vi "UHR-Fleezers Control (host) - 10.8MV.vi"() -> ()   [LabVIEW 2013]
uses:
  <vilib>/Utility/miscctls.llb/LVPoint32TypeDef.ctl
  <vilib>/Utility/miscctls.llb/LVMinMaxIncTypeDef.ctl
  <vilib>/userdefined/High Color/nirio_resource_hc.ctl
  <vilib>/Platform/TimedLoop/XDataNode/timing_clust.ctl
  <vilib>/Platform/TimedLoop/XDataNode/nitl_modes.ctl
  <vilib>/Platform/TimedLoop/XDataNode/wakeup.ctl
  <vilib>/Analysis/baseanly.llb/Mean (DBL).vi
  <vilib>/FPGAPlugInAG/PCIe-7852R/niLvFpga_Open_PCIe-7852R.vi
  <vilib>/FPGAPlugInAG/PCIe-7852R/niLvFpga_Reset_PCIe-7852R.vi
  <vilib>/Utility/error.llb/Error Cluster From Error Code.vi
  <vilib>/rvi/errors/niLvFpgaAdjustHostInterfaceError.vi
  <vilib>/rvi/interface/common/niFpgaWaitOnOcc.vi
  <vilib>/FPGAPlugInAG/PCIe-7852R/niLvFpga_Run_PCIe-7852R.vi
  <vilib>/express/express analysis/Spectral/Block/exnSpectralBlock spectral measurements PSD poly.vi
  <vilib>/express/express analysis/Spectral/Block/exnSpectralBlock spectral measurements PSD WFM.vi
  <vilib>/Waveform/WDTOps.llb/WDT Append Waveforms DBL.vi
  <vilib>/FPGAPlugInAG/PCIe-7852R/niLvFpga_Abort_PCIe-7852R.vi
  <vilib>/FPGAPlugInAG/PCIe-7852R/niLvFpga_Close_PCIe-7852R.vi
  openfpgaref.8.6.ctl
  <vilib>/Platform/TimedLoop/XDataNode/XDataNode.xnode
  <vilib>/rvi/interface/nirviOpenFPGA/nirviOpenFPGA.xnode
  FPGA Bitfiles/UHR-FleezersInst_FPGATarget_UHR-FleezersCont_0F5B06C4.lvbitx
  UHR-Fleezers Control (fpga) - 10.3.vi
  <vilib>/rvi/interface/nirviMethod/nirviMethod.xnode
  <vilib>/rvi/interface/nirviReadWriteControl/nirviReadWriteControl.xnode
  <vilib>/express/express analysis/Spectral/XNode/ExpressSpectralMeasurementsBlockNode.xnode
  <vilib>/rvi/interface/nirviCloseFPGA/nirviCloseFPGA.xnode
  <vilib>/Analysis/NI_AALBase.lvlib
  <vilib>/Platform/TimedLoop/XDataNode/XDNodeRunTimeDep.lvlib
  <vilib>/vision/NI_Vision_Development_Module.lvlib
  NiFpgaLv.dll
  <vilib>/FPGAPlugInAG/PCIe-7852R/niLvFpga_ConfigureFifo_PCIe-7852R.vi
  <vilib>/rvi/errors/niLvFpgaMergeErrorWithErrorCode.vi
  <vilib>/FPGAPlugInAG/PCIe-7852R/niLvFpga_ReadFifo_PCIe-7852R.vi
panel:
  out "Location path":path=path "D:/UnifiedHighRes_VIs/Locations.txt"
  in  "ESP ZL-Limit":string="-0.5"
  in  "ESP ZR-Limit":string="12.5"
  out "Location Matrix":string[][](array[string])=[["N.D.\r\n", "N.D.\r\n", "N.D.\r\n"], ["0.19233\r\n", "0.00156\r\n", "0.20615\r\n"], ["N.D.\r\n", "N.D.\r\n", "N.D.\r\n"], ["N.D.\r\n", "N.D.\r\n", "N.D.\r\n"]]
  in  "radius":i32=10 min=1 max=20
  in  "clear markers":bool
  in  "trap\nmarkers?":bool
  in  "Sample Channel Flow":bool
  in  "Pump 3 contents":string="Bottom: ADig beads" caption="contents"
  in  "Pump 1 contents":string="Top: DNA beads" caption="contents"
  in  "Scripts":T1(tab)
  in  "Take Stepping Data":bool
  in  "Got DNA bead":bool
  in  "Got ADig bead":bool
  in  "Cap 1 Flow ON":bool=TRUE
  in  "Move Cap. 1 (DNA Top)":bool
  in  "Cal/Data Acq. Spot":bool
  in  "Dump Beads":bool
  in  "Cap 1 T ON":bool=TRUE
  in  "Cap 1 Samp Flow ON":bool=TRUE
  in  "Offset 2 Set":dbl=2.0
  in  "Offset 1 Set":dbl
  in  "Cal @ (MHz)":dbl=41.0
  in  "W/ Offset 1":bool
  in  "Offset 1 Start (MHz)":dbl=13.0
  in  "W/ Offset 2":bool
  in  "Offset 2 Start (MHz)":dbl=16.0
  in  "Pause at Closest Delta (s)":dbl
  in  "Move to Delta 2 (MHz)":dbl=41.0
  in  "Attempt Limit":dbl=30.0 caption="Limit"
  out "Attempts":dbl=1.0
  in  "Wait Before Save (s)":u32=1
  in  "Fish for Tether":bool
  in  "Closest Delta (MHz)":dbl=21.0 step=0.25
  in  "Stop F (pN)":dbl=3.0
  in  "Then...":string(combo)="5"
  in  "Move to Delta 1 (MHz)":dbl=41.0
  in  "Tether Alarm?":bool=TRUE
  out "Tether":bool
  in  "TA Cancel Save?":bool=TRUE
  in  "TA Green Off?":bool=TRUE
  in  "Raster Set Upon Tether":u32=1
  in  "Save at end (5, 6)":bool
  in  "N Steps":dbl=20.0
  in  "Step Size (nm)":dbl=0.34
  in  "Save ave factor":dbl=1.0
  in  "Dip Trap Delta 1 (MHz)":dbl=15.0
  in  "Move Trap Before?":bool
  in  "Save Data After?":bool
  in  "Green ON After?":bool
  in  "Dip Trap Delta 2 (MHz)":dbl=15.0
  in  "Move Trap After?":bool
  in  "Duration (s)":dbl=1.0
  in  "Dip for Protein":bool
  in  "APD to Watch":bool
  out "Duration (s)":dbl
  in  "Action":string(combo)="Yank"
  in  "Fl. Triggered...":bool
  in  "Fl. Delta Thresh. (kHz)":dbl=0.6
  out "Waiting":bool
  out "Fl. High":bool
  in  "N pts to average":u16=6
  in  "Yank Delay (s)":dbl=3.5
  in  "Yank to Delta Array (MHz)":dbl[](array[numeric])=[16.3, 15.85, 14.85]
  in  "N Array El":u8=3 min=1 step=1
  in  "Random Choice":bool=TRUE
  in  "Force Yank":bool
  in  "Force Reset":bool
  in  "Y change (mm)":dbl
  in  "Profile":bool
  out "Sigma/Mean 2":dbl=nan caption="Sigma/Mean" format="%#_2g"
  out "Rate sigma (Hz) 2":dbl caption="Sigma (Hz)" format="%0.2f"
  out "APD 2 Rate (Hz)":dbl format="%#_3p"
  out "Primary Video Display":T2(plugin-control)
  out "Waveform Graph":dbl[](graph) caption="APD Line Scan"
  in  "Inject Top":bool caption="Inject Pump 3"
  in  "Inject Bottom":bool caption="Inject Pump 1"
  out "Messages":string="7:59 AM\tUHR-Fleezers ready.\r"
  in  "APD Ave N":dbl=10.0
  out "Int. Time (s)":dbl=3.0
  in  "Stop All":bool=TRUE
  out "Sigma/Mean":dbl=nan format="%#_2g"
  out "Rate sigma (Hz)":dbl caption="Sigma (Hz)" format="%0.2f"
  in  "Tab Control 6":T3(tab)
  in  "APD 2 Offset":dbl
  in  "APD 1 Offset":dbl
  out "RMS (Ang)":dbl=nan format="%_2g"
  in  "Bead Sep. Int. Time (s)":dbl=5.0 caption="Int. Time (s)"
  in  "Below (kHz)":dbl=0.5
  in  "Above (kHz)":dbl=2.0
  in  "Adjust Scale\nto Mean":bool
  in  "Rescale on Mean":bool
  in  "Offset (nm)":dbl
  out "Mean":dbl=nan caption="Mean (V)" format="%#_3g"
  out "Force":waveform(dbl)[](graph)=[{"t0"=timestamp(12.90000000000001 s since 1904-01-01), "dt"=0.15, "Y"=[nan, nan], "attributes"=variant("NI_ChannelName"=variant(string "T1 X"))}, {"t0"=timestamp(12.90000000000001 s since 1904-01-01), "dt"=0.15, "Y"=[nan, nan], "attributes"=variant("NI_ChannelName"=variant(string "T2 X"))}]
  out "APD Chart":waveform(dbl)[](graph)=[{"t0"=timestamp(12.90000000000001 s since 1904-01-01), "dt"=0.02, "Y"=[0.0, 0.0, 0.0, 0.0, 0.0, 0.0, 0.0, 0.0, 0.0, 0.0, 0.0, 0.0, 0.0, 0.0, 0.0], "attributes"=variant("NI_ChannelName"=variant(string "APD 1"))}, {"t0"=timestamp(12.90000000000001 s since 1904-01-01), "dt"=0.02, "Y"=[0.0, 0.0, 0.0, 0.0, 0.0, 0.0, 0.0, 0.0, 0.0, 0.0, 0.0, 0.0, 0.0, 0.0, 0.0], "attributes"=variant("NI_ChannelName"=variant(string "APD 2"))}]
  in  "Calibration":u16(ring) items=["None", "Position", "Force"]
  out "T1 X":dbl=nan caption="T1 X (V)" format="%0.2f"
  out "T2 X":dbl=nan caption="T2 X (V)" format="%0.2f"
  out "Bead Separation":waveform(dbl)(graph)={"t0"=timestamp(12.90000000000001 s since 1904-01-01), "dt"=0.15, "Y"=[nan, nan], "attributes"=variant("NI_ChannelName"=variant(string "T1 X"))}
  in  "Amplitude (nm)":dbl=3.0
  out "Bead Mean (nm)":dbl=nan caption="Mean (nm)" format="%0.2f"
  out "Difference":dbl=nan caption="Difference (V)" format="%.2g"
  in  "Take Detection Laser\nImage":bool
  out "APD 2":T2(plugin-control) caption="APD 2 (Cy5)"
  in  "Flip Green Filter":bool
  in  "Set X Only":bool
  in  "Set Y Only":bool
  out "APD 1":T2(plugin-control) caption="APD 1 (Cy3)"
  out "Detection Laser Y":T2(plugin-control)
  out "Pointer Y (V)":dbl format="%_3g"
  out "Pointer X (V)":dbl format="%_3g"
  in  "Set Confocal Spot (X-Y)":bool
  out "Detection Laser X":T2(plugin-control)
  out "Saved APD":dbl[][](graph) caption="Most Recent Time Trace"
  out "Trap Delta Graph":dbl[](graph) caption="Most Recent Time Trace"
  out "Save APD Deriv":dbl[][](graph) caption="Most Recent Time Trace"
  out "Delta Fl. 1":dbl
  out "Delta Fl. 2":dbl
  out "All Signals":waveform(dbl)[](graph)=[{"t0"=timestamp(12.90000000000001 s since 1904-01-01), "dt"=0.02, "Y"=[0.0, 0.0, 0.0, 0.0, 0.0, 0.0, 0.0, 0.0, 0.0, 0.0, 0.0, 0.0, 0.0, 0.0, 0.0], "attributes"=variant("NI_ChannelName"=variant(string "APD 1"))}, {"t0"=timestamp(12.90000000000001 s since 1904-01-01), "dt"=0.02, "Y"=[0.0, 0.0, 0.0, 0.0, 0.0, 0.0, 0.0, 0.0, 0.0, 0.0, 0.0, 0.0, 0.0, 0.0, 0.0], "attributes"=variant("NI_ChannelName"=variant(string "APD 2"))}, {"t0"=timestamp(12.90000000000001 s since 1904-01-01), "dt"=0.15, "Y"=[nan, nan], "attributes"=variant("NI_ChannelName"=variant(string "T1 Y"))}, {"t0"=timestamp(12.90000000000001 s since 1904-01-01), "dt"=0.15, "Y"=[nan, nan], "attributes"=variant("NI_ChannelName"=variant(string "T1 X"))}, {"t0"=timestamp(12.90000000000001 s since 1904-01-01), "dt"=0.15, "Y"=[-0.0004235663930173644, -0.0004722739341410556], "attributes"=variant("NI_ChannelName"=variant(string "T1 Sum"))}, {"t0"=timestamp(12.90000000000001 s since 1904-01-01), "dt"=0.15, "Y"=[nan, nan], "attributes"=variant("NI_ChannelName"=variant(string "T2 Y"))}, {"t0"=timestamp(12.90000000000001 s since 1904-01-01), "dt"=0.15, "Y"=[nan, nan], "attributes"=variant("NI_ChannelName"=variant(string "T2 X"))}, {"t0"=timestamp(12.90000000000001 s since 1904-01-01), "dt"=0.15, "Y"=[-0.0005883053071687949, -0.0006281319620349712], "attributes"=variant("NI_ChannelName"=variant(string "T2 Sum"))}, {"t0"=timestamp(12.90000000000001 s since 1904-01-01), "dt"=0.15, "Y"=[nan, nan], "attributes"=variant("NI_ChannelName"=variant(string "T1 FB X"))}, {"t0"=timestamp(12.90000000000001 s since 1904-01-01), "dt"=0.15, "Y"=[-0.0004680013428144157, -0.0005167699209570592], "attributes"=variant("NI_ChannelName"=variant(string "T2 FB Sum"))}, {"t0"=timestamp(12.90000000000001 s since 1904-01-01), "dt"=0.15, "Y"=[nan, nan], "attributes"=variant("NI_ChannelName"=variant(string "T2 FB X"))}, {"t0"=timestamp(12.90000000000001 s since 1904-01-01), "dt"=0.15, "Y"=[-0.0006226691488387671, -0.0006504715109714008], "attributes"=variant("NI_ChannelName"=variant(string "T2 FB Sum"))}, {"t0"=timestamp(12.90000000000001 s since 1904-01-01), "dt"=0.15, "Y"=[-0.0007901852473525123, -0.0008601641895809732], "attributes"=variant("NI_ChannelName"=variant(string "PSD Y"))}, {"t0"=timestamp(12.90000000000001 s since 1904-01-01), "dt"=0.15, "Y"=[0.00031556138798181086, 0.0002525101474044007], "attributes"=variant("NI_ChannelName"=variant(string "PSD X"))}, {"t0"=timestamp(12.90000000000001 s since 1904-01-01), "dt"=0.15, "Y"=[-0.00019678334910122974, -0.0002453993346964931], "attributes"=variant("NI_ChannelName"=variant(string "PSD Sum"))}]
  in  "Signals to Plot":i32(listbox)
  out "Trap Disp. Freq. (Hz)":dbl=6.666666666666667 caption="Freq. (Hz)" format="%#_6p"
  out "Display Period (s)":dbl=0.15 caption="Period (s)" format="%#_6p"
  in  "Trap Disp. Downsample":dbl=10000.0 caption="Downsample" max=20000.0
  in  "APD Disp. Scale":dbl=0.1 caption="Scale (Divide,\nfor above plot only)"
  in  "APD Disp. Downsample":dbl=2.0 caption="Integrate" min=1.0 max=30.0 step=1.0
  out "APD Display Freq. (Hz)":dbl=50.0 caption="Freq. (Hz)"
  out "APD Display Period (s)":dbl=0.02 caption="Period (s)"
  out "FFT 1":cluster{"f0":dbl, "df":dbl, "magnitude":dbl[]}[](graph)=[{"f0"=0.0, "df"=16.666666666666668, "magnitude"=[-331.1367572010275, -79.05506245821404, -86.61411242440559, -88.4728176091699, -90.3181253945935, -94.12566333707997, -92.52740723119955, -94.92192587982518, -99.60936585245742, -96.87568627870715, -94.02570383337763, -83.8058550151726, -97.57441397235512, -101.59968530846606, -101.523049255742, -103.35038532190343, -101.58594091014982, -102.96098031851216, -91.39759462745924, -103.75019963279499, -104.45030075054324, -103.04245334279298, -104.0720279134107, -106.06482372394834, -103.69131867828104, -104.40395035115309, -105.96420043276396, -107.6735556337804, -106.673030006608, -107.34889066208132, -108.05626565233933, -106.25659018850432, -105.29934513380842, -105.43096056709592, -108.3728498841465, -106.0555440144992, -105.78001282181421, -107.48741857324953, -108.67624970548897, -105.39976667156175, -105.91413119232612, -109.4222808198164, -107.0898971593174, -107.91164191890915, -108.26032038855709, -107.58332347164534, -108.23559688234297, -108.01271040303237, -107.66511723652701, -106.51901583170391, -109.27249501469946, -108.55647681594805, -107.93499259231463, -107.05068166453935, -109.13641475410455, -109.29679733781423, -108.19360835527803, -109.57747591546632, -109.58364591011674, -110.47061433372711, -109.8144340420426, -108.79067462293897, -107.54887553357234, -107.99559866705923, -108.85023923652685, -109.68733225238618, -108.51101278437793, -108.51620475114115, -108.22212402200637, -104.63726950302143, -110.2989919678048, -107.61796444414897, -108.68882962798736, -104.79193983043893, -103.59504263746938, -93.64633660288543, -101.9191640501395, -105.73717393151816, -108.92572458793902, -107.43962662800902, -107.79595323081325, -107.0923101993207, -108.17603277205289, -107.87074270713183, -109.20899066381877, -108.61832060412445, -109.10072003106593, -105.76480632823524, -108.60877649218978, -109.67541158970121, -110.2286232768028, -109.84952155309578, -109.33772024076384, -109.95251642394683, -110.14777282585466, -109.13825677905699, -110.05989365698167, -109.39359990189426, -110.56255614635295, -109.66477183197163, -108.9397158528824, -110.26529907650465, -109.20049464984628, -108.20183857013548, -109.09752250184418, -108.00440442238454, -108.35465963524055, -111.16774134451799, -110.34812550238405, -108.94506763426756, -108.72845542102493, -109.41512344014713, -112.44661664432377, -110.35437330889101, -111.32939440655925, -109.42989530434981, -110.98084669076195, -111.92160561143541, -108.57755551751093, -111.40042616180912, -110.15284955891853, -112.21455132279115, -111.40787773511747, -108.82949641635288, -110.13442122547907, -111.42229298204664, -112.06314940885191, -110.6015308813694, -109.51144097251623, -111.15989713761475, -110.25535755335385, -109.65868178057926, -110.51649885452997, -109.77194745285269, -108.4234206864394, -109.50892632093968, -109.46471287444389, -107.92241289271415, -109.72283805386196, -108.63426821579918, -110.37316681536255, -111.09713996884652, -110.32903619589223, -105.32012665515045, -107.36858557554393, -108.00382215905725, -110.06430686942338, -108.81666625979916, -110.01277074453823, -110.94194741225512, -109.65934609082873, -107.80979136006962, -112.81333866824724, -111.61474300955487, -109.83998277184975, -109.45953946904639, -109.79640584952526, -108.19172301667324, -109.28894656674316, -107.61471301278785, -108.83814006090513, -109.08866847726084, -108.20250571862371, -107.96222236861584, -107.03811197900873, -108.93533000393974, -107.74482548035408, -110.79811544577694, -111.1387476496877, -107.42970105883512, -109.18442281176472, -108.73546184641192, -108.71800246690864, -108.51945944378063, -108.06825856571285, -107.27210712368412, -108.12304695877637, -107.84933283677306, -109.73682373154998, -109.32284761503395, -109.31328817453769, -106.68762108642842, -109.79203616876461, -109.9020278896408, -110.27080024357275, -108.54152101558762, -111.00464391726017, -112.42244020766577, -110.82707315747889, -111.00344011890857, -109.90461839395674, -109.42877207451863, -109.73549298167016, -111.67494793393293, -108.85799077901427, -108.5348443278263, -109.803781083881, -108.30644755543659, -108.5079527456017, -111.2055351312823, -108.53089994340155, -108.01739789012176, -108.70360662855235, -107.95873456794631, -109.58297170693093, -108.9372401694271, -110.15921663527153, -109.22399119911955, -110.89883651739237, -108.92840112258382, -110.0545300523626, -109.05961065387005, -109.45831398589371, -108.61239387653227, -110.13001256174265, -108.80060224137931, -109.46327400696283, -108.0177965824709, -109.29727944627197, -110.3237255895986, -109.03258262543821, -110.97880178489321, -109.70034895077919, -111.16405638194153, -109.17324451464711, -109.65698250854277, -108.96750235822178, -112.00534231585624, -108.69274607723942, -108.98110446396657, -108.40723795464795, -111.44459094807324, -111.74799245277113, -111.1601960491512, -108.92048232753773, -110.30506377784799, -111.33145973979093, -110.91850998672503, -110.33684985776448, -108.90206518366908, -109.28458878227542, -108.98773986023751, -110.85813863075646, -109.00041591105906, -110.84543686681204, -109.84382395806176, -109.69722434763266, -108.50915601095721, -107.80829925826895, -110.59736107582401, -109.75377770317087, -109.3992084496136, -110.51151565846742, -112.49753959826434, -109.7299632589479, -109.54070743868353, -109.90314341132164, -111.05974202976806, -109.03766862152392, -109.46667095459878, -109.52800799036197, -111.3163121356807, -110.07817134522178, -108.69251657453547, -109.40472158898045, -109.71400709815576, -110.60534468715097, -109.46937396724682, -107.70342491418788, -109.86331122597839, -108.64971387994616, -110.90117371097081, -108.34928840565928, -110.04172889660904, -111.52979926554961, -110.34759300823305, -109.62712781837159, -109.24131154553284, -110.23196152450447, -108.68509612326807, -108.0246905483419, -106.61876139289784, -101.5519630114271, -80.57695480953835, -102.03744443354402, -107.1449217193017, -110.0695213407169, -106.61597783999268, -110.79221011808191, -109.58974545931426, -109.1149802216988, -109.20993813088597, -109.63768480465863, -110.10428394219181, -109.08445084271477, -108.83472375362581, -109.69508502050168, -108.05588796178941, -110.62586360101581, -109.95315261676905, -107.52208264977473, -108.80708007514875, -110.43484881098874, -110.45942171588936, -107.83804717866751, -109.98973910294193, -109.3496496054193, -108.425252911127, -110.94579264380809, -108.54181722177951, -108.67696070083541, -108.4150202151644, -109.24973583101504, -112.0454922608961, -111.29046597340738, -110.75018248960077, -109.38326363603683, -109.2033340336957, -109.45076170874889, -109.52878049853727, -109.32340869724774, -110.98123395128233, -110.75736340635505, -109.7218385823809, -107.97422606064993, -109.77313701758703, -110.95948744392717, -110.08996774172691, -108.51011830110778, -109.78063140243836, -110.65996628628228, -109.83684298615616, -110.33329049188029, -110.13755118968292, -110.3717925645783, -108.55302219178951, -106.86811628734195, -108.6302156589162, -108.75341391045045, -108.32589578384841, -108.70061474734084, -112.30742263527534, -109.16842570592085, -109.29767035534508, -108.87829025017463, -108.2255616391397, -108.4316108616088, -108.82995906929271, -110.40135575415563, -109.51623498946435, -109.79409808792403, -107.03832759632121, -108.36534528684132, -109.72010868372905, -107.90933028179892, -106.95643597294047, -111.29929166165778, -110.23001135794706, -108.98838015381585, -109.79115357104436, -108.18627479511115, -108.14988122174307, -109.12074063466532, -109.41904850488358, -111.40409873721113, -108.83156790193294, -108.77032248953847, -108.88363158686694, -108.47515048290681, -105.94172147874599, -109.38146940214403, -109.21277078848794, -108.11309390545507, -110.70840012427504, -109.5504457849329, -109.52330684534209, -110.06776026911132, -108.21949434182314, -111.21266686269992, -108.78581501170974, -108.43115799297222, -109.63260325780062, -109.84070220619535, -109.72041980780126, -110.29615941882527, -110.60316734262464, -108.79165446414692, -110.95840439895592, -109.64926233107009, -109.16526769544322, -108.65292362430982, -109.56113898129935, -109.85693046339026, -108.92316027325207, -109.79492493553914, -109.38157962945887, -110.24545136266825, -109.30031463492487, -109.0795429936869, -111.4091719525013, -108.63499083917162, -108.43863465339358, -109.23207864880891, -111.21947487191643, -109.24525201480154, -109.56842406077318, -109.46711940800672, -111.91389548262572, -108.15655736690546, -108.71882059966947, -111.26328503478568, -110.95027143873176, -108.4853106242357, -110.36902802777546, -109.9314203579182, -108.77686164101732, -108.71871020068312, -111.04829661168574, -109.95072655339462, -109.88221342875462, -109.53241732756136, -108.2625005404823, -108.00677030040697, -110.19659317581693, -108.93858924796267, -109.46817875483995, -110.78063992017232, -111.11066570318451, -110.78774336696706, -109.19199744617812, -108.54914256407436, -109.28414960420909, -110.64143585101183, -110.5855350821307, -109.47578632252726, -108.89705360836223, -109.89214013612292, -107.93271261027171, -109.32631601340563, -108.60274611341092, -109.40110159872573, -110.889237682208, -110.01391165813328, -109.99747108785071, -108.65542819213674, -110.37211847668736, -110.44656500845738, -110.8128133834973, -108.8909299260433, -110.19551227077532, -111.37647266643523, -110.83802189730321, -109.98519377913681, -110.52378970770522, -108.16970420057817, -110.70974729773344, -110.76836765494402, -110.26884275594577, -109.22041044268806, -109.87809744746195, -107.76823252107832, -109.12119474042969, -110.28066108731146, -108.55000033509207, -110.18152097767907, -110.73030521152278, -111.49470908029893, -110.2320929919509, -110.03370979233021, -109.79181668155233, -108.6673501209991, -109.86695766650877, -107.88926518046961, -110.95525003776572, -109.18130359755742, -110.42618009658618, -107.90341931158893, -111.44736855661769, -110.72634267386593, -109.29945988519303, -107.67889101961411, -108.81148059987765, -109.13375212757057, -109.8122873383549, -109.80176697684155, -109.96342275204768, -109.90406635707086, -108.75674342748256, -110.12362902701081, -109.82151095527837, -108.62543344241836, -110.09171852771195, -110.21434637862887, -109.97254504855631, -109.27043209093468, -111.35149588204125, -110.12399876776051, -111.65983675538546, -109.28788875768564, -110.86554069990251, -111.26990906470603, -108.60956517491746, -111.49613890850938, -111.79685722966795, -109.26269485364045, -110.38555615546439, -109.40641023162068, -110.966136593156, -108.78892524584494, -110.29340727375603, -111.44032043281035, -109.95212021173755, -109.79233511584334, -112.41184021118175, -109.73687851881148, -108.65493879781806, -110.76132988919045, -108.43230346094671, -110.32968175895853, -110.29890782023821, -108.77609076424456, -110.3298662333555, -109.47734504217333, -108.2677295732245, -109.21234363352882, -107.83278941978479, -108.85136784424789, -108.43241251530755, -109.76609391460555, -108.53204373005357, -110.9660641972934, -110.3152512161094, -110.72570499399905, -109.23877906286317, -111.72407743101837, -109.20311421918561, -108.06021800233717, -109.29288625761943, -108.78395253409145, -111.85250172876302, -108.78827588901797, -109.79775055719482, -109.12089297455859, -109.49896359356035, -110.34432647103819, -107.94700097960238, -109.30489238477631, -108.89170290869342, -108.82574563272509, -110.11024077194833, -107.37946433552314, -109.60167933458756, -107.80625057819019, -110.11489057210264, -107.35436859378505, -105.69819484613895, -109.11280625683739, -109.27770293057978, -107.7053735252589, -109.75022444894368, -109.3310543596577, -107.87683693707739, -108.19931495338068, -109.26462246191564, -106.71885779297867, -100.00018022217961, -92.54434511397295, -107.20472143807373, -107.39203415155283, -110.04461177268398, -108.48860496315312, -109.0057168110333, -108.37627790492552, -108.4108380728248, -109.65509454313073, -109.64243000632982, -97.04219069306761, -109.0928856629964, -107.9760697315632, -107.52611064047497, -108.87702814778996, -109.08437599027614, -110.70097118837974, -109.00969860961283, -110.38275386163214, -110.0699155421545, -106.91498895181175, -106.22178738309017, -109.36827866896039, -107.59953130968307, -109.19516217272808, -108.31502495393616, -109.384158926223, -107.11670654202719, -108.09436312738853, -110.14559230873704, -109.84997663447679, -107.83465335309926, -108.60947100624459, -108.9932479423645, -109.17174810371898, -108.79457339828916, -109.40909327982367, -109.6328723628302, -109.51081854476179, -107.63054408568418, -109.63728404010122, -108.51163794839918, -107.55002282725216, -108.97796212764939, -107.24648164623483, -112.21470452291085, -108.74294024554423, -109.62070777514892, -108.05768666239368, -109.8224946685739, -109.34575507446003, -108.53536952609525, -109.60789300457671, -107.56681538208278, -109.22777325016398, -108.79047910308894, -110.10332477250668, -108.00206387955672, -108.45604004720035, -109.00645795765472, -109.81039564269616, -108.92785144634745, -108.3978471520567, -107.94411095685999, -110.53486519304262, -108.8773780319227, -109.03345093296107, -107.30746693745031, -108.54277704832029, -108.77629108166091, -108.91111762599647, -107.74965195880401, -109.97375370738439, -109.76326492689246, -107.91717581777407, -109.0730556927617, -107.66804873204664, -110.40438871064791, -108.05794247751498, -108.80206615156494, -107.51329354700796, -108.83687012994949, -107.57713176895379, -107.94774159581414, -109.41894615439651, -107.10869425078764, -110.51480854078629, -108.92221367099775, -109.91358786461535, -110.1744263092835, -109.30795472883494, -107.91359710691006, -109.77888185049835, -109.52060975706438, -108.66686651982212, -108.71041801553639, -110.13619546359467, -108.87957097273856, -109.72150387215271, -109.00776068810654, -109.70251113927438, -110.75769213896399, -108.53234896741436, -109.69439526582246, -110.15412541604617, -108.25183374628219, -107.97402569656481, -110.34920156998648, -108.45106995186384, -108.82031145748209, -111.38690005057539, -107.01968459818563, -110.3044500039584, -110.8755481852125, -111.08915057663255, -107.94824988655199, -110.21669144934839, -109.90539774633154, -109.58985438756767, -110.12258796623348, -109.41689951612143, -109.31128210476795, -109.00258476567323, -109.11093063041056, -108.83347064311234, -108.32685287566952, -109.44770946560935, -108.40145063144861, -109.68448193892085, -108.76525439243828, -107.62837139034596, -107.39300298848994, -109.36993934990318, -109.2465218489418, -106.66307369796812, -110.15891092764934, -109.57151745419041, -108.92425698310808, -109.8036704717834, -108.79751146756549, -109.25926431818017, -108.46260574057584, -109.1967554647261, -110.63319560262356, -109.02343067385144, -111.22073171487528, -109.4731095097105, -109.69335000085164, -109.48782989577005, -107.95204227683271, -108.19468255763758, -111.36195112053247, -109.55696116543685, -110.3130767640534, -108.9621824253354, -109.99735074896789, -109.20198058456344, -108.12100614259485, -111.27227490807289, -110.09248554008288, -109.14395535060149, -110.80882692379708, -109.22632926901655, -108.64497210802793, -111.00030482190711, -111.1317849358033, -107.43140429257826, -107.9783302193555, -109.2639893652291, -108.97008485446163, -108.66556668859064, -108.12995785876932, -109.73001061107855, -108.09691302413727, -110.68391499215569, -112.78583642012705, -108.7093037763389, -110.67868795924797, -109.0190959349128, -108.36247198231372, -109.82829353258869, -108.24916379311045, -109.84154533905823, -108.55470160833775, -109.75438989348815, -108.82865632118325, -107.63622268162582, -111.00943492886312, -110.81824358463759, -109.46028423652966, -107.52479398900992, -108.99087806823736, -109.94494831750349, -110.26788355564504, -109.8954055022304, -106.9478122391182, -108.91705388158901, -107.76095584490312, -109.28456723055147, -109.7982307261767, -108.98552661346622, -109.98937979783426, -110.57907422426224, -108.68113463944836, -108.06257240208589, -110.0707224529617, -109.19515280354733, -109.35868842818849, -110.37311467065695, -109.0404734478992, -108.16686395270187, -108.61859220485148, -109.19986437876149, -108.19707189725302, -110.06564239663074, -108.87850403465154, -110.63824157544798, -107.36918104067212, -108.7008736325543, -110.9359398265406, -111.08529123080929, -108.44209934821818, -109.79529621208783, -108.38917887958179, -108.169117639508, -109.24332926356216, -110.50584058811704, -109.63592524002665, -109.32261039377495, -109.16720880524552, -109.3084314664462, -109.5812223978583, -107.70213196487856, -108.0557884982431, -110.67058020007828, -111.68459781023608, -109.66270627185824, -110.52536245663693, -109.70208409132103, -108.78645420809342, -109.23122088059863, -109.24601474121832, -111.25604763816514, -109.50225851581177, -107.32434217163818, -109.28548556764925, -107.59972621660836, -110.46928774723048, -109.25950101547609, -110.32016453935465, -107.78482761561703, -107.89462895091089, -107.51366154391481, -108.08036891159172, -109.53371809947035, -101.2452927166745, -109.32763325689056, -107.52166868423687, -109.89648659445174, -109.11350200980485, -109.81336712738089, -110.02799517445062, -108.02767143538516, -107.97850220501483, -109.50772934896838, -109.31069875721964, -108.49991657749598, -105.60880911233095, -109.79128597340213, -106.91084537903113, -107.84880087118997, -109.63628170511824, -109.03203967193224, -110.64186113413658, -110.98027990365594, -112.33841002907062, -111.01793075565425, -108.58025797022215, -110.4259296883756, -110.38643255981424, -108.93051671115133, -110.97544177116494, -108.63883100482677, -108.37581711765226, -108.90240163126536, -107.94688047875466, -109.9482937437732, -110.09097112364414, -110.09805032265376, -111.44307114024532, -109.15483789122554, -110.9713708217832, -107.8548737634672, -111.41418477109195, -109.45699779859628, -97.03595099331734, -109.16746744169623, -109.66209204485918, -112.57048704774604, -109.73989735035725, -108.16252575067017, -110.7546980664636, -108.91536673403449, -109.20509151422344, -111.0260632167785, -109.62924582406518, -110.45466277291722, -110.2973970018937, -109.67550222925419, -108.84481022020094, -107.23686414357573, -111.79004633370906, -109.85453094194085, -109.45617270081004, -110.73920606732504, -108.90879956851099, -109.67774425528265, -109.4745715721361, -110.18080454693559, -109.26079184315502, -109.41692499885505, -109.02240975088358, -107.80833423058168, -109.32657361431549, -107.87138278655101, -110.910364670719, -109.70067156846706, -108.55301754282077, -109.4243252157005, -109.77567725161107, -107.83737232063925, -110.36509412773016, -109.6371048811367, -109.49430894422814, -108.55509251499753, -108.03996302911446, -110.4385715838736, -110.08864436068788, -109.48922484379962, -109.90865554258562, -109.7491963238264, -110.04796094537969, -107.413043439116, -108.54229076126079, -108.2522516728666, -109.75464941327974, -110.26795832300996, -109.28073673851144, -108.62990200974927, -109.89408067552287, -109.09160284731726, -109.90740624925795, -109.92534708896517, -109.79578862362752, -109.97278346890566, -107.80679350393824, -112.81728446281548, -108.09689504419987, -109.89549991422173, -108.43930976031248, -109.95153099843282, -108.18277483720716, -111.89607792605433, -109.52567003805, -109.17125106979698, -109.64300739407085, -108.21045178846524, -109.64036472149706, -109.02324448538845, -109.039163008889, -110.41006510134076, -109.50289952116489, -110.4732620447796, -110.08777181504614, -110.15589511434341, -109.55705089158471, -109.2547682932589, -110.86823885471617, -109.96330502176939, -109.85995369810554, -110.63211290903473, -112.08007783432191, -110.24725218052279, -107.62861148917592, -110.08691795849435, -108.89793794632287, -111.07702220466341, -109.46946126482341, -109.19747345337464, -110.70018609416007, -109.66366205691908, -110.78032312133551, -108.05724200456513, -108.195661625627, -110.90724508408255, -110.08307674771669, -110.76863516643007, -110.46620425061583, -109.16986788877276, -109.61921294239114, -108.51159432329543, -109.96308336765689, -107.38178944242856, -111.95930944846394, -109.3329826827624, -109.59119636368249, -108.83148571828912, -110.46194288788257, -105.87694286145472, -107.985886302892, -109.2975019660806, -111.05138725716857, -109.60005889204612, -110.92871351729086, -110.73480546964537, -108.41587420326718, -109.84275465824477, -108.8249071047676, -107.65358887817105, -108.3254150042995, -111.47362100321767, -112.7287536850025, -108.8217125660507, -109.50232320231771, -110.29587061625348, -109.30644535112089, -107.69178032077258, -110.84522325672016, -109.3735891463141, -109.12506388923123, -109.65582307934665, -111.11427272192576, -112.19827973435466, -109.11306367925813, -108.19203577968261, -107.89831568266465, -108.85805249169313, -109.51100049661844, -111.71546684086955, -109.53880495724334, -107.07739286222231, -110.66836728754211, -111.5415170557177, -110.16051267940297, -110.6107546662698, -111.36389129556191, -107.77888179117923, -110.34160392509817, -109.61287125994414, -110.23791773883013, -111.00669159903549, -110.97165069538953, -109.43965413392434, -110.6813161690388, -110.31441293654314, -111.96129906273796, -108.15998218707462, -110.08095912053633, -109.41084567452768, -109.28774416263552, -110.80159950384204, -110.41956747809755, -108.85005186267244, -107.9069227847757, -108.84249369063123, -109.92569208845894, -109.34109797584448, -109.41334788055491, -108.76462023086997, -108.22069272136177, -107.0786679601274, -108.30206755098202, -108.57613406368954, -110.83330887636482, -111.93966942736989, -109.76373713473264, -108.25782074884941, -108.16490627215555, -109.93351470267982, -110.75525684428368, -108.22814762283093, -109.73442331991602, -107.53145627482685, -108.27195221226805, -110.33032779278457, -109.48951857415828, -108.12599093700939, -107.97627415508097, -108.81426859968796, -111.21764717894752, -109.80856212352333, -110.92658779118501, -109.71551885834796, -110.38682741010847, -108.87671328341361, -109.68368600774755, -108.35359806351899, -111.7519400010676, -109.89407081573103, -108.24301180922755, -110.00646944788126, -108.6685299083706, -107.52856885980722, -111.7622363038509, -111.0025144494897, -108.64719599357296, -110.62968467177518, -108.821509935539, -107.94915453463719, -111.53070432277694, -109.87282048586256, -110.71167589371663, -109.79225006081626, -109.96203471712074, -110.29921092232489, -110.10644439440416, -111.28815007382043, -111.19165661703703, -108.46024117100558, -110.22528296512183, -110.32184972386672, -110.05120383416072, -109.78792549362107, -109.00355659956696, -108.85989369286315, -113.00899556732638, -110.91756826567867, -111.25016866167897, -111.84225040552181, -110.54451635944174, -110.72722829912917, -109.60759702177283, -110.49362602516815, -108.74419542915284, -110.3379671069179, -109.66259088220754, -110.45956400953156, -109.13956157147233, -109.27130155486806, -110.83015602667983, -109.17970724944131, -109.09662765889193, -108.0447366108107, -108.9536269357457, -110.35663108940085, -108.73418835472056, -113.42965806805827, -111.81270536656905, -110.06155590173537, -108.76582224646269, -106.7488061675813, -108.5700320158723, -111.11038264410035, -110.41435767488723, -109.12763443489911, -109.30517580756394, -111.61251165371237, -109.8116632664339, -109.36845864976851, -109.00390009629231, -110.54359197165573, -109.52629258465976, -110.75932197632896, -109.50903215359567, -107.42652056246085, -107.81146496533543, -103.22224383145215, -108.53803076819163, -109.78623360072066, -109.66306634612869, -110.80245829141279, -111.87835085452016, -102.27372781471168, -111.27763038431458, -108.45838423437681, -108.79077917058028, -109.31951755762685, -110.05415097017186, -109.5535934823387, -111.62732254641111, -110.73478247119641, -109.9468722686683, -110.39698367573979, -109.30612942398305, -109.7578384694043, -109.34817295524313, -105.56944757301993, -110.1940418750125, -109.27076023513962, -111.03491935225027, -112.2980497521063, -110.65725497955563, -109.0567530102422, -110.31700596563523, -109.64508026365678, -109.6190471404421, -110.52566833759428, -109.68595899227789, -109.7431160985074, -110.4798230300751, -109.45506977604765, -110.69504157940786, -110.63067849573177, -108.06456949500138, -107.99354148885966, -108.11349194720599, -109.15944121207349, -110.61766925164031, -110.14145801314527, -110.67420842201165, -111.91532881806512, -112.15901550030345, -109.94774413630104, -109.2819568305201, -110.94623189179737, -110.17685430287735, -110.39082916961016, -109.53953238698966, -110.76940623620611, -109.89327922318515, -109.10275695043765, -110.21445972656734, -110.58968777252528, -110.57016757660259, -109.59208496373341, -109.07946946465374, -109.10762003745964, -110.36892993974607, -109.81864495218393, -112.12972189864566, -109.26185849434863, -111.56305819991357, -111.36019621828058, -110.3397604159226, -109.58675612753163, -110.58041217474447, -106.34739062044932, -108.6722699609389, -110.03906060709869, -109.16794717548382, -109.65012481802809, -109.35377624077988, -110.51889143862303, -110.03397458059777, -110.7981307056636, -110.56653507062292, -107.61367005067231, -109.99279736988825, -111.79875182878175, -108.60382315996031, -109.71381533228038, -108.60388131505613, -107.0933685540362, -107.86037690830757, -108.40980028847238, -108.83869602763895, -110.76921375395764, -109.96766364716046, -110.8256171465781, -110.13805084291067, -108.5349140035878, -110.57158437465219, -110.8920694413417, -108.71646695477324, -108.33274238445665, -108.96152108305608, -111.03750932994224, -109.48915027983756, -110.29725207211165, -110.79527247268442, -109.47969936716117, -109.79306701834035, -110.16840035577498, -110.29840230783668, -109.15306387075587, -110.72651274964761, -109.08881658764956, -110.8349724030761, -110.64653625576447, -111.40392562616867, -109.94581588927414, -108.85136340231294, -109.77228546607624, -111.48297395390018, -109.7334001251941, -109.30537415590783, -109.63937411233408, -109.69785848648013, -109.3523781030017, -112.04667421182404, -111.56311816195343, -108.18548447362308, -110.63388993686104, -111.39768634137992, -109.87157345395542, -108.6734208287271, -109.46213300216168, -111.75774769437145, -110.10245994173216, -109.52385139033495, -110.96513097775451, -111.8709319163154, -111.54948269614047, -110.29760900080463, -108.52168175904663, -111.09033925738258, -111.14752744054172, -108.83074523709202, -109.05704141259113, -111.74377805749482, -109.57200906899736, -108.84121318623825, -110.86657990204343, -109.54363603755047, -110.89448416316372, -109.58965570570145, -110.21012263847972, -110.4063470702923, -109.5021950342969, -110.33648801598177, -110.90551031296536, -109.69205870504638, -109.8648503154861, -110.28183391384131, -109.65970942950766, -108.43615680946908, -111.11790511866548, -110.89043476451553, -113.64898442872548, -113.08004494963895, -110.81525412051718, -113.91009875719509, -110.95802128672312, -110.40944585634135, -110.33464695414992, -109.98984645778987, -110.18795067005652, -110.62364351231234, -110.44029833291248, -109.01598585569788, -110.95430216511514, -109.77987141110621, -108.54452361812068, -111.41780266439777, -110.47172771858405, -109.06084635984516, -109.30794593246578, -108.8764083815745, -108.18222749506985, -110.31330487887435, -109.04176821738014, -108.8558386035048, -109.47888284507395, -110.01459604573937, -110.48596659065309, -112.6781342298378, -109.85522803775775, -109.0569534499285, -109.08991286548698, -110.89485727880403, -109.18715778948663, -111.50381433568144, -111.3545424730884, -110.07710926239977, -111.99977850157067, -109.47444853853723, -109.81605328527645, -110.74995213151195, -112.56834665925544, -108.52052472391404, -110.89121213995557, -112.02004142355113, -108.66413739656008, -111.10053848695652, -110.41241079991636, -111.80152991764473, -110.21746151515111, -110.63265128607344, -109.483042128511, -112.78639954059729, -109.47114195846122, -109.23309637902875, -108.97133643967169, -110.08909147812822, -111.01105271457081, -111.18602432128249, -110.04633990216801, -109.53453538673071, -108.81939452082017, -111.13486114285661, -111.65877073200598, -111.63763706753498, -112.14107810664572, -113.6231865196724, -109.31743865878806, -109.18551713085722, -108.74951309653638, -109.28206426212142, -112.36687029711229, -110.10933061193728, -111.29501093502684, -108.19021080564794, -109.34497312126749, -110.37228033937312, -108.63277512903049, -110.61033993911002, -111.2975761598062, -111.49780004751436, -109.91019436685814, -109.32789992989028, -111.4482538110117, -110.1538439123475, -110.66347034043578, -110.05055133068794, -108.53002033538341, -111.7522199783972, -113.49108651193104, -108.03793940563418, -110.07108694011555, -110.83958739865201, -109.62805629409038, -112.69637731014087, -109.57996950503268, -110.104850643722, -108.83376203949506, -108.69400304840181, -110.59434352922563, -110.69121011800921, -110.18694553784364, -111.90598571547098, -110.30230802494223, -109.66810649416752, -112.6017099000434, -111.00296745333219, -110.64462650261785, -111.4775358707403, -111.98753241268494, -112.26574909791167, -112.04796822399412, -110.65853064447325, -109.6623218025264, -109.40559579075378, -110.42174451813142, -109.18991987957241, -111.02050178263048, -112.77950487440032, -110.42443751566815, -111.35440372400903, -108.5263524245987, -105.07498063939795, -107.15444425741984, -110.4508720018025, -110.25163264819463, -111.1383261104107, -109.91171620173931, -110.52200560606038, -110.5299174299573, -109.34628087255733, -110.26101817411786, -109.65071853372183, -109.66953335961068, -110.83590602054682, -110.980546313788, -109.4110066989163, -111.47223607390256, -110.00281523859483, -109.4088722967626, -109.00401922839337, -109.59655302543185, -109.7359970854586, -111.46016206343049, -110.23478747568004, -109.29441275295858, -109.82941912510167, -110.43088525283673, -108.21649744751299, -108.70220592702613, -105.2334473604296, -110.60620657984927, -107.97533820921146, -110.7664079806058, -110.56406610911355, -111.76465470250328, -108.84172809688911, -111.03661078143631, -109.85351980370237, -110.70091167176791, -109.52380717508088, -108.4356492672842, -112.25498760397127, -110.69648730540193, -110.36748838594507, -109.99090797924349, -111.2678642544111, -110.42541694325627, -111.4575545259775, -109.3211175669008, -112.7465573314208, -109.56208667784249, -111.59733497772172, -109.42295730962105, -108.55804089331346, -108.71397903286748, -110.09188290952392, -108.90810063278326, -110.31333217069538, -109.69794714542728, -109.06210020835357, -112.42465112160288, -111.74630553904855, -109.99304310093493, -108.93867687355595, -113.1669287525049, -109.09193568851137, -109.27500368450697, -108.99643325722404, -110.53962759110647, -111.2052088429852, -110.05855563908841, -110.30763723153481, -110.03411001268613, -109.6161415052669, -110.6304714466923, -110.17116005754627, -109.0753171640551, -110.92564270851628, -109.60831770517053, -110.25913363817017, -107.76644895378317, -109.2619309023068, -107.64198246311884, -107.37056168314048, -107.31978563121643, -107.68171928702894, -104.57515288104209, -104.75187637758803, -105.27246893266054, -106.96524396060869, -105.93920355631757, -103.66449995825586, -104.08476660009461, -104.53081578265315, -103.0148493379086, -106.74751670818362, -104.92309629919443, -103.98320340724693, -104.81633219413234, -105.77996356028235, -107.12559309216644, -107.28196039053535, -108.84583578337953, -109.4494696919565, -109.15525441177898, -109.7634811359225, -110.79433338587495, -108.44440079452527, -108.79597700117748, -109.98590735173822, -110.72144284267539, -109.30550753718086, -109.70072152916897, -109.65801130162137, -109.65949265997646, -109.82238573025273, -110.30669821947491, -109.83394128869384, -108.90433312205332, -110.664046708231, -110.39926453734134, -110.37725911098757, -112.12508639032839, -110.26795666332589, -108.98741993218054, -107.76168841100478, -109.82334992872889, -110.83516363498563, -112.60649745671253, -111.1960726449926, -111.03919163866381, -112.05129034965563, -108.83187987662883, -109.57240688505179, -109.32857861150738, -109.54934849013647, -108.29359879300195, -111.5179112931669, -109.52702486426027, -109.95429980789645, -110.7011078611564, -109.43204524997455, -105.56031249677113, -107.70609254346495, -108.78303653454363, -108.11457060956113, -110.44215460317537, -110.78267897406572, -110.33119812901934, -109.34449539666907, -108.82636558484161, -107.1834151347969, -108.83808254322192, -108.2542825327446, -108.80298057862501, -107.59922121598055, -108.9131916496929, -109.51519107961856, -107.7704986323755, -108.79678029009878, -111.13791068210752, -110.402746275919, -111.31702623823912, -108.49812727557243, -110.63723264798182, -109.32890666586829, -110.29721723278237, -111.66560929315017, -111.04227698307153, -111.36927505376269, -112.5203298417673, -109.93967930487354, -110.14533835678606, -110.3868348991775, -110.85413569165249, -108.44519725537315, -107.93391978795047, -109.82778679299085, -109.79311153223738, -109.25261055399044, -111.47738679135526, -111.11775495397512, -108.65898844492045, -110.26505495390529, -111.02017977446526, -110.34817965403467, -107.55161094495372, -110.21667403085983, -112.43970497917284, -110.70535338255132, -110.79438078890512, -109.81809822502822, -108.99167960596515, -106.5556893069368, -97.51736665041192, -105.29926513345109, -108.72453297392224, -108.23203912463346, -109.50324111400698, -110.9939986929772, -108.05367524487318, -108.37339392211176, -109.8553291283933, -110.46179639493138, -112.48795697163695, -111.88145079973545, -110.8678969738583, -110.62677605624849, -111.83824818603244, -109.76798658735359, -109.6654742351465, -112.58543522753767, -110.3406716250781, -109.55013159400883, -108.00481229232405, -109.90793236599207, -111.28597960985334, -110.54144527494444, -110.14704702870655, -111.2652554338908, -110.97520848958668, -108.63647576273343, -110.52472680617548, -113.16137826273847, -109.62457037485827, -109.53869420402964, -110.71399284283449, -108.55435337782664, -108.09492728294455, -112.2373886856363, -110.3693019226993, -111.65116752865308, -111.3223986412311, -109.67734725401074, -111.36420709226297, -109.14293108556625, -110.5982939020188, -110.29596476096043, -112.69847120697035, -108.39052787054206, -109.06205229490357, -110.00045399262885, -110.71775009467346, -110.69530760167493, -112.54144940754935, -109.55755373438097, -107.88943697845929, -109.98578587243783, -110.14202980613851, -110.80051915904802, -109.11327182471621, -109.50637030500913, -109.77023677605327, -109.98552825925917, -110.40235854896, -109.37603004890141, -111.36989177909379, -110.8399811877331, -109.30394670937987, -112.2769814990538, -109.10893172594731, -109.17733972841754, -108.35968166480572, -112.64492569586005, -110.13779257328873, -110.64439690778532, -108.45446935516622, -108.97325006911116, -110.54637968933774, -110.66412364132371, -111.38627695224784, -109.8942998516069, -110.36392017322382, -109.92355133054227, -109.61886697310419, -109.71969465343778, -109.85627196259388, -112.1407808286419, -111.1013489416651, -110.70428953307596, -109.3454280179969, -110.22984684615578, -109.53826801613613, -107.83673208330934, -108.72742563398342, -109.5745872123195, -108.83031823548816, -110.89059911076627, -109.87842545384129, -109.21980161063786, -109.07140273870678, -109.04628915564135, -108.79255665097845, -105.20875397856382, -110.0838008881032, -109.68293832806683, -111.24644641302518, -110.01257579497496, -110.99281477454484, -108.99296184719546, -110.96495665514604, -110.70404386182749, -108.25078498739035, -100.77667501455139, -107.61479263900088, -110.06600976399395, -110.02035637581871, -111.45524052052504, -109.975541184397, -111.07333860975358, -108.4808974233161, -109.59513524582242, -110.74711589861774, -109.50005300854993, -105.23071652566294, -111.81094849223531, -109.0168079712372, -111.89029991620679, -109.90672274216391, -109.30959446424889, -108.23718655264584, -110.10868108588909, -109.21139771899594, -110.33333323577992, -110.25792318324204, -110.67825932924109, -112.33148517950511, -108.9724848367048, -110.78371843797613, -111.40913868573313, -110.2930522718577, -111.9538408094371, -108.63639312641844, -112.4462941079034, -110.40266356498321, -108.66617580940074, -109.44306834729083, -111.08962916641603, -110.52132608161017, -110.53757698855654, -111.5587344449704, -109.77722315102946, -110.40060629757771, -109.45395807961631, -108.77558572395142, -109.0151938598724, -109.80739619986889, -108.9332873172888, -112.49933978358132, -111.28667321897437, -110.40629082858706, -109.9829216820938, -108.85102919990373, -110.84179127037925, -110.27309817549309, -109.88857884367955, -112.24517967927224, -110.23377125710859, -111.26951227953063, -110.09782138347559, -109.77508406986834, -110.55359722398646, -110.09534729906368, -109.96333904888587, -110.29372855476366, -111.36651812163072, -109.97141184588116, -110.16701683369045, -112.8562627359291, -110.66651146857079, -108.78873821095968, -108.59208174618087, -110.31784275318834, -109.43177042415276, -112.80272887161644, -111.79874205007107, -111.08216899537892, -110.73699224045636, -111.04738767291953, -110.43395896705012, -111.62106163510778, -111.32599933330843, -110.29360981749807, -109.66562228449096, -109.21316193790335, -110.06363162177448, -110.54480468587292, -109.31791670875509, -112.65386492377107, -109.91857609999171, -110.57233605624137, -110.7597333064856, -111.49767138733276, -109.36548654843229, -112.34145274183716, -110.52831153822652, -111.55802243871352, -111.81399803046556, -110.17680125962372, -111.23811621944807, -110.48042049674514, -112.43786993562033, -109.56507357271987, -110.67030752598993, -110.86377249100713, -109.06001892813467, -111.37023727930494, -109.52881096984436, -112.95107295160436, -110.49467818026214, -109.29804210589607, -109.89270706931751, -109.46354468058833, -112.10350702955014, -111.06083529077077, -110.49996587015904, -111.1617248913634, -108.84725633199014, -111.42852695852422, -110.01433866707184, -109.11616968390972, -110.76961079765468, -111.80403513904453, -109.84442686379181, -109.65447921666167, -111.3378640555306, -110.8882647652338, -112.58014202075226, -109.67128881545659, -111.73429980763389, -110.82258070774773, -110.71895931098041, -112.5117489008152, -109.16182299471309, -109.71651258790612, -109.7770618808562, -111.94294809571427, -111.1629115541574, -109.57489224865171, -109.8402445779754, -111.17931450307283, -110.09045865447595, -109.23658206733491, -112.54929616847242, -110.5150381158864, -111.32296447909377, -111.64472156295191, -111.65832771066007, -111.03359562742956, -110.85303206770837, -110.80655337650862, -109.3712696310075, -110.57313454785879, -111.18525355670417, -111.67423695430561, -112.00829831274282, -111.08915434609605, -110.3298290221436, -108.68552957386795, -112.11377370993225, -110.80288297661977, -110.33640536217185, -109.5907971201988, -107.9195263775506, -108.50223113159429, -111.91191347156142, -110.29585599512956, -109.50902788911351, -110.76819145749467, -108.86899533416589, -112.09963049260891, -110.13374376572433, -110.15881393584463, -110.87392107947531, -109.18658540731009, -109.72734703956934, -110.18732487568724, -108.76554115185057, -109.94122289815374, -110.39583285609643, -111.09540935727229, -110.6618176357367, -111.6281345666718, -109.69686483639367, -110.31633402076315, -110.61246951748903, -111.73300235294965, -111.34221378834899, -109.46708370903485, -110.70412671997354, -110.7007891485379, -110.31685483435038, -111.03016917417074, -110.94517365625376, -109.46580797053619, -111.20935248224806, -109.20661126636224, -109.50147037097533, -110.14241781654353, -109.8510950344643, -111.3794198224028, -111.28966889207122, -110.43347441663424, -109.86759980279523, -111.92101892013198, -109.31594011390644, -112.92253433794441, -110.74000829597605, -110.3690783911604, -111.9386136764295, -111.04196305034188, -110.41800427558245, -110.94287511448232, -111.66035388807579, -107.53723747644062, -110.68014818358719, -111.86628806511304, -110.12097497430523, -109.69880468221378, -111.4312783987915, -109.18240866486639, -111.45649839248873, -110.1242345454651, -113.75911576151633, -112.71747598882953, -110.9614554157337, -110.92294419716129, -110.87229098694876, -111.09943759113875, -109.48107247947176, -108.62783006742795, -110.8108025857779, -111.63342408317932, -112.0221522906341, -109.96411229549527, -111.29821085030613, -110.04566676239914, -108.41674583097112, -107.50256474992416, -108.68086611003493, -110.3738906060137, -108.86763212826641, -109.81681043446049, -111.04539822346567, -111.73290882980949, -109.75238769150758, -110.55268275367449, -110.48423701377924, -112.1116140908134, -109.53952175199518, -108.538611608547, -111.3788321484912, -110.36378736224961, -110.37712171023523, -109.82150687920334, -109.17046632238393, -105.1169578108227, -110.84067642540583, -112.91626789016587, -111.32030958133453, -108.93375913686056, -112.44450956563915, -111.1596840012794, -110.17380444915341, -109.634859036508, -110.68819277718731, -110.0648098825346, -108.87385575091399, -111.99676414571755, -111.32585405719519, -110.59892045991457, -110.32589048340424, -111.1172696292077, -109.79946399891651, -110.10030723919304, -110.71841081343656, -112.23013150012054, -108.94400401141407, -109.71044551701596, -111.77560214164039, -109.68779520039777, -110.96119601299907, -113.66477058855787, -110.17794649102234, -110.30159876509862, -110.11953836266514]}, ...(2 in all)]
  out "FFT 2":cluster{"f0":dbl, "df":dbl, "magnitude":dbl[]}[](graph)=[{"f0"=0.0, "df"=16.666666666666668, "magnitude"=[-324.19011195451765, -78.1272953812706, -85.85545438627958, -89.30587144190069, -92.90590394398903, -93.63083388385274, -91.8644929119412, -95.26924857401164, -97.0710469181336, -98.01148078956652, -99.33043660296804, -95.58776817681839, -99.9570097527269, -101.45494093095093, -101.51838334751548, -101.00386616525799, -103.01963069818913, -103.20223925731209, -103.53783076500916, -103.48065647812659, -103.97797518531912, -104.58942778240602, -104.46991277190502, -104.59813972158683, -104.56685024229951, -104.69893799348945, -105.05669000016238, -106.17061117835001, -106.43303821862656, -107.39468286383597, -106.2899368267905, -105.7863846168199, -105.17170638885071, -104.53818172761852, -106.70340956723133, -106.55444321137247, -106.67654843051936, -107.79888413750199, -107.86424326005849, -106.09722609215336, -107.71648639013972, -107.79500725395155, -106.17330953637067, -105.43663624517525, -108.04970689199158, -109.92106271611999, -106.2505251183406, -110.60221373795562, -107.11377887451098, -108.4126937286195, -108.37794745021417, -113.22457316369011, -106.38281814065472, -107.55385617652075, -108.93026538982782, -106.19334142366085, -108.90462602264525, -107.63084712174981, -109.12192537022624, -107.90627042480016, -109.44472079190832, -108.91731458372392, -105.74102972706788, -105.74407510394178, -107.5989477192235, -106.2838630137392, -107.46190542725505, -107.38881299750702, -109.08024783239452, -104.97871836903269, -106.65424712290651, -107.04966019632134, -106.16202578092883, -102.98374199247179, -99.1568704142098, -87.07383781389657, -96.41471411313154, -102.65176579899618, -107.65674867775193, -102.85397890306213, -107.58658613411464, -104.79044898833125, -106.65282019869865, -108.65027966345534, -109.46169054950127, -108.69969979291741, -110.4048706652988, -108.81020193837274, -109.42808902484134, -108.85398463561398, -108.3849716744813, -109.1844457168716, -109.32787859535676, -111.01992124870878, -106.64843449415699, -108.9926343573667, -111.59837822080355, -110.57121677672183, -111.17280164669164, -110.68901970586144, -111.69013245592781, -109.90200577018311, -109.3554172126163, -110.7515368822992, -109.2863324212524, -109.66209701262974, -108.50795548698007, -110.58126481096504, -112.36093896766921, -109.78612141282203, -108.85120530917233, -109.91424431080952, -109.84698632196245, -110.93960894966105, -109.77214706089354, -110.30762971422381, -108.77791302937449, -110.79522659679036, -108.47242514643455, -111.20629758187835, -109.05996769621125, -111.13574821570619, -107.79388178889101, -111.5768481279296, -110.52058839597171, -111.58729762739313, -108.99000864386126, -111.6585121505227, -110.50715371958135, -108.87151956974363, -110.30486244367107, -108.32392040018144, -108.1769507919999, -110.43198471512189, -109.81454097966842, -110.26717009815644, -110.82924135076777, -110.34103661156989, -110.0692667126265, -109.34555682020833, -109.1694484721415, -109.9940980324044, -110.81940616215803, -108.21162003366862, -107.97087538330561, -107.55312461506225, -110.60339321606872, -110.09004629292225, -109.05860430198882, -113.1412749514818, -109.81628200948371, -108.62343219429849, -109.48172424209761, -110.85978755785311, -109.47778611557064, -108.81728552967951, -107.47864241666747, -107.61735128422292, -109.62511618983821, -110.32417726356636, -108.24287897478176, -108.60460879530194, -110.2181558494026, -107.95550802888957, -110.80234484950323, -111.09955733353904, -109.43923052503506, -108.98949130235951, -110.05778199870154, -110.36224432927585, -108.13523430027999, -110.681114579241, -110.49106131529867, -108.73493328004297, -110.07663907252234, -109.9968931372618, -112.10715231091008, -108.80994125105168, -111.63774865669372, -111.54355694032755, -111.64024217585788, -109.34986300492378, -108.88053713185408, -111.14370830146245, -111.17327416167232, -110.36311492990576, -109.99414559884396, -112.96912007380595, -111.43191437097785, -111.71327312809349, -108.77202323682606, -110.25970374932486, -112.59574277180732, -109.77247894866957, -110.09219852365874, -111.7197662726775, -109.85454092697009, -110.06789440397942, -110.38055758638309, -111.04251386932805, -111.54279434240568, -109.74385329575985, -110.98924544863415, -111.17898077762852, -110.98364252730245, -110.75024385843372, -109.24766708578407, -109.67753987004863, -110.6537235844391, -111.84436313010086, -109.12654337292446, -109.65519521121124, -111.1845162935778, -110.5009101465602, -110.22980642268818, -110.88540043278346, -110.29249073109453, -108.80459864528464, -107.49372141121728, -108.50353962704821, -110.00730069533373, -112.012876492648, -109.01283702976382, -109.07442203290057, -108.2961442983685, -111.60962842680907, -108.84312815413224, -108.6276642979969, -108.75132871638827, -109.30004903844721, -107.20359872252604, -109.12175943862074, -110.43914247337625, -109.55954680842791, -110.37116786618797, -108.55907813251434, -110.19249995041955, -106.95269845697632, -111.07027929458712, -110.1073996792702, -110.61729280468039, -109.6419175310234, -109.47995019876329, -109.66602827275211, -110.01953864498805, -108.45989120418268, -109.79778555296474, -109.94663827736616, -109.52410616839379, -110.58014441463794, -110.09182359045897, -111.0487262011397, -110.49609187214915, -110.6114701312941, -111.17752423063314, -109.74965389041003, -108.58973724447526, -108.84292130035902, -108.90689510645983, -110.69840140049361, -111.30494362640982, -111.00224390075273, -110.50848328538423, -111.59232911931113, -109.30826761863756, -108.44510893127558, -109.63744704504391, -108.95037574307332, -111.36486409910674, -112.74508631930381, -111.03952454593811, -110.57133212903979, -110.59969855145111, -108.25570461975128, -110.44617635200193, -110.32190307214704, -110.95204704643322, -112.0595421753479, -110.45342552693265, -112.50183987758867, -110.08217804938009, -108.90353583389084, -107.02032313792242, -88.3334978919524, -107.92027625495886, -109.83148570028482, -110.30427997450572, -110.92855407802753, -109.67404674397338, -111.03606345823586, -110.58277018943096, -109.77692362669393, -109.39170901729935, -110.20711662408928, -109.41601946806779, -110.34213214925832, -111.2283900972803, -111.51682597931386, -110.47069117801351, -110.93808974285523, -111.11277478000933, -112.50698886748012, -112.12918507523611, -110.46316790252011, -109.9387334819968, -109.78723249688426, -107.13037722044297, -108.16132376075751, -109.07255491017162, -108.85068428558272, -110.28038153100799, -107.77611023481016, -110.69754506886444, -110.09495581837979, -109.21214884561816, -112.62718526248648, -109.22048725312992, -109.17793923163308, -110.87372121410577, -109.71902632604333, -112.61041177225496, -109.6374750969677, -110.74738952366951, -108.93404661877067, -109.84938675700889, -112.25316361679832, -110.30788094875312, -109.26929069321925, -111.20853536783942, -110.05212566057608, -111.72448131932816, -111.55474439772887, -111.81988954424324, -108.44452452934028, -109.21897824914645, -109.55634869894358, -111.36318572800242, -110.05777399011298, -109.64458567712875, -108.73315084760529, -108.93332091319675, -108.4816455312154, -108.80120578498936, -108.1804470361839, -109.7177707524778, -109.31977709844544, -109.33603116022124, -111.46120546572519, -111.7480378245176, -109.17907150677627, -110.47970652472505, -109.73718750984082, -109.7935026884937, -110.40458408612054, -110.91781389491092, -108.39352075861481, -108.27512197925346, -109.59155075404814, -110.40183121737397, -109.25423373270381, -108.37769008625712, -107.91335995938509, -109.5576520703013, -107.27392145737491, -110.98592762117059, -108.41809950647861, -111.48163889400448, -109.70961684769624, -109.22952568656495, -109.76504719131209, -108.86928627177666, -107.97855299877004, -109.8412204399902, -109.6690048999326, -112.28329030175193, -111.54977099314607, -109.55689540119126, -107.93716711232997, -109.84247640855929, -111.5098351445789, -109.14317615215809, -110.28319116384824, -110.57901069942578, -107.2890252845352, -109.66754569546274, -110.15708115946433, -108.83782190109405, -111.60783857760667, -111.46884385151185, -109.21985333366634, -109.63605494317056, -110.87999187262697, -112.26992029775087, -111.05491095860552, -109.22795442529183, -108.99135781712076, -110.46475190704264, -109.35746113713218, -109.29125989270668, -107.40922407684049, -109.24391685563656, -110.41554602144217, -110.68952735085914, -110.62457364102458, -110.39856310555466, -108.84256124354566, -110.01614601335088, -109.8071306678428, -110.2804500736802, -108.76205061238203, -110.3962440297242, -108.98253716257014, -109.32990745926702, -111.17276766165281, -110.41113652364085, -110.36616199963426, -112.09767002991742, -108.43599666470733, -110.91876588140981, -109.05329272502944, -107.07198690769708, -108.72934463903034, -108.6666471996132, -108.97529973794413, -109.68895260146817, -109.2658844652487, -109.75690097249196, -109.38585024123027, -110.17593039468063, -107.87223111061134, -108.15261097418302, -110.09277437980633, -110.8665497655964, -108.43061614348413, -110.3052458526819, -109.22446919161898, -110.51909692711594, -110.06620699121913, -109.53439413051383, -110.31952463872884, -111.4732125902982, -110.41443606663168, -109.9579358088152, -109.930778061577, -108.5473214465574, -109.34719220288939, -109.16964653934396, -110.04824158176345, -109.42616539603762, -108.3556027482992, -110.62331917617789, -111.3652147859356, -110.12362012120938, -110.13175448595814, -111.20110099151856, -111.50643914621541, -108.11659117128028, -111.06037600347967, -109.03822892917451, -108.25678204604324, -110.82608024151122, -109.15887945314851, -109.88255674562845, -111.18322672526185, -110.95836040044516, -107.91535345885436, -110.66285812468733, -109.61906549925033, -109.58059721670746, -109.65198009505977, -109.65950565672951, -108.95264505276342, -109.23343669003113, -110.74308548011575, -106.39170014998685, -109.61471203101753, -108.24258770956924, -109.84609566640096, -107.83834185503922, -108.93052854090027, -107.55568820082641, -109.758551082242, -110.65892780872205, -111.99907420485852, -110.71043004141137, -110.62257237494617, -109.15610413532767, -106.87403836327807, -108.19175324576331, -110.27819583792918, -110.23918003777561, -108.29703377268754, -110.07182881114713, -109.60256111108491, -111.00394752430006, -110.30750337485472, -108.78309624082331, -109.24103013025798, -108.76979253891403, -109.91618737478264, -108.83915940855513, -110.92536150834754, -109.72250903746432, -108.96533939688658, -111.08949280651164, -109.20335070860871, -109.37826578362439, -109.77953166722301, -110.1867310744785, -110.07114559821346, -110.7003631567182, -107.86455899696074, -108.94113264174617, -109.35999427135138, -109.33627364788704, -108.96588828808375, -109.08716536982254, -108.73575375369026, -109.47770132070654, -109.83726171472907, -110.73516506891792, -110.56827134787686, -107.65667508354096, -109.30200115708924, -109.28406803847896, -110.55374624323233, -111.2017766725333, -108.50851279608973, -109.79494403619485, -109.08320018013063, -110.21850624918747, -108.4652936555984, -108.74837610538873, -108.81326140648238, -108.83830180036702, -108.785270477003, -110.01845876259073, -108.76030368637825, -108.57879884880157, -110.6610608456059, -108.74669367794318, -111.55956030460833, -110.22906685783455, -110.48411613865359, -109.48060880085136, -112.77556331479562, -108.2676071206087, -108.8571136162698, -108.56944905160177, -109.16406757131058, -111.42259299295839, -108.25216316582294, -110.48487127684025, -109.69532331373831, -108.13992755196784, -109.2987762526628, -109.82536192480795, -111.28650061088359, -109.12820736404241, -109.37960655471406, -108.96014976926716, -107.97535047619023, -112.31953123574708, -109.06198330523004, -107.52722515967098, -107.31555373665437, -99.89671790804692, -107.44442600896275, -110.6549218761941, -108.02265794322076, -109.63582761762919, -110.00574746987859, -109.51565124961209, -109.3550083591902, -110.4541529175301, -107.85799722437162, -105.1197113090786, -110.25038075579738, -110.39710812865657, -109.3618876098789, -107.6131301952152, -109.21529527621463, -108.7995754403799, -108.48347353145697, -106.45678488065816, -109.60427918561142, -110.81194387812535, -109.52215044127382, -109.88751598659705, -109.30205143590227, -110.74984456751768, -109.03952092986351, -110.69170786328897, -110.39236248162467, -108.65456161733339, -107.60439764386904, -109.97367926606955, -110.2754359970249, -108.81546418006434, -106.99691398176165, -108.42047325825182, -107.24499915944605, -109.28116135603187, -108.70650358781573, -108.05516916105047, -107.20893100196241, -112.07029265690055, -109.38099990478445, -111.53461820465232, -108.11312509555277, -108.76714028655223, -109.89565008459624, -107.71879172001115, -108.08434857420214, -108.79142773619792, -107.25153085963885, -110.05595039449301, -109.31604222314259, -109.94405791565286, -109.04715370361387, -108.89278831045846, -108.84682466376424, -110.0067927716526, -107.63768959294084, -108.98109382020348, -111.4720219575084, -110.76023788797733, -108.78599647633777, -106.59726674064618, -108.66715709719243, -107.99134359630926, -110.11396713841884, -107.21091759882775, -108.08576824949941, -108.80217666857972, -111.72949572713338, -107.33126296136014, -107.33731660097102, -108.04470462977443, -109.42963925921418, -111.03517778720736, -109.55293581015796, -107.99948151285162, -106.59480934999681, -107.63777243313498, -108.96490626068824, -108.8948210299064, -108.30870516747477, -109.13612869658097, -109.59971429402015, -110.2571461001396, -108.7655464686992, -109.81144209568883, -109.80796806645141, -109.20948481699544, -108.68653880881129, -109.26329796696166, -109.22428132233863, -110.12571678351438, -109.14615461144786, -107.08261621308327, -109.11338327144382, -107.75421565039201, -107.45291780756361, -109.00477000647248, -107.41031480478154, -109.98948062864928, -107.45953654921264, -106.37522884807879, -107.7786128523167, -108.03610987358499, -108.05926797128022, -108.59400205554164, -109.89620453365603, -109.03811240487515, -109.96909236705363, -109.28212981785472, -109.6772152101994, -108.26493868190678, -110.55558039199732, -106.6252818398841, -110.19075011176416, -109.56520012524705, -109.8023423576176, -111.2697570480663, -108.26752571816566, -112.00337375484828, -109.85709226796116, -109.36922081321148, -108.8424844298318, -111.2512302139209, -110.61775974680471, -110.22501328999012, -107.76874906708105, -110.71023653476604, -109.4025656165291, -107.66667684986125, -107.59759854092948, -107.94763263251238, -107.3888591871119, -108.62692803125044, -109.18012867988286, -107.78662871481455, -108.5072814073944, -109.50348958982907, -109.95177634938378, -107.78756251182895, -108.03865042797304, -110.1814993556385, -109.34937567548833, -109.52162025123161, -109.50819015441117, -108.20953105254624, -110.52154040214435, -109.3324404469266, -109.2696617050831, -109.54675609195674, -108.5940367000989, -109.40184828664549, -108.2518305610941, -108.55972691669434, -109.03647225394408, -108.48166656251695, -107.42023429066523, -109.42453054302521, -110.09532345960083, -108.78315822119662, -109.97508586102265, -108.22687406536997, -109.17110028890058, -110.15390449992647, -107.88577458651508, -108.28851074361447, -108.52030295163331, -110.03496861709483, -109.40014319167584, -107.73048113044877, -108.17571683963915, -110.34839852994926, -108.55894048192191, -108.74107339998285, -111.17734138993401, -110.22946440841412, -109.45511941802884, -108.0657300641843, -109.33797363184166, -106.95974095511333, -107.93068343723691, -109.78867669512647, -107.2087297624043, -109.542665021243, -110.05035859052961, -110.30235238883523, -109.20586170783808, -109.2796396673401, -109.14260673746566, -108.22019460542734, -109.99011886871159, -109.89103038547285, -110.36964772493243, -108.62340319923602, -109.06779821699769, -109.21830861066148, -107.7402395759509, -107.7178850938205, -113.45665085929117, -109.24039191621704, -109.30387033426037, -107.61849760982835, -109.41430582703529, -109.11482836392241, -111.89328423764577, -111.84653367963301, -109.00674896486915, -109.84488648739638, -109.41914760797953, -108.53442910169935, -109.66883322968232, -107.68762956301386, -109.82583101109167, -107.83405397804887, -108.78052031141966, -107.37842078941692, -105.40843158543845, -108.81430898189338, -109.57374640194516, -109.41111270322058, -108.82621700188898, -110.2552502368822, -110.23903890097205, -110.52171662278697, -108.21249857906324, -109.97268479379733, -108.20088823960992, -108.85682002802234, -110.11642849164285, -109.94087886999255, -111.63180946270296, -108.20899499456195, -106.73341567332112, -109.90003508676807, -110.14688274481229, -109.62259307329889, -107.57811196819495, -106.88584597822792, -109.16132624528932, -109.78677836397806, -108.59319344451784, -108.55877448618652, -109.46883711353044, -108.47309455543844, -108.09487065732198, -109.82219079158135, -109.63780237877428, -109.28348848877269, -107.62893405379826, -109.46986737961593, -108.03089712610223, -110.3931917410696, -106.06970126043262, -109.41866550703786, -105.31710372440419, -109.20218082282653, -108.28467118008108, -108.80026326744611, -107.40729224715713, -111.07322915141532, -107.1057186510818, -107.98286374205958, -108.51298722989311, -108.69632670891366, -107.96509231988331, -108.15882223414738, -106.85862416470376, -109.70705792539056, -108.64519930633055, -106.78708421443504, -109.43552377900174, -109.4474526498122, -109.10135248755788, -111.43316642580763, -109.33457343739448, -110.23547887071898, -108.95690647379442, -109.21159903769149, -108.12969562680841, -110.82751409340537, -108.55724349027832, -109.8796329603075, -108.50369978374582, -107.43145467247209, -108.60003323209516, -108.77155705999647, -109.33806063660796, -108.37500858898439, -109.65641721611547, -109.81905873737344, -108.03483220769625, -110.48028107566635, -108.60527372219985, -109.28768201151478, -99.8804125587218, -108.8913334544964, -108.23534920737794, -111.07646463287153, -108.59029790589766, -110.3405916586831, -107.66387718565608, -108.73793152614131, -110.61440166477816, -108.76211382544581, -110.23236978486065, -109.10669297094852, -109.15247609779597, -109.00539004923506, -110.14424353412238, -110.55445060661157, -109.48721312920799, -108.17040942305823, -108.77592227268228, -108.77130256578067, -107.82494496098512, -109.57266989523707, -108.75767497229612, -108.13688624150026, -107.8280716764963, -105.676279602552, -107.6370316684844, -109.73508547021689, -109.25365178573009, -108.86767843317584, -109.70969944273735, -108.91917504090888, -109.97734866522867, -112.17308993943783, -110.28356299479682, -110.7927103729386, -110.30837645846702, -107.56364161860179, -109.50188349731121, -109.36065627483853, -109.75389877587511, -109.81713476007774, -108.14524057525358, -109.43832376796216, -110.89342891210596, -108.15657882822792, -106.84106061627887, -107.83091759905821, -108.61794662682962, -109.57142366843581, -109.85402645528154, -110.12877022469837, -109.19414429724044, -110.56168468006764, -108.74720588273881, -107.90448559921305, -108.54421401507743, -105.06700039841249, -109.17937358052484, -108.94317576365822, -107.79410219455083, -109.24955437598658, -108.23334395173994, -108.98759227946937, -107.05986359444529, -107.20956512998849, -109.00295831471958, -109.43119556916457, -108.93348410522628, -108.99932477701081, -106.6448790859128, -109.06877251308666, -107.67053918439544, -109.15052780608639, -110.16878033319385, -106.55101141640301, -108.02811045752685, -111.52173447126572, -110.16854119242062, -110.93164036911654, -111.25979320890855, -108.82629030379024, -108.52004501839738, -107.09697056562636, -108.94233383169858, -107.37962568194772, -109.1239201710643, -108.93949898577122, -110.62573772949195, -110.09592372075662, -107.56136391005947, -110.45600430869621, -108.79481000016084, -109.41462449554598, -109.30248158488335, -108.70735295493108, -109.9174743694956, -109.94232543385962, -110.71725446170196, -110.0346196158573, -110.34814317845934, -110.6651078322521, -107.55409880424479, -108.71734776861287, -109.50902203986271, -110.40207542979611, -108.7847687630861, -111.10599488129682, -109.30824728923263, -108.20134064331717, -110.55959112431609, -107.77099734327174, -110.23862843385446, -108.48520797666865, -108.54205896654946, -107.79288769037599, -109.84022250170581, -108.02758364115576, -109.35132492327935, -108.87009749667932, -109.86905123364855, -109.19826752168308, -106.835240323691, -109.37910022114056, -110.80633973102931, -109.12703823829597, -111.07432699570984, -111.8064506085314, -110.09349947650527, -108.66467295777367, -108.75119108236053, -112.63983351316729, -110.90940743670113, -110.27973159222081, -109.57141664526549, -108.61645363771719, -109.31742355616147, -109.5839599160637, -110.01188998365383, -110.01923429741011, -108.94779759137936, -108.26169431000017, -109.24553201026085, -109.95709526422822, -110.68677343596859, -108.7678734483002, -110.47090469179284, -110.31604700116512, -110.10256600741997, -109.76634647265719, -110.8830805828562, -109.94609564072982, -109.20662382740542, -108.12492970530919, -110.5274435478767, -108.02351960398035, -110.6264936805739, -107.14559226383577, -109.13821777857531, -111.05324489472586, -110.15190797512811, -107.96366234783144, -110.03950681967147, -109.17476300510336, -110.41251816187909, -111.39219865477246, -111.32530426869943, -109.97369363558423, -108.98666403063845, -109.62049358645565, -109.58130494498671, -111.72738873188874, -110.39825891106616, -108.57430325757545, -111.28625510212446, -108.77421250595326, -109.75025415031793, -109.51948456745635, -108.82129398637998, -109.81362137198361, -107.86292494316123, -107.49318292857053, -109.66948564589373, -109.54288390056654, -107.99912445612077, -110.3497559614379, -108.00549349666127, -110.01361420523357, -108.4977916421456, -109.67078387286976, -109.85678367732866, -112.01237658746248, -108.4855625950998, -110.84880875737286, -110.9178674382154, -110.44187536727453, -108.75076921971127, -110.04946286646651, -109.99780941000827, -110.14242932305507, -109.56343773672316, -109.6278993388131, -108.77419573790174, -109.10543670530926, -109.7801848627463, -110.30733124104881, -113.13440550301436, -109.32709134514755, -109.74136656933283, -110.01525283266193, -109.43924662938396, -110.25325289253, -107.75460576671303, -110.60057027395933, -110.71458404922404, -110.15788509050662, -110.69167485018224, -110.96006652476157, -111.01156633983031, -111.6058448010008, -109.51364005052672, -109.76058205940885, -108.43421621088261, -109.47973949170208, -109.25533250208288, -109.47422603921065, -111.36411644613841, -107.27566171102698, -110.45098686173688, -109.93589296291184, -109.03803734663714, -110.53118128434016, -110.2408872254969, -110.0532234862915, -109.94185495614619, -110.2662004220774, -109.51094016962288, -108.5210104215432, -108.13691752270934, -110.18460088390265, -108.32609309150783, -109.89652230508281, -109.80923900768477, -109.01917388968883, -110.01248300968739, -109.43415605440147, -108.09823485138017, -107.40637725320931, -109.40632232658412, -111.97981999127656, -111.16609811629485, -111.64500793960192, -110.99793748693381, -109.55531276386903, -110.2535662621666, -108.17429802469516, -109.09425673355422, -110.23187110421917, -110.55358397926925, -109.93461124753053, -109.55604345832225, -109.44569510408274, -109.72185151080762, -109.52963702944834, -109.2303630328152, -109.74819502244243, -109.3932530349457, -109.17096788339686, -110.46153727064616, -113.1073731246639, -109.43753070459397, -108.13332547768168, -109.42294574929969, -108.45798401969856, -110.29453435046327, -112.66249403705643, -108.78314667434937, -105.9634478773668, -109.14327524669528, -108.50645190860273, -100.81571594994128, -104.4482859840643, -110.68926237051092, -109.12362553230196, -109.45234390564677, -107.91461416156068, -110.67788819353727, -110.05744935668449, -111.78333392154664, -106.83628914455993, -110.11115457346548, -109.13434608275826, -110.80006861194663, -110.35323502651462, -112.29149906501372, -109.01656376530778, -109.30871662948859, -109.79736315392456, -109.17848983603582, -108.09752397056482, -111.6039030763455, -109.27008844877828, -110.84475733314184, -109.72393917557073, -111.31060762894991, -110.78858793807466, -107.12841545099752, -109.54510865218204, -105.2805426080281, -106.28514149354733, -109.50656759582803, -110.14700878401054, -110.49737016725709, -109.19811547071924, -109.92527399676051, -110.7961615015146, -109.7447227818197, -109.49432012009893, -108.714081576733, -110.09766801550917, -109.08448507943001, -110.36154838733857, -109.86328656267403, -109.21144237434696, -112.4145136888034, -108.57567151011159, -109.66748589540896, -109.72985837578446, -109.29989238126763, -109.85868902806475, -111.01778182304162, -111.23625326328558, -110.01270868104203, -109.27067928081415, -109.71171312410247, -109.28697459293629, -110.67868067201007, -110.91353786857455, -111.21479955051575, -109.11315965407708, -109.40418681804496, -107.80511819596003, -107.37201025889816, -111.81969609169838, -109.89875624306032, -110.29328043898657, -109.74853280072202, -111.39527865400605, -109.47746221101964, -111.75141177452517, -109.31325306583483, -109.30117448911659, -109.3997781364162, -109.45356931295724, -109.60585285774386, -111.33951689512735, -107.74187210470228, -109.62706021606415, -108.72139655505221, -109.79552836110567, -110.64354037499807, -110.96138240913136, -110.02215059889615, -110.92978442698893, -110.0620778287114, -110.85019647293322, -111.77397403227091, -109.81257196800128, -109.15643451383403, -110.72777566469594, -108.7463769025616, -109.80959395914073, -111.24500986151126, -110.48863498350322, -110.30863780110901, -109.79331354195703, -110.34087081762074, -109.45183222569266, -109.6440990067103, -111.15034876658994, -112.14912485578341, -111.8886180186196, -110.57054820211916, -111.07556239924551, -110.5872832735073, -110.28912501038172, -108.91501133754849, -111.44575118962761, -109.90799859177967, -109.74421995550023, -108.70941446115883, -110.28822893097275, -109.70039554000401, -110.33701797570251, -110.79445894683306, -109.57694314608153, -108.816904416038, -109.66517126767175, -109.39501469321644, -110.85775022889956, -109.3689402795614, -112.09107318723095, -110.67985626248422, -110.32971146814747, -112.08166943494875, -109.93955548712543, -109.31722953035252, -110.2062913031861, -108.22565380081006, -110.680898028151, -111.95386604441454, -110.83354130587097, -108.5873626748948, -111.97536144124408, -109.23944159551515, -111.57859477689586, -110.80135186615524, -110.4800953731021, -110.14040729648133, -109.25873050390551, -108.87000960474569, -110.97091597211167, -110.15787270199012, -111.62434537618091, -108.5421625277294, -110.42258666403919, -110.96896115868603, -108.98253068925274, -109.54245055160168, -110.28051096122468, -109.48060498658319, -109.77618362117276, -111.64513838754992, -111.13945484239875, -110.18094280356001, -110.43757222770748, -110.81588360154201, -110.11656805555333, -108.47936291282355, -109.16476249859961, -109.3549985917136, -110.77753190334253, -111.46065694661178, -110.40387985996301, -109.95673803226478, -111.58660981285446, -108.59894875229345, -109.37333363882607, -110.26849699991793, -109.30500469266264, -109.23789020998296, -110.82000706486865, -109.25927538839868, -111.03285659417519, -111.08899832832414, -110.69361682858042, -109.45187168573815, -109.9614018482838, -109.70209527974106, -112.11903952100165, -109.59713611623246, -110.70292028698111, -110.12743849746808, -110.63315585514292, -108.60450276298175, -109.32832664986026, -109.99753023477764, -109.46644696130294, -109.1781290160558, -111.58830180575129, -111.67229040267557, -111.3750024136205, -108.33616679452298, -109.99797067800029, -110.50892429124391, -108.66074740829372, -111.17094662568759, -109.87538933985836, -109.152526628291, -110.44623159817101, -110.21603106403009, -110.64376935639365, -109.36897426842583, -108.67303022227141, -109.89327693080823, -111.50442955563923, -111.37532237834381, -109.38132821290205, -109.73509680539144, -110.53918379735906, -111.22869870340647, -109.39977573957616, -110.3674665334106, -110.5366125953241, -109.99025356764304, -109.97300035646616, -109.87631077033762, -109.64608829594286, -113.02486102973394, -108.26250283140733, -109.62234918138763, -111.18766216512655, -110.33666026406992, -110.5808115327039, -108.2971671321189, -110.10964334161903, -110.61254021379767, -109.89852549557533, -110.16562049054073, -109.41433790018287, -111.2453823439446, -110.45554802599901, -113.11454453784393, -110.7333866145056, -110.00858191882439, -108.54745315874294, -110.08430415376903, -111.9006972727596, -110.3031506154679, -110.26331790366497, -109.36797925566673, -109.04860552478912, -111.83514212681175, -111.38960737633833, -109.01429665187288, -110.96404839103826, -108.95488871107163, -109.09652004914592, -111.884304581971, -110.57566691021339, -111.95113404442795, -110.13677174050159, -108.10078686353354, -107.69442565416006, -112.42676605669463, -109.12681161784135, -109.23120766087519, -110.57649395555585, -110.22143082743162, -108.40065951773644, -109.46923168308618, -111.39095086729745, -110.46375658526013, -111.45145283328486, -112.22610823637353, -110.61090190564383, -112.22250292674809, -111.7379343196361, -110.18530386733481, -108.93867365671692, -111.89304844956082, -109.06146134986984, -110.98405731832798, -109.76366821333497, -108.08326795663608, -109.95041147835065, -112.94140614324155, -111.79814935135965, -108.07337559063119, -109.13733403265212, -111.74906646037496, -111.12228668433455, -110.02899450462209, -110.22237716929811, -109.0224776891049, -110.18135850497721, -113.32516073881047, -111.3576490243877, -110.60510094465171, -109.6935518470342, -110.36313473154901, -111.95933240129618, -109.49625308071019, -109.18827910216122, -110.54311407822692, -108.4811035913567, -112.81280225723607, -108.86530665787413, -110.85796435061886, -110.40059714639627, -108.19250716343407, -108.96956521802292, -108.61281798886506, -109.78061525370413, -111.58885511891798, -109.06279169160345, -111.43043988466789, -111.63169336321079, -109.54702536206447, -109.62860636296405, -109.47865811135546, -108.02265793654806, -109.97461304995515, -110.72549884050886, -111.57309413919933, -110.03317891949746, -110.39570411598524, -110.27606115470397, -110.63294457306095, -110.71821689302902, -110.38076268941819, -111.51223508887897, -110.40703572670697, -112.24933273737743, -109.74954300082398, -108.46020292937696, -111.05315219575881, -110.38635148390118, -109.58268303790976, -112.34211536832117, -108.45894118755307, -108.96463982695337, -110.56040438523046, -110.67803313671729, -111.07349872375121, -110.42184162876096, -111.82081126435692, -108.85923651136297, -112.57723799596502, -113.65690874668172, -112.62314325834605, -110.70357529341362, -110.959925221544, -111.26336183001875, -108.1350700630152, -107.94545932312926, -111.17610778209841, -110.20386728310686, -108.55646511121591, -109.8400922569145, -111.73466587035968, -110.47272877573613, -108.33011124048193, -107.93042857580332, -108.60928277989103, -109.25240966798974, -108.96403833602028, -106.94222615757475, -109.37086694261907, -106.72743097285155, -109.03160193412796, -107.3549903889451, -106.8543848510082, -107.83503929060929, -106.30745467433752, -108.36915807168845, -107.13065938379303, -107.84769200880969, -106.08004345082777, -108.15244601930225, -108.37254117816573, -106.57863034819223, -108.1283698227614, -108.19776505569902, -107.58283412238643, -108.17365133196301, -108.6794309781181, -107.91552140588759, -111.60122989270022, -107.04360635941174, -111.55535949001795, -109.39870426166594, -109.55937904851662, -111.81389508925734, -109.88957041098786, -110.84764586896561, -110.59130246272693, -111.15944135223884, -110.19496154041607, -111.51861903129362, -110.74798816525838, -111.37312965175558, -110.10842817220238, -110.73198099204856, -111.36708667993291, -110.30840247819665, -110.11744489669044, -110.55237850846444, -108.2073528237766, -112.70750856801911, -110.99917956040802, -109.84949484779976, -111.3403161887679, -110.08924435263565, -110.17749213365616, -112.10849123224503, -110.94270741299202, -109.29350963424746, -110.33477486966507, -112.19620157705627, -111.45484078395934, -111.86858843505124, -110.22491147345858, -108.96177661263177, -108.67862820579893, -107.55155410582937, -108.27984439169573, -108.72682528077233, -110.64231212183269, -109.32873093119183, -112.98564364754564, -110.78933114228725, -108.50921025910479, -107.91087245586935, -112.57350030929283, -111.75871577457525, -108.42095298945462, -112.31266064114303, -110.1295657579673, -109.67444664474456, -110.33749884929306, -109.16098218724147, -109.63554874360221, -109.15892392675141, -111.90580809179818, -108.81196712336858, -111.42223552606656, -109.90571484965518, -109.99739812086352, -111.64103850263211, -111.31463957090885, -110.61247447444549, -110.20960333715526, -110.1707327818923, -109.70412636554525, -110.97278093107532, -110.24386747740314, -109.81378546061525, -110.83784085086458, -109.77357954318757, -111.22663832948885, -111.14563050139252, -110.87152231402447, -110.34246044319893, -109.97174570657546, -110.23599592972218, -111.08206161770731, -110.0073315341242, -111.11748366902188, -112.04005964728601, -109.81290191679287, -109.68543639040858, -112.01143296194752, -110.13641850530031, -108.19348942447623, -109.7534468948808, -109.36697824644176, -97.56454580435337, -104.97829040517887, -108.1539132982256, -110.048991273122, -107.46172505860011, -110.49269280640675, -109.94209901400029, -109.38576869679022, -111.43699124347364, -110.89973083498887, -111.2994445418276, -109.25144782032437, -113.25676258473536, -110.82078737428088, -109.97779571182073, -113.36294799183014, -111.38584551238931, -112.17267897274873, -108.56430946159155, -112.06841286528645, -110.36822473102735, -109.54758527532016, -110.48190506674653, -110.03535695860182, -109.3951469796576, -112.41910682256774, -111.38124138857238, -109.37850389100952, -111.65544568836181, -111.55876881606889, -109.3029209617236, -109.20030046194076, -108.82610577621037, -110.53329453526098, -109.96090595542142, -109.67834229432077, -110.62303603007352, -109.8388817181171, -109.22430039793213, -108.92749786663613, -110.05794249283548, -109.58534943218437, -110.50493887507297, -109.96373022997366, -111.0645036323456, -111.28501675364454, -109.77386932343008, -108.8952247140968, -110.09242801628717, -112.90943444063141, -110.72299296247249, -109.39094335967056, -110.95165384057718, -109.59809519359453, -110.4978602309597, -109.67109981692639, -111.2489619905986, -110.0937750887109, -109.76771021128954, -108.32976315018955, -111.3058145792439, -111.09464974601362, -110.99797900696136, -109.174315000222, -109.630351559617, -110.26289147175856, -110.22688407202517, -109.96748050100612, -112.13247633583758, -110.59994952890855, -110.93023020153811, -109.22457750926695, -110.26162558926984, -110.09713110375579, -111.73858994918328, -109.78183160058515, -109.7603471824367, -110.96016892586911, -111.23309626937036, -109.83093663960678, -114.05354944347246, -111.58202863059464, -110.42281828744524, -110.9521484732059, -112.5120328206343, -111.614891937737, -109.84428787405484, -111.61119567831453, -110.43095563229411, -111.71833448430398, -110.01132196809407, -109.37558169247951, -109.14091380022785, -110.42663661754088, -110.3598013572826, -109.78207135281417, -109.94058843992468, -109.88210328447205, -108.6217811850147, -107.17834387173707, -110.6447226986756, -111.10704778101115, -111.24396771977769, -110.47849395539598, -110.75150631628034, -109.67662689396347, -109.23145032835053, -108.83780193265358, -109.43468321661163, -102.22521103859944, -106.90009867479111, -108.91580608784525, -109.58671397003187, -110.56692028436989, -108.75103142680105, -111.00795573084157, -110.75039085328763, -109.48222099288613, -111.8621134816908, -110.26507966786443, -108.885924716389, -109.30841399453053, -112.3188631425597, -111.05677697153163, -108.8268571902449, -109.63028152237679, -114.82339015806369, -107.03435216376964, -111.34847692589166, -109.61354114874855, -112.32687758049907, -109.59816404231358, -111.64248480241805, -111.84075757907273, -110.44017657636552, -110.15181635726277, -111.93813663582833, -109.11826378836209, -109.99779889778326, -109.927119030584, -109.4389650887841, -111.52448814187727, -111.38736268499642, -110.51920914917922, -108.64230614681055, -108.90307263595304, -110.57246891832371, -109.65575340646116, -109.80359672370373, -108.83368585528197, -111.09385004343437, -108.83430005497769, -112.37784208819113, -109.50005381621696, -109.67421750136593, -111.39664088797532, -109.70867599669316, -109.52498993629875, -111.12341349673187, -110.0484037026941, -109.55138667646308, -111.06614422098669, -109.4785941493091, -110.25724082617013, -110.93950616855716, -110.53487953881397, -111.45722057988401, -110.32393446412904, -110.34361936710438, -108.6610336097813, -109.53631603696368, -108.06930707969195, -107.68056561368934, -108.73860971027449, -108.87111384617579, -108.40433837098611, -110.55999576884835, -106.83832061167207, -108.28786975902513, -109.18482905697472, -107.81071696594883, -107.91047268802457, -108.79613111673706, -111.05361322310213, -109.97897453479862, -109.12920563729425, -111.20538391490288, -109.26286135293664, -111.31400407177502, -109.92167984752287, -110.70854322826071, -108.59406515713611, -109.69371333227458, -109.36664873267313, -110.35521729513704, -110.40667924006368, -112.0181844636846, -111.01529188207431, -110.59246505728431, -109.95068312717868, -110.75807466894047, -109.58596443762707, -111.12127793384956, -109.59041634463125, -111.56255571372793, -110.43405578864342, -108.39660324329928, -111.1420710307505, -113.64788483868595, -111.67645688353934, -111.36878760365944, -109.68523694561108, -110.11608766310304, -109.25670490330123, -110.73546181099229, -111.77855039399805, -107.9662794718261, -109.67483334602832, -109.891258579519, -110.24757768183042, -109.50202895993814, -110.07763831916637, -109.96891925839451, -110.97268925927641, -109.31698133827767, -112.27933593506792, -110.36206721075725, -109.47379463718867, -110.27836850941338, -110.63738280998388, -111.3611682777485, -110.72689155959884, -111.55480904927032, -111.16689658479412, -110.35555645743601, -111.56609319131051, -110.88279459952174, -114.73607246523177, -109.95813757295693, -107.64639932425493, -111.26486783320321, -112.03946356928121, -111.8915972448334, -110.35245920812773, -110.83155104803564, -110.67437747473863, -110.9959682920065, -110.7815352345103, -111.13722283763049, -112.54797265493127, -110.06894780898469, -111.65186554925783, -111.83545188116254, -110.65894756123697, -108.48458025065264, -112.43760714427981, -114.1368408201927, -110.40065777895025, -110.1066998945526, -108.60654239598591, -110.5716060205154, -110.74257357180736, -111.1136089342442, -111.53539811075092, -113.2559601458872, -109.2003227548348, -110.42285840441025, -111.4086884998834, -111.61503050693868, -110.8194303494779, -108.9701587059964, -112.58521089509063, -110.10873915265242, -112.43440038319561, -110.03468788439882, -111.57896603236308, -110.21939233582523, -109.03614470500777, -110.11738923539659, -109.55359574898291, -110.416473622654, -109.4626868574157, -111.17164025076731, -110.3579689035081, -109.04338716157822, -112.36157114517567, -109.32125615922843, -112.71105693789394, -110.11019129547768, -108.96439402555632, -111.107663418839, -111.48306369859839, -110.9317530461794, -107.98628540532181, -111.1636972328743, -110.47837837583148, -109.04649309175733, -110.27110334963734, -111.35803630614352, -110.77259078859605, -111.46352820533895, -111.16789261049541, -109.2376344776325, -111.6795794983659, -111.74292205167644, -109.40835022991612, -111.02163652600731, -108.79482078001607, -110.6718658416566, -111.08747067599332, -112.15383726791498, -109.47049126158717, -109.061574046483, -111.23993049318979, -111.02521156588335, -109.46012868444186, -110.13918914826291, -112.08180381836377, -110.61929875223015, -111.4424805369965, -111.43420275069585, -109.71347556238717, -110.24726273025648, -109.7860268673935, -109.94126895018422, -111.41948668868926, -108.90555991781676, -110.81242861886172, -109.65007052722677, -112.12672329335953, -110.01123170946096, -111.13980448279096, -113.92013682657084, -108.6000853867411, -110.66793592761913, -110.61237681642844, -110.00839105230496, -109.38083187034974, -109.46119372195675, -110.3708067287448, -108.55518656223285, -113.33935987443276, -111.92184778392033, -111.80820718236087, -107.36852757311246, -109.51077803361602, -110.066791721019, -108.756710558672, -107.91391289865918, -110.72851430959301, -111.39074956442978, -112.928843679455, -109.87348280521556, -112.21371750380071, -110.82495902297394, -109.94006136010094, -110.58757785050143, -110.2790091349881, -111.43884888223081, -108.09540986530712, -109.63783244641691, -110.19577975613292, -110.01690033746098, -112.75938920157155, -109.27158857362184, -111.19519821680541, -110.14381902425255, -110.45955291199236, -111.55660330002316, -110.75604254261134, -111.02122553784838, -111.6490091060193, -110.93362819419399, -110.49033159684308, -110.70789549836027, -110.41991882034145, -110.0264093421208, -109.18432746063652, -110.15292268755287, -112.40733942236504, -111.32869665965416, -110.95418667871114, -111.14291568823575, -111.75555369152653, -112.98146297069803, -109.73870744292117, -111.33806139459435, -110.18838799491355, -112.60408243005732, -110.26112648646833, -110.58257045107274, -109.75155437454112]}, ...(2 in all)]
  in  "FFT 1 Choice 1":u16(ring) items=["T1 Y", "T1 X", "T1 Sum", "T2 Y", "T2 X", "T2 Sum", "T1 FB X", "T1 FB Sum", "T2 FB X", "T2 FB Sum", "PSD Y", "PSD X", "PSD Y Sum", "none"]
  in  "FFT 2 Choice 1":u16(ring)=3 items=["T1 Y", "T1 X", "T1 Sum", "T2 Y", "T2 X", "T2 Sum", "T1 FB X", "T1 FB Sum", "T2 FB X", "T2 FB Sum", "PSD Y", "PSD X", "PSD Y Sum", "none"]
  in  "FFT 1 Choice 2":u16(ring)=1 items=["T1 Y", "T1 X", "T1 Sum", "T2 Y", "T2 X", "T2 Sum", "T1 FB X", "T1 FB Sum", "T2 FB X", "T2 FB Sum", "PSD Y", "PSD X", "PSD Y Sum", "none"]
  in  "FFT 2 Choice 2":u16(ring)=4 items=["T1 Y", "T1 X", "T1 Sum", "T2 Y", "T2 X", "T2 Sum", "T1 FB X", "T1 FB Sum", "T2 FB X", "T2 FB Sum", "PSD Y", "PSD X", "PSD Y Sum", "none"]
  in  "Compute FFT":bool
  in  "Reset FFT":bool
  in  "# Spectra to Ave.":dbl=25.0
  out "Ave. Time (s)":dbl=1.5
  out "1 Channel":waveform(dbl)(graph)={"t0"=timestamp(0 s since 1904-01-01), "dt"=1.4999999999999999e-05, "Y"=array[20000 elements], "attributes"=variant("NI_ChannelName"=variant(string "T1 Y"))}
  out "Slow mean":dbl=nan format="%0.2f"
  in  "Slow mean N ave.":dbl=1.0 min=1.0 step=1.0
  out "Mean Intensity":dbl=nan
  out "Sigma":dbl=nan
  out "Sigma/Mean":dbl=nan
  in  "Subtract mean":bool
  in  "High Res. Display":u16(ring) items=["T1 Y", "T1 X", "T1 Sum", "T2 Y", "T2 X", "T2 Sum", "T1 FB X", "T1 FB Sum", "T2 FB X", "T2 FB Sum", "PSD Y", "PSD X", "PSD Y Sum"]
  out "APD 1 Rate (Hz)":dbl format="%#_3p"
  in  "Tab Control":T4(tab)=enum."Sample Stage"
  out "Stage Moving":bool
  in  "Read Cal":bool
  in  "Confocal Linescan":bool
  in  "Speed (nm/s)":dbl=100.0
  in  "Furthest Withdraw (MHz)":dbl=15.0
  in  "Confocal Image":bool
  in  "Round T1 X":bool caption="Round"
  in  "T1 offset_x (mV)":dbl=nan format="%#_2g"
  in  "T1 kappa_x (pN/nm)":dbl=nan min=0.0 step=0.001 format="%#_2g"
  out "Time (s)":dbl=6.12
  out "Total Time (s)":dbl=60.0
  in  "Start Saving":bool
  in  "Cal sets to save":u32=50 min=1 step=1
  in  "Comment (data description)":string="testing confocal setup"
  out "Calibrating Trap...":bool
  in  "Trap 2 (ON/OFF)":bool=TRUE
  in  "Trap 1 (ON/OFF)":bool=TRUE
  in  "Save Calibration":bool
  in  "N sets to save":u32=200 caption="N Sets"
  in  "Save N Sets":bool
  out "Save file name":path=path "C:/Data/110526/110526_022.dat"
  in  "Save ave N":dbl=500.0 caption="Averaging Factor"
  out "Saving...":bool
  in  "Stop Saving":bool
  out "Progress":u16(slide) scale=0.0..100.0
  out "Manipulating Trap":bool
  out "Buffer Status":dbl(slide) scale=0.0..1.0
  out "Overflow (data lost)":bool
  in  "Reset":bool
  out "Data Rate (Hz)":dbl=66666.66666666667 caption="Trap Data Rate (Hz)" format="%#_3p"
  out "Data Period (s)":dbl=1.4999999999999999e-05 caption="Trap Data Period (s)" format="%#_6p"
  out "Save Data Rate (Hz)":dbl=133.33333333333334 caption="Rate (Hz)" format="%#_6p"
  out "Save Data Period (s)":dbl=0.0075 caption="Period (s)" format="%#_6p"
  in  "T1 alpha_x (nm/V)":dbl=nan step=10.0 format="%#_3g"
  in  "T2 alpha_x (nm/V)":dbl=nan step=10.0 format="%#_3g"
  in  "T2 kappa_x (pN/nm)":dbl=nan min=0.0 step=0.001 format="%#_2g"
  in  "T2 offset_x (mV)":dbl=nan format="%#_2g"
  in  "BD 1 Frequency 2 (MHz)":dbl=80.0 caption="T2 X (MHz)" min=50.0 max=100.0 step=1.0 format="%#_6p"
  in  "Green Laser ON/Interlacing":bool=TRUE
  in  "Round T2 X":bool caption="Round"
  in  "AO1":dbl(slide)=5.0 caption="Confocal Y (V)" min=0.0 max=10.0 step=0.01 scale=0.0..10.0 scale format="%_1f"
  in  "AO2":dbl(slide)=5.0 caption="Confocal X (V)" min=0.0 max=10.0 step=0.01 scale=0.0..10.0 scale format="%_1f"
  in  "Trap Raster Scan":bool
  out "Raster Scanning...":bool
  in  "Trap Delta (MHz)":dbl=41.0
  in  "Trap Intensity\nSetpoints (V)":cluster{"Set 1":dbl, "Set 2":dbl}={"Set 1"=5.2, "Set 2"=6.6}
  in  "Index":dbl=1.0 caption="Save File Index" min=1.0 step=1.0
  in  "BD 1 Frequency 1 (MHz)":dbl=65.0 caption="T1 X (MHz)" min=50.0 max=100.0 step=1.0 format="%#_6p"
  out "Current Position":dbl[](array[numeric])=[4.2944, 4.91027471, 2.9278058] format="%7_7g"
  in  "Position Label 5":string="upper flow spot" caption="5"
  in  "Position 1 Label":string="Top capillary (SA beads)" caption="1"
  in  "Position 2 Label":string="Bottom capillary (AD) beads)" caption="2"
  in  "Position 3 Label":string="lower flow spot (ATP)" caption="3"
  in  "Position 4 Label":string="Dump beads" caption="4"
  out "Pump 3 cont disp":string="Left: ADig beads"
  out "Pump 1 cont disp":string="Right: DNA beads "
  in  "Ch 1 Inject Rate (ul/h)":dbl=50.0
  in  "Pump write delay (ms)":dbl=300.0
  in  "All Pump Parameters":T5={"Pump 1"={"Diameter (mm)"=4.61, "Units"=4.0, "Volume"=100.0, "Rate"=50.0}, "Pump 2"={"Diameter (mm)"=4.61, "Units"=3.0, "Volume"=0.0, "Rate"=0.0}, "Pump 3"={"Diameter (mm)"=4.61, "Units"=4.0, "Volume"=100.0, "Rate"=250.0}}
  in  "Ch 2 Inject Volume (uL)":dbl=100.0
  in  "Pump pause delay (ms)":u32
  in  "Ch 3 Inject Volume (uL)":dbl=100.0
  in  "Ch 3 Inject Rate (ul/h)":dbl=250.0
  in  "Flush Center Ch Volume (uL)":dbl=15.0
  in  "Flush Center Ch Rate (ul/m)":dbl=100.0
  in  "Inject Valve B":bool caption="Inject Pump 2\n(Flush Center)"
  in  "Total Volume\nFlushed (uL)":dbl
  in  "Tab Control 2":T6(tab)=enum."Feedback on Trap Intensity"
  in  "Restart RF":bool
  out "Total Counts (ticks)":u32=600
  in  "Trap ON/OFF X or Y Amp?":bool=TRUE
  in  "Oscillate Set 2":bool
  in  "Trap 1 ON":bool=TRUE
  in  "Number Interlace Sets":u8=3 min=1 max=3
  in  "DIO count 3 (ticks)":u32=200
  in  "DIO count 2 (ticks)":u32=200
  in  "DIO count 1 (ticks)":u32=200
  in  "BD 2 Amplitude 3 (%)":dbl min=0.0 max=75.0 step=1.0
  in  "BD 2 Amplitude 2 (%)":dbl min=0.0 max=75.0 step=1.0
  in  "BD 2 Amplitude 1 (%)":dbl min=0.0 max=75.0 step=1.0
  in  "BD 1 Amplitude 3 (%)":dbl min=0.0 max=75.0 step=1.0
  in  "BD 1 Amplitude 2 (%)":dbl=25.0 min=0.0 max=75.0 step=1.0
  in  "BD 1 Amplitude 1 (%)":dbl=25.0 min=0.0 max=75.0 step=1.0
  in  "BD 2 Frequency 3 (MHz)":dbl=26.0 min=50.0 max=100.0 step=1.0 format="%#_6p"
  in  "BD 1 Frequency 3 (MHz)":dbl=70.0 min=50.0 max=100.0 step=1.0 format="%#_6p"
  in  "BD 2 Frequency 2 (MHz)":dbl=26.0 min=50.0 max=100.0 step=1.0 format="%#_6p"
  in  "BD 2 Frequency 1 (MHz)":dbl=26.0 min=50.0 max=100.0 step=1.0 format="%#_6p"
  in  "Not-Interlacing Set":enum32{"Set 1", "Set 2", "Set 3"}(radio)
  in  "Interlace":bool=TRUE
  in  "Trap 2 ON":bool=TRUE
  in  "Trap 3 ON":bool
  in  "Scan axis 2":bool=TRUE
  in  "Osc. freq. (Hz)":dbl=0.25
  in  "Osc. amp. (MHz)":dbl=2.0 format="%1_3g"
  out "Coords":T7
  in  "Manipulation Scaling":cluster{"Horizontal":dbl, "Vertical":dbl}={"Horizontal"=0.075, "Vertical"=0.01}
  in  "Freq or Amp switch first":bool=TRUE
  in  "Swap F1 and F2":bool
  in  "Freq switch delay":u16
  in  "Amp switch delay":u16=5
  in  "Period":i64=2
  in  "MCL Step Increment (V_int)":dbl=3.0
  out "Time to Finish All (min)":dbl=0.122877 format="%#_2p"
  in  "Scan Speed (nm/s)":dbl=100.0
  in  "Scan Range (nm)":dbl=369.00000000000034
  in  "Step Size (nm)":dbl=1.0
  in  "MCL/AOM Scale Tweak":dbl=1.0
  in  "MCL Step Position Ratio":dbl=0.5
  in  "Move MCL Also?":bool=TRUE
  out "Final sep (nm)":dbl=4587.0
  out "Initial sep (nm)":dbl=4218.0
  out "Save index":dbl=22.0
  out "Final delta (MHz)":dbl=44.0
  out "Initial delta (MHz)":dbl=41.0
  out "Final freq. (MHz)":dbl=50.0
  out "Initial freq. (MHz)":dbl=53.0
  in  "Saved AOD Raster Scan Parameter Sets":T8(array[cluster])=[{"Scan Range AOD (nm) 2"=500.0, "Step Size AOD (nm) 2"=1.0, "Scan Speed AOD (nm/s) 2"=100.0, "Number of scans (AOD) 2"=1, "Label"="offset curve"}, {"Scan Range AOD (nm) 2"=420.0, "Step Size AOD (nm) 2"=1.0, "Scan Speed AOD (nm/s) 2"=100.0, "Number of scans (AOD) 2"=1, "Label"="hp raster check"}, {"Scan Range AOD (nm) 2"=6.8, "Step Size AOD (nm) 2"=0.34, "Scan Speed AOD (nm/s) 2"=0.34, "Number of scans (AOD) 2"=1, "Label"="3.4 kbp - 1 bp steps"}]
  in  "Load parameters":bool
  out "Scan Range (MHz)":dbl=-3.0000000000000027
  in  "Restart DMA? (AOD)":bool=TRUE caption="Restart DMA?"
  out "Incr. int (AOD)":i64=-7759651845
  out "Time/Scan (s) (AOD)":dbl=3.68631 format="%#_2p"
  out "Data points/scans":dbl=491508.0
  out "Data points/scan (f/b)":dbl=491508.0
  in  "Save scans":bool=TRUE
  out "AOD Scan I":u64 caption="Scan I"
  in  "Continuous AOD Scanning":bool caption="Continuous Scanning"
  in  "Abort AOD Scan":bool caption="Abort Scan"
  in  "Scan BD":bool=TRUE
  out "Cycles/step (AOD)":u64=666 format="%.3p"
  in  "Number of F/B Scans (AOD)":u16=1 min=1
  out "Scan steps (AOD)":u64=369
  out "Scan Increment (MHz)":dbl=-0.008152173913043485
  out "AOD Scanning":bool caption="Scanning"
  in  "Start AOD Scan":bool caption="Start Scan"
  out "N sets should be saved":dbl=24.5754
  out "Progress 2":u16(slide) caption="Progress" scale=0.0..100.0
  in  "Abort save 2":bool caption="Abort save"
  in  "Trap 1 Bead Size (nm)":dbl=880.0
  in  "Trap 2 Bead Size (nm)":dbl=900.0
  out "MCL Count":dbl=230502201.82069838
  in  "All FB On/Off":bool
  in  "AI2 to Setpoint":cluster{"Set 1":bool, "Set 2":bool}
  out "AI2 (V)":cluster{"Set 1":dbl, "Set 2":dbl}={"Set 1"=-0.0012207403790398877, "Set 2"=0.004577776421399579}
  in  "Reset Feedback":cluster{"Set 1":bool, "Set 2":bool}
  in  "PID Gains":T9={"Set 1"={"proportional gain (Kc)"=0, "integral gain (Kc*Ts/Ti)"=5, "derivative gain (Kc*Td/Ts)"=0}, "Set 2"={"proportional gain (Kc)"=0, "integral gain (Kc*Ts/Ti)"=5, "derivative gain (Kc*Td/Ts)"=0}}
  in  "Feedback On/Off":cluster{"Set 1":bool, "Set 2":bool}={"Set 1"=TRUE, "Set 2"=TRUE}
  in  "Set SP to Reading":bool
  out "Trap X (AI1)":T10={"Trap 1"=-1.0, "Trap 2"=0.899993896484375}
  in  "Trap Pos FB SP":fxp<+/-,16,1>=-0.092803955078125 caption="Setpoint"
  in  "Trap Pos. FB ON":bool
  in  "Reset Trap Pos. FB":bool
  out "Trap Positions":waveform(dbl)[](graph)=[{"t0"=timestamp(12.90000000000001 s since 1904-01-01), "dt"=0.15, "Y"=[-1.7479351299698465e-12, -1.7479351299698465e-12], "attributes"=variant("NI_ChannelName"=variant(string "Trap 1 Pos."))}, {"t0"=timestamp(12.90000000000001 s since 1904-01-01), "dt"=0.15, "Y"=[6.991740519879386e-12, 6.991740519879386e-12], "attributes"=variant("NI_ChannelName"=variant(string "Trap 2 Pos."))}]
  in  "Tab Control 8":enum32{"Main Setting", "Details"}(tab)
  in  "Trap Pos FB Int Count":u16=100
  in  "Trap Pos. FB Gains":T11={"proportional gain (Kc)"=10.0, "integral gain (Kc*Ts/Ti)"=10.0, "derivative gain (Kc*Td/Ts)"=0.0} {"proportional gain (Kc)" format="%.11g"; "integral gain (Kc*Ts/Ti)" format="%.11g"; "derivative gain (Kc*Td/Ts)" format="%.11g"}
  in  "Trap Pos. FB Offset Factor":i64
  in  "Trap Pos FB Negate Action":bool
  in  "Trap Pos. FB Mult Factor":i64=33554432
  in  "Trap Pos. AI1 X Pre-scale":u16
  in  "Trap Pos. FB Range":T12={"output high"=0.999969482421875, "output low"=-1.0}
  out "Trap Pos FB Int Signal":fxp<+/-,24,9> format="%.18g"
  out "Trap Pos FB Int-Norm Signal":fxp<+/-,16,1> format="%.16g"
  in  "Set SP Using...":bool
  in  "Trap Pos FB Monitor\nT1 or T2":bool
  out "Trap X AI1 (DMA)":T13={"Set 1"=0.999969482421875, "Set 2"=0.999969482421875}
  in  "N El. to Ave.":dbl=10000.0
  out "Trap Pos FB Action":i64
  out "Action (%)":dbl(knob) scale=-100.0..100.0
  in  "Trap Pos. FB Out Scale 2^n":u8=23 caption="Action Scale"
  out "Mean T1 Position (nm)":dbl=-1.7479351299698465e-12 caption="Mean T1 (nm)" format="%0.2f"
  out "Trap 1 Position RMS (A)":dbl caption="RMS (Ang)"
  in  "Tab Control 3":enum32{"Timing", "MCL Scan", "Analog Out"}(tab)
  out "APD 2 Gate Late Counter":u32
  out "APD 2 Gate Relative Phase":i16
  in  "Phase Adj. (APD 2 Gate)":i16=20
  in  "Initial Phase Adjustment (APD 2 Gate)":i16=55
  out "APD 1 Gate Late Counter":u32
  in  "- phase (APD 1 Gate)":bool
  in  "+ phase (APD 1 Gate)":bool
  out "APD 1 Gate Relative Phase":i16
  in  "Phase Adj. (APD 1 Gate)":i16=20
  in  "Initial Phase Adjustment (APD 1 Gate)":i16=60
  in  "Save APD Data\nwith Trap Data":bool=TRUE
  out "APD FIFO Elements Remaining":u32
  in  "- phase (APD Acq)":bool
  in  "+ phase (APD Acq)":bool
  out "APD Acq Late Counter":u32
  out "APD Acq Relative Phase":i16
  in  "Phase Adj. (APD Acq)":i16=20
  in  "Initial Phase Adjustment (APD Acq)":i16
  in  "Invert APD Gate":bool caption="Invert Gate"
  in  "APD Gate OFF Count":u32=450 caption="Gate OFF Count"
  in  "APD Gate ON Count":u32=150 caption="Gate ON Count"
  in  "APD Gate":enum32{"ON", "OFF", "Interlace"}(radio)=enum."Interlace"
  in  "APD Integration Time (s)":dbl=0.01 caption="Integration Time (s)"
  out "APD Acq Rate (Hz)":dbl=100.0 caption="Rate (Hz)"
  out "APD Samples/FIFO Acq.":dbl=30.0
  out "APD Elements/DMA read":u32=60
  out "APD Int. Count":u32=400000 format="%.0p"
  in  "+ phase (APD 2 Gate)":bool
  in  "- phase (APD 2 Gate)":bool
  in  "Tab Control 5":enum32{"PSD X", "PSD Y", "Other Data Channel"}(tab)
  out "Data map":dbl[][](graph)
  in  "Channel":i32=4
  in  "Abort MCL Scan":bool
  out "MCL Scan I":u64
  out "MCL Scanning":bool
  in  "Start MCL Scan":bool
  out "wait to reset values":bool
  in  "Tab Control 4":enum32{"Scan Settings", "MCL FPGA Loop Timing"}(tab)
  out "Total Time (s)":dbl=48.0
  in  "Scan lines (y)":u64=20
  in  "Fast Scan Dir":bool=TRUE
  in  "2D or 1D Scan":bool=TRUE
  out "Initial X":dbl
  out "Initial Y":dbl
  out "Time/f+b scan (s) (MCL)":dbl=2.4 caption="Time/scan (s)"
  in  "Number of scans (MCL)":u64=1 caption="Scans"
  in  "Scan steps (MCL)":u64=40 caption="Scan steps (x)"
  in  "N APD Samp/step":dbl=3.0
  in  "Scan Range (V)\n(of steps)":dbl=3.5
  in  "Restart DMA? (MCL)":bool=TRUE caption="Restart DMA?"
  in  "Continuous MCL Scanning":bool caption="Cont. Scanning"
  in  "Center Scan":bool=TRUE
  in  "Save Data (MCL)":bool=TRUE caption="Save Data"
  out "Actual Incr. int (MCL)":i16=294 caption="Incr. int"
  out "Desired incr (int)":dbl=294.0628205128205
  out "Desired Scan Incr (V)":dbl=0.08974358974358974
  out "N sets should be saved (MCL)":dbl=160.0 caption="N sets should be saved"
  out "Data points/scans (MCL)":dbl=4800.0 caption="Data points/scans"
  out "Data points/scan (f+b)":dbl=240.0 caption="points/scan (f+b)"
  out "Cycles/step (MCL)":u64=2000 caption="Cycles/step" format="%.0p"
  out "Actual MCL Inc (V)":dbl=0.08972441785943175
  in  "Phase adjust (MCL)":i16 caption="Phase adjust"
  out "Relative Phase (MCL)":i16 caption="Relative Phase"
  in  "Initial Phase Adj. (MCL)":i16 caption="Initial Phase Adj."
  in  "Update Count (MCL)":u32=600
  in  "+ phase (MCL)":bool
  in  "- phase (MCL)":bool
  out "MCL Late Counter":u32
  in  "APD 1 AO Mult.":i16=1 min=1
  in  "APD 2 AO Mult.":i16=1 min=1
  in  "Tab Control 7":enum32{"Green FB Signals", "Slow MCL Scan"}(tab)
  out "Green FB Plot":dbl(graph)=10.0
  out "MCL Scan 2":cluster{"Begin (V)":dbl, dbl, dbl[]}(graph)
  out "MCL Scan":cluster{"Begin (V)":dbl, dbl, dbl[]}(graph)
  in  "Green laser mode":enum32{"Laser ON", "Laser OFF", "Interlace"}(radio)
  in  "GI Frequency, ON count":u32=150 min=1 step=1
  in  "Invert GI":bool
  out "GI Late Counter":u32
  in  "Phase adj. (GI)":i16=5
  out "GI relative phase":i16
  in  "+ phase (GI)":bool
  in  "Initial Phase Adjustment (GI)":i16=19
  in  "GI Frequency, OFF count":u32=450 min=1 step=1
  in  "- phase (GI)":bool
  out "Green FB Signals (V)":cluster{"Y":dbl, "X":dbl, "Sum":dbl}={"Y"=1.0, "X"=1.0, "Sum"=10.0}
  out "Relative phase (Green FB)":i16
  in  "+ phase (Green FB)":bool
  in  "- phase (Green FB)":bool
  in  "Green FB Count":u32=600
  in  "Phase adj. (Green FB)":i16=10
  in  "Initial Phase Adjustment (Green FB)":i16=50
  in  "Green FB On/Off":bool
  in  "Current When FB OFF (%)":dbl=10.0 min=0.0 max=100.0 step=1.0
  in  "Green int current ON count adj":u32=150
  in  "Green FB Gains":T14={"proportional gain (Kc)"=10, "integral gain (Kc*Ts/Ti)"=5, "derivative gain (Kc*Td/Ts)"=0}
  in  "Green FB Setpoint (mV)":dbl=100.0
  in  "- phase (GI) 2":bool
  in  "Initial Phase Adjustment (GI) 2":i16=-100
  in  "+ phase (GI) 2":bool
  out "GI relative phase 2":i16
  in  "Phase adj. (GI) 2":i16=20
  out "GI Late Counter 2":u32
  in  "Trap Position FIFO Depth":u32=300000 format="%.0p"
  in  "# Samples/trap":u32=20000 format="%.0p"
  out "Trap AI Elements/DMA read":u32=320000 format="%.0p"
  out "Ave. Rate (Hz)":dbl=200000.0 format="%#_6p"
  out "Trap AI FIFO El. Rem.":u32 format="%.0p"
  in  "Phase adj. (AI1)":i16
  out "Relative phase (AI1)":i16
  in  "+ phase (AI1)":bool
  in  "- phase (AI1)":bool
  out "Late Counter (AI1)":u32
  in  "Initial Phase Adjustment (AI1)":i16=180
  out "AI rate (Hz)":dbl=200000.0 format="%#_6p"
  in  "AI Count (ticks)":u32=200
  out "# Samples/channel":u32=40000 format="%.0p"
  in  "Trap AI FIFO Depth":u32=340000 format="%.0p"
  in  "Detector Type":string(combo)="UCB Fleezers 052511"
  in  "N Acq Sets (Traps + Fl.)":i16=3
  in  "Sets to FIFO (Traps)":T15={"Set 1"=TRUE, "Set 2"=TRUE, "Set 3"=FALSE}
  in  "FPGA Ave.":dbl=1.0 min=1.0 step=1.0
  out "Ave. Period (s)":dbl=5e-06 format="%#_6p"
  out "DMA Update Period (s)":dbl=0.3
  out "FPGA Averaging":bool
  out "Trap Sets":u32=2
  out "Counts/DMA":dbl=12000000.0 format="%#_6p"
  out "Trap Pos FIFO El Remaining":u32=141
  out "Trap Pos Elements/DMA read":u32=120000 format="%.0p"
  out "Trap AI FIFO Timeout":u16
  out "Trap Pos FIFO Timeout":u16
  out "Waveform Chart":i32(graph)=320000
  out "error out 2":errorcluster
  in  "Lost Tether Alarm Threshold (pN)":dbl=0.5
  in  "AOM X Cal (nm/MHz)":dbl=123.0
  in  "MCL X Cal (nm/V)":dbl=1070.0
  out "X RF Amplitude Limits (%)":T16={"Minimum"=0.0, "Maximum"=50.0, "Increment"=1.0}
  out "X RF Frequency Limits (MHz)":T16={"Minimum"=50.0, "Maximum"=100.0, "Increment"=1.0}
  out "Y RF Frequency Limits (MHz)":T16={"Minimum"=50.0, "Maximum"=100.0, "Increment"=1.0}
  out "Y RF Amplitude Limits (%)":T16={"Minimum"=0.0, "Maximum"=50.0, "Increment"=1.0}
  in  "Manip. X?":bool=TRUE
  in  "Manip. Y?":bool
  in  "Force Manip Abort":bool
  out "Read cal error":errorcluster
  in  "DAQ Delay (ms)":u32=1000
  in  "Start Scan":bool
  in  "Scan axis":bool
  in  "Osc. amp. (V)":dbl=5.0
  in  "Osc. center (V)":dbl=5.0
  in  "Osc. freq. (Hz) 2":dbl=1.0
  in  "MCL Mode":u16(ring) items=["Manual Positioning", "Sinusoidal Wave", "Linear Scan"]
  in  "Begin (V)":dbl
  in  "End (V)":dbl=10.0
  in  "N Points":dbl=20.0
  in  "Delay to Interlace (s)":dbl
  in  "Delayed Interlace Start":bool
  in  "Read Lateness and Rel Phase":bool
  out "Vec Mean of T1 T2":dbl[](array[numeric])=[nan, nan]
  in  "Cal read wait (s)":u32=5
  out "Time tether formed":timestamp=timestamp(3371146929.513132 s since 1904-01-01)
  in  "Chemyx Syringe Pump Serial Port":refnum<visa-resource-name>="ASRL3::INSTR"
  in  "Limit Min (MHz)":dbl=10.0 caption="Min (MHz)"
  in  "Limit Max (MHz)":dbl=16.0 caption="Max (MHz)"
  in  "Limits Enable":bool=TRUE caption="Enable"
  out "AI labels":string[](array[string])=["T1 Y", "T1 X", "T1 Sum", "T2 Y", "T2 X", "T2 Sum", "T1 FB X", "T2 FB Sum", "T2 FB X", "T2 FB Sum", "PSD Y", "PSD X", "PSD Sum"]
  in  "Save Trap Pos. Data":bool=TRUE
  in  "ESP Port":refnum<visa-resource-name>="COM22"
  out "Z Pos Pos":string="0.21899\r\n"
  out "Y Pos":string="0.00713\r\n"
  out "X Pos":string="0.20503\r\n"
  out "error out":errorcluster
  in  "error in":errorcluster
  in  "Locations":i32(listbox)=1
  out "Selected Location":cluster{"x":string, "y":string, "z":string}={"x"="0.19233\r\n", "y"="0.00156\r\n", "z"="0.20615\r\n"}
  in  "Capture":bool
  in  "Save":bool
  in  "Goto Top (F6)":bool
  in  "Goto Exp (F8)":bool
  in  "Goto Bottom (F7)":bool
  in  "Axis 3":string="0.00500\r\n"
  in  "Axis 2":string="0.00500\r\n"
  in  "Axis 1":string="0.00500\r\n"
  in  "Axis 3":string="0.20000\r\n"
  in  "Axis 2":string="0.20000\r\n"
  in  "Axis 1":string="0.20000\r\n"
  in  "Activate Joystick":bool
  # "After"
  # "During"
  # "Trap On?"
  # "BD Flow ON?"
  # "Samp Flow ON?"
  # "1"
  # "2"
  # "Trap Display:"
  # "APD Display:"
  # "originally 10k"
  # "Trap Manipulation"
  # "DAQ"
  # "Data Saving"
  # "F9"
  # "Bead Calibration"
  # "F10"
  # "F4"
  # "Press F12 to move stage\nwith the mouse. F12 to cancel."
  # "F5"
  # "F6"
  # "F7"
  # "F8"
  # "Harvard Pump\n(sample channel for flow exp)"
  # "Chemyx Pump 2"
  # "Units: \n1 = ml/m\n2 = ml/h\n3 = ul/m\n4 = ul/h"
  # "Rate param is ul/h\nVolume param is ul"
  # "X"
  # "Y"
  # "Oscillate Set 2 freq. (debugging)"
  # "BD 1"
  # "BD 2"
  # "AOD Raster Scan"
  # "Approx. trap separations"
  # "X"
  # "Y"
  # "DON'T TURN ON\nUNTIL YOU CLOSE\nTHE LOOP"
  # "FPGA\nreading"
  # "DMA\ntransfer"
  # "APD Gates"
  # "APD 2"
  # "APD 1"
  # "X"
  # "2D"
  # "Y"
  # "1D"
  # "Green Laser Interlacing"
  # "Green FB Measurement"
  # "Digital Gate"
  # "Current Analog Control"
  # "was 87"
  # "originally 600k"
  # "Total AI Rates (NOT rates/trap)"
  # "originally 20k"
  # "(Samples/trap x Trap Sets)"
  # "(Samples/channel x\n8 if averaging (8 channels)\n4 if no averaging)"
  # "Trap 1"
  # "Trap 2"
  # "Flour./Trap 3"
  # "External Video Window"
  # "MCL Position Debugging"
  # "Temporary Control Storage\n(these used to be somewhere else, still want to keep them)"
  # "Y"
  # "X"
  # "Trap Position Difference Limits"
  # "Joystick Control"
  # "Current Location"
  # "Save Positions of Cambers"
  # "Errors detected in determing Current Location"
  # "High Jog Velocity"
  # "Low Jog Velocity"
  # "Select the chamber to go to"
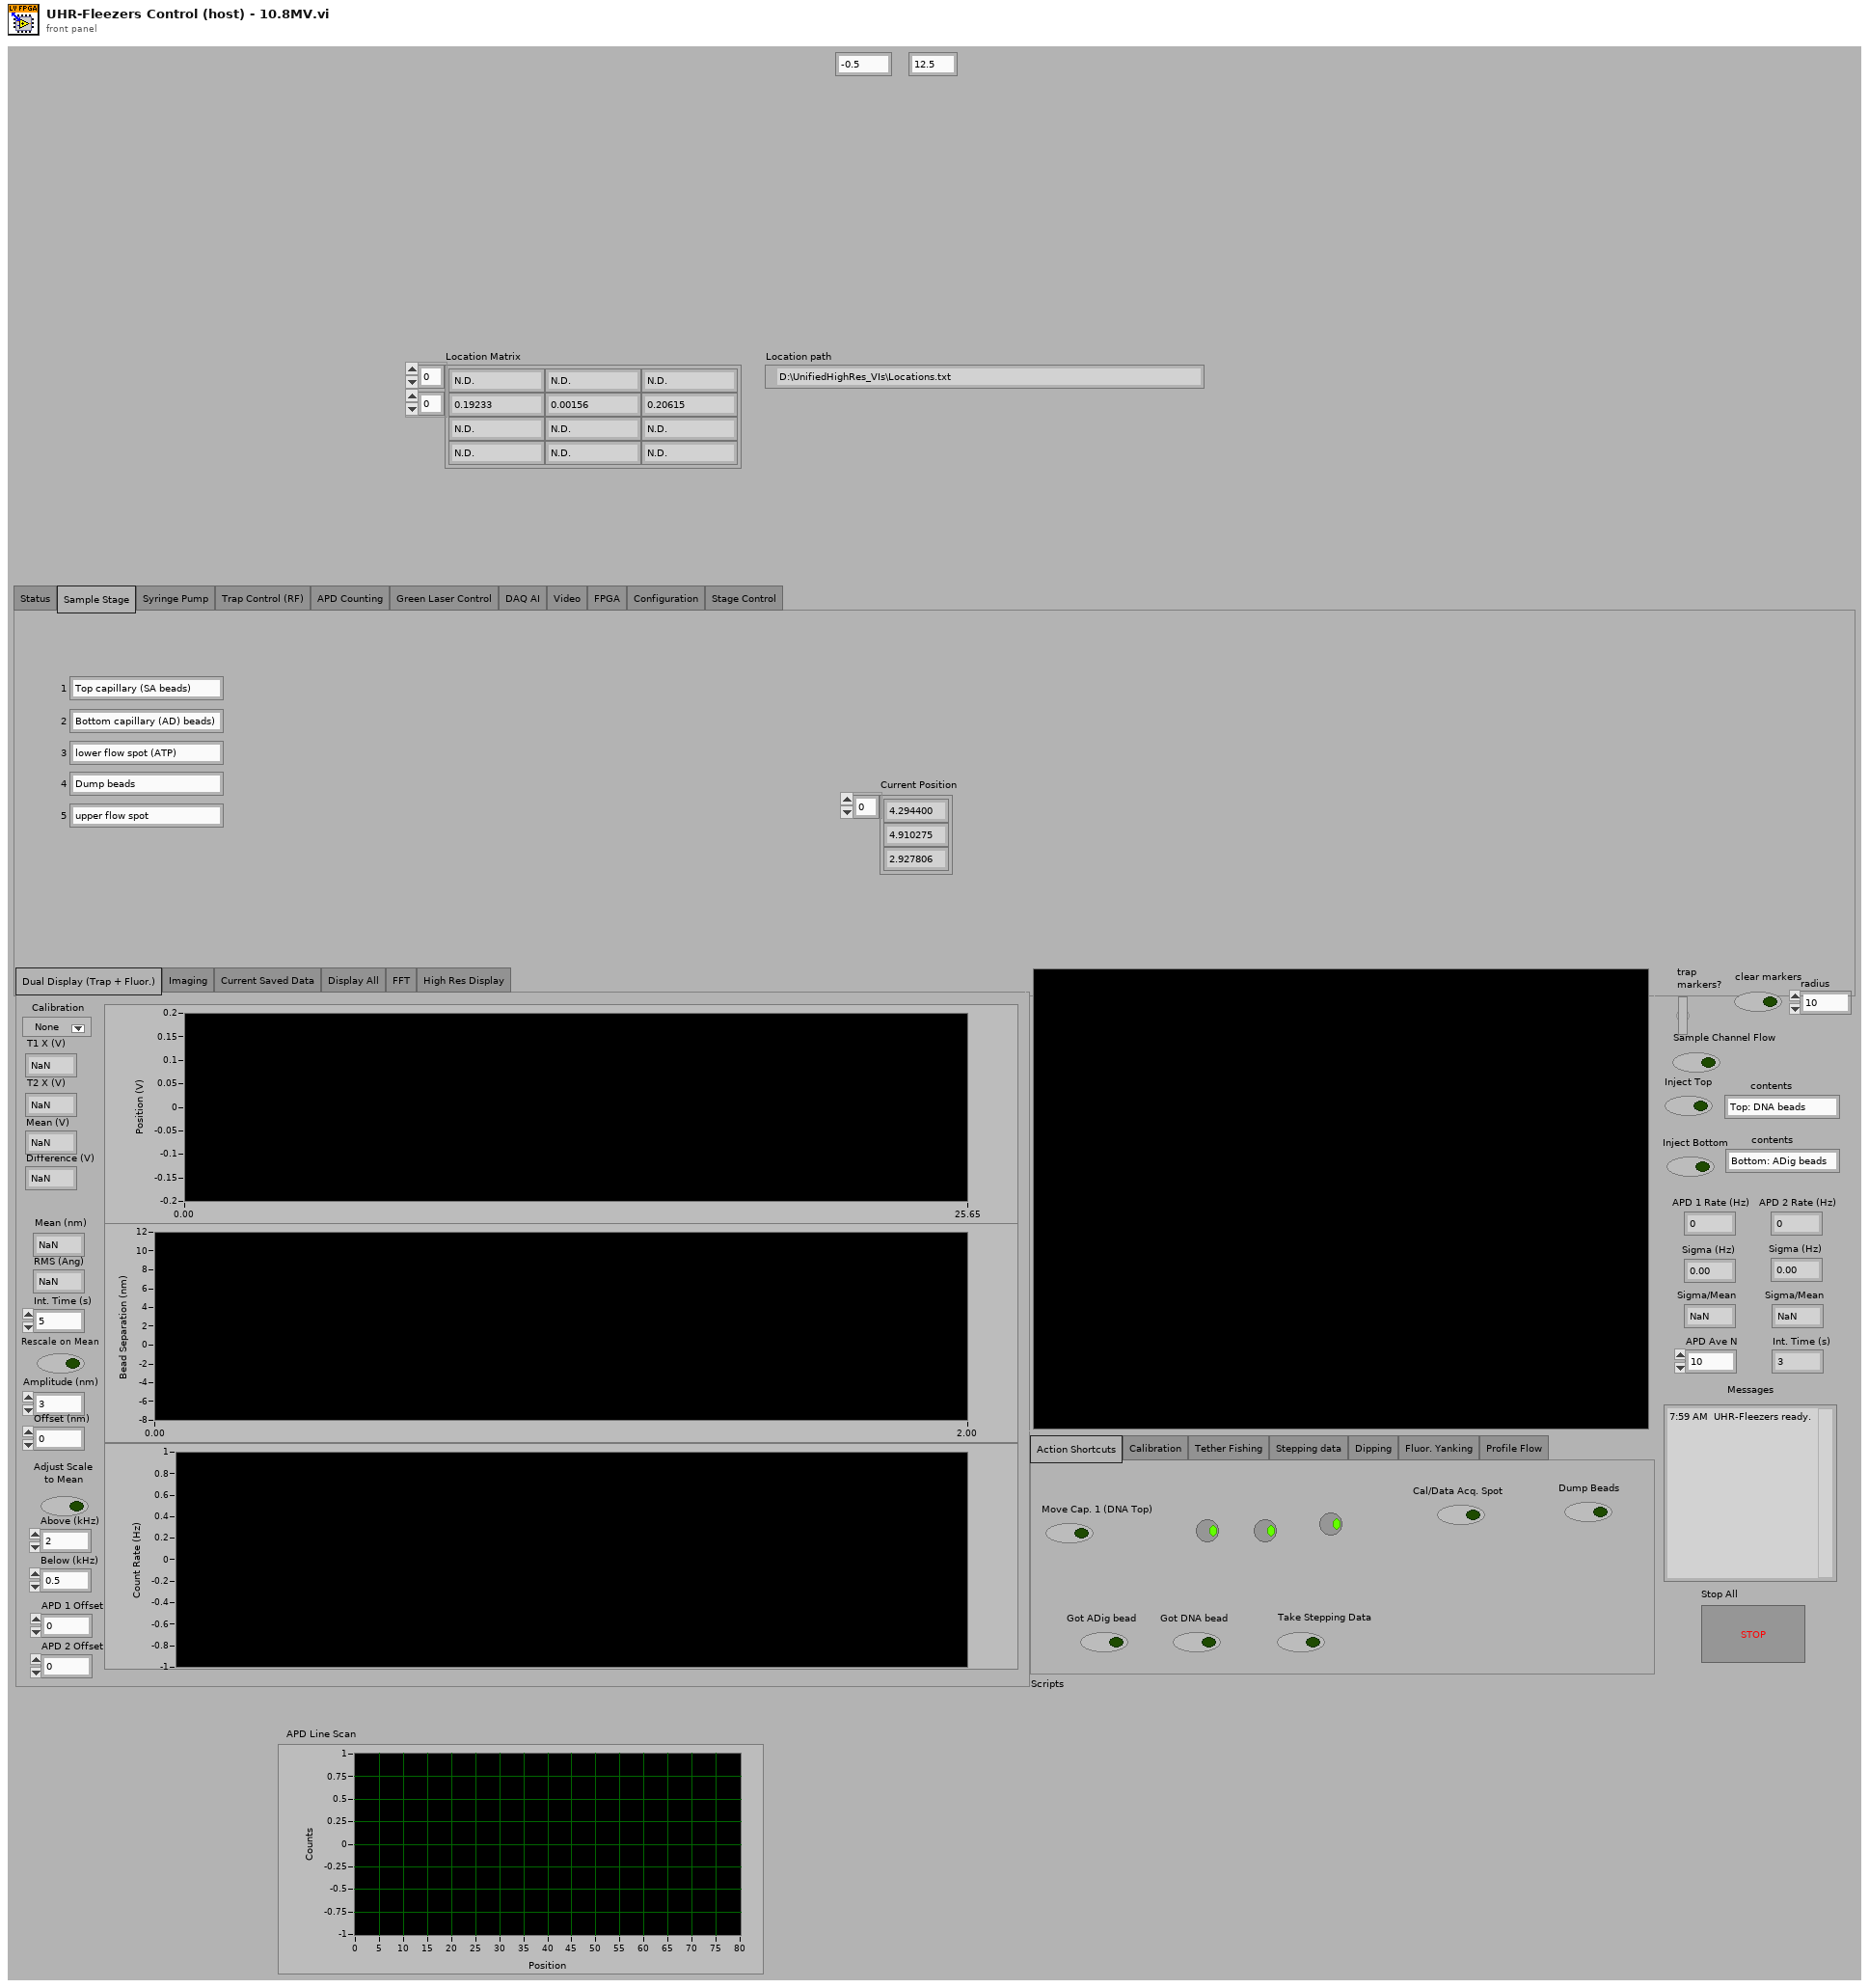
[diagram p1: front panel]
types:
  T1 = enum32{"Action Shortcuts", "Calibration", "Tether Fishing", "Stepping data", "Dipping", "Fluor. Yanking", "Profile Flow"}
  T2 = typedef "IMAQ Image.ctl" = refnum<image>
  T3 = enum32{"Dual Display (Trap + Fluor.)", "Imaging", "Current Saved Data", "Display All", "FFT", "High Res Display"}
  T4 = enum32{"Status", "Sample Stage", "Syringe Pump", "Trap Control (RF)", "APD Counting", "Green Laser Control", "DAQ AI", "Video", "FPGA", "Configuration", "Stage Control"}
  T5 = cluster{"Pump 1":cluster{"Diameter (mm)":dbl, "Units":dbl, "Volume":dbl, "Rate":dbl}, "Pump 2":cluster{"Diameter (mm)":dbl, "Units":dbl, "Volume":dbl, "Rate":dbl}, "Pump 3":cluster{"Diameter (mm)":dbl, "Units":dbl, "Volume":dbl, "Rate":dbl}}
  T6 = enum32{"IR Laser Interlacing (Direct RF Board Control Method)", "AOD Raster Scan", "Feedback on Trap Intensity", "Feedback on Trap Position"}
  T7 = typedef "LVPoint32TypeDef.ctl" = cluster{"Horizontal":i32, "Vertical":i32}
  T8 = cluster{"Scan Range AOD (nm) 2":dbl, "Step Size AOD (nm) 2":dbl, "Scan Speed AOD (nm/s) 2":dbl, "Number of scans (AOD) 2":u16, "Label":string}[]
  T9 = cluster{"Set 1":cluster{"proportional gain (Kc)":i16, "integral gain (Kc*Ts/Ti)":i16, "derivative gain (Kc*Td/Ts)":i16}, "Set 2":cluster{"proportional gain (Kc)":i16, "integral gain (Kc*Ts/Ti)":i16, "derivative gain (Kc*Td/Ts)":i16}}
  T10 = cluster{"Trap 1":fxp<+/-,16,1>, "Trap 2":fxp<+/-,16,1>}
  T11 = cluster{"proportional gain (Kc)":fxp<+/-,16,8>, "integral gain (Kc*Ts/Ti)":fxp<+/-,16,8>, "derivative gain (Kc*Td/Ts)":fxp<+/-,16,8>}
  T12 = cluster{"output high":fxp<+/-,16,1>, "output low":fxp<+/-,16,1>}
  T13 = cluster{"Set 1":fxp<+/-,16,1>, "Set 2":fxp<+/-,16,1>}
  T14 = cluster{"proportional gain (Kc)":i16, "integral gain (Kc*Ts/Ti)":i16, "derivative gain (Kc*Td/Ts)":i16}
  T15 = cluster{"Set 1":bool, "Set 2":bool, "Set 3":bool}
  T16 = typedef "LVMinMaxIncTypeDef.ctl" = cluster{"Minimum":dbl, "Maximum":dbl, "Increment":dbl}
  T17 = typedef "Image Type" = u32
  T18 = typedef "nirio_resource_hc.ctl" = tag
  T19 = typedef "openfpgaref.8.6.ctl" = refnum<k20>
  T20 = enum16{"CONNECT", "INITIALIZE VALVES", "DISCONNECT", "MOVE VALVE"}
  T21 = cluster{"New Image":T2, "New Image":T2, "New Image":T2, "New Image":T2}
  T22 = enum16{"open", "replace", "create", "open or create", "replace or create", "replace or create with confirmation"}
  T23 = typedef "XDNodeRunTimeDep.lvlib/timing_clust.ctl" = cluster{"Expected End [f-1]":u64, "Actual End [f-1]":u64, "Finished Late? [f-1]":bool, "Expected End [i-1]":u64, "Actual End [i-1]":u64, "Finished Late? [i-1]":bool, "Expected Start [i]":u64, "Actual Start [i]":u64, "Expected Start [f]":u64, "Actual Start [f]":u64, "Source Name":string, "Structure Name":string, "Period":i64, "Deadline":i64, "Offset":i64, "Start":i64, "Priority":i32, "Timeout":i32, "Mode":T24, "Wakeup Reason":T25, "Error":errorcluster, "Source Type":string, "Secondary Source Type":string, "Global End Time":u64, "Global Start Time":u64, "Frame Duration":u64, "Iteration Duration":u64, "Assigned CPU":i32, "I/O Scan Engine Mode":u32}
  T24 = typedef "XDNodeRunTimeDep.lvlib/nitl_modes.ctl" = enum32{"No Change", "Process missed periods, maintain original phase", "Discard missed periods, maintain original phase", "Process missed periods, ignore original phase", "Discard missed periods, ignore original phase"}
  T25 = typedef "XDNodeRunTimeDep.lvlib/wakeup.ctl" = enum32{"Normal", "Aborted", "Asynchronous wakeup", "Timing source error", "Timed loop error", "Timeout"}
  T26 = cluster{"[0]":i32, "[1]":i32, "[2]":i32, "[3]":i32}
  T27 = cluster{"[0]":i32, "[1]":i32, "[2]":i32, "[3]":i32}[]
  T28 = cluster{"Location Matrix[0]":string, "Location Matrix[1]":string, "Location Matrix[2]":string}
  T29 = enum16{"big-endian, network order", "native, host order", "little-endian"}
  T30 = cluster{"Scan Range AOD (nm) 2":dbl, "Step Size AOD (nm) 2":dbl, "Scan Speed AOD (nm/s) 2":dbl, "Number of scans (AOD) 2":u16, "Label":string}
  T31 = cluster{"[0]":dbl, "[1]":dbl, "[2]":dbl, "[3]":dbl, "[4]":dbl, "[5]":dbl}
  T32 = cluster{"Diameter (mm)":dbl, "Units":dbl, "Volume":dbl, "Rate":dbl}
  T33 = enum32{"Normal Display", "Dual Display (APD)", "FFT", "High Res Display"}
  T34 = cluster{"Origin Pixel":cluster{"X":sgl, "Y":sgl}, "Angle Relative to Horizontal (deg)":sgl, "Axis Reference":u32}
  T35 = typedef "Simple Grid Descriptor" = cluster{"X Step":sgl, "Y Step":sgl, "Unit":T36}
  T36 = typedef "Image Unit" = enum32{"Undefined", "Angström", "Micrometer", "Millimeter", "Centimeter", "Meter", "Kilometer", "Microinch", "Inch", "Feet", "Nautical miles", "Standard miles", "Steps"}
  T37 = cluster{"averaging mode":u16, "weighting mode":u16, "number of averages":u32}
  T38 = cluster{"dB On (F)":bool, "unwrap phase (F)":bool, "convert to degree (F)":bool}
  T39 = cluster{string, string, string, string, string, string, string, string}
  T40 = cluster{string, string, string, string, string, string, string, string, string, string, string, string}
  T41 = cluster{string, string, string, string, string, string, string, string, string, string, string, string, string}
  T42 = cluster{string, string, string, string, string, string, string, string, string, string, string, string, string, string}
  T43 = cluster{"BD 1 Frequency 1 (MHz)":dbl, "BD 1 Frequency 2 (MHz)":dbl}
  T44 = cluster{"f0":dbl, "df":dbl, "magnitude":dbl[]}[][]
  T45 = cluster{"Green FB Ch 0":i16, "Green FB Ch 1":i16, "Green FB Ch 2":i16}
  T46 = cluster{"Green FB Ch 0":dbl, "Green FB Ch 1":dbl, "Green FB Ch 2":dbl}
  T47 = cluster{"Left":i32, "Top":i32, "Width":u32, "Height":u32}
  T48 = cluster{cluster{"Left":i32, "Top":i32, "Width":u32, "Height":u32}}[]
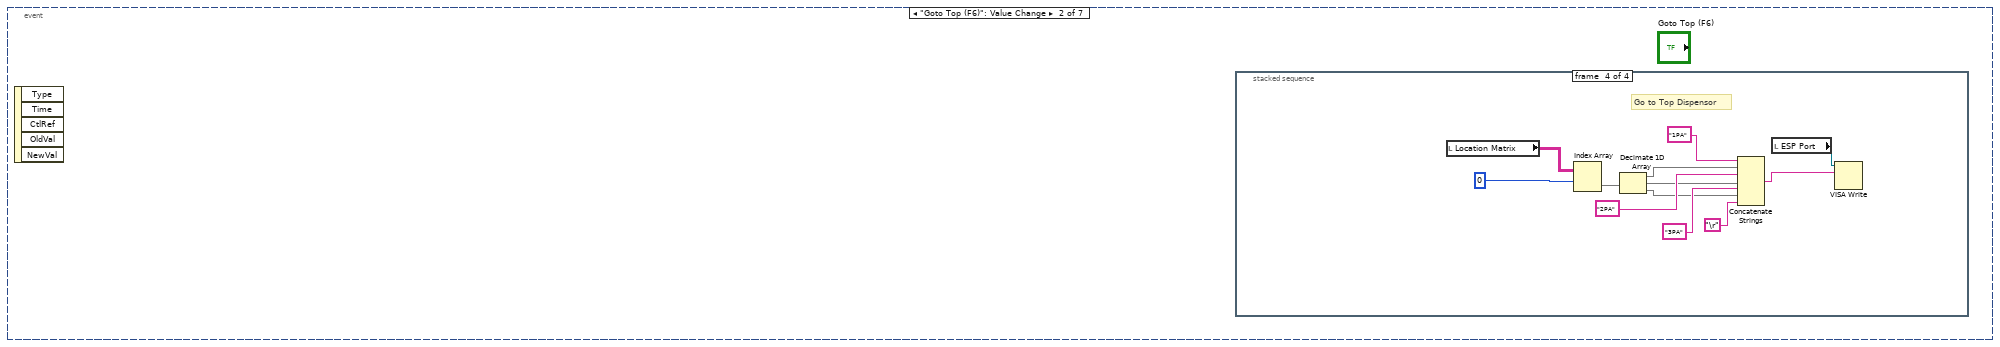
[diagram p3: hidden frame]
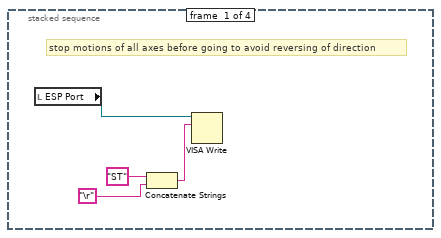
[diagram p4: hidden frame]
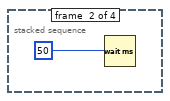
[diagram p5: hidden frame]
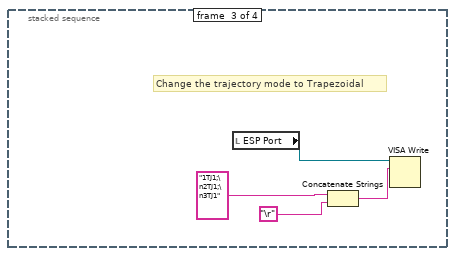
[diagram p6: hidden frame]
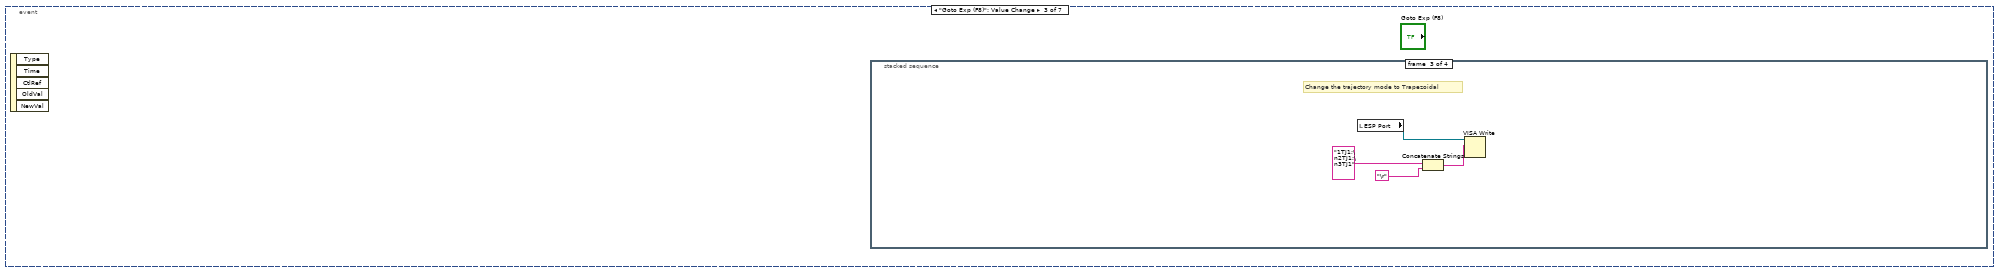
[diagram p7: hidden frame]
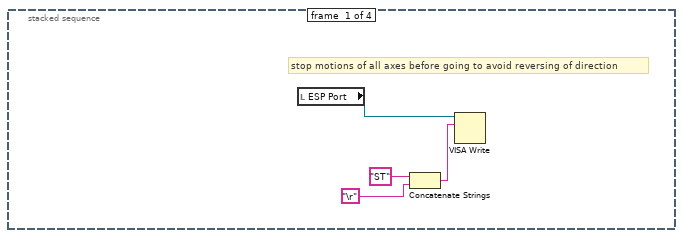
[diagram p8: hidden frame]
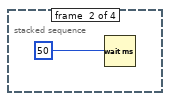
[diagram p9: hidden frame]
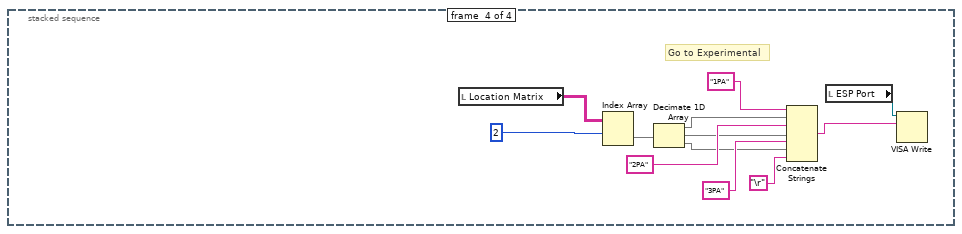
[diagram p10: hidden frame]
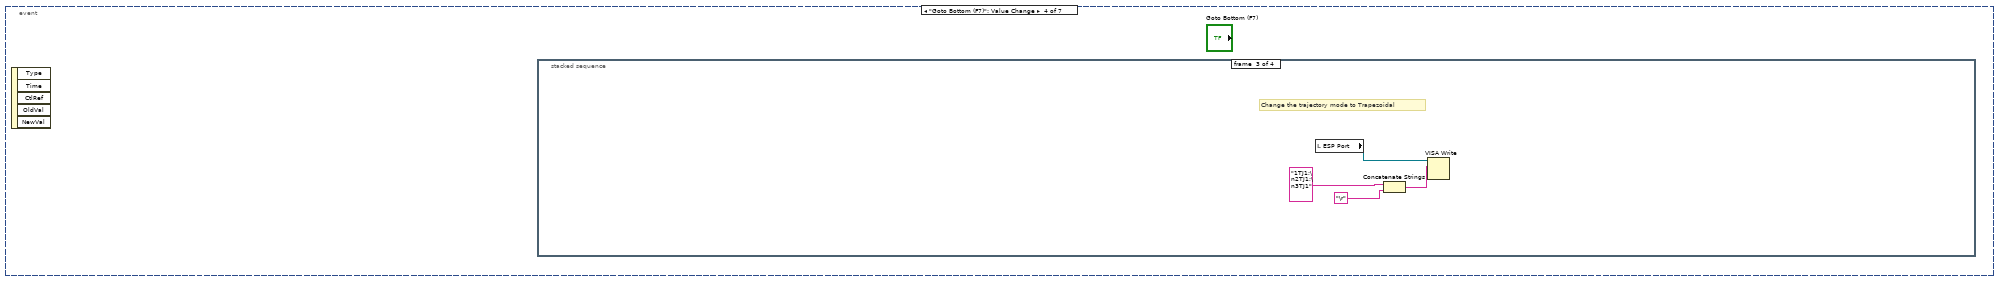
[diagram p11: hidden frame]
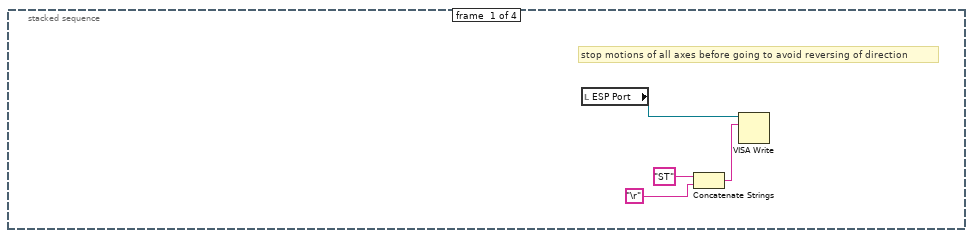
[diagram p12: hidden frame]
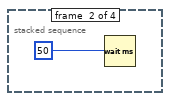
[diagram p13: hidden frame]
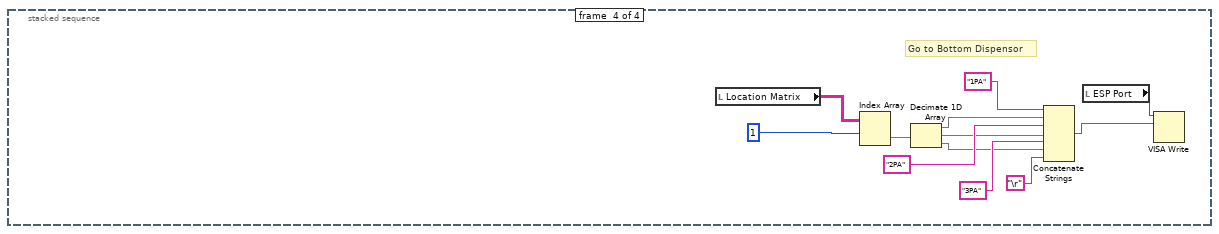
[diagram p14: hidden frame]
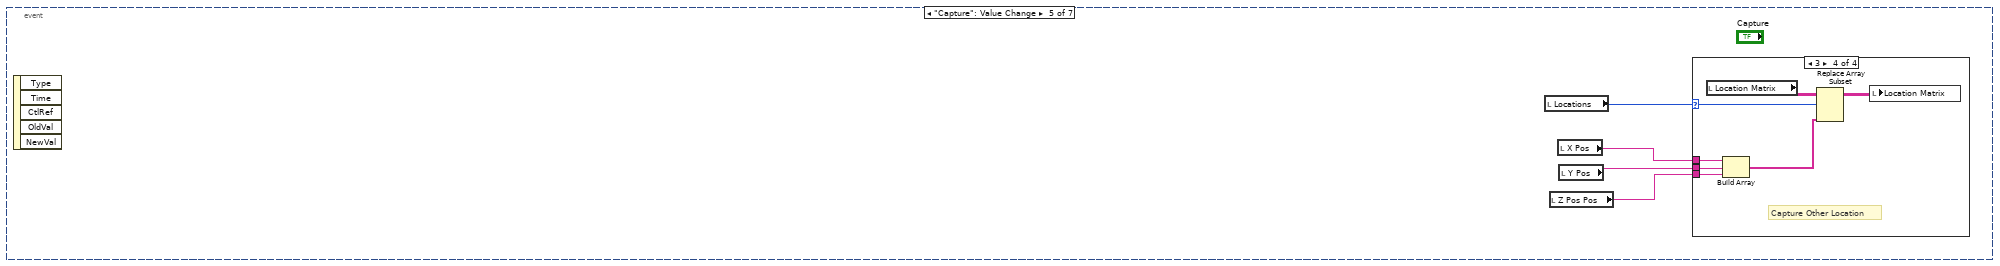
[diagram p15: hidden frame]
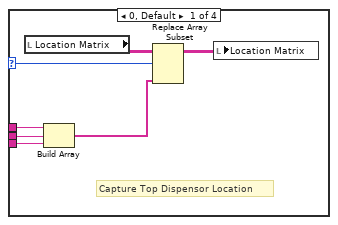
[diagram p16: hidden frame]
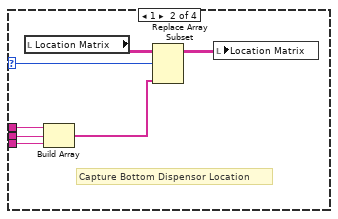
[diagram p17: hidden frame]
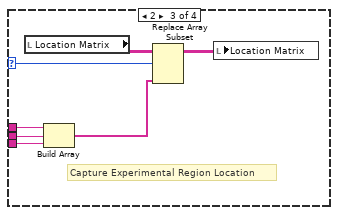
[diagram p18: hidden frame]
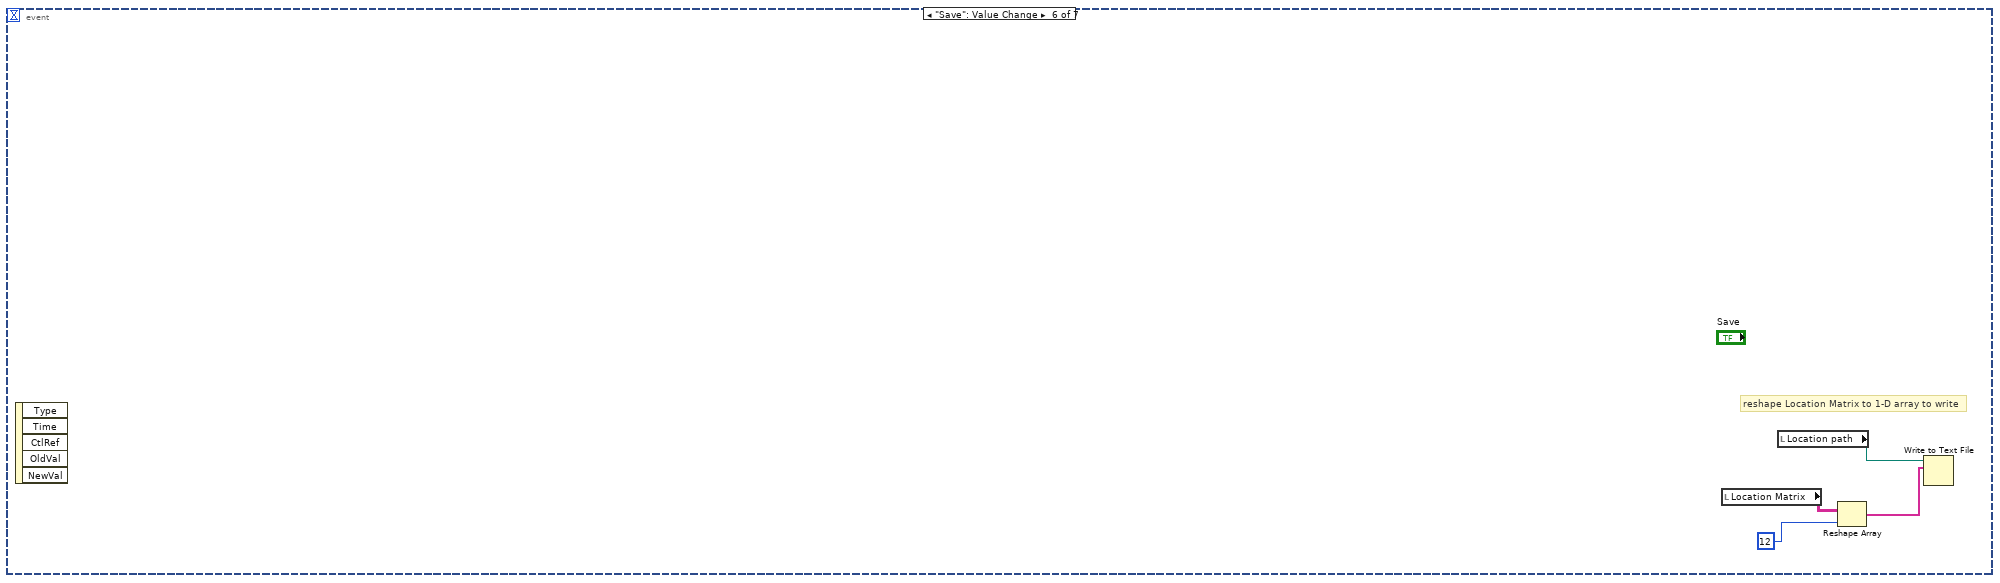
[diagram p19: hidden frame]
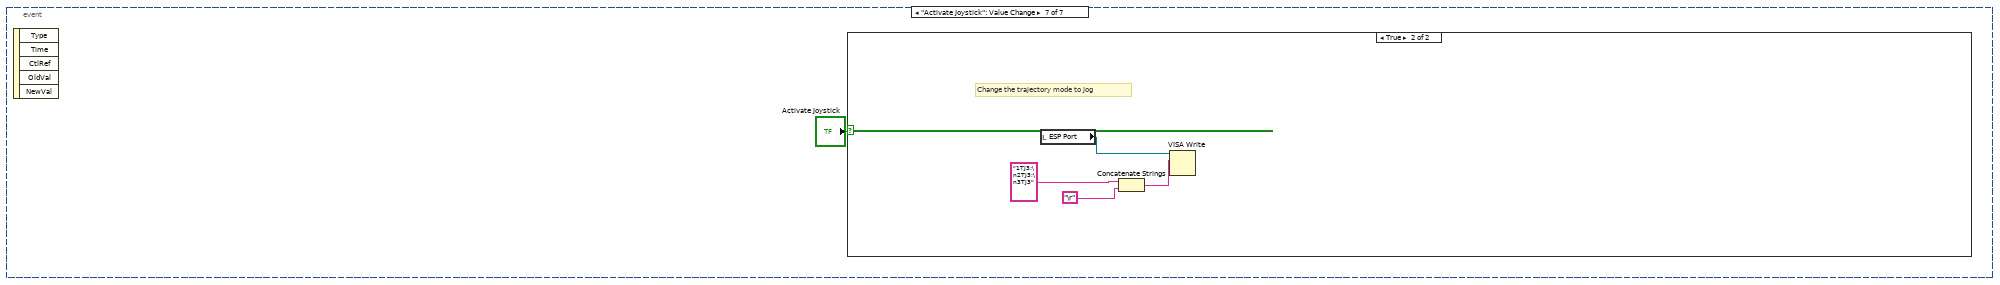
[diagram p20: hidden frame]
diagram:
  w64 = T17 2 items=["Grayscale (U8)", "Grayscale (I16)", "Grayscale (SGL)", "Complex (CSG)", "RGB (U32)", "HSL (U32)", "RGB (U64)", "Grayscale (U16)"] ("Image Type")
  w121 = cluster{"output high":i16, "output low":i16} {"output high"=3000, "output low"=0} ("FB output range 1")
  w196 = 10.0 ("y")
  w195 = 32767.0 ("y")
  w211 = 6.0  # clock mult.
  w212 = 49152000.0  # TCXO frequ.
  # "Initialize location matrix"
  n1 = Build Array("DIO count 1 (ticks)", "DIO count 2 (ticks)", "DIO count 3 (ticks)") -> (w110:u32[])
  n2 = Multiply(x="APD Integration Time (s)", y=40000000.0) -> (x*y=w128:dbl)
  n3 = Reciprocal(x="APD Integration Time (s)") -> (1/x=w125:dbl)
  n4 = local write "APD Acq Rate (Hz)"(w125) -> ()
  n5 = local read "AO1"() -> (w190:dbl)
  n6 = local read "AO2"() -> (w189:dbl)
  n7 = To Unsigned Long Integer(number=w128) -> (unsigned 32bit integer=w127:u32)
  "APD Int. Count" <- w127
  n8 = local read "Scan Increment (MHz)"() -> (w207:dbl)
  n9 = local read "Continuous MCL Scanning"() -> (w177:bool)
  n10 = local read "Fast Scan Dir"() -> (w176:bool)
  n11 = local read "Trap Intensity\nSetpoints (V)"() -> (w226:cluster{"Set 1":dbl, "Set 2":dbl})
  n12 = local read "Number of scans (MCL)"() -> (w178:u64)
  n13 = Multiply(x=w190, y=w195) -> (x*y=w192:dbl)
  n14 = Multiply(x=w189, y=w195) -> (x*y=w194:dbl)
  n15 = Divide(x=w192, y=w196) -> (x/y=w191:dbl)
  n16 = Divide(x=w194, y=w196) -> (x/y=w193:dbl)
  n17 = To Word Integer(number=w191) -> (16bit integer=w188:i16)
  n18 = To Word Integer(number=w193) -> (16bit integer=w187:i16)
  n19 = Not(x=w176) -> (.not. x?=w171:bool)
  n20 = local read "Cycles/step (MCL)"() -> (w179:u64)
  n21 = Multiply(x=w207, y=1000.0) -> (x*y=w214:dbl)
  n22 = local read "Scan steps (MCL)"() -> (w180:u64)
  n23 = local write "Trap Pos FIFO Timeout"(u16 0 ("Trap Pos FIFO Timeout")) -> ()
  n24 = local read "Desired Scan Incr (V)"() -> (w182:dbl)
  n25 = Scale By Power Of 2(n=48, x=w214) -> (x*2^n=w215:dbl)
  n26 = Multiply(x=w212, y=w211) -> (x*y=w210:dbl)
  n27 = Divide(x=w215, y=w210) -> (x/y=w209:dbl)
  n28 = local read "Number Interlace Sets"() -> (w103:u8)
  n29 = Split 1D Array(array=w110, index=w103) -> (first subarray=w112:u32[])  [unwired: 1 out]
  n30 = Add Array Elements(numeric array=w112) -> (sum=w111:u32)
  n31 = property on="AI Count (ticks)" class="DigNum (strict)"("Val(Sgnl)"="AI Count (ticks)") -> ()  [unwired: 2 in, 2 out]
  n32 = local read "# Samples/channel"() -> (w199:u32)
  n33 = local read "Number of F/B Scans (AOD)"() -> (w200:u16)
  n34 = To Quad Integer(1:w209) -> (0:w206:i64)
  n35 = local read "Not-Interlacing Set"() -> (w102:enum32{"Set 1", "Set 2", "Set 3"})
  n36 = To Unsigned Byte Integer(number=w102) -> (unsigned 8bit integer=w108:u8)
  n37 = Index Array(array=w110, index=w108) -> (element=w109:u32)
  n38 = local read "Feedback On/Off"() -> (w229:cluster{"Set 1":bool, "Set 2":bool})
  n39 = local read "PID Gains"() -> (w221:T9)
  n40 = Divide(x=40000000.0, y="AI Count (ticks)") -> (x/y=w168:dbl)
  n41 = Multiply(x=w182, y=32767.0) -> (x*y=w184:dbl)
  n42 = local read "Scan steps (AOD)"() -> (w205:u64)
  n43 = local read "All FB On/Off"() -> (w230:bool)
  n44 = local read "Cycles/step (AOD)"() -> (w204:u64)
  n45 = local write "AI rate (Hz)"(w168) -> ()
  n46 = Divide(x=w184, y=10.0) -> (x/y=w183:dbl)
  n47 = Multiply(x=w205, y=w204) -> (x*y=w203:u64)
  n48 = Multiply(x=3276.7, y=w226) -> (x*y=w225:cluster{"Set 1":dbl, "Set 2":dbl})
  n49 = To Word Integer(number=w183) -> (16bit integer=w181:i16)
  n50 = Multiply(x=w203, y=u64 2) -> (x*y=w201:u64)
  n51 = local read "Sets to FIFO (Traps)"() -> (w233:T15)
  n52 = Divide(x=w168, y="FPGA Ave.") -> (x/y=w169:dbl)
  n53 = To Word Integer(number=w225) -> (16bit integer=w224:cluster{"Set 1":i16, "Set 2":i16})
  n54 = xnode "Open FPGA VI Reference"("resource name"=T18 "750kHzDAQ") -> ("FPGA VI Reference Out"=w218:T19)  [unwired: 1 in, 1 out]
  n55 = Unbundle By Name(w221) -> ("Set 1"=w220:T14, "Set 2"=w219:T14)
  n56 = Multiply(x=w201, y=w200) -> (x*y=w198:u64)
  n57 = local write "Ave. Rate (Hz)"(w169) -> ()
  n58 = Divide(x=w198, y=w199) -> (x/y=w197:dbl)
  n59 = Unbundle By Name(w224) -> ("Set 1"=w223:i16, "Set 2"=w222:i16)
  n60 = local read "2D or 1D Scan"() -> (w122:bool)
  n61 = local write "Data points/scans"(w198) -> ()
  n62 = local read "Scan BD"() -> (w216:bool)
  n63 = And(x=w229, y=w230) -> (x .and. y?=w228:cluster{"Set 1":bool, "Set 2":bool})
  n64 = local write "Data points/scan (f/b)"(w201) -> ()
  n65 = Reciprocal(x=w169) -> (1/x=w170:dbl)
  n66 = local read "N Acq Sets (Traps + Fl.)"() -> (w161:i16)
  n67 = local write "N sets should be saved"(w197) -> ()
  n68 = Unbundle By Name(w228) -> ("Set 1"=w232:bool, "Set 2"=w231:bool)
  n69 = local read "Interlace"() -> (w104:bool)
  n70 = Select(t=w111, s=w104, f=w109) -> (s? t:f=w101:u32)
  n71 = local write "Update Count (MCL)"(w101) -> ()
  n72 = local write "Total Counts (ticks)"(w101) -> ()
  n73 = xnode "Invoke Method"("FPGA VI Reference In"=w218) -> ("FPGA VI Reference Out"=w120:T19, "error out"=w139:errorcluster)  [unwired: 1 in]
  n74 = local write "Ave. Period (s)"(w170) -> ()
  n75 = property on="2D or 1D Scan" class="Bool (strict)"("Val(Sgnl)"=w122) -> ()  [unwired: 2 in, 2 out]
  n76 = xnode "Read/Write Control"("FPGA VI Reference In"=w119, "error in"=w139, "ai count"="AI Count (ticks)", "Interlace ON/OFF"=w104, "Number Interlace Cycles"=w103, "AI1 Sets to FIFO"=w233, "FB On/Off Set 1"=w232, "FB On/Off Set 2"=w231, "Interlace Off Parameters"=w102, "FB Setpoint Set 1"=w223, "FB Setpoint Set 2"=w222, "FB Gains Set 1"=w220, "FB Gains Set 2"=w219, "FB output range 1"=w121, "FB output range 2"=w121, "Cycles per step"=w204, "Scan BD"=w216, "Number of scans"=w200, "Scan steps"=w205, "Scan freq.  increment"=w206, "AO1"=w188, "AO2"=w187, "Scan freq.  increment (MCL)"=w181, "Scan steps (MCL)"=w180, "Cycles per step (MCL)"=w179, "Number of scans (MCL)"=w178, "MCL count"=w101, "Cont. Scan (MCL)"=w177, "MCL Scan Axis"=w171, "1D or 2D Scan?"=w122, "N of AI1 Int Acq Sets"=w161, "Freq or Amp switch first"="Freq or Amp switch first", "Freq switch delay"="Freq switch delay", "Amp switch delay"="Amp switch delay", "Swap F1 and F2"="Swap F1 and F2", "APD Acq Rate Count"=w127, "APD to FIFO"=FALSE, "APD Gate Operating Mode"="APD Gate", "APD Gate ON Count"="APD Gate ON Count", "APD Gate OFF Count"="APD Gate OFF Count", "Invert APD Gate"="Invert APD Gate", "DIO count 1 (ticks)"="DIO count 1 (ticks)", "DIO count 2 (ticks)"="DIO count 2 (ticks)", "DIO count 3 (ticks)"="DIO count 3 (ticks)", "APD 1 AO scale factor"="APD 1 AO Mult.", "APD 2 AO scale factor"="APD 2 AO Mult.") -> ("FPGA VI Reference Out"=w96:T19, "error out"=w98:errorcluster)  [unwired: 1 in]
  n77 = local read "Green Laser ON/Interlacing"() -> (w99:bool)
  n78 = local read "Green laser mode"() -> (w100:enum32{"Laser ON", "Laser OFF", "Interlace"})
  n79 = local read "GI Frequency, OFF count"() -> (w92:u32)
  n80 = local read "GI Frequency, ON count"() -> (w91:u32)
  n81 = Multiply(x="Current When FB OFF (%)", y=655.35) -> (x*y=w82:dbl)
  n82 = local read "Green FB Count"() -> (w90:u32)
  n83 = Multiply(x="Green FB Setpoint (mV)", y=3.2767) -> (x*y=w79:dbl)
  n84 = To Unsigned Word Integer(number=w82) -> (unsigned 16bit integer=w80:u16)
  n85 = local read "Invert GI"() -> (w94:bool)
  n86 = To Word Integer(number=w79) -> (16bit integer=w77:i16)
  n87 = case shown="True" w99 {
    tunnel: w100 -> [_ w253]
    tunnel: [enum32{"Laser ON", "Laser OFF", "Interlace"}."Laser OFF" ("Green laser mode") w253] -> w93
    frame False {
    }
    frame True {
    }
  }
  n88 = local read "Trap Pos. AI1 X Pre-scale"() -> (w48:u16)
  n89 = local read "Trap Pos FB Monitor\nT1 or T2"() -> (w55:bool)
  n90 = local read "Trap Pos FB Int Count"() -> (w43:u16)
  n91 = local read "Trap Pos FB Negate Action"() -> (w54:bool)
  n92 = local read "Trap Pos. FB Offset Factor"() -> (w53:i64)
  n93 = local read "Trap Pos. FB Mult Factor"() -> (w52:i64)
  n94 = local read "Trap Pos. FB Gains"() -> (w50:T11)
  n95 = local read "Trap Pos. FB Range"() -> (w51:T12)
  n96 = xnode "Read/Write Control"("FPGA VI Reference In"=w96, "error in"=w98, "Green interlace ON count 2"=w91, "Green interlace OFF count 2"=w92, "Invert GI 2"=w94, "Operating Mode 2"=w93, "Green FB Gains"="Green FB Gains", "Green FB Setpoint"=w77, "Green FB On/Off"="Green FB On/Off", "Current Out"=w80, "Green int current ON count adj"="Green int current ON count adj", "Green FB Count"=w90, "Operating Mode"=w93, "Green interlace OFF count"=w92, "Green interlace ON count"=w91, "Invert GI"=w94, "Trap Pos FB Monitor T1 or T2"=w55, "Trap Pos FB Negate Action"=w54, "Trap Pos. FB Offset Factor"=w53, "Trap Pos. FB Mult Factor"=w52, "Trap Pos. FB Range"=w51, "Trap Pos. FB Gains"=w50, "Force feedback"=FALSE, "AI1 X Scale"=w48, "Trap Pos to FIFO"=TRUE, "Trap Pos FB Int Count"=w43) -> ("FPGA VI Reference Out"=w95:T19, "error out"=w97:errorcluster)
  n97 = xnode "Invoke Method"("FPGA VI Reference In"=w95, "error in"=w97, "Requested Depth"="Trap AI FIFO Depth") -> ("FPGA VI Reference Out"=w58:T19, "error out"=w57:errorcluster)  [unwired: 1 out]
  n98 = xnode "Invoke Method"("FPGA VI Reference In"=w58, "error in"=w57, "Requested Depth"="Trap Position FIFO Depth") -> ("FPGA VI Reference Out"=w45:T19, "error out"=w44:errorcluster)  [unwired: 1 out]
  n99 = flat-sequence {
    tunnel: w120 -> [w258]
    tunnel: [w258] -> w119
    tunnel: [w257] -> w118
    tunnel: [w256] -> w117
    tunnel: [w254] -> w115
    tunnel: [w255] -> w116
    frame #0 {
      w255 = T16 {"Minimum"=50.0, "Maximum"=100.0, "Increment"=1.0} ("Min Max Inc")
      w254 = T16 {"Minimum"=0.0, "Maximum"=75.0, "Increment"=1.0} ("Data Entry Limits")
      w257 = T16 {"Minimum"=50.0, "Maximum"=100.0, "Increment"=1.0} ("Min Max Inc")
      w256 = T16 {"Minimum"=0.0, "Maximum"=75.0, "Increment"=1.0} ("Data Entry Limits")
      n100 = property on="BD 2 Frequency 1 (MHz)" class="DigNum (strict)"("Data Range"=w255) -> ()  [unwired: 2 in, 2 out]
      n101 = property on="BD 2 Frequency 3 (MHz)" class="DigNum (strict)"("Data Range"=w255) -> ()  [unwired: 2 in, 2 out]
      n102 = property on="BD 2 Frequency 2 (MHz)" class="DigNum (strict)"("Data Range"=w255) -> ()  [unwired: 2 in, 2 out]
      n103 = property on="BD 1 Frequency 1 (MHz)" class="DigNum (strict)"("Data Range"=w257) -> ()  [unwired: 2 in, 2 out]
      n104 = property on="BD 1 Frequency 2 (MHz)" class="DigNum (strict)"("Data Range"=w257) -> ()  [unwired: 2 in, 2 out]
      n105 = property on="BD 1 Frequency 3 (MHz)" class="DigNum (strict)"("Data Range"=w257) -> ()  [unwired: 2 in, 2 out]
      n106 = property on="BD 2 Amplitude 1 (%)" class="DigNum (strict)"("Data Range"=w254) -> ()  [unwired: 2 in, 2 out]
      n107 = property on="BD 2 Amplitude 2 (%)" class="DigNum (strict)"("Data Range"=w254) -> ()  [unwired: 2 in, 2 out]
      n108 = property on="BD 2 Amplitude 3 (%)" class="DigNum (strict)"("Data Range"=w254) -> ()  [unwired: 2 in, 2 out]
      n109 = property on="BD 1 Amplitude 3 (%)" class="DigNum (strict)"("Data Range"=w256) -> ()  [unwired: 2 in, 2 out]
      n110 = property on="BD 1 Amplitude 2 (%)" class="DigNum (strict)"("Data Range"=w256) -> ()  [unwired: 2 in, 2 out]
      n111 = property on="BD 1 Amplitude 1 (%)" class="DigNum (strict)"("Data Range"=w256) -> ()  [unwired: 2 in, 2 out]
      "X RF Frequency Limits (MHz)" <- w257
      "X RF Amplitude Limits (%)" <- w256
      "Y RF Amplitude Limits (%)" <- w254
      "Y RF Frequency Limits (MHz)" <- w255
    }
  }
  n112 = xnode "Invoke Method"("FPGA VI Reference In"=w45, "error in"=w44) -> ("FPGA VI Reference Out"=w22:T19, "error out"=w21:errorcluster)  [unwired: 1 in]
  n113 = flat-sequence "Initial FPGA Loop Relative Phase Adjustment" {
    tunnel: "Initial Phase Adjustment (APD 2 Gate)" -> [w260]
    tunnel: "Initial Phase Adjustment (GI) 2" -> [w261]
    tunnel: "Initial Phase Adj. (MCL)" -> [w262]
    tunnel: w21 -> [w263]
    tunnel: w22 -> [w264]
    tunnel: "Initial Phase Adjustment (GI)" -> [w265]
    tunnel: "Initial Phase Adjustment (AI1)" -> [w266]
    tunnel: [w266] -> w31
    tunnel: [w265] -> w30
    tunnel: [w264] -> w29
    tunnel: [w263] -> w28
    tunnel: [w262] -> w27
    tunnel: [w261] -> w26
    tunnel: [w260] -> w25
    tunnel: [w278] -> w145
    tunnel: [w272] -> w143
    tunnel: "Initial Phase Adjustment (APD Acq)" -> [w271]
    tunnel: "Initial Phase Adjustment (APD 1 Gate)" -> [w270]
    tunnel: "Initial Phase Adjustment (Green FB)" -> [w269]
    tunnel: w31 -> [w277]
    tunnel: w30 -> [w276]
    tunnel: w29 -> [w275]
    tunnel: w28 -> [w274]
    tunnel: w27 -> [w273]
    tunnel: w26 -> [w268]
    tunnel: w25 -> [w267]
    tunnel: w145 -> [w280]
    tunnel: [w281] -> w144
    tunnel: w143 -> [w281]
    tunnel: [w280] -> w142
    tunnel: w144 -> [w284]
    tunnel: w142 -> [w283]
    tunnel: [w286] -> w141
    tunnel: [w285] -> w140
    tunnel: [w288] -> w20
    tunnel: [w289] -> w23
    tunnel: w141 -> [w289]
    tunnel: w140 -> [w288]
    frame #0 {
      n114 = Wait (ms)(milliseconds to wait=u32 1000) -> ()  [unwired: 1 out]
    }
    frame #1 {
      n115 = xnode "Read/Write Control"("FPGA VI Reference In"=w275, "error in"=w274, "Phase count adjustment"=w277, "Phase count adjustment (GI)"=w276, "Phase count adjustment (MCL)"=w273, "Phase Count Adjustment (APD Acq)"=w271, "Phase count adjustment (APD 1 Gate)"=w270, "Phase count adjustment (APD 2 Gate)"=w267, "Phase count adjustment (Green FB)"=w269, "Phase count adjustment (GI) 2"=w268) -> ("FPGA VI Reference Out"=w272:T19, "error out"=w278:errorcluster)
    }
    frame #2 {
      n116 = Wait (ms)(milliseconds to wait=u32 1000) -> ()  [unwired: 1 out]
    }
    frame #3 {
      w282 = TRUE
      n117 = xnode "Read/Write Control"("FPGA VI Reference In"=w284, "error in"=w283, "+ phase"=w282, "+ phase (GI)"=w282, "+ phase (MCL)"=w282, "+ phase (APD Acq)"=w282, "+ phase (APD 1 Gate)"=w282, "+ phase (APD 2 Gate)"=w282, "+ phase (Green FB)"=w282, "+ phase (GI) 2"=w282) -> ("FPGA VI Reference Out"=w285:T19, "error out"=w286:errorcluster)
    }
    frame #4 {
      n118 = Wait (ms)(milliseconds to wait=u32 1000) -> ()  [unwired: 1 out]
    }
  }
  n119 = local read "Phase adj. (Green FB)"() -> (w113:i16)
  n120 = local read "Phase adj. (GI) 2"() -> (w83:i16)
  n121 = local read "Phase adjust (MCL)"() -> (w172:i16)
  n122 = local read "Phase adj. (AI1)"() -> (w174:i16)
  n123 = local read "Phase adj. (GI)"() -> (w173:i16)
  n124 = xnode "Read/Write Control"("FPGA VI Reference In"=w20, "error in"=w23, "Phase count adjustment"=w174, "Phase count adjustment (GI)"=w173, "Phase count adjustment (MCL)"=w172, "Phase Count Adjustment (APD Acq)"="Phase Adj. (APD Acq)", "Phase count adjustment (APD 1 Gate)"="Phase Adj. (APD 1 Gate)", "Phase count adjustment (APD 2 Gate)"="Phase Adj. (APD 2 Gate)", "Phase count adjustment (Green FB)"=w113, "Phase count adjustment (GI) 2"=w83) -> ("FPGA VI Reference Out"=w19:T19, "error out"=w18:errorcluster)
  n125 = call "Initialize RF boards - interlace 3.vi"("error in"=w18, "FPGA VI Reference In"=w19) -> ("FPGA VI Reference Out"=w150:T19)  [unwired: 1 out]
  n126 = call "set RF board frequency - interlace.vi"("Board 2 Frequency Limits"=w116, "Board 1 Frequency Limits"=w118, "FPGA VI Reference In"=w150, "Board 2 Frequency 3 (MHz)"="BD 2 Frequency 3 (MHz)", "Board 1 Frequency 3 (MHz)"="BD 1 Frequency 3 (MHz)", "Board 2 Frequency 2 (MHz)"="BD 2 Frequency 2 (MHz)", "Board 2 Frequency 1 (MHz)"="BD 2 Frequency 1 (MHz)", "Board 1 Frequency 2 (MHz)"="BD 1 Frequency 2 (MHz)", "Board 1 Frequency 1  (MHz)"="BD 1 Frequency 1 (MHz)") -> ("error out"=w244:errorcluster, "FPGA VI Reference Out"=w245:T19)  [unwired: 1 in]
  n127 = call "set RF board amplitude - interlace.vi"("Board 2 Amplitude Limits"=w115, "Board 1 Amplitude Limits"=w117, "error in"=w244, "FPGA VI Reference In"=w245, "Board 2 Amplitude 3 (%)"="BD 2 Amplitude 3 (%)", "Board 1 Amplitude 3 (%)"="BD 1 Amplitude 3 (%)", "Board 2 Amplitude 2 (%)"="BD 2 Amplitude 2 (%)", "Board 2 Amplitude 1 (%)"="BD 2 Amplitude 1 (%)", "Board 1 Amplitude 2 (%)"="BD 1 Amplitude 2 (%)", "Board 1 Amplitude 1 (%)"="BD 1 Amplitude 1 (%)") -> ("error out"=w16:errorcluster, "FPGA VI Reference Out"=w17:T19)
  n128 = flat-sequence {
    tunnel: w17 -> [w298]
    tunnel: w16 -> [w297]
    tunnel: [w296] -> w237
    tunnel: [w295] -> w236
    tunnel: [w302] -> w235
    tunnel: w237 -> [w302]
    tunnel: [w301] -> w234
    tunnel: w236 -> [w301]
    tunnel: w235 -> [w311]
    tunnel: w234 -> [w310]
    tunnel: [w309] -> w12
    tunnel: [w304] -> w11
    tunnel: [w314] -> w40
    tunnel: [w318] -> w24
    tunnel: w12 -> [w318]
    tunnel: w11 -> [w313]
    frame #0 {
      n129 = local read "Trap 1 (ON/OFF)"() -> (w290:bool)
      n130 = xnode "Read/Write Control"("FPGA VI Reference In"=w298, "error in"=w297, "Direct RF Box  Communication"=FALSE) -> ("FPGA VI Reference Out"=w296:T19, "error out"=w295:errorcluster)
      n131 = local write "Saving..."(FALSE ("Saving Data")) -> ()
      n132 = local write "Stop All"(FALSE ("Stop All")) -> ()
      n133 = local write "Index"(1.0 ("Index")) -> ()
      n134 = property on="Trap 1 ON" class="Bool (strict)"("Value"=w290) -> ()  [unwired: 2 in, 2 out]
      "Manipulating Trap" <- FALSE ("Manipulating Trap")
    }
    frame #1 {
      n135 = local read "Trap 2 (ON/OFF)"() -> (w300:bool)
      n136 = Wait (ms)(milliseconds to wait=u32 50) -> ()  [unwired: 1 out]
      n137 = property on="Trap 2 ON" class="Bool (strict)"("Val(Sgnl)"=w300) -> ()  [unwired: 2 in, 2 out]
    }
    frame #2 {
      n138 = local read "Scan Range (nm)"() -> (w305:dbl)
      n139 = xnode "Read/Write Control"("FPGA VI Reference In"=w311, "error in"=w310, "FPGA Controls  RF Box"=TRUE ("Direct RF Box  Communication")) -> ("FPGA VI Reference Out"=w309:T19, "error out"=w304:errorcluster)
      n140 = call "Update messages.vi"("Message to add"="UHR-Fleezers ready.", "Old message string"="") -> ("New message string"=w308:string)
      n141 = local write "Messages"(w308) -> ()
      n142 = property on="Scan Range (nm)" class="DigNum (strict)"("Val(Sgnl)"=w305) -> ()  [unwired: 2 in, 2 out]
    }
    frame #3 {
      n143 = call "hamilton_controller.vi"("error in"=w313, "action"=T20."CONNECT") -> ("error out"=w315:errorcluster)  [unwired: 9 in]
      n144 = call "hamilton_controller.vi"("error in"=w315, "action"=T20."INITIALIZE VALVES") -> ("error out"=w314:errorcluster)  [unwired: 9 in]
    }
  }
  n145 = Subtract(x="BD 1 Frequency 1 (MHz)", y="BD 1 Frequency 2 (MHz)") -> (x-y=w160:dbl)
  n146 = Subtract(x="BD 2 Frequency 1 (MHz)", y="BD 2 Frequency 2 (MHz)") -> (x-y=w159:dbl)
  n147 = Square(x=w159) -> (x^2=w157:dbl)
  n148 = Square(x=w160) -> (x^2=w158:dbl)
  n149 = Add(x=w158, y=w157) -> (x+y=w156:dbl)
  n150 = Square Root(x=w156) -> (sqrt(x)=w155:dbl)
  n151 = local write "Trap Delta (MHz)"(w155) -> ()
  n152 = Current VI's Path() -> (path=w1:path)
  n153 = Strip Path(path=w1) -> (stripped path=w2:path)  [unwired: 1 out]
  n154 = Build Path(base path=w2, name or relative path="Locations.txt") -> (appended path=→"Location path":path)
  n155 = Concatenate Strings("N.D.", "\r\n") -> (w5:string)
  n156 = Initialize Array(w5, 4, 3) -> (w8:string[][])
  n157 = local write "Location Matrix"(w8) -> ()
  n158 = call "IMAQ Create"("Image Name"="APD 1 Image", "Image Type"=w64) -> ("New Image"=w63:T2)  [unwired: 3 in, 1 out]
  n159 = call "IMAQ Create"("Image Name"="APD 2 Image", "Image Type"=w64) -> ("New Image"=w62:T2)  [unwired: 3 in, 1 out]
  n160 = call "IMAQ Create"("Image Name"="Det. X Image", "Image Type"=w64) -> ("New Image"=w61:T2)  [unwired: 3 in, 1 out]
  n161 = call "IMAQ Create"("Image Name"="Det. Y Image", "Image Type"=w64) -> ("New Image"=w60:T2)  [unwired: 3 in, 1 out]
  n162 = Bundle("New Image"=w63, "New Image"=w62, "New Image"=w61, "New Image"=w60) -> (w59:T21)  [unwired: 1 in]
  n163 = disable-structure shown="Disabled" {
    disable-tunnel: w24 -> [w347 _]
    frame Disabled {
      w342 = T17 0 items=["Grayscale (U8)", "Grayscale (I16)", "Grayscale (SGL)", "Complex (CSG)", "RGB (U32)", "HSL (U32)", "RGB (U64)", "Grayscale (U16)"] ("Image Type")
      n164 = call <vilib>:"IMAQ Init.vi"("Interface Name"="img0") -> ("error out"=w344:errorcluster, "IMAQ Session Out"=w346:refnum<k11>)  [unwired: 9 in]
      n165 = call <vilib>:"IMAQ Grab Setup.vi"("error in (no error)"=w344, "IMAQ Session In"=w346) -> ("error out"=w340:errorcluster, "IMAQ Session Out"=w341:refnum<k11>)  [unwired: 8 in]
      n166 = call "IMAQ Create"("Image Name"="untitled", "Image Type"=w342) -> ("New Image"=w339:T2)  [unwired: 3 in, 1 out]
      n167 = call <vilib>:"Application Directory.vi"() -> ("Application Directory"=w326:path)
      n168 = Build Path(base path=w326, name or relative path="_trap_screen_positions") -> (appended path=w334:path)
      n169 = Open/Create/Replace File(file path (use dialog)=w334, operation (0:open)=T22."open or create", access (0:read/write)=enum16{"read/write", "read-only", "write-only"}."read/write") -> (refnum out=w336:refnum<file>)  [unwired: 3 in, 2 out]
      n170 = local read "Trap Sets"() -> (w328:u32)
      n171 = for "Load trap positions on video screen from file." {
        N: w328 -> [_]
        tunnel: [w354] -> w329
        tunnel: w336 -> [w353]
        tunnel: [w350] -> w325 mode=indexing
        w352 = 4
        n172 = for {
          N: w352 -> [_]
          tunnel: [w358] -> w354
          tunnel: w353 -> [w357]
          tunnel: w352 -> [w356]
          tunnel: [w355] -> w351 mode=indexing
          n173 = Read from Binary File(5:w356, 11:w357) -> (2:w355:i32, 3:w358:refnum<file>)  [unwired: 4 in, 2 out]
        }
        n174 = Array To Cluster(array=w351) -> (cluster=w350:T26)
      }
      n175 = node-c288() -> (w349:T23)  [unwired: 4 in]
      n176 = timed-loop "acquire video and stage position" {
        timing: w349 -> [_]
        timing-out: [_] -> w348
        tunnel: w341 -> [w377]
        tunnel: w340 -> [w376]
        tunnel: w339 -> [w375]
        tunnel: [w374] -> w321
        tunnel: [w371] -> w322
        tunnel: [w372] -> w320
        tunnel: w347 -> [_]
        shift-right: [w368] -> w338
        shift-left: w325 -> [w369]
        tunnel: w328 -> [w366]
        stop <- w373 stop-if-true
        n177 = node-c288() -> ()  [unwired: 1 in, 1 out]
        n178 = event shown="[2] \"Primary Video Display\": Mouse Down" {
          selector: _ -> [_ _ _ _]
          dyn-events: _ -> [_ _ _ _]
          timeout: 10 -> [_ _ _ _]
          tunnel: w377 -> [w388 w403 w412 w431]
          tunnel: w376 -> [w387 w405 w410 w433]
          tunnel: w375 -> [w386 w404 w411 w432]
          tunnel: [w385 w403 w412 w431] -> w374
          tunnel: [w378 w407 FALSE FALSE] -> w373
          tunnel: [w382 w405 w410 w433] -> w372
          tunnel: [w381 w404 w411 w432] -> w371
          tunnel: "radius" -> [_ _ w417 _]
          tunnel: w369 -> [w379 w406 w415 _]
          tunnel: [w379 w406 w416 cluster{i32, i32, i32, i32}[] []] -> w368
          tunnel: w366 -> [_ _ w408 _]
          event Timeout {
            n179 = event-data() -> ()  [unwired: 1 in, 2 out]
            n180 = call <vilib>:"IMAQ Grab Acquire.vi"("error in (no error)"=w387, "Image In"=w386, "IMAQ Session In"=w388) -> ("error out"=w383:errorcluster, "Image Out"=w384:T2, "IMAQ Session Out"=w385:refnum<k11>)  [unwired: 5 in, 1 out]
            n181 = case shown="True" "trap\nmarkers?" {
              tunnel: w379 -> [_ w396]
              tunnel: w384 -> [w390 w395]
              tunnel: w383 -> [w389 w394]
              tunnel: [w389 w393] -> w382
              tunnel: [w390 w391] -> w381
              frame False {
              }
              frame True {
                n182 = for {
                  tunnel: w396 -> [w402] mode=indexing
                  shift-right: [w400] -> w391
                  shift-left: w395 -> [w401]
                  tunnel: w394 -> [w399]
                  tunnel: [w398] -> w393
                  tunnel: u32 16711680 ("Color") -> [w397]
                  n183 = call "IMAQ Overlay Oval"("Color"=w397, "error in (no error)"=w399, "Bounding Rectangle"=w402, "Image"=w401) -> ("error out"=w398:errorcluster, "Image Out"=w400:T2)  [unwired: 6 in]
                }
              }
            }
            "Primary Video Display" <- w381
            n184 = Unbundle By Name(w383) -> ("status"=w378:bool)
          }
          event "Stop All": Value Change {
            n185 = event-data() -> ()  [unwired: 1 in, 5 out]
            n186 = local read "Stop All"() -> (w407:bool)
          }
          event "Primary Video Display": Mouse Down {
            n187 = event-data() -> ()  [unwired: 1 in, 7 out]
            n188 = Array Size(array=w415) -> (size(s)=w414:i32)
            n189 = Less?(x=w414, y=w408) -> (x < y?=w413:bool)
            n190 = case shown="True" w413 {
              tunnel: w417 -> [_ w427]
              tunnel: w415 -> [w418 w421]
              tunnel: [w418 w420] -> w416
              frame False {
              }
              frame True {
                n191 = property on="Primary Video Display" class="ImageControl"() -> ("Last Mouse Position"=w419:cluster{"X":i32, "Y":i32})  [unwired: 2 in, 2 out]
                n192 = Unbundle By Name(w419) -> ("X"=w429:i32, "Y"=w428:i32)
                n193 = Add(x=w428, y=w427) -> (x+y=w425:i32)
                n194 = Subtract(x=w428, y=w427) -> (x-y=w423:i32)
                n195 = Add(x=w429, y=w427) -> (x+y=w424:i32)
                n196 = Subtract(x=w429, y=w427) -> (x-y=w426:i32)
                n197 = Bundle(w426, w425, w424, w423) -> (w422:cluster{i32, i32, i32, i32})  [unwired: 1 in]
                n198 = Build Array (concatenate)(w421, w422) -> (w420:T27)
              }
            }
          }
          event "clear markers": Value Change {
            n199 = event-data() -> ()  [unwired: 1 in, 5 out]
          }
        }
        n200 = node-c288() -> ()  [unwired: 1 in, 1 out]
      }
      n201 = node-c288(w348) -> ()  [unwired: 1 out]
      n202 = Set File Position(offset (in bytes) (0)=i64 0, refnum=w329, from (0:start)=enum16{"start", "end", "current"}."start") -> (refnum out=w330:refnum<file>)  [unwired: 1 in, 1 out]
      n203 = for "Write trap positions to file so they can be remembered\nwhen program is removed from memory" {
        tunnel: w338 -> [w362] mode=indexing
        tunnel: [w360] -> w337
        tunnel: w330 -> [w359]
        n204 = Cluster To Array(cluster=w362) -> (array=w361:i32[])
        n205 = for {
          tunnel: w361 -> [w365] mode=indexing
          tunnel: [w364] -> w360
          tunnel: w359 -> [w363]
          n206 = Write to Binary File(file (use dialog)=w363, data=w365) -> (refnum out=w364:refnum<file>)  [unwired: 4 in, 2 out]
        }
      }
      n207 = Close File(refnum=w337) -> ()  [unwired: 1 in, 2 out]
      n208 = call "IMAQ Dispose"("Image"=w322, "error in (no error)"=w320) -> ("error out"=w319:errorcluster)  [unwired: 4 in]
      n209 = call <vilib>:"IMAQ Stop.vi"("error in (no error)"=w319, "IMAQ Session In"=w321) -> ("error out"=w323:errorcluster, "IMAQ Session Out"=w324:refnum<k11>)  [unwired: 8 in]
      n210 = call <vilib>:"IMAQ Close.vi"("error in (no error)"=w323, "IMAQ Session In"=w324) -> ()  [unwired: 9 in, 1 out]
    }
    frame Enabled {
    }
  }
  n211 = while {
    stop <- w439 stop-if-true
    n212 = event shown="[0] Timeout" {
      selector: _ -> [_ _ _ _ _ _ _]
      dyn-events: _ -> [_ _ _ _ _ _ _]
      timeout: 10 -> [_ _ _ _ _ _ _]
      tunnel: [FALSE _ _ _ _ _ _] -> w439
      event Timeout {
        # "Setting ESP300 left and right limits for Z-axis, input in mm"
        # "Change Low Jog Velocity"
        # "Change High Jog Velocity"
        # "Display Selected Location"
        # "Query and display stage positions"
        n213 = event-data() -> ()  [unwired: 1 in, 2 out]
        n214 = local read "ESP Port"() -> (w447:refnum<visa-resource-name>)
        n215 = Concatenate Strings("3SL" ("Substring"), "ESP ZL-Limit", "3SR", "ESP ZR-Limit", "\r") -> (w446:string)
        n216 = VISA Write(VISA resource name=w447, write buffer=w446) -> ()  [unwired: 1 in, 3 out]
        n217 = local read "Location Matrix"() -> (w471:string[][])
        n218 = local read "Locations"() -> (w470:i32)
        n219 = Index Array(array=w471, index (row)=w470) -> (element=w469:string[])  [unwired: 1 in]
        n220 = Concatenate Strings("1JH" ("Substring"), "Axis 1", "2JH" ("Substring"), "Axis 2", "3JH" ("Substring"), "Axis 3", "\r") -> (w465:string)
        n221 = local read "ESP Port"() -> (w464:refnum<visa-resource-name>)
        n222 = VISA Write(VISA resource name=w464, write buffer=w465) -> ()  [unwired: 1 in, 3 out]
        n223 = Array To Cluster(array=w469) -> (cluster=w468:T28)
        n224 = local write "Selected Location"(w468) -> ()
        n225 = Concatenate Strings("1JW" ("Substring"), "Axis 1", "2JW" ("Substring"), "Axis 2", "3JW" ("Substring"), "Axis 3", "\r") -> (w456:string)
        n226 = local read "ESP Port"() -> (w455:refnum<visa-resource-name>)
        n227 = VISA Write(VISA resource name=w455, write buffer=w456) -> ()  [unwired: 1 in, 3 out]
        n228 = Concatenate Strings("1TP;\n2TP;\n3TP" ("Substring"), "\r") -> (w474:string)
        n229 = local read "ESP Port"() -> (w477:refnum<visa-resource-name>)
        n230 = VISA Write(VISA resource name=w477, write buffer=w474, error in (no error)="error in") -> (VISA resource name out=w475:refnum<visa-resource-name>, error out=w473:errorcluster)  [unwired: 1 out]
        n231 = case shown="True" TRUE ("Case Constant\n(See Context Help)") {
          tunnel: w475 -> [_ w490]
          tunnel: w473 -> [w480 w489]
          tunnel: [w480 w486] -> w479
          frame False {
          }
          frame True {
            w482 = u16 10 items=["1.0"=10, "1.5"=15, "2.0"=20] ("Serial Settings:Stop Bits")
            w483 = u16 0 items=["None", "Odd", "Even", "Mark", "Space"] ("Serial Settings:Parity")
            n232 = property class="Instr"(reference=w490, error in=w489, "Baud"=u32 921600 ("Serial Settings:Baud Rate"), "Data Bits"=u16 8 ("Serial Settings:Data Bits"), "Parity"=w483, "Stop Bits"=w482) -> (reference out=w488:refnum<visa-resource-name>, error out=w487:errorcluster, "Bytes at Port"=w481:u32)
            n233 = Wait (ms)(milliseconds to wait=u32 10) -> ()  [unwired: 1 out]
            n234 = VISA Read(VISA resource name=w488, byte count=w481, error in (no error)=w487) -> (VISA resource name out=w496:refnum<visa-resource-name>, read buffer=→"X Pos":string, error out=w497:errorcluster)  [unwired: 1 out]
            n235 = VISA Read(VISA resource name=w496, byte count=w481, error in (no error)=w497) -> (VISA resource name out=w494:refnum<visa-resource-name>, read buffer=→"Y Pos":string, error out=w495:errorcluster)  [unwired: 1 out]
            n236 = VISA Read(VISA resource name=w494, byte count=w481, error in (no error)=w495) -> (read buffer=→"Z Pos Pos":string, error out=w486:errorcluster)  [unwired: 2 out]
          }
        }
        "error out" <- w479
      }
      event "Goto Top (F6)": Value Change {
        n237 = event-data() -> ()  [unwired: 1 in, 5 out]
        n238 = stacked-sequence {
          frame #0 {
            # "stop motions of all axes before going to avoid reversing of direction"
            n239 = local read "ESP Port"() -> (w502:refnum<visa-resource-name>)
            n240 = Concatenate Strings("ST" ("Substring"), "\r") -> (w499:string)
            n241 = VISA Write(VISA resource name=w502, write buffer=w499) -> ()  [unwired: 1 in, 3 out]
          }
          frame #1 {
            n242 = Wait (ms)(milliseconds to wait=u32 50) -> ()  [unwired: 1 out]
          }
          frame #2 {
            # "Change the trajectory mode to Trapezoidal"
            n243 = local read "ESP Port"() -> (w507:refnum<visa-resource-name>)
            n244 = Concatenate Strings("1TJ1;\n2TJ1;\n3TJ1" ("Substring"), "\r") -> (w504:string)
            n245 = VISA Write(VISA resource name=w507, write buffer=w504) -> ()  [unwired: 1 in, 3 out]
          }
          frame #3 {
            # "Go to Top Dispensor"
            n246 = local read "Location Matrix"() -> (w519:string[][])
            n247 = Index Array(array=w519, index (row)=0) -> (element=w515:string[])  [unwired: 1 in]
            n248 = Decimate 1D Array(w515) -> (w513:string[], w511:string[], w509:string[])
            n249 = Concatenate Strings("1PA" ("Substring"), w513, "2PA" ("Substring"), w511, "3PA" ("Substring"), w509, "\r") -> (w517:string)
            n250 = local read "ESP Port"() -> (w516:refnum<visa-resource-name>)
            n251 = VISA Write(VISA resource name=w516, write buffer=w517) -> ()  [unwired: 1 in, 3 out]
          }
        }
      }
      event "Goto Exp (F8)": Value Change {
        n252 = event-data() -> ()  [unwired: 1 in, 5 out]
        n253 = stacked-sequence {
          frame #0 {
            # "stop motions of all axes before going to avoid reversing of direction"
            n254 = local read "ESP Port"() -> (w523:refnum<visa-resource-name>)
            n255 = Concatenate Strings("ST" ("Substring"), "\r") -> (w520:string)
            n256 = VISA Write(VISA resource name=w523, write buffer=w520) -> ()  [unwired: 1 in, 3 out]
          }
          frame #1 {
            n257 = Wait (ms)(milliseconds to wait=u32 50) -> ()  [unwired: 1 out]
          }
          frame #2 {
            # "Change the trajectory mode to Trapezoidal"
            n258 = local read "ESP Port"() -> (w528:refnum<visa-resource-name>)
            n259 = Concatenate Strings("1TJ1;\n2TJ1;\n3TJ1" ("Substring"), "\r") -> (w525:string)
            n260 = VISA Write(VISA resource name=w528, write buffer=w525) -> ()  [unwired: 1 in, 3 out]
          }
          frame #3 {
            # "Go to Experimental"
            n261 = local read "Location Matrix"() -> (w540:string[][])
            n262 = Index Array(array=w540, index (row)=2) -> (element=w536:string[])  [unwired: 1 in]
            n263 = Decimate 1D Array(w536) -> (w534:string[], w532:string[], w530:string[])
            n264 = Concatenate Strings("1PA" ("Substring"), w534, "2PA" ("Substring"), w532, "3PA" ("Substring"), w530, "\r") -> (w538:string)
            n265 = local read "ESP Port"() -> (w537:refnum<visa-resource-name>)
            n266 = VISA Write(VISA resource name=w537, write buffer=w538) -> ()  [unwired: 1 in, 3 out]
          }
        }
      }
      event "Goto Bottom (F7)": Value Change {
        n267 = event-data() -> ()  [unwired: 1 in, 5 out]
        n268 = stacked-sequence {
          frame #0 {
            # "stop motions of all axes before going to avoid reversing of direction"
            n269 = local read "ESP Port"() -> (w544:refnum<visa-resource-name>)
            n270 = Concatenate Strings("ST" ("Substring"), "\r") -> (w541:string)
            n271 = VISA Write(VISA resource name=w544, write buffer=w541) -> ()  [unwired: 1 in, 3 out]
          }
          frame #1 {
            n272 = Wait (ms)(milliseconds to wait=u32 50) -> ()  [unwired: 1 out]
          }
          frame #2 {
            # "Change the trajectory mode to Trapezoidal"
            n273 = local read "ESP Port"() -> (w549:refnum<visa-resource-name>)
            n274 = Concatenate Strings("1TJ1;\n2TJ1;\n3TJ1" ("Substring"), "\r") -> (w546:string)
            n275 = VISA Write(VISA resource name=w549, write buffer=w546) -> ()  [unwired: 1 in, 3 out]
          }
          frame #3 {
            # "Go to Bottom Dispensor"
            n276 = local read "Location Matrix"() -> (w561:string[][])
            n277 = Index Array(array=w561, index (row)=1) -> (element=w557:string[])  [unwired: 1 in]
            n278 = Decimate 1D Array(w557) -> (w555:string[], w553:string[], w551:string[])
            n279 = Concatenate Strings("1PA" ("Substring"), w555, "2PA" ("Substring"), w553, "3PA" ("Substring"), w551, "\r") -> (w559:string)
            n280 = local read "ESP Port"() -> (w558:refnum<visa-resource-name>)
            n281 = VISA Write(VISA resource name=w558, write buffer=w559) -> ()  [unwired: 1 in, 3 out]
          }
        }
      }
      event "Capture": Value Change {
        n282 = event-data() -> ()  [unwired: 1 in, 5 out]
        n283 = local read "Locations"() -> (w562:i32)
        n284 = local read "Z Pos Pos"() -> (w563:string)
        n285 = local read "X Pos"() -> (w565:string)
        n286 = local read "Y Pos"() -> (w564:string)
        n287 = case shown="3" w562 {
          selector: w562 -> [w569 w576 w583 w590]
          tunnel: w565 -> [w572 w579 w586 w593]
          tunnel: w564 -> [w571 w578 w585 w592]
          tunnel: w563 -> [w570 w577 w584 w591]
          frame 0, Default {
            # "Capture Top Dispensor Location"
            n288 = local read "Location Matrix"() -> (w568:string[][])
            n289 = Build Array(w572, w571, w570) -> (w567:string[])
            n290 = Replace Array Subset(array=w568, new element=w567, index (row)=w569) -> (w566:string[][])  [unwired: 1 in]
            n291 = local write "Location Matrix"(w566) -> ()
          }
          frame 1 {
            # "Capture Bottom Dispensor Location"
            n292 = local read "Location Matrix"() -> (w575:string[][])
            n293 = Build Array(w579, w578, w577) -> (w574:string[])
            n294 = Replace Array Subset(array=w575, new element=w574, index (row)=w576) -> (w573:string[][])  [unwired: 1 in]
            n295 = local write "Location Matrix"(w573) -> ()
          }
          frame 2 {
            # "Capture Experimental Region Location"
            n296 = local read "Location Matrix"() -> (w582:string[][])
            n297 = Build Array(w586, w585, w584) -> (w581:string[])
            n298 = Replace Array Subset(array=w582, new element=w581, index (row)=w583) -> (w580:string[][])  [unwired: 1 in]
            n299 = local write "Location Matrix"(w580) -> ()
          }
          frame 3 {
            # "Capture Other Location"
            n300 = local read "Location Matrix"() -> (w589:string[][])
            n301 = Build Array(w593, w592, w591) -> (w588:string[])
            n302 = Replace Array Subset(array=w589, new element=w588, index (row)=w590) -> (w587:string[][])  [unwired: 1 in]
            n303 = local write "Location Matrix"(w587) -> ()
          }
        }
      }
      event "Save": Value Change {
        # "reshape Location Matrix to 1-D array to write"
        n304 = event-data() -> ()  [unwired: 1 in, 5 out]
        n305 = local read "Location Matrix"() -> (w597:string[][])
        n306 = local read "Location path"() -> (w594:path)
        n307 = Reshape Array(w597, 12) -> (w595:string[])
        n308 = Write to Text File(file (use dialog)=w594, text=w595) -> ()  [unwired: 2 in, 3 out]
      }
      event "Activate Joystick": Value Change {
        n309 = event-data() -> ()  [unwired: 1 in, 5 out]
        n310 = case shown="True" "Activate Joystick" {
          frame False {
          }
          frame True {
            # "Change the trajectory mode to Jog"
            n311 = local read "ESP Port"() -> (w602:refnum<visa-resource-name>)
            n312 = Concatenate Strings("1TJ3;\n2TJ3;\n3TJ3" ("Substring"), "\r") -> (w599:string)
            n313 = VISA Write(VISA resource name=w602, write buffer=w599) -> ()  [unwired: 1 in, 3 out]
          }
        }
      }
    }
  }
  n314 = node-c288(2 ("Processor")) -> (w15:T23)  [unwired: 3 in]
  n315 = node-c288() -> (w69:T23)  [unwired: 4 in]
  n316 = node-c288(i64 1 ("Period"), 1 ("Processor")) -> (w164:T23)  [unwired: 2 out]
  n317 = disable-structure shown="Enabled" {
    disable-tunnel: [w604 _] -> w35
    disable-tunnel: w24 -> [w603 _]
    frame Enabled {
      n318 = node-c288() -> (w606:T23)  [unwired: 4 out]
      n319 = timed-loop "Rough control of MCL mirror stage (debugging)" {
        tunnel: w603 -> [w609]
        tunnel: [w608] -> w604
        timing: w606 -> [_]
        timing-out: [_] -> w605
        stop <- w608 stop-if-true
        n320 = node-c288() -> ()  [unwired: 2 out]
        n321 = case shown="1" "MCL Mode" {
          tunnel: w609 -> [_ w612 w659]
          frame 0, Default {
            # "manual positioning"
          }
          frame 1 {
            # "sinusoidal wave"
            n322 = node-c288() -> (w614:T23)  [unwired: 4 out]
            n323 = timed-loop "Oscillate MCL mirror" {
              timing: w614 -> [_]
              timing-out: [_] -> w613
              tunnel: w612 -> [w653]
              i -> [w652]
              stop <- w615 stop-if-true
              n324 = node-c288() -> (w651:i64)  [unwired: 1 out]
              n325 = Multiply(x="AO1", y=32767.0) -> (x*y=w647:dbl)
              n326 = Multiply(x="AO2", y=32767.0) -> (x*y=w642:dbl)
              n327 = Divide(x=w647, y=10.0) -> (x/y=w648:dbl)
              n328 = Divide(x=w642, y=10.0) -> (x/y=w643:dbl)
              n329 = To Word Integer(number=w648) -> (16bit integer=w640:i16)
              n330 = To Word Integer(number=w643) -> (16bit integer=w639:i16)
              n331 = Divide(x=w651, y=i64 1000) -> (x/y=w622:dbl)
              n332 = Multiply(x=w622, y=w652) -> (x*y=w633:dbl)
              n333 = Multiply(x="Osc. freq. (Hz) 2", y=6.283185307179586) -> (x*y=w634:dbl)
              n334 = Multiply(x=w634, y=w633) -> (x*y=w632:dbl)
              n335 = Sine(x=w632) -> (sin(x)=w631:dbl)
              n336 = Multiply(x=w631, y="Osc. amp. (V)") -> (x*y=w629:dbl)
              n337 = Add(x=w629, y="Osc. center (V)") -> (x+y=w627:dbl)
              n338 = Divide(x=w627, y=10.0) -> (x/y=w625:dbl)
              n339 = Multiply(x=w625, y=32767.0) -> (x*y=w620:dbl)
              n340 = Select(t=w620, s="Scan axis", f=w640) -> (s? t:f=w638:dbl)
              n341 = Select(t=w639, s="Scan axis", f=w620) -> (s? t:f=w637:dbl)
              n342 = local read "MCL Mode"() -> (w619:u16)
              n343 = Not Equal?(x=w619, y=u16 1) -> (x != y?=w616:bool)
              n344 = local read "Stop All"() -> (w617:bool)
              n345 = xnode "Read/Write Control"("FPGA VI Reference In"=w653, "AO1"=w638, "AO2"=w637) -> ()  [unwired: 1 in, 2 out]
              n346 = Compound Arithmetic op=OR(w617, w616) -> (w615:bool)
              n347 = node-c288() -> ()  [unwired: 2 out]
            }
            n348 = node-c288(w613) -> ()  [unwired: 1 out]
          }
          frame 2 {
            # "linear scan"
            n349 = case shown="True" "Start Scan" {
              tunnel: w659 -> [_ w671]
              frame False {
              }
              frame True {
                n350 = Subtract(x="End (V)", y="Begin (V)") -> (x-y=w667:dbl)
                n351 = Decrement(x="N Points") -> (x-1=w666:dbl)
                n352 = Divide(x=w667, y=w666) -> (x/y=w664:dbl)
                n353 = for {
                  N: "N Points" -> [_]
                  tunnel: "Begin (V)" -> [w684]
                  tunnel: w671 -> [w676]
                  tunnel: [w675] -> w670 mode=indexing
                  tunnel: w664 -> [w674]
                  tunnel: [w672] -> w663 mode=indexing
                  i -> [w683]
                  n354 = Multiply(x=w674, y=w683) -> (x*y=w682:dbl)
                  n355 = Add(x=w684, y=w682) -> (x+y=w679:dbl)
                  n356 = local read "Scan axis"() -> (w673:bool)
                  n357 = local read "AO1"() -> (w681:dbl)
                  n358 = local read "AO2"() -> (w680:dbl)
                  n359 = Select(t=w679, s=w673, f=w681) -> (s? t:f=w678:dbl)
                  n360 = Select(t=w680, s=w673, f=w679) -> (s? t:f=w677:dbl)
                  n361 = flat-sequence {
                    tunnel: w678 -> [w688]
                    tunnel: w677 -> [w687]
                    tunnel: w676 -> [w685]
                    tunnel: [w698] -> w675
                    tunnel: [w697] -> w672
                    frame #0 {
                      w691 = 10.0 ("y")
                      w686 = 32767.0 ("y")
                      n362 = Multiply(x=w688, y=w686) -> (x*y=w694:dbl)
                      n363 = Multiply(x=w687, y=w686) -> (x*y=w692:dbl)
                      n364 = Divide(x=w694, y=w691) -> (x/y=w695:dbl)
                      n365 = Divide(x=w692, y=w691) -> (x/y=w693:dbl)
                      n366 = To Word Integer(number=w695) -> (16bit integer=w689:i16)
                      n367 = To Word Integer(number=w693) -> (16bit integer=w690:i16)
                      n368 = xnode "Read/Write Control"("FPGA VI Reference In"=w685, "AO1"=w689, "AO2"=w690) -> ()  [unwired: 1 in, 2 out]
                    }
                    frame #1 {
                      n369 = Wait (ms)(milliseconds to wait="DAQ Delay (ms)") -> ()  [unwired: 1 out]
                    }
                    frame #2 {
                      n370 = local read "Slow mean"() -> (w698:dbl)
                      n371 = local read "Sigma"() -> (w697:dbl)
                    }
                  }
                }
                n372 = Bundle("Begin (V)"="Begin (V)", w664, w670) -> (→"MCL Scan":cluster{"Begin (V)":dbl, dbl, dbl[]})  [unwired: 1 out]
                n373 = Bundle("Begin (V)"="Begin (V)", w664, w663) -> (→"MCL Scan 2":cluster{"Begin (V)":dbl, dbl, dbl[]})  [unwired: 1 out]
              }
            }
          }
        }
        n374 = local read "Stop All"() -> (w608:bool)
        n375 = node-c288() -> ()  [unwired: 2 out]
      }
      n376 = node-c288(w605) -> ()  [unwired: 1 out]
    }
    frame Disabled {
    }
  }
  n377 = timed-loop "Control parameters (event loop)" {
    tunnel: w24 -> [w704]
    shift-right: [w703] -> _
    shift-left: errorcluster {"status"=FALSE, "code"=0, "source"=""} ("error out") -> [w702]
    tunnel: [w701] -> w37
    timing: w15 -> [_]
    timing-out: [_] -> w14
    stop <- w701 stop-if-true
    n378 = node-c288() -> ()  [unwired: 1 in, 1 out]
    n379 = event shown="[22] \"- phase (APD 1 Gate)\", \"+ phase (APD 1 Gate)\": Value Change" {
      selector: _ -> [_ _ _ _ _ _ _ _ _ _ _ _ _ _ _ _ _ _ _ _ _ _ _ _ _ _ _ _ _ _ _ _ _ _ _ _ _ _ _ _ _ _ _ _ _ _ _ _ _ _ _ _ _ _ _]
      dyn-events: _ -> [_ _ _ _ _ _ _ _ _ _ _ _ _ _ _ _ _ _ _ _ _ _ _ _ _ _ _ _ _ _ _ _ _ _ _ _ _ _ _ _ _ _ _ _ _ _ _ _ _ _ _ _ _ _ _]
      timeout: _ -> [_ _ _ _ _ _ _ _ _ _ _ _ _ _ _ _ _ _ _ _ _ _ _ _ _ _ _ _ _ _ _ _ _ _ _ _ _ _ _ _ _ _ _ _ _ _ _ _ _ _ _ _ _ _ _]
      tunnel: w704 -> [w742 _ _ _ w779 _ w801 _ w865 _ _ _ w908 _ _ w951 w957 w962 w968 w1004 w1022 w1029 w1047 w1058 w1069 w1080 w1091 w1102 w1120 w1126 w1220 _ w1229 w1267 _ w1302 w1306 w1317 w1321 w1325 _ w1333 _ _ _ _ w1467 _ w1484 w1487 w1496 w1499 w1503 _ w1520]
      tunnel: [w741 _ _ _ w769 _ w800 _ w828 _ w873 _ w887 _ _ w950 w953 w959 w965 w1003 w1020 w1028 w1041 w1052 w1063 w1074 w1085 w1096 w1118 w1125 w1218 _ w1227 w1265 _ w1300 w1304 w1307 w1319 w1323 _ w1331 _ _ _ _ w1465 _ _ _ _ _ _ _ _] -> w703
      tunnel: w702 -> [w740 _ _ _ w778 _ w799 _ w860 _ w873 _ w907 _ _ w949 w952 w958 w964 w1002 w1021 w1027 w1046 w1057 w1068 w1079 w1090 w1101 w1119 w1124 w1219 _ w1228 w1266 _ w1301 w1305 w1316 w1320 w1324 _ w1332 _ _ _ _ w1466 _ w1483 w1486 w1495 w1498 w1502 _ w1519]
      tunnel: [_ _ _ _ _ _ _ _ _ _ w872 _ _ _ _ _ _ _ _ _ _ _ _ _ _ _ _ _ _ _ _ _ _ _ _ _ _ _ _ _ _ _ _ _ _ _ _ _ _ _ _ _ _ _ _] -> w701
      tunnel: [_ _ _ _ _ _ _ "Round T1 X" _ _ _ _ _ _ _ _ _ _ _ _ _ _ _ _ _ _ _ _ _ _ _ _ _ _ _ _ _ _ _ _ _ _ _ _ _ _ _ _ _ _ _ _ _ _ _] -> _
      tunnel: [_ _ _ "Adjust Scale\nto Mean" _ _ _ _ _ _ _ _ _ _ _ _ _ _ _ _ _ _ _ _ _ _ _ _ _ _ _ _ _ _ _ _ _ _ _ _ _ _ _ _ _ _ _ _ _ _ _ _ "Set SP to Reading" _ _] -> _
      tunnel: [_ _ _ _ _ _ _ _ _ "Round T2 X" _ "Delayed Interlace Start" _ _ _ _ _ _ _ _ _ _ _ _ _ _ _ _ _ _ _ _ _ _ _ _ _ _ _ _ _ _ _ _ _ _ _ _ _ _ _ _ _ _ _] -> _
      event "AI Count (ticks)", "Sets to FIFO (Traps)", "Save ave N", "FPGA Ave.", "# Samples/channel", "N sets to save": Value Change {
        # "So that if 'Save ave N' is updated, the AOD scanning code updates too."
        n380 = event-data() -> ()  [unwired: 6 out]
        n381 = local read "AI Count (ticks)"() -> (w722:u32)
        n382 = Boolean To (0,1)(Boolean="Sets to FIFO (Traps)") -> (0, 1=w732:cluster{"Set 1":i16, "Set 2":i16, "Set 3":i16})
        n383 = xnode "Read/Write Control"("FPGA VI Reference In"=w742, "error in"=w740, "ai count"=w722, "AI1 Sets to FIFO"="Sets to FIFO (Traps)", "N of AI1 Int Acq Sets"="N Acq Sets (Traps + Fl.)") -> ("error out"=w741:errorcluster)  [unwired: 1 out]
        n384 = Cluster To Array(cluster=w732) -> (array=w731:i16[])
        n385 = To Unsigned Long Integer(number=w731) -> (unsigned 32bit integer=w711:u32[])
        n386 = local read "Scan steps (AOD)"() -> (w733:u64)
        n387 = Multiply(x=w722, y="N Acq Sets (Traps + Fl.)") -> (x*y=w720:u32)
        n388 = Divide(x=40000000.0, y=w722) -> (x/y=w714:dbl)
        "AI rate (Hz)" <- w714
        "Ave. Rate (Hz)" <- w714
        n389 = Add Array Elements(numeric array=w711) -> (sum=w723:u32)
        "Trap Sets" <- w723
        n390 = Reciprocal(x=w714) -> (1/x=→"Ave. Period (s)":dbl)
        n391 = property on="Scan steps (AOD)" class="DigNum (strict)"("Val(Sgnl)"=w733) -> ()  [unwired: 2 in, 2 out]
        n392 = Divide(x=w714, y="N Acq Sets (Traps + Fl.)") -> (x/y=w737:dbl)
        "Data Rate (Hz)" <- w737
        n393 = Reciprocal(x=w737) -> (1/x=→"Data Period (s)":dbl)
        n394 = local read "Save ave N"() -> (w736:dbl)
        n395 = Divide(x=w737, y=w736) -> (x/y=w735:dbl)
        "Save Data Rate (Hz)" <- w735
        n396 = Reciprocal(x=w735) -> (1/x=→"Save Data Period (s)":dbl)
        n397 = Multiply(x=w720, y="# Samples/trap") -> (x*y=w718:u32)
        "Counts/DMA" <- w718
        n398 = property on="Trap Disp. Downsample" class="DigNum (strict)"("Maximum"="# Samples/trap") -> ()  [unwired: 2 in, 2 out]
        n399 = Multiply(x=w723, y="# Samples/trap") -> (x*y=w712:u32)
        "# Samples/channel" <- w712
        n400 = Multiply(x=w712, y=u32 8) -> (x*y=→"Trap AI Elements/DMA read":u32)
        n401 = local read "APD Int. Count"() -> (w719:u32)
        n402 = Multiply(x=w712, y=u32 3) -> (x*y=→"Trap Pos Elements/DMA read":u32)
        n403 = Divide(x=w718, y=w719) -> (x/y=w709:dbl)
        "APD Samples/FIFO Acq." <- w709
        n404 = Divide(x=w718, y=40000000.0) -> (x/y=w716:dbl)
        "DMA Update Period (s)" <- w716
        n405 = Multiply(x=2.0, y=w709) -> (x*y=→"APD Elements/DMA read":dbl)
        n406 = property on="APD Disp. Downsample" class="DigNum (strict)"("Maximum"=w709) -> ()  [unwired: 2 in, 2 out]
        n407 = local read "N sets to save"() -> (w729:u32)
        n408 = Multiply(x=w716, y=w729) -> (x*y=→"Total Time (s)":dbl)
        "FPGA Averaging" <- FALSE ("FPGA Averaging")
      }
      event "Rescale on Mean": Value Change {
        n409 = event-data() -> ()  [unwired: 7 out]
        n410 = And(x=FALSE, y="Rescale on Mean") -> (x .and. y?=w744:bool)
        n411 = local write "Rescale on Mean"(w744) -> ()
        n412 = local read "Bead Mean (nm)"() -> (w749:dbl)
        n413 = Add(x="Amplitude (nm)", y=w749) -> (x+y=w747:dbl)
        n414 = Subtract(x=w749, y="Amplitude (nm)") -> (x-y=w746:dbl)
        n415 = property on="Bead Separation" class="WFChart (strict)"("YScale.Minimum"=w746) -> ()  [unwired: 2 in, 2 out]
        n416 = property on="Bead Separation" class="WFChart (strict)"("YScale.Maximum"=w747) -> ()  [unwired: 2 in, 2 out]
      }
      event "Detector Type": Value Change {
        n417 = event-data() -> ()  [unwired: 7 out]
        n418 = local read "AI labels"() -> (w750:string[])
        n419 = property on="High Res. Display" class="Ring (strict)"("Strings []"=w750) -> ()  [unwired: 2 in, 2 out]
        n420 = Build Array (concatenate)(w750, "none") -> (w751:string[])
        n421 = property on="FFT 1 Choice 1" class="Ring (strict)"("Strings []"=w751) -> ()  [unwired: 2 in, 2 out]
        n422 = property on="FFT 1 Choice 2" class="Ring (strict)"("Strings []"=w751) -> ()  [unwired: 2 in, 2 out]
        n423 = property on="FFT 2 Choice 1" class="Ring (strict)"("Strings []"=w751) -> ()  [unwired: 2 in, 2 out]
        n424 = property on="FFT 2 Choice 2" class="Ring (strict)"("Strings []"=w751) -> ()  [unwired: 2 in, 2 out]
        n425 = Bundle("APD 1", "APD 2") -> (w754:cluster{string, string})  [unwired: 1 out]
        n426 = Cluster To Array(cluster=w754) -> (array=w752:string[])
        n427 = Build Array (concatenate)(w752, w751) -> (w756:string[])
        n428 = Array Size(array=w756) -> (size(s)=w757:i32)
        n429 = property on="Signals to Plot" class="LstBox (strict)"("Item Names"=w756) -> ()  [unwired: 2 in, 2 out]
        n430 = property on="Signals to Plot" class="LstBox (strict)"("Number of Rows"=w757) -> ()  [unwired: 2 in, 2 out]
        n431 = property on="All Signals" class="WFChart (strict)"("LegNumRows"=w757) -> ()  [unwired: 2 in, 2 out]
      }
      event "Adjust Scale\nto Mean": Value Change {
        n432 = event-data() -> ()  [unwired: 7 out]
        n433 = local read "APD 1 Rate (Hz)"() -> (w766:dbl)
        n434 = Multiply(x=1000.0, y="Above (kHz)") -> (x*y=w764:dbl)
        n435 = Multiply(x=1000.0, y="Below (kHz)") -> (x*y=w762:dbl)
        n436 = Add(x=w764, y=w766) -> (x+y=w759:dbl)
        n437 = Subtract(x=w766, y=w762) -> (x-y=w760:dbl)
        n438 = property on="APD Chart" class="WFChart (strict)"("YScale.Minimum"=w760) -> ()  [unwired: 2 in, 2 out]
        n439 = property on="APD Chart" class="WFChart (strict)"("YScale.Maximum"=w759) -> ()  [unwired: 2 in, 2 out]
      }
      event "Phase adj. (AI1)", "+ phase (AI1)", "- phase (AI1)": Value Change {
        n440 = event-data() -> ()  [unwired: 7 out]
        n441 = Negate(x="Phase adj. (AI1)") -> (-x=w776:i16)
        n442 = Select(t=w776, s="- phase (AI1)", f="Phase adj. (AI1)") -> (s? t:f=w775:i16)
        n443 = xnode "Read/Write Control"("FPGA VI Reference In"=w779, "error in"=w778, "Phase count adjustment"=w775) -> ("FPGA VI Reference Out"=w774:T19, "error out"=w773:errorcluster)
        n444 = Or(x="- phase (AI1)", y="+ phase (AI1)") -> (x .or. y?=w770:bool)
        n445 = xnode "Read/Write Control"("FPGA VI Reference In"=w774, "error in"=w773, "+ phase"=w770) -> ("error out"=w769:errorcluster)  [unwired: 1 out]
      }
      event "Signals to Plot": Double Click {
        w782 = u32 9868950 ("Color Box")
        n446 = event-data() -> ("Row"=w784:i32)  [unwired: 9 out]
        n447 = property on="All Signals" class="WFChart (strict)"("Active Plot"=w784) -> (error out=w795:errorcluster)  [unwired: 2 in, 1 out]
        n448 = property on="All Signals" class="WFChart (strict)" props=["Plot", "Visible?", "Plot", "Plot Color"](error in=w795) -> (error out=w794:errorcluster, "Plot.Visible?"=w793:bool)  [unwired: 1 in, 2 out]
        n449 = Select(t=FALSE ("Plot.Visible"), s=w793, f=TRUE ("Plot.Visible")) -> (s? t:f=w788:bool)
        n450 = property on="All Signals" class="WFChart (strict)"(error in=w794, "Plot.Visible?"=w788) -> (error out=w790:errorcluster)  [unwired: 1 in, 1 out]
        n451 = property on="All Signals" class="WFChart (strict)"(error in=w790) -> (error out=w785:errorcluster, "Plot.Plot Color"=w789:u32)  [unwired: 1 in, 1 out]
        n452 = property on="Signals to Plot" class="LstBox (strict)"(error in=w785, "Active Row"=w784) -> (error out=w783:errorcluster)  [unwired: 1 in, 1 out]
        n453 = Select(t=w789, s=w788, f=u32 0) -> (s? t:f=w786:u32)
        n454 = property on="Signals to Plot" class="LstBox (strict)"(error in=w783, "CellFontColor"=w786, "SelColor"=w782, "CellBG"=w782, "CellFontSize"=u32 20 ("Active Row:Cell Font:Size"), "CellFontBold"=TRUE ("Active Row:Cell Font:Bold")) -> ()  [unwired: 1 in, 2 out]
      }
      event "BD 1 Frequency 1 (MHz)", "BD 1 Frequency 2 (MHz)", "BD 1 Frequency 3 (MHz)", "BD 2 Frequency 1 (MHz)", "BD 2 Frequency 2 (MHz)", "BD 2 Frequency 3 (MHz)", "Trap Delta (MHz)": Value Change {
        # "anytime one of the frequencies is changed, write it to the RF board UNLESS Set 2 is being oscillated. The oscillation\nscript writes the frequencies to the RF board."
        n455 = event-data() -> ("CtlRef"=w798:refnum<vi>)  [unwired: 6 out]
        n456 = control-ref of="Trap Delta (MHz)"() -> (w797:refnum<vi>)
        n457 = Equal?(x=w797, y=w798) -> (x = y?=w796:bool)
        n458 = case shown="False" "Oscillate Set 2" {
          tunnel: w801 -> [w821 _]
          tunnel: [w820 w824] -> w800
          tunnel: w799 -> [w819 w824]
          tunnel: w796 -> [w805 _]
          frame False {
            n459 = local read "BD 1 Frequency 1 (MHz)"() -> (w803:dbl)
            n460 = local read "BD 1 Frequency 2 (MHz)"() -> (w807:dbl)
            n461 = Add(x=w803, y="Trap Delta (MHz)") -> (x+y=w806:dbl)
            n462 = Select(t=w806, s=w805, f=w807) -> (s? t:f=w804:dbl)
            n463 = local read "Y RF Frequency Limits (MHz)"() -> (w809:T16)
            n464 = local read "X RF Frequency Limits (MHz)"() -> (w810:T16)
            n465 = local read "BD 1 Frequency 3 (MHz)"() -> (w822:dbl)
            n466 = local write "BD 1 Frequency 2 (MHz)"(w804) -> ()
            n467 = local read "BD 2 Frequency 1 (MHz)"() -> (w813:dbl)
            n468 = local read "BD 2 Frequency 2 (MHz)"() -> (w812:dbl)
            n469 = local read "BD 2 Frequency 3 (MHz)"() -> (w823:dbl)
            n470 = call "set RF board frequency - interlace.vi"("Board 2 Frequency Limits"=w809, "Board 1 Frequency Limits"=w810, "error in"=w819, "FPGA VI Reference In"=w821, "Board 2 Frequency 3 (MHz)"=w823, "Board 1 Frequency 3 (MHz)"=w822, "Board 2 Frequency 2 (MHz)"=w812, "Board 2 Frequency 1 (MHz)"=w813, "Board 1 Frequency 2 (MHz)"=w804, "Board 1 Frequency 1  (MHz)"=w803) -> ("error out"=w820:errorcluster)  [unwired: 1 out]
            n471 = Subtract(x=w813, y=w812) -> (x-y=w817:dbl)
            n472 = Subtract(x=w804, y=w803) -> (x-y=w818:dbl)
            n473 = Square(x=w817) -> (x^2=w815:dbl)
            n474 = Square(x=w818) -> (x^2=w816:dbl)
            n475 = Add(x=w816, y=w815) -> (x+y=w814:dbl)
            n476 = Square Root(x=w814) -> (sqrt(x)=w811:dbl)
            n477 = local write "Trap Delta (MHz)"(w811) -> ()
            n478 = property on="Initial delta (MHz)" class="DigNum (strict)"("Val(Sgnl)"=w811) -> ()  [unwired: 2 in, 2 out]
          }
          frame True {
          }
        }
      }
      event "Round T1 X": Value Change {
        n479 = event-data() -> ()  [unwired: 7 out]
        n480 = local read "BD 1 Frequency 1 (MHz)"() -> (w827:dbl)
        n481 = Round To Nearest(number=w827) -> (nearest integer value=w826:dbl)
        n482 = property on="BD 1 Frequency 1 (MHz)" class="DigNum (strict)"("Val(Sgnl)"=w826) -> ()  [unwired: 2 in, 2 out]
      }
      event "Restart RF": Value Change {
        n483 = event-data() -> ()  [unwired: 7 out]
        n484 = xnode "Read/Write Control"("FPGA VI Reference In"=w865, "error in"=w860, "FPGA Controls  RF Box"=FALSE) -> ("FPGA VI Reference Out"=w864:T19, "error out"=w859:errorcluster)
        n485 = local read "Y RF Amplitude Limits (%)"() -> (w840:T16)
        n486 = local read "X RF Amplitude Limits (%)"() -> (w841:T16)
        n487 = local read "X RF Frequency Limits (MHz)"() -> (w843:T16)
        n488 = local read "Y RF Frequency Limits (MHz)"() -> (w842:T16)
        n489 = xnode "Read/Write Control"("FPGA VI Reference In"=w864, "error in"=w859, "Direct RF Box  Communication"=TRUE) -> ("FPGA VI Reference Out"=w863:T19, "error out"=w858:errorcluster)
        n490 = local read "BD 2 Frequency 3 (MHz)"() -> (w850:dbl)
        n491 = local read "BD 2 Frequency 2 (MHz)"() -> (w851:dbl)
        n492 = local read "BD 1 Frequency 3 (MHz)"() -> (w854:dbl)
        n493 = local read "BD 1 Frequency 1 (MHz)"() -> (w855:dbl)
        n494 = local read "BD 2 Frequency 1 (MHz)"() -> (w852:dbl)
        n495 = local read "BD 1 Frequency 2 (MHz)"() -> (w853:dbl)
        n496 = call "Initialize RF boards - interlace 3.vi"("error in"=w858, "FPGA VI Reference In"=w863) -> ("error out"=w857:errorcluster, "FPGA VI Reference Out"=w862:T19)
        n497 = local read "BD 2 Amplitude 2 (%)"() -> (w845:dbl)
        n498 = local read "BD 2 Amplitude 1 (%)"() -> (w846:dbl)
        n499 = local read "BD 2 Amplitude 3 (%)"() -> (w844:dbl)
        n500 = local read "BD 1 Amplitude 3 (%)"() -> (w849:dbl)
        n501 = local read "BD 1 Amplitude 1 (%)"() -> (w848:dbl)
        n502 = local read "BD 1 Amplitude 2 (%)"() -> (w847:dbl)
        n503 = call "set RF board frequency - interlace.vi"("Board 2 Frequency Limits"=w842, "Board 1 Frequency Limits"=w843, "error in"=w857, "FPGA VI Reference In"=w862, "Board 2 Frequency 3 (MHz)"=w850, "Board 1 Frequency 3 (MHz)"=w854, "Board 2 Frequency 2 (MHz)"=w851, "Board 2 Frequency 1 (MHz)"=w852, "Board 1 Frequency 2 (MHz)"=w853, "Board 1 Frequency 1  (MHz)"=w855) -> ("error out"=w856:errorcluster, "FPGA VI Reference Out"=w861:T19)
        n504 = call "set RF board amplitude - interlace.vi"("Board 2 Amplitude Limits"=w840, "Board 1 Amplitude Limits"=w841, "error in"=w856, "FPGA VI Reference In"=w861, "Board 2 Amplitude 3 (%)"=w844, "Board 1 Amplitude 3 (%)"=w849, "Board 2 Amplitude 2 (%)"=w845, "Board 2 Amplitude 1 (%)"=w846, "Board 1 Amplitude 2 (%)"=w847, "Board 1 Amplitude 1 (%)"=w848) -> ("error out"=w833:errorcluster, "FPGA VI Reference Out"=w837:T19)
        n505 = xnode "Read/Write Control"("FPGA VI Reference In"=w837, "error in"=w833, "Direct RF Box  Communication"=FALSE) -> ("FPGA VI Reference Out"=w836:T19, "error out"=w835:errorcluster)
        n506 = flat-sequence {
          tunnel: w835 -> [w866]
          tunnel: [w866] -> w834
          frame #0 {
            n507 = Wait (ms)(milliseconds to wait=u32 50) -> ()  [unwired: 1 out]
          }
        }
        n508 = xnode "Read/Write Control"("FPGA VI Reference In"=w836, "error in"=w834, "FPGA Controls  RF Box"=TRUE) -> ("error out"=w829:errorcluster)  [unwired: 1 out]
        n509 = property on="Restart RF" class="Bool (strict)"(error in=w829, "Value"=FALSE ("Restart RF")) -> (error out=w828:errorcluster)  [unwired: 1 in, 1 out]
      }
      event "Round T2 X": Value Change {
        n510 = event-data() -> ()  [unwired: 7 out]
        n511 = local read "BD 1 Frequency 2 (MHz)"() -> (w869:dbl)
        n512 = Round To Nearest(number=w869) -> (nearest integer value=w868:dbl)
        n513 = property on="BD 1 Frequency 2 (MHz)" class="DigNum (strict)"("Val(Sgnl)"=w868) -> ()  [unwired: 2 in, 2 out]
      }
      event "Stop All": Value Change {
        n514 = event-data() -> ()  [unwired: 7 out]
        n515 = call "hamilton_controller.vi"("action"=T20."DISCONNECT") -> ()  [unwired: 10 in, 1 out]
        n516 = local read "Stop All"() -> (w872:bool)
      }
      event "Delayed Interlace Start": Value Change {
        n517 = event-data() -> ()  [unwired: 7 out]
        n518 = flat-sequence {
          frame #0 {
            n519 = Multiply(x="Delay to Interlace (s)", y=1000.0) -> (x*y=w875:dbl)
            n520 = Wait (ms)(milliseconds to wait=w875) -> ()  [unwired: 1 out]
          }
          frame #1 {
            n521 = property on="Green laser mode" class="RadioBtnsControl (strict)"("Val(Sgnl)"=enum32{"Laser ON", "Laser OFF", "Interlace"}."Interlace" ("Value (Signaling)")) -> ()  [unwired: 2 in, 2 out]
          }
        }
      }
      event "BD 1 Amplitude 1 (%)", "BD 1 Amplitude 2 (%)", "BD 1 Amplitude 3 (%)", "BD 2 Amplitude 1 (%)", "BD 2 Amplitude 2 (%)", "BD 2 Amplitude 3 (%)", "Trap 1 ON", "Trap 2 ON", "Trap 3 ON", "Feedback On/Off", "All FB On/Off": Value Change {
        w899 = i16 1 ("f")
        n522 = event-data() -> ()  [unwired: 7 out]
        n523 = local write "Trap 1 (ON/OFF)"("Trap 1 ON") -> ()
        n524 = local write "Trap 2 (ON/OFF)"("Trap 2 ON") -> ()
        n525 = Boolean To (0,1)(Boolean="Trap 3 ON") -> (0, 1=w900:i16)
        n526 = Boolean To (0,1)(Boolean="Trap 1 ON") -> (0, 1=w901:i16)
        n527 = Boolean To (0,1)(Boolean="Trap 2 ON") -> (0, 1=w902:i16)
        n528 = Select(t=w902, s="Trap ON/OFF X or Y Amp?", f=w899) -> (s? t:f=w897:i16)
        n529 = Select(t=w901, s="Trap ON/OFF X or Y Amp?", f=w899) -> (s? t:f=w898:i16)
        n530 = Select(t=w900, s="Trap ON/OFF X or Y Amp?", f=w899) -> (s? t:f=w896:i16)
        n531 = Select(t=w899, s="Trap ON/OFF X or Y Amp?", f=w902) -> (s? t:f=w894:i16)
        n532 = Select(t=w899, s="Trap ON/OFF X or Y Amp?", f=w901) -> (s? t:f=w895:i16)
        n533 = Select(t=w899, s="Trap ON/OFF X or Y Amp?", f=w900) -> (s? t:f=w893:i16)
        n534 = And(x="All FB On/Off", y="Feedback On/Off") -> (x .and. y?=w891:cluster{"Set 1":bool, "Set 2":bool})
        n535 = local read "BD 1 Amplitude 1 (%)"() -> (w911:dbl)
        n536 = local read "BD 1 Amplitude 2 (%)"() -> (w910:dbl)
        n537 = local read "BD 1 Amplitude 3 (%)"() -> (w909:dbl)
        n538 = Unbundle By Name(w891) -> ("Set 1"=w886:bool, "Set 2"=w883:bool)
        n539 = local read "Y RF Amplitude Limits (%)"() -> (w879:T16)
        n540 = local read "X RF Amplitude Limits (%)"() -> (w880:T16)
        n541 = local read "BD 2 Amplitude 1 (%)"() -> (w912:dbl)
        n542 = local read "BD 2 Amplitude 2 (%)"() -> (w913:dbl)
        n543 = local read "BD 2 Amplitude 3 (%)"() -> (w914:dbl)
        n544 = And(x="Trap 2 ON", y=w883) -> (x .and. y?=w881:bool)
        n545 = And(x="Trap 1 ON", y=w886) -> (x .and. y?=w884:bool)
        n546 = Multiply(x=w898, y=w911) -> (x*y=w906:dbl)
        n547 = Multiply(x=w910, y=w897) -> (x*y=w904:dbl)
        n548 = Multiply(x=w909, y=w896) -> (x*y=w905:dbl)
        n549 = Multiply(x=w912, y=w895) -> (x*y=w915:dbl)
        n550 = Multiply(x=w913, y=w894) -> (x*y=w916:dbl)
        n551 = Multiply(x=w914, y=w893) -> (x*y=w917:dbl)
        n552 = call "set RF board amplitude - interlace.vi"("Board 2 Amplitude Limits"=w879, "Board 1 Amplitude Limits"=w880, "error in"=w907, "FPGA VI Reference In"=w908, "Board 2 Amplitude 3 (%)"=w917, "Board 1 Amplitude 3 (%)"=w905, "Board 2 Amplitude 2 (%)"=w916, "Board 2 Amplitude 1 (%)"=w915, "Board 1 Amplitude 2 (%)"=w904, "Board 1 Amplitude 1 (%)"=w906) -> ("error out"=w888:errorcluster, "FPGA VI Reference Out"=w889:T19)
        n553 = xnode "Read/Write Control"("FPGA VI Reference In"=w889, "error in"=w888, "FB On/Off Set 1"=w884, "FB On/Off Set 2"=w881) -> ("error out"=w887:errorcluster)  [unwired: 1 out]
      }
      event "Load parameters": Value Change {
        n554 = event-data() -> ()  [unwired: 7 out]
        n555 = property on="Saved AOD Raster Scan Parameter Sets" class="Arr (strict)"() -> ("Index Values"=w928:u32[])  [unwired: 2 in, 2 out]
        n556 = Index Array(array=w928, index=0) -> (element=w925:u32)
        n557 = local write "Load parameters"(FALSE ("Load parameters")) -> ()
        n558 = Index Array(array="Saved AOD Raster Scan Parameter Sets", index=w925) -> (element=w924:T30)
        n559 = Unbundle By Name(w924) -> ("Scan Range AOD (nm) 2"=w923:dbl, "Step Size AOD (nm) 2"=w922:dbl, "Scan Speed AOD (nm/s) 2"=w921:dbl, "Number of scans (AOD) 2"=w920:u16)
        n560 = flat-sequence {
          tunnel: w923 -> [w931]
          tunnel: w922 -> [w930]
          tunnel: w921 -> [w929]
          tunnel: w920 -> [w932]
          frame #0 {
            n561 = local write "Scan Speed (nm/s)"(w929) -> ()
            n562 = local write "Scan Range (nm)"(w931) -> ()
            n563 = local write "Step Size (nm)"(w930) -> ()
          }
          frame #1 {
            n564 = property on="Number of F/B Scans (AOD)" class="DigNum (strict)"("Val(Sgnl)"=w932) -> ()  [unwired: 2 in, 2 out]
          }
        }
      }
      event "Trap 1 (ON/OFF)", "Trap 2 (ON/OFF)": Value Change {
        n565 = event-data() -> ()  [unwired: 7 out]
        n566 = property on="Trap 2 ON" class="Bool (strict)"("Val(Sgnl)"="Trap 2 (ON/OFF)") -> ()  [unwired: 2 in, 2 out]
        n567 = property on="Trap 1 ON" class="Bool (strict)"("Val(Sgnl)"="Trap 1 (ON/OFF)") -> ()  [unwired: 2 in, 2 out]
      }
      event "DIO count 1 (ticks)", "DIO count 2 (ticks)", "DIO count 3 (ticks)", "Interlace", "Number Interlace Sets", "Not-Interlacing Set": Value Change {
        n568 = event-data() -> ()  [unwired: 7 out]
        n569 = local read "DIO count 3 (ticks)"() -> (w945:u32)
        n570 = local read "DIO count 1 (ticks)"() -> (w947:u32)
        n571 = local read "DIO count 2 (ticks)"() -> (w946:u32)
        n572 = To Unsigned Byte Integer(number="Not-Interlacing Set") -> (unsigned 8bit integer=w936:u8)
        n573 = Add(x=w936, y=u8 1) -> (x+y=w940:u8)
        n574 = xnode "Read/Write Control"("FPGA VI Reference In"=w951, "error in"=w949, "DIO count 1 (ticks)"=w947, "DIO count 2 (ticks)"=w946, "DIO count 3 (ticks)"=w945, "Interlace ON/OFF"="Interlace", "Number Interlace Cycles"="Number Interlace Sets", "Interlace Off Parameters"=w940) -> ("error out"=w950:errorcluster)  [unwired: 1 out]
        n575 = Build Array(w947, w946, w945) -> (w938:u32[])
        n576 = Split 1D Array(array=w938, index="Number Interlace Sets") -> (first subarray=w948:u32[])  [unwired: 1 out]
        n577 = Index Array(array=w938, index=w936) -> (element=w937:u32)
        n578 = Add Array Elements(numeric array=w948) -> (sum=w942:u32)
        n579 = Select(t=w942, s="Interlace", f=w937) -> (s? t:f=→"Total Counts (ticks)":u32)
      }
      event "Reset Feedback": Value Change {
        n580 = event-data() -> ()  [unwired: 7 out]
        n581 = Unbundle By Name("Reset Feedback") -> ("Set 1"=w955:bool, "Set 2"=w954:bool)
        n582 = xnode "Read/Write Control"("FPGA VI Reference In"=w957, "error in"=w952, "FB Reset Set 1"=w955, "FB Reset Set 2"=w954) -> ("error out"=w953:errorcluster)  [unwired: 1 out]
      }
      event "PID Gains": Value Change {
        n583 = event-data() -> ()  [unwired: 7 out]
        n584 = Unbundle By Name("PID Gains") -> ("Set 1"=w961:T14, "Set 2"=w960:T14)
        n585 = xnode "Read/Write Control"("FPGA VI Reference In"=w962, "error in"=w958, "FB Gains Set 1"=w961, "FB Gains Set 2"=w960) -> ("error out"=w959:errorcluster)  [unwired: 1 out]
      }
      event "AI2 to Setpoint", "Trap Intensity\nSetpoints (V)": Value Change {
        n586 = event-data() -> ()  [unwired: 7 out]
        n587 = xnode "Read/Write Control"("FPGA VI Reference In"=w968, "error in"=w964) -> ("FPGA VI Reference Out"=w967:T19, "error out"=w966:errorcluster, "AI2 Y Sum Set 1"=w975:i16, "AI2 Y Sum Set 2"=w974:i16)
        n588 = Cluster To Array(cluster="AI2 to Setpoint") -> (array=w978:bool[])
        n589 = local read "AI2 (V)"() -> (w976:cluster{"Set 1":dbl, "Set 2":dbl})
        n590 = Or Array Elements(Boolean array=w978) -> (logical OR=w979:bool)
        n591 = Bundle By Name(cluster=w976, "Set 1"=w975, "Set 2"=w974) -> (w973:cluster{"Set 1":dbl, "Set 2":dbl})
        n592 = Divide(x=w973, y=3276.7) -> (x/y=w972:cluster{"Set 1":dbl, "Set 2":dbl})
        "AI2 (V)" <- w972
        n593 = case shown="True" w979 {
          tunnel: [w982 w999] -> w971
          tunnel: "AI2 to Setpoint" -> [_ w995]
          tunnel: "Trap Intensity\nSetpoints (V)" -> [w983 w998]
          tunnel: w972 -> [_ w992]
          frame False {
            n594 = Multiply(x=3276.7, y=w983) -> (x*y=w984:cluster{"Set 1":dbl, "Set 2":dbl})
            n595 = To Word Integer(number=w984) -> (16bit integer=w982:cluster{"Set 1":i16, "Set 2":i16})
          }
          frame True {
            n596 = Unbundle By Name(w992) -> ("Set 1"=w991:dbl, "Set 2"=w990:dbl)
            n597 = Unbundle By Name(w998) -> ("Set 1"=w997:dbl, "Set 2"=w996:dbl)
            n598 = Unbundle By Name(w995) -> ("Set 1"=w994:bool, "Set 2"=w993:bool)
            n599 = Select(t=w991, s=w994, f=w997) -> (s? t:f=w989:dbl)
            n600 = Select(t=w990, s=w993, f=w996) -> (s? t:f=w988:dbl)
            n601 = Bundle By Name(cluster=w998, "Set 1"=w989, "Set 2"=w988) -> (w986:cluster{"Set 1":dbl, "Set 2":dbl})
            n602 = local write "Trap Intensity\nSetpoints (V)"(w986) -> ()
            n603 = Multiply(x=3276.7, y=w986) -> (x*y=w987:cluster{"Set 1":dbl, "Set 2":dbl})
            n604 = To Word Integer(number=w987) -> (16bit integer=w999:cluster{"Set 1":i16, "Set 2":i16})
          }
        }
        n605 = Unbundle By Name(w971) -> ("Set 1"=w970:i16, "Set 2"=w969:i16)
        n606 = xnode "Read/Write Control"("FPGA VI Reference In"=w967, "error in"=w966, "FB Setpoint Set 1"=w970, "FB Setpoint Set 2"=w969) -> ("error out"=w965:errorcluster)  [unwired: 1 out]
      }
      event "Invert GI": Value Change {
        n607 = event-data() -> ()  [unwired: 7 out]
        n608 = xnode "Read/Write Control"("FPGA VI Reference In"=w1004, "error in"=w1002, "Invert GI"="Invert GI", "Invert GI 2"="Invert GI") -> ("error out"=w1003:errorcluster)  [unwired: 1 out]
      }
      event "Green FB Setpoint (mV)", "Green FB Gains", "Green FB On/Off", "Current When FB OFF (%)", "Green int current ON count adj": Value Change {
        n609 = event-data() -> ()  [unwired: 7 out]
        n610 = local read "Green FB Setpoint (mV)"() -> (w1011:dbl)
        n611 = local read "Current When FB OFF (%)"() -> (w1014:dbl)
        n612 = Multiply(x=w1011, y=3.2767) -> (x*y=w1010:dbl)
        n613 = Multiply(x=w1014, y=655.35) -> (x*y=w1015:dbl)
        n614 = To Unsigned Word Integer(number=w1015) -> (unsigned 16bit integer=w1013:u16)
        n615 = local read "Green int current ON count adj"() -> (w1018:u32)
        n616 = local read "Green FB Gains"() -> (w1017:T14)
        n617 = local read "Green Laser ON/Interlacing"() -> (w1008:bool)
        n618 = local read "Green laser mode"() -> (w1007:enum32{"Laser ON", "Laser OFF", "Interlace"})
        n619 = local read "Green FB On/Off"() -> (w1019:bool)
        n620 = Equal?(x=w1007, y=enum32{"Laser ON", "Laser OFF", "Interlace"}."Interlace") -> (x = y?=w1005:bool)
        n621 = Compound Arithmetic op=AND(w1005, w1019, w1008) -> (w1009:bool)
        n622 = xnode "Read/Write Control"("FPGA VI Reference In"=w1022, "error in"=w1021, "Green FB Setpoint"=w1010, "Green FB On/Off"=w1009, "Current Out"=w1013, "Green int current ON count adj"=w1018, "Green FB Gains"=w1017) -> ("error out"=w1020:errorcluster)  [unwired: 1 out]
      }
      event "Green laser mode", "Green Laser ON/Interlacing": Value Change {
        n623 = event-data() -> ()  [unwired: 7 out]
        n624 = case shown="True" "Green Laser ON/Interlacing" {
          tunnel: "Green laser mode" -> [_ w1036]
          tunnel: [enum32{"Laser ON", "Laser OFF", "Interlace"}."Laser OFF" ("Green laser mode") w1036] -> w1024
          tunnel: [FALSE w1032] -> w1023
          frame False {
          }
          frame True {
            n625 = local read "Green FB On/Off"() -> (w1033:bool)
            n626 = Equal?(x=w1036, y=enum32{"Laser ON", "Laser OFF", "Interlace"}."Interlace") -> (x = y?=w1034:bool)
            n627 = And(x=w1034, y=w1033) -> (x .and. y?=w1032:bool)
          }
        }
        n628 = xnode "Read/Write Control"("FPGA VI Reference In"=w1029, "error in"=w1027, "Operating Mode"=w1024, "Operating Mode 2"=w1024, "Green FB On/Off"=w1023) -> ("error out"=w1028:errorcluster)  [unwired: 1 out]
      }
      event "- phase (APD 1 Gate)", "+ phase (APD 1 Gate)": Value Change {
        n629 = event-data() -> ()  [unwired: 7 out]
        n630 = local read "Phase Adj. (APD 1 Gate)"() -> (w1037:i16)
        n631 = Negate(x=w1037) -> (-x=w1045:i16)
        n632 = Select(t=w1045, s="- phase (APD 1 Gate)", f=w1037) -> (s? t:f=w1044:i16)
        n633 = Or(x="- phase (APD 1 Gate)", y="+ phase (APD 1 Gate)") -> (x .or. y?=w1040:bool)
        n634 = xnode "Read/Write Control"("FPGA VI Reference In"=w1047, "error in"=w1046, "Phase count adjustment (APD 1 Gate)"=w1044) -> ("FPGA VI Reference Out"=w1042:T19, "error out"=w1043:errorcluster)
        n635 = xnode "Read/Write Control"("FPGA VI Reference In"=w1042, "error in"=w1043, "+ phase (APD 1 Gate)"=w1040) -> ("error out"=w1041:errorcluster)  [unwired: 1 out]
      }
      event "+ phase (APD 2 Gate)", "- phase (APD 2 Gate)": Value Change {
        n636 = event-data() -> ()  [unwired: 7 out]
        n637 = local read "Phase Adj. (APD 2 Gate)"() -> (w1048:i16)
        n638 = Negate(x=w1048) -> (-x=w1056:i16)
        n639 = Select(t=w1056, s="- phase (APD 2 Gate)", f=w1048) -> (s? t:f=w1055:i16)
        n640 = Or(x="- phase (APD 2 Gate)", y="+ phase (APD 2 Gate)") -> (x .or. y?=w1051:bool)
        n641 = xnode "Read/Write Control"("FPGA VI Reference In"=w1058, "error in"=w1057, "Phase count adjustment (APD 2 Gate)"=w1055) -> ("FPGA VI Reference Out"=w1053:T19, "error out"=w1054:errorcluster)
        n642 = xnode "Read/Write Control"("FPGA VI Reference In"=w1053, "error in"=w1054, "+ phase (APD 2 Gate)"=w1051) -> ("error out"=w1052:errorcluster)  [unwired: 1 out]
      }
      event "Phase Adj. (APD Acq)", "+ phase (APD Acq)", "- phase (APD Acq)": Value Change {
        n643 = event-data() -> ()  [unwired: 7 out]
        n644 = local read "Phase Adj. (APD Acq)"() -> (w1061:i16)
        n645 = Negate(x=w1061) -> (-x=w1067:i16)
        n646 = Select(t=w1067, s="+ phase (APD Acq)", f=w1061) -> (s? t:f=w1066:i16)
        n647 = Or(x="+ phase (APD Acq)", y="- phase (APD Acq)") -> (x .or. y?=w1062:bool)
        n648 = xnode "Read/Write Control"("FPGA VI Reference In"=w1069, "error in"=w1068, "Phase Count Adjustment (APD Acq)"=w1066) -> ("FPGA VI Reference Out"=w1064:T19, "error out"=w1065:errorcluster)
        n649 = xnode "Read/Write Control"("FPGA VI Reference In"=w1064, "error in"=w1065, "+ phase (APD Acq)"=w1062) -> ("error out"=w1063:errorcluster)  [unwired: 1 out]
      }
      event "Phase adj. (GI)", "+ phase (GI)", "- phase (GI)": Value Change {
        n650 = event-data() -> ()  [unwired: 7 out]
        n651 = Negate(x="Phase adj. (GI)") -> (-x=w1078:i16)
        n652 = Select(t=w1078, s="+ phase (GI)", f="Phase adj. (GI)") -> (s? t:f=w1077:i16)
        n653 = Or(x="+ phase (GI)", y="- phase (GI)") -> (x .or. y?=w1073:bool)
        n654 = xnode "Read/Write Control"("FPGA VI Reference In"=w1080, "error in"=w1079, "Phase count adjustment (GI)"=w1077) -> ("FPGA VI Reference Out"=w1075:T19, "error out"=w1076:errorcluster)
        n655 = xnode "Read/Write Control"("FPGA VI Reference In"=w1075, "error in"=w1076, "+ phase (GI)"=w1073) -> ("error out"=w1074:errorcluster)  [unwired: 1 out]
      }
      event "Phase adj. (GI) 2", "+ phase (GI) 2", "- phase (GI) 2": Value Change {
        n656 = event-data() -> ()  [unwired: 7 out]
        n657 = Negate(x="Phase adj. (GI) 2") -> (-x=w1089:i16)
        n658 = Select(t=w1089, s="+ phase (GI) 2", f="Phase adj. (GI) 2") -> (s? t:f=w1088:i16)
        n659 = Or(x="+ phase (GI) 2", y="- phase (GI) 2") -> (x .or. y?=w1084:bool)
        n660 = xnode "Read/Write Control"("FPGA VI Reference In"=w1091, "error in"=w1090, "Phase count adjustment (GI) 2"=w1088) -> ("FPGA VI Reference Out"=w1086:T19, "error out"=w1087:errorcluster)
        n661 = xnode "Read/Write Control"("FPGA VI Reference In"=w1086, "error in"=w1087, "+ phase (GI) 2"=w1084) -> ("error out"=w1085:errorcluster)  [unwired: 1 out]
      }
      event "Phase adj. (Green FB)", "- phase (Green FB)", "+ phase (Green FB)": Value Change {
        n662 = event-data() -> ()  [unwired: 7 out]
        n663 = Negate(x="Phase adj. (Green FB)") -> (-x=w1100:i16)
        n664 = Select(t=w1100, s="+ phase (Green FB)", f="Phase adj. (Green FB)") -> (s? t:f=w1099:i16)
        n665 = Or(x="+ phase (Green FB)", y="- phase (Green FB)") -> (x .or. y?=w1095:bool)
        n666 = xnode "Read/Write Control"("FPGA VI Reference In"=w1102, "error in"=w1101, "Phase count adjustment (Green FB)"=w1099) -> ("FPGA VI Reference Out"=w1097:T19, "error out"=w1098:errorcluster)
        n667 = xnode "Read/Write Control"("FPGA VI Reference In"=w1097, "error in"=w1098, "+ phase (Green FB)"=w1095) -> ("error out"=w1096:errorcluster)  [unwired: 1 out]
      }
      event "Invert APD Gate", "APD Gate ON Count", "APD Gate OFF Count", "APD Gate", "APD Integration Time (s)", "APD 1 AO Mult.", "APD 2 AO Mult.": Value Change {
        n668 = event-data() -> ()  [unwired: 7 out]
        n669 = local read "APD Integration Time (s)"() -> (w1103:dbl)
        n670 = local read "APD Gate ON Count"() -> (w1116:u32)
        n671 = local read "APD Gate OFF Count"() -> (w1115:u32)
        n672 = local read "Invert APD Gate"() -> (w1117:bool)
        n673 = local read "APD Gate"() -> (w1114:enum32{"ON", "OFF", "Interlace"})
        n674 = Multiply(x=w1103, y=40000000.0) -> (x*y=w1112:dbl)
        n675 = Reciprocal(x=w1103) -> (1/x=→"APD Acq Rate (Hz)":dbl)
        n676 = To Unsigned Long Integer(number=w1112) -> (unsigned 32bit integer=w1111:u32)
        n677 = local read "DMA Update Period (s)"() -> (w1104:dbl)
        n678 = Divide(x=w1104, y=w1103) -> (x/y=w1107:dbl)
        n679 = local read "APD 1 AO Mult."() -> (w1109:i16)
        n680 = local read "APD 2 AO Mult."() -> (w1108:i16)
        n681 = Multiply(x=2.0, y=w1107) -> (x*y=w1106:dbl)
        n682 = local write "APD Samples/FIFO Acq."(w1107) -> ()
        n683 = local write "APD Elements/DMA read"(w1106) -> ()
        n684 = xnode "Read/Write Control"("FPGA VI Reference In"=w1120, "error in"=w1119, "Invert APD Gate"=w1117, "APD Gate ON Count"=w1116, "APD Gate OFF Count"=w1115, "APD Acq Rate Count"=w1111, "APD Gate Operating Mode"=w1114, "APD 1 AO scale factor"=w1109, "APD 2 AO scale factor"=w1108) -> ("error out"=w1118:errorcluster)  [unwired: 1 out]
      }
      event "GI Frequency, ON count", "Green FB Count", "GI Frequency, OFF count": Value Change {
        n685 = event-data() -> ()  [unwired: 7 out]
        n686 = xnode "Read/Write Control"("FPGA VI Reference In"=w1126, "error in"=w1124, "Green interlace ON count"="GI Frequency, ON count", "Green interlace OFF count"="GI Frequency, OFF count", "Green interlace ON count 2"="GI Frequency, ON count", "Green interlace OFF count 2"="GI Frequency, OFF count", "Green FB Count"="Green FB Count") -> ("error out"=w1125:errorcluster)  [unwired: 1 out]
      }
      event "Number of F/B Scans (AOD)", "Scan Speed (nm/s)", "Scan BD", "Initial delta (MHz)", "Step Size (nm)", "Scan Range (nm)": Value Change {
        w1188 = 123.0  # AOM cal (nm/MHz)
        n687 = event-data() -> ()  [unwired: 7 out]
        n688 = local read "BD 1 Frequency 1 (MHz)"() -> (w1171:dbl)
        n689 = local read "AOM X Cal (nm/MHz)"() -> (w1163:dbl)
        n690 = local read "X RF Frequency Limits (MHz)"() -> (w1175:T16)
        n691 = local read "Y RF Frequency Limits (MHz)"() -> (w1172:T16)
        n692 = local read "BD 2 Frequency 1 (MHz)"() -> (w1177:dbl)
        n693 = Negate(x="Scan Range (nm)") -> (-x=w1141:dbl)
        n694 = Divide(x=w1141, y=w1163) -> (x/y=w1145:dbl)
        n695 = Select(t=w1175, s="Scan BD", f=w1172) -> (s? t:f=w1174:T16)
        n696 = Select(t=w1171, s="Scan BD", f=w1177) -> (s? t:f=w1176:dbl)
        n697 = Unbundle By Name(w1174) -> ("Maximum"=w1183:dbl, "Minimum"=w1182:dbl)
        n698 = Add(x=w1145, y=w1176) -> (x+y=w1180:dbl)
        n699 = Divide(x=w1141, y="Step Size (nm)") -> (x/y=w1160:dbl)
        n700 = Divide(x="Step Size (nm)", y=w1163) -> (x/y=w1169:dbl)
        n701 = Absolute Value(x=w1160) -> (abs(x)=w1144:dbl)
        n702 = Sign(1:w1141) -> (0:w1142:dbl)
        n703 = In Range and Coerce(upper limit=w1183, x=w1180, lower limit=w1182) -> (coerced(x)=w1179:dbl, In Range?=w1181:bool)
        n704 = To Unsigned Quad Integer(1:w1144) -> (0:w1159:u64)
        "Scan steps (AOD)" <- w1159
        n705 = call "IR AOM freq to word.vi"("Frequency In (MHz)"=w1169) -> ("Frequency Word Out (double)"=w1166:dbl)
        n706 = Multiply(x=w1142, y=w1166) -> (x*y=w1143:dbl)
        n707 = Subtract(x=w1180, y=w1179) -> (x-y=w1178:dbl)
        n708 = To Quad Integer(1:w1143) -> (0:w1165:i64)
        "Incr. int (AOD)" <- w1165
        n709 = Subtract(x=w1145, y=w1178) -> (x-y=w1164:dbl)
        "Scan Range (MHz)" <- w1164
        n710 = Select(t=w1145, s=w1181, f=w1164) -> (s? t:f=w1184:dbl)
        n711 = Multiply(x=w1164, y=w1163) -> (x*y=w1162:dbl)
        n712 = Decrement(x=w1159) -> (x-1=w1212:u64)
        n713 = Negate(x=w1162) -> (-x=w1158:dbl)
        n714 = local write "Scan Range (nm)"(w1158) -> ()
        n715 = Divide(x=w1184, y=w1212) -> (x/y=w1168:dbl)
        "Scan Increment (MHz)" <- w1168
        n716 = call "IR AOM freq to word.vi"("Frequency In (MHz)"=w1168) -> ("Frequency Word Out (double)"=w1167:dbl)
        n717 = Divide(x="Step Size (nm)", y="Scan Speed (nm/s)") -> (x/y=w1155:dbl)
        n718 = To Quad Integer(1:w1167) -> ()  [unwired: 1 out]
        n719 = local read "Number Interlace Sets"() -> (w1139:u8)
        n720 = local read "AI Count (ticks)"() -> (w1140:u32)
        n721 = local read "Total Counts (ticks)"() -> (w1138:u32)
        n722 = local read "# Samples/trap"() -> (w1170:u32)
        n723 = Multiply(x=w1140, y=w1139) -> (x*y=w1137:u32)
        n724 = Divide(x=w1138, y=w1137) -> (x/y=w1136:dbl)
        n725 = Select(t=w1171, s="Scan BD", f=w1177) -> (s? t:f=w1209:dbl)
        "Initial freq. (MHz)" <- w1209
        n726 = Add(x=w1184, y=w1209) -> (x+y=→"Final freq. (MHz)":dbl)
        n727 = Divide(x=w1138, y=40000000.0) -> (x/y=w1154:dbl)
        n728 = Divide(x=w1155, y=w1154) -> (x/y=w1153:dbl)
        n729 = To Unsigned Quad Integer(1:w1153) -> (0:w1128:u64)
        n730 = Quotient & Remainder(x=w1128, y=u64 2) -> (x-y*floor(x/y)=w1132:u64)  [unwired: 1 out]
        n731 = Equal?(x=w1132, y=u64 0) -> (x = y?=w1130:bool)
        n732 = Decrement(x=w1128) -> (x-1=w1129:u64)
        n733 = Select(t=w1128, s=w1130, f=w1129) -> (s? t:f=w1127:u64)
        "Cycles/step (AOD)" <- w1127
        n734 = xnode "Read/Write Control"("FPGA VI Reference In"=w1220, "error in"=w1219, "Scan steps"=w1159, "Number of scans"="Number of F/B Scans (AOD)", "Cycles per step"=w1127, "Scan freq.  increment"=w1165, "Scan BD"="Scan BD") -> ("error out"=w1218:errorcluster)  [unwired: 1 out]
        n735 = Multiply(x=w1159, y=w1127) -> (x*y=w1213:u64)
        n736 = Multiply(x=w1213, y=u64 2) -> (x*y=w1135:u64)
        n737 = Multiply(x=w1136, y=w1135) -> (x*y=w1134:dbl)
        "Data points/scan (f/b)" <- w1134
        n738 = Multiply(x=w1134, y="Number of F/B Scans (AOD)") -> (x*y=w1216:dbl)
        "Data points/scans" <- w1216
        n739 = Divide(x=w1216, y=w1170) -> (x/y=→"N sets should be saved":dbl)
        n740 = Multiply(x=w1213, y=w1154) -> (x*y=w1152:dbl)
        "Time/Scan (s) (AOD)" <- w1152
        n741 = Select(t=w1184, s="Scan BD", f=0.0) -> (s? t:f=w1210:dbl)
        n742 = Select(t=0.0, s="Scan BD", f=w1184) -> (s? t:f=w1206:dbl)
        n743 = local read "BD 2 Frequency 2 (MHz)"() -> (w1202:dbl)
        n744 = local read "BD 1 Frequency 2 (MHz)"() -> (w1205:dbl)
        n745 = Add(x=w1206, y=w1177) -> (x+y=w1203:dbl)
        n746 = Add(x=w1171, y=w1210) -> (x+y=w1204:dbl)
        n747 = Multiply(x=w1152, y=2.0) -> (x*y=w1151:dbl)
        n748 = Multiply(x=w1151, y="Number of F/B Scans (AOD)") -> (x*y=w1148:dbl)
        n749 = Divide(x=w1148, y=60.0) -> (x/y=→"Time to Finish All (min)":dbl)
        n750 = Add(x="Trap 2 Bead Size (nm)", y="Trap 1 Bead Size (nm)") -> (x+y=w1192:dbl)
        n751 = local read "Initial delta (MHz)"() -> (w1189:dbl)
        n752 = Divide(x=w1192, y=2.0) -> (x/y=w1186:dbl)
        n753 = Subtract(x=w1203, y=w1202) -> (x-y=w1200:dbl)
        n754 = Subtract(x=w1204, y=w1205) -> (x-y=w1201:dbl)
        n755 = Square(x=w1200) -> (x^2=w1199:dbl)
        n756 = Square(x=w1201) -> (x^2=w1198:dbl)
        n757 = Add(x=w1198, y=w1199) -> (x+y=w1197:dbl)
        n758 = Square Root(x=w1197) -> (sqrt(x)=w1196:dbl)
        "Final delta (MHz)" <- w1196
        n759 = Multiply(x=w1188, y=w1196) -> (x*y=w1195:dbl)
        n760 = Multiply(x=w1189, y=w1188) -> (x*y=w1187:dbl)
        n761 = Subtract(x=w1187, y=w1186) -> (x-y=→"Initial sep (nm)":dbl)
        n762 = Subtract(x=w1195, y=w1186) -> (x-y=→"Final sep (nm)":dbl)
      }
      event "Raster Scanning...": Value Change {
        n763 = event-data() -> ("NewVal"=w1221:bool)  [unwired: 6 out]
        n764 = case shown="True" w1221 {
          frame False {
          }
          frame True {
            n765 = property on="BD 1 Frequency 1 (MHz)" class="DigNum (strict)"("Val(Sgnl)"=65.0 ("Value (Signaling)")) -> ()  [unwired: 2 in, 2 out]
          }
        }
      }
      event "Freq or Amp switch first", "Swap F1 and F2", "Freq switch delay", "Amp switch delay": Value Change {
        n766 = event-data() -> ()  [unwired: 7 out]
        n767 = local read "Freq or Amp switch first"() -> (w1223:bool)
        n768 = local read "Amp switch delay"() -> (w1224:u16)
        n769 = local read "Freq switch delay"() -> (w1226:u16)
        n770 = local read "Swap F1 and F2"() -> (w1225:bool)
        n771 = xnode "Read/Write Control"("FPGA VI Reference In"=w1229, "error in"=w1228, "Freq switch delay"=w1226, "Swap F1 and F2"=w1225, "Amp switch delay"=w1224, "Freq or Amp switch first"=w1223) -> ("error out"=w1227:errorcluster)  [unwired: 1 out]
      }
      event "Scan steps (MCL)", "Number of scans (MCL)", "Scan Range (V)\n(of steps)", "2D or 1D Scan", "N APD Samp/step", "Fast Scan Dir", "Continuous MCL Scanning", "Scan lines (y)": Value Change {
        w1231 = 32767.0 ("y")
        n772 = event-data() -> ()  [unwired: 7 out]
        n773 = Select(t="Scan lines (y)", s="2D or 1D Scan", f="Number of scans (MCL)") -> (s? t:f=w1236:u64)
        n774 = Decrement(x="Scan steps (MCL)") -> (x-1=w1252:u64)
        n775 = Divide(x="Scan Range (V)\n(of steps)", y=w1252) -> (x/y=w1251:dbl)
        "Desired Scan Incr (V)" <- w1251
        n776 = local read "APD Integration Time (s)"() -> (w1244:dbl)
        n777 = Multiply(x=w1251, y=w1231) -> (x*y=w1260:dbl)
        n778 = Divide(x=w1260, y=10.0) -> (x/y=w1250:dbl)
        "Desired incr (int)" <- w1250
        n779 = local read "Update Count (MCL)"() -> (w1256:u32)
        n780 = Round Toward -Infinity(1:w1250) -> (0:w1259:dbl)
        n781 = To Word Integer(number=w1259) -> (16bit integer=w1234:i16)
        "Actual Incr. int (MCL)" <- w1234
        n782 = Multiply(x=w1244, y=40000000.0) -> (x*y=w1257:dbl)
        n783 = Divide(x=w1257, y=w1256) -> (x/y=w1255:dbl)
        n784 = Multiply(x=i16 10, y=w1234) -> (x*y=w1232:i16)
        n785 = Multiply(x="N APD Samp/step", y=w1255) -> (x*y=w1254:dbl)
        "Cycles/step (MCL)" <- w1254
        n786 = Divide(x=w1232, y=w1231) -> (x/y=→"Actual MCL Inc (V)":dbl)
        n787 = Multiply(x="N APD Samp/step", y="Scan steps (MCL)") -> (x*y=w1246:dbl)
        n788 = local read "APD Samples/FIFO Acq."() -> (w1243:dbl)
        n789 = Multiply(x=w1246, y=u64 2) -> (x*y=w1245:dbl)
        "Data points/scan (f+b)" <- w1245
        n790 = Multiply(x=w1245, y=w1236) -> (x*y=w1263:dbl)
        "Data points/scans (MCL)" <- w1263
        n791 = Multiply(x=w1244, y=w1245) -> (x*y=w1237:dbl)
        "Time/f+b scan (s) (MCL)" <- w1237
        n792 = Divide(x=w1263, y=w1243) -> (x/y=→"N sets should be saved (MCL)":dbl)
        n793 = Multiply(x=w1237, y=w1236) -> (x*y=→"Total Time (s)":dbl)
        n794 = Not(x="Fast Scan Dir") -> (.not. x?=w1241:bool)
        n795 = xnode "Read/Write Control"("FPGA VI Reference In"=w1267, "error in"=w1266, "Scan steps (MCL)"="Scan steps (MCL)", "Number of scans (MCL)"=w1236, "Cycles per step (MCL)"=w1254, "Scan freq.  increment (MCL)"=w1234, "1D or 2D Scan?"="2D or 1D Scan", "MCL Scan Axis"=w1241, "Cont. Scan (MCL)"="Continuous MCL Scanning") -> ("error out"=w1265:errorcluster)  [unwired: 1 out]
      }
      event "Read Cal": Value Change {
        w1269 = 1000.0 ("y")
        n796 = event-data() -> ()  [unwired: 7 out]
        n797 = local read "Save file name"() -> (w1294:path)
        n798 = local write "Read Cal"(FALSE ("Read Cal")) -> ()
        n799 = Strip Path(path=w1294) -> (stripped path=w1293:path)  [unwired: 1 out]
        n800 = Path To String(path=w1293) -> (string=w1292:string)
        n801 = Concatenate Strings(w1292, "\\current.cal" ("string")) -> (w1290:string)
        n802 = String To Path(string=w1290) -> (path=w1289:path)
        n803 = Open/Create/Replace File(file path (use dialog)=w1289, operation (0:open)=T22."open", access (0:read/write)=enum16{"read/write", "read-only", "write-only"}."read-only") -> (refnum out=w1297:refnum<file>, error out=w1283:errorcluster)  [unwired: 1 in, 3 out]
        n804 = Deny Access(4:w1283, 7:w1297) -> (0:w1282:errorcluster, 3:w1288:refnum<file>)  [unwired: 1 out]
        n805 = Read from Binary File(5:0.0, 8:w1282, 9:T29."big-endian, network order" ("byte order (0:big-endian, network order)"), 10:-1 ("count (1)"), 11:w1288) -> (0:w1281:errorcluster, 2:w1279:dbl[], 3:w1284:refnum<file>)  [unwired: 2 out]
        n806 = Array To Cluster(array=w1279) -> (cluster=w1278:T31)
        n807 = Unbundle(w1278) -> ("[0]"=w1277:dbl, "[1]"=w1276:dbl, "[2]"=w1275:dbl, "[3]"=w1274:dbl, "[4]"=w1273:dbl, "[5]"=w1272:dbl)
        n808 = Close File(refnum=w1284, error in=w1281) -> (error out=→"Read cal error":errorcluster)  [unwired: 1 out]
        n809 = Multiply(x=w1272, y=w1269) -> (x*y=w1270:dbl)
        n810 = local write "T2 kappa_x (pN/nm)"(w1274) -> ()
        n811 = local write "T1 kappa_x (pN/nm)"(w1275) -> ()
        n812 = local write "T1 alpha_x (nm/V)"(w1277) -> ()
        n813 = local write "T2 alpha_x (nm/V)"(w1276) -> ()
        n814 = Multiply(x=w1273, y=w1269) -> (x*y=w1271:dbl)
        n815 = local write "T1 offset_x (mV)"(w1271) -> ()
        n816 = local write "T2 offset_x (mV)"(w1270) -> ()
      }
      event "Abort MCL Scan": Value Change {
        n817 = event-data() -> ()  [unwired: 7 out]
        n818 = local write "MCL Scanning"(FALSE ("MCL Scanning")) -> ()
        n819 = xnode "Read/Write Control"("FPGA VI Reference In"=w1302, "error in"=w1301, "Abort scan (MCL)"="Abort MCL Scan") -> ("error out"=w1300:errorcluster)  [unwired: 1 out]
      }
      event "Update Count (MCL)": Value Change {
        n820 = event-data() -> ()  [unwired: 7 out]
        n821 = xnode "Read/Write Control"("FPGA VI Reference In"=w1306, "error in"=w1305, "MCL count"="Update Count (MCL)") -> ("error out"=w1304:errorcluster)  [unwired: 1 out]
      }
      event "Phase adjust (MCL)", "+ phase (MCL)", "- phase (MCL)": Value Change {
        n822 = event-data() -> ()  [unwired: 7 out]
        n823 = Negate(x="Phase adjust (MCL)") -> (-x=w1315:i16)
        n824 = Select(t=w1315, s="- phase (MCL)", f="Phase adjust (MCL)") -> (s? t:f=w1313:i16)
        n825 = Or(x="- phase (MCL)", y="+ phase (MCL)") -> (x .or. y?=w1308:bool)
        n826 = xnode "Read/Write Control"("FPGA VI Reference In"=w1317, "error in"=w1316, "Phase count adjustment (MCL)"=w1313) -> ("FPGA VI Reference Out"=w1309:T19, "error out"=w1310:errorcluster)
        n827 = xnode "Read/Write Control"("FPGA VI Reference In"=w1309, "error in"=w1310, "+ phase (MCL)"=w1308) -> ("error out"=w1307:errorcluster)  [unwired: 1 out]
      }
      event "Abort AOD Scan": Value Change {
        n828 = event-data() -> ()  [unwired: 7 out]
        n829 = xnode "Read/Write Control"("FPGA VI Reference In"=w1321, "error in"=w1320, "Abort scan"="Abort AOD Scan") -> ("error out"=w1319:errorcluster)  [unwired: 1 out]
      }
      event "Continuous AOD Scanning": Value Change {
        n830 = event-data() -> ()  [unwired: 7 out]
        n831 = xnode "Read/Write Control"("FPGA VI Reference In"=w1325, "error in"=w1324, "Cont. Scan"="Continuous AOD Scanning") -> ("error out"=w1323:errorcluster)  [unwired: 1 out]
      }
      event "Index": Value Change {
        n832 = event-data() -> ()  [unwired: 7 out]
        n833 = call "Create new save file.vi"("Insert"="", "Ext"=".dat" ("string"), "Index In"="Index") -> ("Path Out"=→"Save file name":path, "Index Out"=w1326:dbl)
        "Save index" <- w1326
        n834 = local write "Index"(w1326) -> ()
      }
      event "AO1", "AO2": Value Change {
        w1341 = 10.0 ("y")
        w1340 = 32767.0 ("y")
        n835 = event-data() -> ()  [unwired: 7 out]
        n836 = local read "AO2"() -> (w1339:dbl)
        n837 = local read "AO1"() -> (w1336:dbl)
        n838 = Multiply(x=w1336, y=w1340) -> (x*y=w1335:dbl)
        n839 = Multiply(x=w1339, y=w1340) -> (x*y=w1338:dbl)
        n840 = Divide(x=w1335, y=w1341) -> (x/y=w1334:dbl)
        n841 = Divide(x=w1338, y=w1341) -> (x/y=w1337:dbl)
        n842 = To Word Integer(number=w1334) -> (16bit integer=w1342:i16)
        n843 = To Word Integer(number=w1337) -> (16bit integer=w1343:i16)
        n844 = xnode "Read/Write Control"("FPGA VI Reference In"=w1333, "error in"=w1332, "AO1"=w1342, "AO2"=w1343) -> ("error out"=w1331:errorcluster)  [unwired: 1 out]
      }
      event "Inject Bottom": Value Change {
        n845 = event-data() -> ()  [unwired: 7 out]
        n846 = disable-structure shown="Enabled" {
          disable-tunnel: "Inject Bottom" -> [w1345 w1385]
          frame Disabled {
            n847 = local read "Chemyx Syringe Pump Serial Port"() -> (w1346:refnum<visa-resource-name>)
            n848 = local read "Pump write delay (ms)"() -> (w1347:dbl)
            n849 = case shown="True" w1345 {
              tunnel: w1347 -> [w1353 w1367]
              tunnel: w1346 -> [w1350 w1366]
              frame False {
                n850 = flat-sequence {
                  tunnel: w1350 -> [w1354]
                  tunnel: [w1354] -> w1351
                  tunnel: w1353 -> [_]
                  tunnel: [w1357] -> w1352
                  tunnel: w1351 -> [w1357]
                  tunnel: w1352 -> [w1358]
                  tunnel: [w1358] -> w1348
                  tunnel: [w1360] -> w1349
                  tunnel: w1348 -> [w1360]
                  tunnel: w1349 -> [w1362]
                  frame #0 {
                    n851 = call "Write to pump.vi"("string"="enter pump1", "VISA resource name"=w1354) -> ()  [unwired: 1 out]
                  }
                  frame #1 {
                    n852 = Wait (ms)(milliseconds to wait="Pump pause delay (ms)") -> ()  [unwired: 1 out]
                  }
                  frame #2 {
                    n853 = call "Write to pump.vi"("string"="stop", "VISA resource name"=w1358) -> ()  [unwired: 1 out]
                  }
                  frame #3 {
                    n854 = Wait (ms)(milliseconds to wait=u32 500) -> ()  [unwired: 1 out]
                  }
                  frame #4 {
                    n855 = call "Write to pump.vi"("string"="stop", "VISA resource name"=w1362) -> ()  [unwired: 1 out]
                  }
                }
              }
              frame True {
                n856 = flat-sequence {
                  tunnel: w1366 -> [w1376]
                  tunnel: w1367 -> [w1371]
                  tunnel: w1367 -> [w1378]
                  tunnel: w1366 -> [w1379]
                  tunnel: [w1379] -> w1364
                  tunnel: [w1381] -> w1365
                  tunnel: w1364 -> [w1381]
                  tunnel: w1365 -> [w1383]
                  frame #0 {
                    n857 = local read "All Pump Parameters"() -> (w1370:T5)
                    n858 = Unbundle By Name(w1370) -> ("Pump 1"=w1377:T32)
                    n859 = call "Set pump parameters.vi"("Pump write delay (ms)"=w1371, "Volume (uL)"="Ch 2 Inject Volume (uL)", "Rate (uL/h)"="Ch 1 Inject Rate (ul/h)", "Units"=4.0, "Pump #"=1.0, "Pump Parameters In"=w1377, "VISA resource name"=w1376) -> ("Pump Parameters Out"=w1369:T32)  [unwired: 3 in]
                    n860 = Bundle By Name(cluster=w1370, "Pump 1"=w1369) -> (w1368:T5)
                    n861 = local write "All Pump Parameters"(w1368) -> ()
                  }
                  frame #1 {
                    n862 = Wait (ms)(milliseconds to wait=w1378) -> ()  [unwired: 1 out]
                  }
                  frame #2 {
                    n863 = call "Write to pump.vi"("string"="start", "VISA resource name"=w1379) -> ()  [unwired: 1 out]
                  }
                  frame #3 {
                    n864 = Wait (ms)(milliseconds to wait=u32 500) -> ()  [unwired: 1 out]
                  }
                  frame #4 {
                    n865 = call "Write to pump.vi"("string"="start", "VISA resource name"=w1383) -> ()  [unwired: 1 out]
                  }
                }
              }
            }
          }
          frame Enabled {
            n866 = call "hamilton_controller.vi"("Open?"=w1385, "valve"=enum16{"A", "B", "C", "D", "ALL"}."B", "action"=T20."MOVE VALVE") -> ()  [unwired: 8 in, 1 out]
          }
        }
      }
      event "Inject Top": Value Change {
        n867 = event-data() -> ()  [unwired: 7 out]
        n868 = disable-structure shown="Disabled" {
          disable-tunnel: "Inject Top" -> [_ w1429]
          frame Disabled {
            n869 = local read "Pump write delay (ms)"() -> (w1390:dbl)
            n870 = case shown="False" w1391 {
              tunnel: w1390 -> [w1397 w1411]
              tunnel: "Chemyx Syringe Pump Serial Port" -> [w1394 w1410]
              frame False {
                n871 = flat-sequence {
                  tunnel: w1394 -> [w1398]
                  tunnel: [w1398] -> w1395
                  tunnel: w1397 -> [_]
                  tunnel: [w1401] -> w1396
                  tunnel: w1395 -> [w1401]
                  tunnel: w1396 -> [w1402]
                  tunnel: [w1402] -> w1392
                  tunnel: [w1404] -> w1393
                  tunnel: w1392 -> [w1404]
                  tunnel: w1393 -> [w1406]
                  frame #0 {
                    n872 = call "Write to pump.vi"("string"="enter pump3", "VISA resource name"=w1398) -> ()  [unwired: 1 out]
                  }
                  frame #1 {
                    n873 = local read "Pump pause delay (ms)"() -> (w1400:u32)
                    n874 = Wait (ms)(milliseconds to wait=w1400) -> ()  [unwired: 1 out]
                  }
                  frame #2 {
                    n875 = call "Write to pump.vi"("string"="stop", "VISA resource name"=w1402) -> ()  [unwired: 1 out]
                  }
                  frame #3 {
                    n876 = Wait (ms)(milliseconds to wait=u32 0) -> ()  [unwired: 1 out]
                  }
                  frame #4 {
                    n877 = call "Write to pump.vi"("string"="stop", "VISA resource name"=w1406) -> ()  [unwired: 1 out]
                  }
                }
              }
              frame True {
                n878 = flat-sequence {
                  tunnel: w1410 -> [w1420]
                  tunnel: w1411 -> [w1415]
                  tunnel: w1411 -> [w1422]
                  tunnel: w1410 -> [w1423]
                  tunnel: [w1423] -> w1408
                  tunnel: [w1426] -> w1409
                  tunnel: w1408 -> [w1426]
                  tunnel: w1409 -> [w1427]
                  frame #0 {
                    n879 = local read "All Pump Parameters"() -> (w1414:T5)
                    n880 = Unbundle By Name(w1414) -> ("Pump 3"=w1421:T32)
                    n881 = call "Set pump parameters.vi"("Pump write delay (ms)"=w1415, "Volume (uL)"="Ch 3 Inject Volume (uL)", "Rate (uL/h)"="Ch 3 Inject Rate (ul/h)", "Units"=4.0, "Pump #"=3.0, "Pump Parameters In"=w1421, "VISA resource name"=w1420) -> ("Pump Parameters Out"=w1413:T32)  [unwired: 3 in]
                    n882 = Bundle By Name(cluster=w1414, "Pump 3"=w1413) -> (w1412:T5)
                    n883 = local write "All Pump Parameters"(w1412) -> ()
                  }
                  frame #1 {
                    n884 = Wait (ms)(milliseconds to wait=w1422) -> ()  [unwired: 1 out]
                  }
                  frame #2 {
                    n885 = call "Write to pump.vi"("string"="start", "VISA resource name"=w1423) -> ()  [unwired: 1 out]
                  }
                  frame #3 {
                    n886 = Wait (ms)(milliseconds to wait=u32 500) -> ()  [unwired: 1 out]
                  }
                  frame #4 {
                    n887 = call "Write to pump.vi"("string"="start", "VISA resource name"=w1427) -> ()  [unwired: 1 out]
                  }
                }
              }
            }
          }
          frame Enabled {
            n888 = call "hamilton_controller.vi"("Open?"=w1429, "valve"=enum16{"A", "B", "C", "D", "ALL"}."A", "action"=T20."MOVE VALVE") -> ()  [unwired: 8 in, 1 out]
          }
        }
      }
      event "Inject Valve B": Value Change {
        n889 = event-data() -> ()  [unwired: 7 out]
        n890 = disable-structure shown="Enabled" {
          disable-tunnel: "Inject Valve B" -> [w1433 w1453]
          frame Disabled {
            n891 = local read "Pump write delay (ms)"() -> (w1435:dbl)
            n892 = flat-sequence {
              tunnel: w1434 -> [w1448]
              tunnel: w1435 -> [w1444]
              tunnel: w1433 -> [_]
              tunnel: w1435 -> [w1450]
              tunnel: w1434 -> [w1451]
              frame #0 {
                n893 = local read "All Pump Parameters"() -> (w1443:T5)
                n894 = Multiply(x=60.0, y="Flush Center Ch Rate (ul/m)") -> (x*y=w1440:dbl)
                n895 = Unbundle By Name(w1443) -> ("Pump 2"=w1449:T32)
                n896 = call "Set pump parameters.vi"("Pump write delay (ms)"=w1444, "Volume (uL)"="Flush Center Ch Volume (uL)", "Rate (uL/h)"=w1440, "Units"=3.0, "Pump #"=2.0, "Pump Parameters In"=w1449, "VISA resource name"=w1448) -> ("Pump Parameters Out"=w1442:T32)  [unwired: 3 in]
                n897 = Bundle By Name(cluster=w1443, "Pump 2"=w1442) -> (w1441:T5)
                n898 = local write "All Pump Parameters"(w1441) -> ()
                n899 = Add(x="Flush Center Ch Volume (uL)", y="Total Volume\nFlushed (uL)") -> (x+y=w1437:dbl)
                n900 = local write "Total Volume\nFlushed (uL)"(w1437) -> ()
              }
              frame #1 {
                n901 = Wait (ms)(milliseconds to wait=w1450) -> ()  [unwired: 1 out]
              }
              frame #2 {
                n902 = call "Write to pump.vi"("string"="start", "VISA resource name"=w1451) -> ()  [unwired: 1 out]
              }
            }
            n903 = local read "Chemyx Syringe Pump Serial Port"() -> (w1434:refnum<visa-resource-name>)
          }
          frame Enabled {
            n904 = call "hamilton_controller.vi"("Open?"=w1453, "valve"=enum16{"A", "B", "C", "D", "ALL"}."B", "action"=T20."MOVE VALVE") -> ()  [unwired: 8 in, 1 out]
          }
        }
      }
      event "Sample Channel Flow": Value Change {
        n905 = event-data() -> ()  [unwired: 7 out]
        n906 = call "hamilton_controller.vi"("Open?"="Sample Channel Flow", "valve"=enum16{"A", "B", "C", "D", "ALL"}."C", "action"=T20."MOVE VALVE") -> ()  [unwired: 8 in, 1 out]
      }
      event "Flip Green Filter": Value Change {
        n907 = event-data() -> ()  [unwired: 7 out]
        n908 = Not(x="Flip Green Filter") -> (.not. x?=w1459:bool)
        n909 = local write "Flip Green Filter"(w1459) -> ()
        n910 = flat-sequence {
          tunnel: w1467 -> [w1472]
          tunnel: w1466 -> [w1471]
          tunnel: [w1469] -> w1464
          tunnel: [w1468] -> w1463
          tunnel: [w1474] -> w1462
          tunnel: w1464 -> [w1474]
          tunnel: [w1473] -> w1461
          tunnel: w1463 -> [w1473]
          tunnel: w1462 -> [w1478]
          tunnel: w1461 -> [w1477]
          tunnel: [w1476] -> w1465
          frame #0 {
            n911 = xnode "Read/Write Control"("FPGA VI Reference In"=w1472, "error in"=w1471, "Green Filter Flipper"=TRUE) -> ("FPGA VI Reference Out"=w1469:T19, "error out"=w1468:errorcluster)
          }
          frame #1 {
            n912 = Wait (ms)(milliseconds to wait=u32 100) -> ()  [unwired: 1 out]
          }
          frame #2 {
            n913 = xnode "Read/Write Control"("FPGA VI Reference In"=w1478, "error in"=w1477, "Green Filter Flipper"=FALSE) -> ("error out"=w1476:errorcluster)  [unwired: 1 out]
          }
        }
      }
      event "Pump 1 contents", "Pump 3 contents": Value Change {
        n914 = event-data() -> ()  [unwired: 7 out]
        n915 = local read "Pump 1 contents"() -> (→"Pump 1 cont disp":string)
        n916 = local read "Pump 3 contents"() -> (→"Pump 3 cont disp":string)
      }
      event "Reset Trap Pos. FB": Value Change {
        n917 = event-data() -> ()  [unwired: 7 out]
        n918 = xnode "Read/Write Control"("FPGA VI Reference In"=w1484, "error in"=w1483, "Trap Pos. FB Reset"="Reset Trap Pos. FB") -> ()  [unwired: 2 out]
      }
      event "Trap Pos. FB ON": Value Change {
        n919 = event-data() -> ()  [unwired: 7 out]
        n920 = xnode "Read/Write Control"("FPGA VI Reference In"=w1487, "error in"=w1486, "Force feedback"="Trap Pos. FB ON") -> ()  [unwired: 2 out]
      }
      event "Trap Pos. FB Range", "Trap Pos. FB Gains", "Trap Pos. FB Mult Factor", "Trap Pos. FB Offset Factor", "Trap Pos FB Negate Action", "Trap Pos FB Monitor\nT1 or T2": Value Change {
        n921 = event-data() -> ()  [unwired: 7 out]
        n922 = xnode "Read/Write Control"("FPGA VI Reference In"=w1496, "error in"=w1495, "Trap Pos. FB Range"="Trap Pos. FB Range", "Trap Pos. FB Gains"="Trap Pos. FB Gains", "Trap Pos. FB Mult Factor"="Trap Pos. FB Mult Factor", "Trap Pos. FB Offset Factor"="Trap Pos. FB Offset Factor", "Trap Pos FB Negate Action"="Trap Pos FB Negate Action", "Trap Pos FB Monitor T1 or T2"="Trap Pos FB Monitor\nT1 or T2", "AI1 X Scale"="Trap Pos. AI1 X Pre-scale") -> ()  [unwired: 2 out]
      }
      event "Trap Pos FB SP": Value Change {
        n923 = event-data() -> ()  [unwired: 7 out]
        n924 = xnode "Read/Write Control"("FPGA VI Reference In"=w1499, "error in"=w1498, "Trap Pos. FB SP"="Trap Pos FB SP") -> ()  [unwired: 2 out]
      }
      event "Set SP to Reading": Value Change {
        n925 = event-data() -> ()  [unwired: 7 out]
        n926 = local read "Trap Pos FB Monitor\nT1 or T2"() -> (w1507:bool)
        n927 = local read "Trap X AI1 (DMA)"() -> (w1510:T13)
        n928 = local read "Trap X (AI1)"() -> (w1513:T10)
        n929 = Unbundle By Name(w1513) -> ("Trap 1"=w1512:fxp<+/-,16,1>, "Trap 2"=w1511:fxp<+/-,16,1>)
        n930 = Unbundle By Name(w1510) -> ("Set 1"=w1509:fxp<+/-,16,1>, "Set 2"=w1508:fxp<+/-,16,1>)
        n931 = Select(t=w1512, s=w1507, f=w1511) -> (s? t:f=w1506:fxp<+/-,16,1>)
        n932 = Select(t=w1509, s=w1507, f=w1508) -> (s? t:f=w1505:fxp<+/-,16,1>)
        n933 = Not(x="Set SP Using...") -> (.not. x?=w1500:bool)
        n934 = Select(t=w1506, s=w1500, f=w1505) -> (s? t:f=w1501:fxp<+/-,16,1>)
        n935 = xnode "Read/Write Control"("FPGA VI Reference In"=w1503, "error in"=w1502, "Trap Pos. FB SP"=w1501) -> ()  [unwired: 2 out]
        n936 = local write "Trap Pos FB SP"(w1501) -> ()
      }
      event "Trap Pos. FB Out Scale 2^n": Value Change {
        n937 = event-data() -> ()  [unwired: 7 out]
        n938 = Scale By Power Of 2(n="Trap Pos. FB Out Scale 2^n", x=ext 1.0) -> (x*2^n=w1515:ext)
        n939 = property on="Trap Pos. FB Mult Factor" class="DigNum (strict)"("Val(Sgnl)"=w1515) -> ()  [unwired: 2 in, 2 out]
      }
      event "Trap Pos FB Int Count": Value Change {
        n940 = event-data() -> ()  [unwired: 7 out]
        n941 = xnode "Read/Write Control"("FPGA VI Reference In"=w1520, "error in"=w1519, "Trap Pos FB Int Count"="Trap Pos FB Int Count") -> ()  [unwired: 2 out]
      }
    }
    "error out 2" <- w703
    n942 = node-c288() -> ()  [unwired: 1 in, 1 out]
  }
  n943 = timed-loop "Run Scripts, including: stage motion" {
    timing: w69 -> [_]
    timing-out: [_] -> w68
    tunnel: w24 -> [_]
    stop <- w1522 stop-if-true
    n944 = node-c288() -> ()  [unwired: 1 in, 1 out]
    n945 = event shown="[6] \"Got ADig bead\": Value Change" {
      selector: _ -> [_ _ _ _ _ _ _ _ _ _ _ _]
      dyn-events: _ -> [_ _ _ _ _ _ _ _ _ _ _ _]
      timeout: 50 -> [_ _ _ _ _ _ _ _ _ _ _ _]
      tunnel: ["Move Cap. 1 (DNA Top)" _ "Cal/Data Acq. Spot" "Dump Beads" "Dip for Protein" _ "Got ADig bead" "Got DNA bead" "Take Stepping Data" _ "Take Detection Laser\nImage" _] -> _
      tunnel: [_ _ _ _ _ _ _ _ _ _ _ w1726] -> w1522
      event "Move Cap. 1 (DNA Top)": Value Change {
        n946 = event-data() -> ()  [unwired: 1 in, 5 out]
        n947 = local write "Move Cap. 1 (DNA Top)"(FALSE ("Move Cap. 1 (DNA Right)")) -> ()
        n948 = flat-sequence {
          tunnel: "Cap 1 Samp Flow ON" -> [w1528]
          frame #0 {
            n949 = local write "Stage Moving"(FALSE ("Stage Moving")) -> ()
            n950 = case "stop flow" shown="True" w1528 {
              frame False {
              }
              frame True {
                n951 = call "hamilton_controller.vi"("Open?"=FALSE, "valve"=enum16{"A", "B", "C", "D", "ALL"}."C", "action"=T20."MOVE VALVE") -> ()  [unwired: 8 in, 1 out]
              }
            }
            n952 = case shown="True" TRUE {
              tunnel: "Cap 1 T ON" -> [w1537 w1538]
              frame False {
                n953 = property on="Trap 1 (ON/OFF)" class="Bool (strict)"("Val(Sgnl)"=w1537) -> ()  [unwired: 2 in, 2 out]
              }
              frame True {
                n954 = property on="Trap 2 (ON/OFF)" class="Bool (strict)"("Val(Sgnl)"=w1538) -> ()  [unwired: 2 in, 2 out]
              }
            }
            n955 = call <vilib>:"Beep.vi"() -> ()  [unwired: 3 in, 9 out]
            n956 = case shown="True" "Cap 1 Flow ON" {
              frame False {
              }
              frame True {
                n957 = property on="Inject Top" class="Bool (strict)"("Val(Sgnl)"=TRUE ("Value (Signaling)")) -> ()  [unwired: 2 in, 2 out]
              }
            }
          }
        }
      }
      event Timeout {
        n958 = event-data() -> ()  [unwired: 1 in, 2 out]
      }
      event "Cal/Data Acq. Spot": Value Change {
        # "wait for calibration file\nto be written"
        # "signal save cal true\nthis tells the data \nacquisition loop to\nstart sending the data\nto a calibration file"
        # "separate traps to\nthe desired trap delta"
        # "move stage to data acquisition spot"
        # "CHANGE FISH FOR TETHER BACK\nTO TRUE VALUE HERE."
        n959 = event-data() -> ()  [unwired: 1 in, 5 out]
        n960 = local write "Cal/Data Acq. Spot"(FALSE ("Cal/Data Acq. Spot")) -> ()
        n961 = flat-sequence {
          tunnel: ["Cal @ (MHz)"] -> w1539
          tunnel: w1539 -> [w1549]
          tunnel: w1539 -> [w1570]
          frame #0 {
            n962 = property on="Trap Delta (MHz)" class="DigNum (strict)"("Val(Sgnl)"="Cal @ (MHz)") -> ()  [unwired: 2 in, 2 out]
            n963 = call <vilib>:"Beep.vi"() -> ()  [unwired: 3 in, 9 out]
          }
          frame #1 {
            n964 = Wait (ms)(milliseconds to wait=u32 100) -> ()  [unwired: 1 out]
          }
          frame #2 {
            n965 = property on="Save Calibration" class="Bool (strict)"("Val(Sgnl)"=TRUE ("Value (Signaling)")) -> ()  [unwired: 2 in, 2 out]
          }
          frame #3 {
            n966 = Wait (ms)(milliseconds to wait=u32 4000) -> ()  [unwired: 1 out]
          }
          frame #4 {
            n967 = while {
              stop <- w1546 stop-if-true
              n968 = local read "Saving..."() -> (w1547:bool)
              n969 = Wait (ms)(milliseconds to wait=u32 100) -> ()  [unwired: 1 out]
              n970 = Not(x=w1547) -> (.not. x?=w1546:bool)
            }
          }
          frame #5 {
            n971 = case shown="True" "W/ Offset 1" {
              tunnel: w1549 -> [_ w1551]
              frame False {
              }
              frame True {
                n972 = stacked-sequence {
                  tunnel: w1551 -> [_ _ _ _ _ _ _ w1568]
                  frame #0 {
                    n973 = Replace Array Subset(array=u32[] [0] ("Index Values"), new element="Offset 1 Set", index=0) -> (w1552:u32[])
                    n974 = property on="Saved AOD Raster Scan Parameter Sets" class="Arr (strict)"("Index Values"=w1552) -> ()  [unwired: 2 in, 2 out]
                    n975 = property on="Trap Delta (MHz)" class="DigNum (strict)"("Val(Sgnl)"="Offset 1 Start (MHz)") -> ()  [unwired: 2 in, 2 out]
                  }
                  frame #1 {
                    n976 = Wait (ms)(milliseconds to wait=u32 200) -> ()  [unwired: 1 out]
                  }
                  frame #2 {
                    n977 = property on="Load parameters" class="Bool (strict)"("Val(Sgnl)"=TRUE ("Value (Signaling)")) -> ()  [unwired: 2 in, 2 out]
                  }
                  frame #3 {
                    n978 = Wait (ms)(milliseconds to wait=u32 200) -> ()  [unwired: 1 out]
                  }
                  frame #4 {
                    n979 = property on="Trap Raster Scan" class="Bool (strict)"("Val(Sgnl)"=TRUE ("Value (Signaling)")) -> ()  [unwired: 2 in, 2 out]
                  }
                  frame #5 {
                    n980 = Wait (ms)(milliseconds to wait=u32 2000) -> ()  [unwired: 1 out]
                  }
                  frame #6 {
                    n981 = while {
                      stop <- w1565 stop-if-true
                      n982 = local read "Raster Scanning..."() -> (w1567:bool)
                      n983 = local read "Saving..."() -> (w1563:bool)
                      n984 = Wait (ms)(milliseconds to wait=u32 100) -> ()  [unwired: 1 out]
                      n985 = Not(x=w1563) -> (.not. x?=w1562:bool)
                      n986 = Not(x=w1567) -> (.not. x?=w1564:bool)
                      n987 = And(x=w1564, y=w1562) -> (x .and. y?=w1565:bool)
                    }
                  }
                  frame #7 {
                    n988 = property on="Trap Delta (MHz)" class="DigNum (strict)"("Val(Sgnl)"=w1568) -> ()  [unwired: 2 in, 2 out]
                  }
                }
              }
            }
          }
          frame #6 {
            n989 = local read "Save ave N"() -> (w1569:dbl)
            n990 = case shown="True" "W/ Offset 2" {
              tunnel: w1570 -> [_ w1576]
              tunnel: w1569 -> [_ w1575]
              frame False {
                n991 = Multiply(x="Cal read wait (s)", y=u32 1000 ("milliseconds to wait")) -> (x*y=w1573:u32)
                n992 = Wait (ms)(milliseconds to wait=w1573) -> ()  [unwired: 1 out]
              }
              frame True {
                n993 = stacked-sequence {
                  tunnel: w1576 -> [_ _ _ _ _ _ _ _ _ w1597 _ _]
                  tunnel: w1575 -> [_ _ _ _ _ _ _ _ _ w1595 _ _]
                  frame #0 {
                    n994 = property on="Save ave N" class="DigNum (strict)"("Val(Sgnl)"=1.0 ("Value (Signaling)")) -> ()  [unwired: 2 in, 2 out]
                  }
                  frame #1 {
                    n995 = Wait (ms)(milliseconds to wait=u32 500) -> ()  [unwired: 1 out]
                  }
                  frame #2 {
                    n996 = property on="Trap Delta (MHz)" class="DigNum (strict)"("Val(Sgnl)"="Offset 2 Start (MHz)") -> ()  [unwired: 2 in, 2 out]
                    n997 = Replace Array Subset(array=u32[] [0] ("Index Values"), new element="Offset 2 Set", index=0) -> (w1581:u32[])
                    n998 = property on="Saved AOD Raster Scan Parameter Sets" class="Arr (strict)"("Index Values"=w1581) -> ()  [unwired: 2 in, 2 out]
                  }
                  frame #3 {
                    n999 = Wait (ms)(milliseconds to wait=u32 500) -> ()  [unwired: 1 out]
                  }
                  frame #4 {
                    n1000 = property on="Load parameters" class="Bool (strict)"("Val(Sgnl)"=TRUE ("Value (Signaling)")) -> ()  [unwired: 2 in, 2 out]
                  }
                  frame #5 {
                    n1001 = Wait (ms)(milliseconds to wait=u32 500) -> ()  [unwired: 1 out]
                  }
                  frame #6 {
                    n1002 = property on="Trap Raster Scan" class="Bool (strict)"("Val(Sgnl)"=TRUE ("Value (Signaling)")) -> ()  [unwired: 2 in, 2 out]
                  }
                  frame #7 {
                    n1003 = Wait (ms)(milliseconds to wait=u32 2000) -> ()  [unwired: 1 out]
                  }
                  frame #8 {
                    n1004 = while {
                      stop <- w1590 stop-if-true
                      n1005 = local read "Raster Scanning..."() -> (w1593:bool)
                      n1006 = local read "Saving..."() -> (w1591:bool)
                      n1007 = Wait (ms)(milliseconds to wait=u32 100) -> ()  [unwired: 1 out]
                      n1008 = Not(x=w1591) -> (.not. x?=w1589:bool)
                      n1009 = Not(x=w1593) -> (.not. x?=w1592:bool)
                      n1010 = And(x=w1592, y=w1589) -> (x .and. y?=w1590:bool)
                    }
                  }
                  frame #9 {
                    n1011 = property on="Trap Delta (MHz)" class="DigNum (strict)"("Val(Sgnl)"=w1597) -> ()  [unwired: 2 in, 2 out]
                    n1012 = property on="Saved AOD Raster Scan Parameter Sets" class="Arr (strict)"("Index Values"=u32[] [0]) -> ()  [unwired: 2 in, 2 out]
                    n1013 = property on="Save ave N" class="DigNum (strict)"("Val(Sgnl)"=w1595) -> ()  [unwired: 2 in, 2 out]
                  }
                  frame #10 {
                    n1014 = Wait (ms)(milliseconds to wait=u32 500) -> ()  [unwired: 1 out]
                  }
                  frame #11 {
                    n1015 = property on="Load parameters" class="Bool (strict)"("Val(Sgnl)"=TRUE ("Value (Signaling)")) -> ()  [unwired: 2 in, 2 out]
                  }
                }
              }
            }
          }
          frame #7 {
            n1016 = property on="Read Cal" class="Bool (strict)"("Val(Sgnl)"=TRUE ("Value (Signaling)")) -> ()  [unwired: 2 in, 2 out]
          }
          frame #8 {
            n1017 = Wait (ms)(milliseconds to wait=u32 500) -> ()  [unwired: 1 out]
          }
          frame #9 {
            n1018 = property on="Fish for Tether" class="Bool (strict)"("Val(Sgnl)"=TRUE ("Value (Signaling)")) -> ()  [unwired: 2 in, 2 out]
          }
        }
      }
      event "Dump Beads": Value Change {
        # "SCRIPT TO REMOVE BOTH BEADS FROM THE TRAPS. TURNS ON LIGHT WHICH INDICATES THAT STAGE IS MOVING. THEN STOPS SAVING DATA. \nSETS Sample Channel Flow TO TRUE. STOPS INTERLACING GREEN FLUORESCENCE. TURNS OFF Tether INDICATOR BECAUSE WE ARE THROWING IT\nAWAY. SHUTS OFF TRAP POSITION FEEDBACK."
        n1019 = event-data() -> ()  [unwired: 1 in, 5 out]
        n1020 = flat-sequence {
          frame #0 {
            w1604 = FALSE ("Fl. Triggered...")
            w1605 = TRUE ("Stage Moving")
            n1021 = local read "Saving..."() -> (w1606:bool)
            n1022 = local write "Fl. Triggered..."(w1604) -> ()
            n1023 = local write "Stage Moving"(w1605) -> ()
            n1024 = local write "Tether"(w1604) -> ()
            n1025 = property on="Green Laser ON/Interlacing" class="Bool (strict)"("Val(Sgnl)"=w1604) -> ()  [unwired: 2 in, 2 out]
            n1026 = property on="Trap Pos. FB ON" class="Bool (strict)"("Val(Sgnl)"=w1604) -> ()  [unwired: 2 in, 2 out]
            n1027 = property on="Sample Channel Flow" class="Bool (strict)"("Val(Sgnl)"=w1605) -> ()  [unwired: 2 in, 2 out]
            n1028 = local write "Stop Saving"(w1606) -> ()
          }
          frame #1 {
            w1607 = FALSE ("Value (Signaling)")
            # "TURNS TRAPS OFF SO THAT\nBEADS REMAIN AT DUMP \nBEADS POSITION"
            n1029 = property on="Trap 1 (ON/OFF)" class="Bool (strict)"("Val(Sgnl)"=w1607) -> ()  [unwired: 2 in, 2 out]
            n1030 = property on="Trap 2 (ON/OFF)" class="Bool (strict)"("Val(Sgnl)"=w1607) -> ()  [unwired: 2 in, 2 out]
            n1031 = call <vilib>:"Beep.vi"() -> ()  [unwired: 3 in, 9 out]
          }
          frame #2 {
            n1032 = local read "Cal @ (MHz)"() -> (w1608:dbl)
            n1033 = property on="Trap Delta (MHz)" class="DigNum (strict)"("Val(Sgnl)"=w1608) -> ()  [unwired: 2 in, 2 out]
          }
        }
      }
      event "Dip for Protein": Value Change {
        n1034 = event-data() -> ()  [unwired: 1 in, 5 out]
        n1035 = flat-sequence {
          frame #0 {
            n1036 = case shown="True" "Move Trap Before?" {
              frame False {
              }
              frame True {
                n1037 = property on="Trap Delta (MHz)" class="DigNum (strict)"("Val(Sgnl)"="Dip Trap Delta 1 (MHz)") -> ()  [unwired: 2 in, 2 out]
              }
            }
          }
          frame #1 {
            n1038 = Multiply(x="Duration (s)", y=1000.0) -> (x*y=w1612:dbl)
            n1039 = Wait (ms)(milliseconds to wait=w1612) -> ()  [unwired: 1 out]
          }
          frame #2 {
            n1040 = case shown="True" "Move Trap After?" {
              frame False {
              }
              frame True {
                n1041 = property on="Trap Delta (MHz)" class="DigNum (strict)"("Val(Sgnl)"="Dip Trap Delta 2 (MHz)") -> ()  [unwired: 2 in, 2 out]
              }
            }
          }
          frame #3 {
            n1042 = case shown="True" "Green ON After?" {
              frame False {
              }
              frame True {
                n1043 = property on="Green Laser ON/Interlacing" class="Bool (strict)"("Val(Sgnl)"=TRUE ("Value (Signaling)")) -> ()  [unwired: 2 in, 2 out]
              }
            }
          }
          frame #4 {
            n1044 = Wait (ms)(milliseconds to wait=u32 500) -> ()  [unwired: 1 out]
          }
          frame #5 {
            n1045 = case shown="True" "Save Data After?" {
              frame False {
              }
              frame True {
                n1046 = property on="Start Saving" class="Bool (strict)"("Val(Sgnl)"=TRUE ("Value (Signaling)")) -> ()  [unwired: 2 in, 2 out]
              }
            }
          }
        }
      }
      event "Profile": Value Change {
        n1047 = event-data() -> ()  [unwired: 1 in, 5 out]
        n1048 = flat-sequence {
          frame #0 {
            w1622 = 0.0 ("element")
            n1049 = Build Array(w1622, "Y change (mm)", w1622) -> ()  [unwired: 1 out]
          }
          frame #1 {
            # "stop saving"
            n1050 = local write "Stop Saving"(TRUE ("Stop Saving")) -> ()
            n1051 = local write "Stage Moving"(FALSE ("Stage Moving")) -> ()
          }
        }
      }
      event "Got ADig bead": Value Change {
        n1052 = event-data() -> ()  [unwired: 1 in, 5 out]
        n1053 = property on="Move Cap. 1 (DNA Top)" class="Bool (strict)"("Val(Sgnl)"=TRUE ("Value (Signaling)")) -> ()  [unwired: 2 in, 2 out]
        n1054 = property on="Inject Bottom" class="Bool (strict)"("Val(Sgnl)"=FALSE ("Value (Signaling)")) -> ()  [unwired: 2 in, 2 out]
      }
      event "Got DNA bead": Value Change {
        n1055 = event-data() -> ()  [unwired: 1 in, 5 out]
        n1056 = property on="Cal/Data Acq. Spot" class="Bool (strict)"("Val(Sgnl)"=TRUE ("Value (Signaling)")) -> ()  [unwired: 2 in, 2 out]
        n1057 = property on="Inject Top" class="Bool (strict)"("Val(Sgnl)"=FALSE ("Value (Signaling)")) -> ()  [unwired: 2 in, 2 out]
      }
      event "Take Stepping Data": Value Change {
        n1058 = event-data() -> ()  [unwired: 1 in, 5 out]
        n1059 = local read "Save ave N"() -> (w1640:dbl)
        n1060 = flat-sequence {
          tunnel: w1640 -> [w1642]
          tunnel: [w1642] -> w1635
          tunnel: [w1644] -> w1636
          tunnel: w1635 -> [w1644]
          tunnel: [w1646] -> w1637
          tunnel: w1636 -> [w1646]
          tunnel: [w1649] -> w1638
          tunnel: w1637 -> [w1649]
          tunnel: [w1651] -> w1639
          tunnel: w1638 -> [w1651]
          tunnel: [w1653] -> w1633
          tunnel: w1639 -> [w1653]
          tunnel: w1633 -> [w1656]
          tunnel: [w1656] -> w1632
          tunnel: w1632 -> [w1657]
          tunnel: [w1657] -> w1634
          tunnel: w1634 -> [w1663]
          frame #0 {
            n1061 = property on="Save ave N" class="DigNum (strict)"("Val(Sgnl)"="Save ave factor") -> ()  [unwired: 2 in, 2 out]
          }
          frame #1 {
            n1062 = Wait (ms)(milliseconds to wait=u32 100) -> ()  [unwired: 1 out]
          }
          frame #2 {
            n1063 = local read "Offset 2 Start (MHz)"() -> (w1648:dbl)
            n1064 = property on="Saved AOD Raster Scan Parameter Sets" class="Arr (strict)"("Index Values"=u32[] [2]) -> ()  [unwired: 2 in, 2 out]
            n1065 = property on="Trap Delta (MHz)" class="DigNum (strict)"("Val(Sgnl)"=w1648) -> ()  [unwired: 2 in, 2 out]
          }
          frame #3 {
            n1066 = property on="Load parameters" class="Bool (strict)"("Val(Sgnl)"=TRUE ("Value (Signaling)")) -> ()  [unwired: 2 in, 2 out]
          }
          frame #4 {
            n1067 = Wait (ms)(milliseconds to wait=u32 100) -> ()  [unwired: 1 out]
          }
          frame #5 {
            n1068 = property on="Trap Raster Scan" class="Bool (strict)"("Val(Sgnl)"=TRUE ("Value (Signaling)")) -> ()  [unwired: 2 in, 2 out]
          }
          frame #6 {
            n1069 = Wait (ms)(milliseconds to wait=u32 1000) -> ()  [unwired: 1 out]
          }
          frame #7 {
            n1070 = while {
              stop <- w1660 stop-if-true
              n1071 = local read "Raster Scanning..."() -> (w1662:bool)
              n1072 = local read "Saving..."() -> (w1661:bool)
              n1073 = Not(x=w1661) -> (.not. x?=w1658:bool)
              n1074 = Not(x=w1662) -> (.not. x?=w1659:bool)
              n1075 = And(x=w1659, y=w1658) -> (x .and. y?=w1660:bool)
            }
          }
          frame #8 {
            n1076 = property on="Save ave N" class="DigNum (strict)"("Val(Sgnl)"=w1663) -> ()  [unwired: 2 in, 2 out]
          }
        }
      }
      event "Step Size (nm)": Value Change {
        n1077 = event-data() -> ()  [unwired: 1 in, 5 out]
        n1078 = flat-sequence {
          frame #0 {
            n1079 = property on="Saved AOD Raster Scan Parameter Sets" class="Arr (strict)"("Index Values"=u32[] [1]) -> ()  [unwired: 2 in, 2 out]
          }
          frame #1 {
            n1080 = Multiply(x="N Steps", y="Step Size (nm)") -> (x*y=w1665:dbl)
            n1081 = property on="Scan Speed AOD (nm/s) 2" class="DigNum (strict)"("Value"="Step Size (nm)") -> ()  [unwired: 2 in, 2 out]
            n1082 = property on="Step Size AOD (nm) 2" class="DigNum (strict)"("Value"="Step Size (nm)") -> ()  [unwired: 2 in, 2 out]
            n1083 = property on="Scan Range AOD (nm) 2" class="DigNum (strict)"("Value"=w1665) -> ()  [unwired: 2 in, 2 out]
          }
        }
      }
      event "Take Detection Laser\nImage": Value Change {
        n1084 = event-data() -> ()  [unwired: 1 in, 5 out]
        n1085 = flat-sequence {
          tunnel: [w1693] -> w1683
          tunnel: [w1692] -> w1676
          tunnel: [w1691] -> w1668
          tunnel: [w1696] -> w1684
          tunnel: w1683 -> [w1696]
          tunnel: [w1695] -> w1677
          tunnel: w1676 -> [w1695]
          tunnel: [w1694] -> w1669
          tunnel: w1668 -> [w1694]
          tunnel: [w1700] -> w1685
          tunnel: w1684 -> [w1700]
          tunnel: [w1699] -> w1678
          tunnel: w1677 -> [w1699]
          tunnel: [w1698] -> w1670
          tunnel: w1669 -> [w1698]
          tunnel: [w1706] -> w1686
          tunnel: w1685 -> [w1706]
          tunnel: [w1705] -> w1679
          tunnel: w1678 -> [w1705]
          tunnel: [w1704] -> w1671
          tunnel: w1670 -> [w1704]
          tunnel: [w1710] -> w1687
          tunnel: w1686 -> [w1710]
          tunnel: [w1709] -> w1680
          tunnel: w1679 -> [w1709]
          tunnel: [w1708] -> w1672
          tunnel: w1671 -> [w1708]
          tunnel: [w1714] -> w1688
          tunnel: w1687 -> [w1714]
          tunnel: [w1713] -> w1681
          tunnel: w1680 -> [w1713]
          tunnel: [w1712] -> w1673
          tunnel: w1672 -> [w1712]
          tunnel: [w1718] -> w1689
          tunnel: w1688 -> [w1718]
          tunnel: [w1717] -> w1682
          tunnel: w1681 -> [w1717]
          tunnel: [w1716] -> w1674
          tunnel: w1673 -> [w1716]
          tunnel: w1689 -> [w1724]
          tunnel: w1682 -> [w1723]
          tunnel: [w1721] -> w1675
          tunnel: w1674 -> [w1721]
          tunnel: w1675 -> [w1725]
          frame #0 {
            n1086 = local read "Green Laser ON/Interlacing"() -> (w1693:bool)
            n1087 = local read "Green laser mode"() -> (w1692:enum32{"Laser ON", "Laser OFF", "Interlace"})
            n1088 = local read "Green FB On/Off"() -> (w1691:bool)
          }
          frame #1 {
            n1089 = property on="Green FB On/Off" class="Bool (strict)"("Val(Sgnl)"=FALSE ("Value (Signaling)")) -> ()  [unwired: 2 in, 2 out]
          }
          frame #2 {
            n1090 = property on="Green Laser ON/Interlacing" class="Bool (strict)"("Val(Sgnl)"=TRUE ("Value (Signaling)")) -> ()  [unwired: 2 in, 2 out]
            n1091 = property on="Flip Green Filter" class="Bool (strict)"("Val(Sgnl)"=TRUE ("Value (Signaling)")) -> ()  [unwired: 2 in, 2 out]
            n1092 = property on="Green laser mode" class="RadioBtnsControl (strict)"("Val(Sgnl)"=enum32{"Laser ON", "Laser OFF", "Interlace"}."Laser ON" ("Value (Signaling)")) -> ()  [unwired: 2 in, 2 out]
          }
          frame #3 {
            n1093 = Wait (ms)(milliseconds to wait=u32 500) -> ()  [unwired: 1 out]
          }
          frame #4 {
            n1094 = property on="Confocal Image" class="Bool (strict)"("Val(Sgnl)"=TRUE ("Value (Signaling)")) -> ()  [unwired: 2 in, 2 out]
          }
          frame #5 {
            n1095 = Wait (ms)(milliseconds to wait=u32 2000) -> ()  [unwired: 1 out]
          }
          frame #6 {
            n1096 = while {
              stop <- w1719 stop-if-true
              n1097 = local read "Saving..."() -> (w1720:bool)
              n1098 = Not(x=w1720) -> (.not. x?=w1719:bool)
            }
          }
          frame #7 {
            n1099 = property on="Flip Green Filter" class="Bool (strict)"("Val(Sgnl)"=TRUE ("Value (Signaling)")) -> ()  [unwired: 2 in, 2 out]
            n1100 = property on="Green Laser ON/Interlacing" class="Bool (strict)"("Val(Sgnl)"=w1724) -> ()  [unwired: 2 in, 2 out]
            n1101 = property on="Green laser mode" class="RadioBtnsControl (strict)"("Val(Sgnl)"=w1723) -> ()  [unwired: 2 in, 2 out]
          }
          frame #8 {
            n1102 = property on="Green FB On/Off" class="Bool (strict)"("Val(Sgnl)"=w1725) -> ()  [unwired: 2 in, 2 out]
          }
        }
      }
      event "Stop All": Value Change {
        n1103 = event-data() -> ()  [unwired: 1 in, 5 out]
        n1104 = local read "Stop All"() -> (w1726:bool)
      }
    }
    n1105 = node-c288() -> ()  [unwired: 1 in, 1 out]
  }
  n1106 = node-c288() -> (w76:T23)  [unwired: 4 out]
  n1107 = timed-loop "Acquire Data" {
    tunnel: w24 -> [w1981]
    tunnel: w40 -> [w1980]
    tunnel: [w2011] -> w33
    tunnel: [w2005] -> w32
    timing: w164 -> [_]
    timing-out: [_] -> w163
    tunnel: w59 -> [w1809]
    stop <- "Stop All" stop-if-true
    (unwired) u32 0 ("Number of Elements")
    w1796 = "NI_ChannelName" ("name")
    n1108 = node-c288() -> ()  [unwired: 2 out]
    n1109 = First Call?() -> (First Call?: T/F=w1762:bool)
    n1110 = Or(x="Reset", y=w1762) -> (x .or. y?=w1763:bool)
    n1111 = case "Reset data stream" shown="True" w1763 {
      tunnel: w1981 -> [w2027 w2035]
      tunnel: w1980 -> [w2026 w2034]
      tunnel: [w2027 w2029] -> w1976
      tunnel: [w2026 w2028] -> w1975
      frame False {
      }
      frame True {
        w2032 = TRUE ("AI to FIFO")
        n1112 = local write "Overflow (data lost)"(FALSE ("Overflow (data lost)")) -> ()
        n1113 = call "reset FPGA DMA.vi"("error in"=w2034, "FPGA VI Reference In"=w2035) -> ("error out"=w2030:errorcluster, "FPGA VI Reference Out"=w2031:T19)
        n1114 = xnode "Read/Write Control"("FPGA VI Reference In"=w2031, "error in"=w2030, "AI to FIFO"=w2032, "APD to FIFO"=w2032) -> ("FPGA VI Reference Out"=w2029:T19, "error out"=w2028:errorcluster)
      }
    }
    n1115 = Or(x="Start AOD Scan", y="Trap Raster Scan") -> (x .or. y?=w1926:bool)
    n1116 = case "Start AOM raster scan" shown="True" w1926 {
      tunnel: w1976 -> [w2764 w2774]
      tunnel: w1975 -> [w2763 w2773]
      tunnel: [w2764 w2767] -> w1974
      tunnel: [w2763 w2766] -> w1973
      frame False {
      }
      frame True {
        n1117 = case shown="True" "Restart DMA? (AOD)" {
          tunnel: [w2812 w2814] -> w2768
          tunnel: [w2811 w2813] -> w2769
          tunnel: w2774 -> [w2812 w2816]
          tunnel: w2773 -> [w2811 w2815]
          frame False {
          }
          frame True {
            n1118 = local write "Overflow (data lost)"(FALSE ("Overflow (data lost)")) -> ()
            n1119 = call "reset FPGA DMA.vi"("error in"=w2815, "FPGA VI Reference In"=w2816) -> ("error out"=w2813:errorcluster, "FPGA VI Reference Out"=w2814:T19)
          }
        }
        n1120 = local write "Trap Raster Scan"(FALSE ("Trap Raster Scan")) -> ()
        n1121 = case shown="False" "Move MCL Also?" {
          tunnel: w2769 -> [w2777 w2806]
          tunnel: w2768 -> [w2778 w2807]
          tunnel: [w2776 w2810] -> w2767
          tunnel: [w2775 w2809] -> w2766
          frame False {
            w2779 = TRUE ("AI to FIFO")
            n1122 = xnode "Read/Write Control"("FPGA VI Reference In"=w2778, "error in"=w2777, "AI to FIFO"=w2779, "APD to FIFO"=w2779, "Start scan"=w2779) -> ("FPGA VI Reference Out"=w2776:T19, "error out"=w2775:errorcluster)
          }
          frame True {
            w2803 = FALSE ("1D or 2D Scan?")
            w2808 = TRUE ("AI to FIFO")
            # "Count for MCL loop"
            # "N total cycles"
            # "N steps"
            # "V_int"
            n1123 = local read "Scan Range (nm)"() -> (w2785:dbl)
            n1124 = local read "Number of F/B Scans (AOD)"() -> (w2802:u16)
            n1125 = Sign(1:w2785) -> (0:w2784:dbl)
            n1126 = Compound Arithmetic op=MULTIPLY(w2785, "MCL Step Position Ratio", "MCL/AOM Scale Tweak") -> (w2789:dbl)
            n1127 = Negate(x=w2784) -> (-x=w2781:dbl)
            n1128 = Multiply(x=w2781, y="MCL Step Increment (V_int)") -> (x*y=w2783:dbl)
            n1129 = Divide(x=w2789, y="MCL X Cal (nm/V)") -> (x/y=w2795:dbl)
            n1130 = Multiply(x=32767.0 ("y"), y=w2795) -> (x*y=w2801:dbl)
            n1131 = local read "Total Counts (ticks)"() -> (w2786:u32)
            n1132 = local read "Cycles/step (AOD)"() -> (w2797:u64)
            n1133 = local read "Scan steps (AOD)"() -> (w2798:u64)
            n1134 = Divide(x=w2801, y=10.0) -> (x/y=w2794:dbl)
            n1135 = Divide(x=w2794, y="MCL Step Increment (V_int)") -> (x/y=w2792:dbl)
            n1136 = Absolute Value(x=w2792) -> (abs(x)=w2780:dbl)
            n1137 = Compound Arithmetic op=MULTIPLY(w2798, w2797, w2786) -> (w2793:u64)
            n1138 = local write "wait to reset values"(w2808) -> ()
            n1139 = local write "MCL Scanning"(w2808) -> ()
            n1140 = Divide(x=w2793, y=w2780) -> (x/y=w2790:dbl)
            "MCL Count" <- w2790
            n1141 = xnode "Read/Write Control"("FPGA VI Reference In"=w2807, "error in"=w2806, "Scan steps (MCL)"=w2780, "Number of scans (MCL)"=w2802, "Cycles per step (MCL)"=u64 1, "Scan freq.  increment (MCL)"=w2783, "1D or 2D Scan?"=w2803, "MCL Scan Axis"=w2803, "Cont. Scan (MCL)"=w2803, "MCL count"=w2790) -> ("FPGA VI Reference Out"=w2805:T19, "error out"=w2804:errorcluster)
            n1142 = xnode "Read/Write Control"("FPGA VI Reference In"=w2805, "error in"=w2804, "AI to FIFO"=w2808, "APD to FIFO"=w2808, "Start scan"=w2808, "Start scan (MCL)"=w2808) -> ("FPGA VI Reference Out"=w2810:T19, "error out"=w2809:errorcluster)
          }
        }
        "Raster Scanning..." <- TRUE ("Scanning...")
      }
    }
    n1143 = And(x="Save scans", y=w1926) -> (x .and. y?=w1972:bool)
    n1144 = Compound Arithmetic op=OR("Start MCL Scan", "Confocal Image", "Confocal Linescan") -> (w1924:bool)
    n1145 = And(x="Save Data (MCL)", y=w1924) -> (x .and. y?=w1971:bool)
    n1146 = case "Start MCL raster scan" shown="True" w1924 {
      tunnel: w1974 -> [w2318 w2333]
      tunnel: w1973 -> [w2317 w2332]
      tunnel: [w2318 w2328] -> w1731
      tunnel: [w2317 w2327] -> w1730
      tunnel: [FALSE w2326] -> w1957
      tunnel: "Start MCL Scan" -> [_ w2321]
      tunnel: "Confocal Image" -> [_ w2320]
      tunnel: "Confocal Linescan" -> [_ _]
      frame False {
      }
      frame True {
        w2326 = TRUE
        n1147 = case shown="True" "Restart DMA? (MCL)" {
          tunnel: [w2378 w2380] -> w2331
          tunnel: [w2377 w2379] -> w2330
          tunnel: w2333 -> [w2378 w2383]
          tunnel: w2332 -> [w2377 w2382]
          frame False {
          }
          frame True {
            n1148 = call "reset FPGA DMA.vi"("error in"=w2382, "FPGA VI Reference In"=w2383) -> ("error out"=w2379:errorcluster, "FPGA VI Reference Out"=w2380:T19)
            n1149 = local write "Overflow (data lost)"(FALSE ("Overflow (data lost)")) -> ()
          }
        }
        n1150 = case shown="False" w2321 {
          selector: w2321 -> [_ w2337]
          tunnel: w2320 -> [w2336 _]
          tunnel: [w2336 w2337] -> w2319
          frame False {
            n1151 = property on="2D or 1D Scan" class="Bool (strict)"("Val(Sgnl)"=w2336) -> ()  [unwired: 2 in, 2 out]
            n1152 = property on="Confocal Image" class="Bool (strict)"("Value"=FALSE ("Start Confocal Map")) -> ()  [unwired: 2 in, 2 out]
          }
          frame True {
          }
        }
        n1153 = local write "MCL Scanning"(w2326) -> ()
        n1154 = local read "AO1"() -> (w2323:dbl)
        n1155 = local read "AO2"() -> (w2322:dbl)
        n1156 = case shown="True" "Center Scan" {
          tunnel: w2331 -> [w2344 w2376]
          tunnel: w2330 -> [w2343 w2375]
          tunnel: [w2342 w2374] -> w2328
          tunnel: [w2341 w2373] -> w2327
          tunnel: [w2339 w2360] -> w2325
          tunnel: [w2338 w2359] -> w2324
          tunnel: w2323 -> [w2339 w2365]
          tunnel: w2322 -> [w2338 w2368]
          tunnel: w2319 -> [_ _]
          frame False {
            w2340 = TRUE ("AI to FIFO")
            n1157 = xnode "Read/Write Control"("FPGA VI Reference In"=w2344, "error in"=w2343, "AI to FIFO"=w2340, "APD to FIFO"=w2340, "Start scan (MCL)"=w2340) -> ("FPGA VI Reference Out"=w2342:T19, "error out"=w2341:errorcluster)
          }
          frame True {
            w2372 = TRUE ("AI to FIFO")
            n1158 = local read "Scan steps (MCL)"() -> (w2351:u64)
            n1159 = local read "Scan lines (y)"() -> (w2347:u64)
            n1160 = local read "Fast Scan Dir"() -> (w2358:bool)
            n1161 = local read "Actual MCL Inc (V)"() -> (w2348:dbl)
            n1162 = Decrement(x=w2347) -> (x-1=w2346:u64)
            n1163 = Decrement(x=w2351) -> (x-1=w2350:u64)
            n1164 = Multiply(x=w2348, y=w2346) -> (x*y=w2345:dbl)
            n1165 = Divide(x=w2345, y=2.0) -> (x/y=w2355:dbl)
            n1166 = Multiply(x=w2348, y=w2350) -> (x*y=w2349:dbl)
            n1167 = Divide(x=w2349, y=2.0) -> (x/y=w2354:dbl)
            n1168 = Select(t=w2354, s=w2358, f=w2355) -> (s? t:f=w2353:dbl)
            n1169 = Select(t=w2355, s=w2358, f=w2354) -> (s? t:f=w2357:dbl)
            n1170 = Subtract(x=w2365, y=w2357) -> (x-y=w2356:dbl)
            n1171 = Subtract(x=w2368, y=w2353) -> (x-y=w2352:dbl)
            n1172 = local read "2D or 1D Scan"() -> (w2370:bool)
            n1173 = Not(x=w2358) -> (.not. x?=w2364:bool)
            n1174 = Not(x=w2370) -> (.not. x?=w2366:bool)
            n1175 = And(x=w2358, y=w2366) -> (x .and. y?=w2367:bool)
            n1176 = And(x=w2366, y=w2364) -> (x .and. y?=w2369:bool)
            n1177 = Select(t=w2368, s=w2369, f=w2352) -> (s? t:f=w2359:dbl)
            n1178 = Select(t=w2365, s=w2367, f=w2356) -> (s? t:f=w2360:dbl)
            n1179 = call "Volt to I16.vi"("Voltage In"=w2360) -> ("I16 Voltage Out"=w2363:i16)
            n1180 = call "Volt to I16.vi"("Voltage In"=w2359) -> ("I16 Voltage Out"=w2362:i16)
            n1181 = xnode "Read/Write Control"("FPGA VI Reference In"=w2376, "error in"=w2375, "AI to FIFO"=w2372, "APD to FIFO"=w2372, "Start scan (MCL)"=w2372, "AO1"=w2363, "AO2"=w2362) -> ("FPGA VI Reference Out"=w2374:T19, "error out"=w2373:errorcluster)
          }
        }
        "Initial Y" <- w2325
        "Initial X" <- w2324
        "wait to reset values" <- w2326
      }
    }
    n1182 = local read "Trap Pos Elements/DMA read"() -> (w1805:u32)
    n1183 = local read "Trap AI Elements/DMA read"() -> (w1729:u32)
    n1184 = local read "APD Elements/DMA read"() -> (w1848:u32)
    n1185 = local read "Trap AI FIFO Depth"() -> (w2021:u32)
    n1186 = xnode "Invoke Method"("FPGA VI Reference In"=w1731, "error in"=w1730, "Number of Elements"=w1805, "Timeout (ms)"=-1) -> ("Data"=w1769:u16[], "Elements Remaining"=→"Trap Pos FIFO El Remaining":u32)  [unwired: 2 out]
    n1187 = xnode "Invoke Method"("FPGA VI Reference In"=w1731, "error in"=w1730, "Number of Elements"=w1729, "Timeout (ms)"=-1 ("Timeout")) -> ("FPGA VI Reference Out"=w1733:T19, "error out"=w1732:errorcluster, "Data"=w1728:i16[], "Elements Remaining"=w1734:u32)
    "Trap AI FIFO El. Rem." <- w1734
    n1188 = xnode "Get APD Data"("FPGA VI Reference In"=w1731, "error in"=w1730, "Number of Elements"=w1848, "Timeout (ms)"=-1) -> ("Data"=w1847:u32[], "Elements Remaining"=→"APD FIFO Elements Remaining":u32)  [unwired: 2 out]
    n1189 = Subtract(x=w2021, y=w1729) -> (x-y=w2020:u32)
    n1190 = Decimate 1D Array(w1769) -> (w1766:u16[], w1768:u16[], w1767:u16[])
    n1191 = Divide(x=w1734, y=w2020) -> (x/y=w2019:dbl)
    "Buffer Status" <- w2019
    n1192 = To Unsigned Long Integer(number=w1766) -> (unsigned 32bit integer=w1765:u32[])
    n1193 = Join Numbers(hi=w1768, lo=w1767) -> ((hi.lo)=w1764:u32[])
    n1194 = Equal?(x=w2019, y=1.0) -> (x = y?=w2017:bool)
    n1195 = Join Numbers(hi=w1765, lo=w1764) -> ((hi.lo)=w1758:u64[])
    n1196 = call "IR AOM word to freq - vec.vi"("Frequency Word In (double vec)"=w1758) -> ("Frequency Out"=w1804:dbl[])
    n1197 = case "Alert buffer overflow" shown="True" w2017 {
      frame False {
      }
      frame True {
        n1198 = call <vilib>:"Beep.vi"() -> ()  [unwired: 3 in, 9 out]
        "Overflow (data lost)" <- TRUE ("Overflow (data lost)")
      }
    }
    n1199 = Decimate 1D Array(w1804) -> (w1803:dbl[], w1802:dbl[])
    n1200 = Array Size(array=w1728) -> (size(s)=→"Waveform Chart":i32)
    n1201 = Build Array(w1803, w1802) -> (w1801:dbl[][])
    n1202 = local read "Trap Sets"() -> (w1885:u32)
    n1203 = case "Deinterlace trap data, average down PSD" shown="2" w1885 {
      tunnel: w1728 -> [w2413 w2478]
      tunnel: [w2410 w2475] -> w1878
      tunnel: [w2413 w2477] -> w1761
      tunnel: "Detector Type" -> [w2412 w2473]
      tunnel: [w2411 w2476] -> w1877
      tunnel: [w2409 w2474] -> w1992
      frame 1, Default {
        n1204 = Divide(x=w2413, y=3276.7) -> (x/y=w2414:dbl[])
        n1205 = Decimate 1D Array(w2414) -> (w2423:dbl[], w2422:dbl[], w2421:dbl[], w2420:dbl[], w2419:dbl[], w2418:dbl[], w2417:dbl[], w2416:dbl[])
        n1206 = case shown="\"IR-QPD + PSD + FB-QPD position\"" w2412 {
          tunnel: w2423 -> [w2447 w2472]
          tunnel: w2422 -> [w2446 w2471]
          tunnel: w2421 -> [w2431 w2449]
          tunnel: w2420 -> [w2432 w2459]
          tunnel: w2419 -> [w2445 w2470]
          tunnel: w2418 -> [w2444 w2469]
          tunnel: w2417 -> [w2428 w2450]
          tunnel: w2416 -> [w2427 w2448]
          tunnel: [w2426 w2456] -> w2411
          tunnel: [w2425 w2455] -> w2410
          tunnel: [w2424 w2454] -> w2409
          frame "IR-QPD + PSD + FB-QPD", Default {
            w2424 = 0  # Channel pattern
            n1207 = Divide(x=w2447, y=w2432) -> (x/y=w2434:dbl[])
            n1208 = Divide(x=w2446, y=w2432) -> (x/y=w2433:dbl[])
            n1209 = Divide(x=w2445, y=w2428) -> (x/y=w2430:dbl[])
            n1210 = Divide(x=w2444, y=w2427) -> (x/y=w2429:dbl[])
            n1211 = Build Array(w2434, w2433, w2432, w2431, w2430, w2429, w2428, w2427) -> (w2425:dbl[][])
            n1212 = Bundle("T1 Y", "T1 X", "T1 Sum", "FB Sum", "PSD Y", "PSD X", "PSD Y Sum", "PSD X Sum") -> (w2443:T39)  [unwired: 1 out]
            n1213 = Cluster To Array(cluster=w2443) -> (array=w2426:string[])
          }
          frame "IR-QPD + PSD + FB-QPD position" {
            w2454 = 3  # Channel pattern
            n1214 = Negate(x=w2450) -> (-x=w2451:dbl[])
            n1215 = Divide(x=w2472, y=w2459) -> (x/y=w2461:dbl[])
            n1216 = Divide(x=w2471, y=w2459) -> (x/y=w2460:dbl[])
            n1217 = Divide(x=w2470, y=w2450) -> (x/y=w2458:dbl[])
            n1218 = Divide(x=w2469, y=w2451) -> (x/y=w2457:dbl[])
            n1219 = Build Array(w2461, w2460, w2459, w2448, w2449, w2458, w2457, w2450) -> (w2455:dbl[][])
            n1220 = Bundle("T1 Y", "T1 X", "T1 Sum", "FB X", "FB Sum", "PSD Y", "PSD X", "PSD Y Sum") -> (w2468:T39)  [unwired: 1 out]
            n1221 = Cluster To Array(cluster=w2468) -> (array=w2456:string[])
          }
        }
      }
      frame 2 {
        n1222 = case shown="\"UCB Fleezers 052511\"" w2473 {
          tunnel: w2478 -> [w2540 w2607 w2635 w2742]
          tunnel: [w2479 w2599 w2630 w2673] -> w2477
          tunnel: [w2506 w2590 w2632 w2720] -> w2476
          tunnel: [w2505 w2554 w2609 w2687] -> w2475
          tunnel: [w2499 w2589 w2672 w2718] -> w2474
          frame "IR-QPD + PSD + FB-QPD", Default {
            w2499 = 1  # Channel pattern
            # "time average x2 the 4th signal and the 4 psd signals (detection laser)"
            # "deinterlace 3 signals from qpd"
            n1223 = Decimate 1D Array(w2540) -> (w2539:i16[], w2538:i16[], w2504:i16[], w2537:i16[], w2527:i16[], w2525:i16[], w2524:i16[], w2522:i16[])
            n1224 = call "downsample 1D array - double.vi"("Ave N"=2.0, "Array In"=w2527) -> ("Array Out"=w2526:dbl[])  [unwired: 1 out]
            n1225 = call "downsample 1D array - double.vi"("Ave N"=2.0, "Array In"=w2522) -> ("Array Out"=w2521:dbl[])  [unwired: 1 out]
            n1226 = call "downsample 1D array - double.vi"("Ave N"=2.0, "Array In"=w2524) -> ("Array Out"=w2523:dbl[])  [unwired: 1 out]
            n1227 = call "downsample 1D array - double.vi"("Ave N"=2.0, "Array In"=w2525) -> ("Array Out"=w2507:dbl[])  [unwired: 1 out]
            n1228 = Decimate 1D Array(w2539) -> (w2536:i16[], w2508:i16[])
            n1229 = Decimate 1D Array(w2538) -> (w2535:i16[], w2533:i16[])
            n1230 = Decimate 1D Array(w2537) -> (w2534:i16[], w2532:i16[])
            n1231 = Decimate 1D Array(w2504) -> (w2503:i16[], w2502:i16[])
            n1232 = Interleave 1D Arrays(w2536, w2535, w2534, w2508, w2533, w2532, w2503, w2502, w2526, w2507, w2523, w2521) -> (w2520:dbl[])
            n1233 = To Word Integer(number=w2520) -> (16bit integer=w2479:i16[])
            n1234 = Divide(x=w2520, y=3276.7) -> (x/y=w2519:dbl[])
            n1235 = Decimate 1D Array(w2519) -> (w2518:dbl[], w2517:dbl[], w2516:dbl[], w2515:dbl[], w2514:dbl[], w2513:dbl[], w2501:dbl[], w2500:dbl[], w2512:dbl[], w2511:dbl[], w2510:dbl[], w2509:dbl[])
            n1236 = Divide(x=w2518, y=w2516) -> (x/y=w2486:dbl[])
            n1237 = Divide(x=w2517, y=w2516) -> (x/y=w2485:dbl[])
            n1238 = Divide(x=w2515, y=w2513) -> (x/y=w2484:dbl[])
            n1239 = Divide(x=w2514, y=w2513) -> (x/y=w2483:dbl[])
            n1240 = Divide(x=w2512, y=w2510) -> (x/y=w2482:dbl[])
            n1241 = Divide(x=w2511, y=w2509) -> (x/y=w2481:dbl[])
            n1242 = Bundle("T1 Y", "T1 X", "T1 Sum", "T2 Y", "T2 X", "T2 Sum", "T1 FB Sum", "T2 FB Sum", "PSD Y", "PSD X", "PSD Y Sum", "PSD X Sum") -> (w2487:T40)  [unwired: 1 out]
            n1243 = Build Array(w2486, w2485, w2516, w2484, w2483, w2513, w2501, w2500, w2482, w2481, w2510, w2509) -> (w2505:dbl[][])
            n1244 = Cluster To Array(cluster=w2487) -> (array=w2506:string[])
          }
          frame "IR-QPD + PSD + FB-QPD X position" {
            w2589 = 2  # Channel pattern
            # "convert\nADC numbers\nto volts"
            # "time average x2 the 3 psd signals (detection laser)"
            # "deinterlace 3 signals from qpds"
            n1245 = Decimate 1D Array(w2607) -> (w2606:i16[], w2605:i16[], w2542:i16[], w2543:i16[], w2552:i16[], w2549:i16[], w2546:i16[], w2577:i16[])
            n1246 = Decimate 1D Array(w2606) -> (w2604:i16[], w2591:i16[])
            n1247 = call "downsample 1D array - I16.vi"("Ave N"=2.0, "Array In"=w2552) -> ("Array Out"=w2550:i16[])  [unwired: 1 in]
            n1248 = call "downsample 1D array - I16.vi"("Ave N"=2.0, "Array In"=w2549) -> ("Array Out"=w2547:i16[])  [unwired: 1 in]
            n1249 = Decimate 1D Array(w2605) -> (w2603:i16[], w2601:i16[])
            n1250 = Decimate 1D Array(w2543) -> (w2602:i16[], w2600:i16[])
            n1251 = Decimate 1D Array(w2577) -> (w2576:i16[], w2574:i16[])
            n1252 = Decimate 1D Array(w2542) -> (w2575:i16[], w2573:i16[])
            n1253 = call "downsample 1D array - I16.vi"("Ave N"=2.0, "Array In"=w2546) -> ("Array Out"=w2544:i16[])  [unwired: 1 in]
            n1254 = Interleave 1D Arrays(w2604, w2603, w2602, w2591, w2601, w2600, w2576, w2575, w2574, w2573, w2550, w2547, w2544) -> (w2599:i16[])
            n1255 = Divide(x=w2599, y=3276.7) -> (x/y=w2598:dbl[])
            n1256 = Decimate 1D Array(w2598) -> (w2597:dbl[], w2596:dbl[], w2595:dbl[], w2594:dbl[], w2593:dbl[], w2592:dbl[], w2565:dbl[], w2563:dbl[], w2562:dbl[], w2560:dbl[], w2559:dbl[], w2558:dbl[], w2555:dbl[])
            n1257 = Divide(x=w2597, y=w2595) -> (x/y=w2581:dbl[])
            n1258 = Divide(x=w2596, y=w2595) -> (x/y=w2580:dbl[])
            n1259 = Divide(x=w2594, y=w2592) -> (x/y=w2579:dbl[])
            n1260 = Divide(x=w2593, y=w2592) -> (x/y=w2578:dbl[])
            n1261 = Divide(x=w2565, y=w2563) -> (x/y=w2564:dbl[])
            n1262 = Divide(x=w2562, y=w2560) -> (x/y=w2561:dbl[])
            n1263 = Divide(x=w2559, y=w2555) -> (x/y=w2557:dbl[])
            n1264 = Negate(x=w2555) -> (-x=w2553:dbl[])
            n1265 = Divide(x=w2558, y=w2553) -> (x/y=w2556:dbl[])
            n1266 = Bundle("T1 Y", "T1 X", "T1 Sum", "T2 Y", "T2 X", "T2 Sum", "T1 FB X", "T1 FB Sum", "T2 FB X", "T2 FB Sum", "PSD Y", "PSD X", "PSD Y Sum") -> (w2582:T41)  [unwired: 1 out]
            n1267 = Build Array(w2581, w2580, w2595, w2579, w2578, w2592, w2564, w2563, w2561, w2560, w2557, w2556, w2555) -> (w2554:dbl[][])
            n1268 = Cluster To Array(cluster=w2582) -> (array=w2590:string[])
          }
          frame "UCB Fleezers 052511" {
            w2672 = 2  # Channel pattern
            n1269 = Decimate 1D Array(w2635) -> (w2670:i16[], w2669:i16[], w2634:i16[], w2633:i16[], w2627:i16[], w2624:i16[], w2623:i16[], w2622:i16[])
            n1270 = Decimate 1D Array(w2670) -> (w2668:i16[], w2653:i16[])
            n1271 = Decimate 1D Array(w2669) -> (w2667:i16[], w2665:i16[])
            n1272 = Decimate 1D Array(w2634) -> (w2666:i16[], w2664:i16[])
            n1273 = Decimate 1D Array(w2633) -> (w2629:i16[], w2628:i16[])
            n1274 = Decimate 1D Array(w2627) -> (w2626:i16[], w2625:i16[])
            n1275 = call "downsample 1D array - I16.vi"("Ave N"=2.0, "Array In"=w2624) -> ("Array Out"=w2621:i16[])  [unwired: 1 in]
            n1276 = call "downsample 1D array - I16.vi"("Ave N"=2.0, "Array In"=w2623) -> ("Array Out"=w2620:i16[])  [unwired: 1 in]
            n1277 = call "downsample 1D array - I16.vi"("Ave N"=2.0, "Array In"=w2622) -> ("Array Out"=w2619:i16[])  [unwired: 1 in]
            n1278 = Interleave 1D Arrays(w2668, w2667, w2666, w2653, w2665, w2664, w2629, w2626, w2628, w2625, w2621, w2620, w2619) -> (w2630:i16[])
            n1279 = Divide(x=w2630, y=3276.7) -> (x/y=w2660:dbl[])
            n1280 = Decimate 1D Array(w2660) -> (w2659:dbl[], w2658:dbl[], w2657:dbl[], w2656:dbl[], w2655:dbl[], w2654:dbl[], w2618:dbl[], w2616:dbl[], w2615:dbl[], w2613:dbl[], w2612:dbl[], w2611:dbl[], w2610:dbl[])
            n1281 = Divide(x=w2659, y=w2657) -> (x/y=w2640:dbl[])
            n1282 = Divide(x=w2658, y=w2657) -> (x/y=w2639:dbl[])
            n1283 = Divide(x=w2656, y=w2654) -> (x/y=w2638:dbl[])
            n1284 = Divide(x=w2655, y=w2654) -> (x/y=w2637:dbl[])
            n1285 = Divide(x=w2618, y=w2616) -> (x/y=w2617:dbl[])
            n1286 = Divide(x=w2615, y=w2613) -> (x/y=w2614:dbl[])
            n1287 = Bundle("T1 Y", "T1 X", "T1 Sum", "T2 Y", "T2 X", "T2 Sum", "T1 FB X", "T2 FB Sum", "T2 FB X", "T2 FB Sum", "PSD Y", "PSD X", "PSD Sum") -> (w2641:T41)  [unwired: 1 out]
            n1288 = Build Array(w2640, w2639, w2657, w2638, w2637, w2654, w2617, w2616, w2614, w2613, w2612, w2611, w2610) -> (w2609:dbl[][])
            n1289 = Cluster To Array(cluster=w2641) -> (array=w2632:string[])
          }
          frame "IR-QPD + PSD + FB-QPD XY positions" {
            w2718 = 4  # Channel pattern
            # "time average x2 the 3 psd signals (detection laser)"
            # "deinterlace 3 signals from qpds"
            n1290 = Decimate 1D Array(w2742) -> (w2741:i16[], w2740:i16[], w2719:i16[], w2739:i16[], w2685:i16[], w2731:i16[], w2730:i16[], w2707:i16[])
            n1291 = Decimate 1D Array "QPD Y"(w2741) -> (w2738:i16[], w2721:i16[])
            n1292 = call "downsample 1D array - double.vi"("Ave N"=2.0, "Array In"=w2731) -> ("Array Out"=w2706:dbl[])  [unwired: 1 out]
            n1293 = call "downsample 1D array - double.vi"("Ave N"=2.0, "Array In"=w2730) -> ("Array Out"=w2705:dbl[])  [unwired: 1 out]
            n1294 = Decimate 1D Array "Feedback Sum"(w2719) -> (w2703:i16[], w2701:i16[])
            n1295 = Decimate 1D Array "Feedback Y"(w2685) -> (w2684:i16[], w2683:i16[])
            n1296 = Decimate 1D Array "Feedback X"(w2707) -> (w2704:i16[], w2702:i16[])
            n1297 = Decimate 1D Array "QPD Sum"(w2739) -> (w2736:i16[], w2734:i16[])
            n1298 = Decimate 1D Array "QPD X"(w2740) -> (w2737:i16[], w2735:i16[])
            n1299 = Interleave 1D Arrays(w2738, w2737, w2736, w2721, w2735, w2734, w2684, w2704, w2703, w2683, w2702, w2701, w2706, w2705) -> (w2729:dbl[])
            n1300 = To Word Integer(number=w2729) -> (16bit integer=w2673:i16[])
            n1301 = Divide(x=w2729, y=3276.7) -> (x/y=w2728:dbl[])
            n1302 = Decimate 1D Array(w2728) -> (w2727:dbl[], w2726:dbl[], w2725:dbl[], w2724:dbl[], w2723:dbl[], w2722:dbl[], w2680:dbl[], w2694:dbl[], w2678:dbl[], w2679:dbl[], w2692:dbl[], w2676:dbl[], w2690:dbl[], w2688:dbl[])
            n1303 = Divide(x=w2727, y=w2725) -> (x/y=w2711:dbl[])
            n1304 = Divide(x=w2726, y=w2725) -> (x/y=w2710:dbl[])
            n1305 = Divide(x=w2724, y=w2722) -> (x/y=w2709:dbl[])
            n1306 = Divide(x=w2723, y=w2722) -> (x/y=w2708:dbl[])
            n1307 = Divide(x=w2680, y=w2678) -> (x/y=w2677:dbl[])
            n1308 = Divide(x=w2694, y=w2678) -> (x/y=w2693:dbl[])
            n1309 = Divide(x=w2679, y=w2676) -> (x/y=w2675:dbl[])
            n1310 = Divide(x=w2692, y=w2676) -> (x/y=w2691:dbl[])
            n1311 = Negate(x=w2688) -> (-x=w2686:dbl[])
            n1312 = Divide(x=w2690, y=w2686) -> (x/y=w2689:dbl[])
            n1313 = Bundle("T1 Y", "T1 X", "T1 Sum", "T2 Y", "T2 X", "T2 Sum", "T1 FB Y", "T1 FB X", "T1 FB Sum", "T2 FB Y", "T2 FB X", "T2 FB Sum", "PSD X", "PSD Y Sum") -> (w2674:T42)  [unwired: 1 out]
            n1314 = Build Array(w2711, w2710, w2725, w2709, w2708, w2722, w2677, w2693, w2678, w2675, w2691, w2676, w2689, w2688) -> (w2687:dbl[][])
            n1315 = Cluster To Array(cluster=w2674) -> (array=w2720:string[])
          }
        }
      }
    }
    "AI labels" <- w1877
    n1316 = Decimate 1D Array(w1847) -> (w1875:u32[], w1811:u32[])
    n1317 = local read "DMA Update Period (s)"() -> (w1886:dbl)
    n1318 = local read "BD 1 Frequency 2 (MHz)"() -> (w1753:dbl)
    n1319 = local read "BD 1 Frequency 1 (MHz)"() -> (w1754:dbl)
    n1320 = Build Array(w1875, w1811) -> (w1954:u32[][])
    n1321 = local read "Data Period (s)"() -> (w1860:dbl)
    n1322 = Decimate 1D Array(w1761) -> (w1784:i16[], w1783:i16[], w1781:i16[], w1780:i16[])  [unwired: 9 out]
    n1323 = To Double Precision Float(number=w1954) -> (double precision float=w1955:dbl[][])
    n1324 = local read "APD Integration Time (s)"() -> (w1824:dbl)
    n1325 = Divide(x=w1784, y=w1783) -> (x/y=w1785:dbl[])
    n1326 = Divide(x=w1781, y=w1780) -> (x/y=w1782:dbl[])
    n1327 = feedback #1(0.0) -> (w1798:dbl)
    n1328 = Add(x=w1886, y=w1798) -> (x+y=w1994:dbl)
    n1329 = feedback-in #1(w1994) -> ()
    n1330 = local read "AOM X Cal (nm/MHz)"() -> (w1751:dbl)
    n1331 = To Time Stamp(1:w1798) -> (0:w1797:timestamp)
    n1332 = Split 1D Array(array=w1785, index="N El. to Ave.") -> (second subarray=w1788:dbl[])  [unwired: 1 out]
    n1333 = Split 1D Array(array=w1782, index="N El. to Ave.") -> (second subarray=w1787:dbl[])  [unwired: 1 out]
    n1334 = local read "Trap X AI1 (DMA)"() -> (w1786:T13)
    n1335 = Multiply(x=w1860, y="Trap Disp. Downsample") -> (x*y=w1799:dbl)
    "Display Period (s)" <- w1799
    n1336 = Bundle("BD 1 Frequency 1 (MHz)"=w1754, "BD 1 Frequency 2 (MHz)"=w1753) -> (w1755:T43)  [unwired: 1 out]
    n1337 = for "Trap AI" {
      tunnel: [w2408] -> w1988 mode=indexing
      tunnel: w1797 -> [w2398]
      tunnel: "Trap Disp. Downsample" -> [w2406]
      tunnel: w1878 -> [w2404] mode=indexing
      tunnel: w1860 -> [w2403]
      tunnel: w1877 -> [w2402] mode=indexing
      tunnel: w1796 -> [w2401]
      tunnel: [w2400] -> w1835 mode=indexing
      tunnel: w1799 -> [w2399]
      n1338 = Bundle By Name("Y"=w2404, "dt"=w2403) -> (w2405:waveform(dbl))  [unwired: 1 out]
      n1339 = Set Waveform Attribute(5:w2402, 6:w2401, 7:w2405) -> (3:w2400:waveform(dbl))  [unwired: 1 in, 2 out]
      n1340 = call "downsample 1D array - double.vi"("Ave N"=w2406, "Array In"=w2404) -> ("Array Out"=w2407:dbl[])  [unwired: 1 out]
      n1341 = Bundle By Name(cluster=w2400, "t0"=w2398, "Y"=w2407, "dt"=w2399) -> (w2408:waveform(dbl))
    }
    n1342 = call-poly <vilib>:"Mean.vi"("X"=w1787) -> ("mean"=w1775:dbl)  [unwired: 1 out]
    n1343 = call-poly <vilib>:"Mean.vi"("X"=w1788) -> ("mean"=w1776:dbl)  [unwired: 1 out]
    n1344 = Cluster To Array(cluster=w1755) -> (array=w1752:dbl[])
    n1345 = Reciprocal(x=w1799) -> (1/x=→"Trap Disp. Freq. (Hz)":dbl)
    n1346 = local read "Data points/scans (MCL)"() -> (w1966:dbl)
    n1347 = To Fixed-Point(number=w1775) -> (fixed-point=w1773:fxp<+/-,16,1>)  [unwired: 1 in]
    n1348 = To Fixed-Point(number=w1776) -> (fixed-point=w1774:fxp<+/-,16,1>)  [unwired: 1 in]
    n1349 = Bundle("Trap 1 Pos.", "Trap 2 Pos.") -> (w1795:cluster{string, string})  [unwired: 1 out]
    n1350 = Bundle By Name(cluster=w1786, "Set 1"=w1774, "Set 2"=w1773) -> (→"Trap X AI1 (DMA)":T13)
    n1351 = Cluster To Array(cluster=w1795) -> (array=w1792:string[])
    n1352 = for "Trap Position" {
      tunnel: w1801 -> [w2048] mode=indexing
      tunnel: "Trap Disp. Downsample" -> [w2047]
      tunnel: w1799 -> [w2045]
      tunnel: w1797 -> [w2044]
      tunnel: w1796 -> [w2042]
      tunnel: w1792 -> [w2041] mode=indexing
      tunnel: [w2040] -> w1750 mode=indexing
      tunnel: w1752 -> [w2038] mode=indexing
      tunnel: w1751 -> [w2036]
      n1353 = call "downsample 1D array - double.vi"("Ave N"=w2047, "Array In"=w2048) -> ("Array Out"=w2046:dbl[])  [unwired: 1 out]
      n1354 = Subtract(x=w2046, y=w2038) -> (x-y=w2039:dbl[])
      n1355 = Multiply(x=w2036, y=w2039) -> (x*y=w2037:dbl[])
      n1356 = Bundle By Name("Y"=w2037, "dt"=w2045, "t0"=w2044) -> (w2043:waveform(dbl))  [unwired: 1 out]
      n1357 = Set Waveform Attribute(5:w2041, 6:w2042, 7:w2043) -> (3:w2040:waveform(dbl))  [unwired: 1 in, 2 out]
    }
    "Trap Positions" <- w1750
    n1358 = Bundle("APD 1", "APD 2") -> (w1987:cluster{string, string})  [unwired: 1 out]
    n1359 = Cluster To Array(cluster=w1987) -> (array=w1984:string[])
    n1360 = for "APD" {
      tunnel: w1955 -> [w2387] mode=indexing
      tunnel: w1824 -> [w2395]
      tunnel: [w2391] -> w1831 mode=indexing
      tunnel: "APD Disp. Scale" -> [w2392]
      tunnel: w1796 -> [w2390]
      tunnel: w1984 -> [w2389] mode=indexing
      tunnel: "APD Disp. Downsample" -> [w2385]
      tunnel: [w2388] -> w1983
      tunnel: w1797 -> [w2384]
      n1361 = call "integrate 1D array interval - double.vi"("Ave N"=w2385, "Array In"=w2387) -> ("Array Out"=w2386:dbl[])  [unwired: 1 out]
      n1362 = Multiply(x=w2395, y=w2385) -> (x*y=w2388:dbl)
      n1363 = Divide(x=w2386, y=w2392) -> (x/y=w2393:dbl[])
      n1364 = Bundle By Name("t0"=w2384, "Y"=w2393, "dt"=w2388) -> (w2394:waveform(dbl))  [unwired: 1 out]
      n1365 = Set Waveform Attribute(5:w2389, 6:w2390, 7:w2394) -> (3:w2391:waveform(dbl))  [unwired: 1 in, 2 out]
    }
    "APD Display Period (s)" <- w1983
    n1366 = Reciprocal(x=w1983) -> (1/x=→"APD Display Freq. (Hz)":dbl)
    n1367 = local read "Display Period (s)"() -> (w1859:dbl)
    n1368 = Increment(x=w1966) -> (x+1=w1967:dbl)
    n1369 = Index Array(array=w1750, index=0) -> (element=w1748:waveform(dbl))
    n1370 = To Double Precision Float(number=w1875) -> (double precision float=w1874:dbl[])
    n1371 = feedback #2(w1967) -> (w1970:dbl)
    n1372 = Select(t=0, s=w1957, f=w1970) -> (s? t:f=w1963:dbl)
    n1373 = Array Size(array=w1874) -> (size(s)=w1969:i32)
    n1374 = Add(x=w1969, y=w1963) -> (x+y=w1964:dbl)
    n1375 = Unbundle By Name(w1748) -> ("Y"=w1746:dbl[])
    n1376 = feedback #3(w1875) -> (w1953:u32[])
    n1377 = Build Array (concatenate)(w1953, w1875) -> (w1950:u32[])
    n1378 = feedback #4(w1811) -> (w1830:u32[])
    n1379 = Divide(x="Bead Sep. Int. Time (s)", y=w1859) -> (x/y=w1744:dbl)
    n1380 = Build Array (concatenate)(w1830, w1811) -> (w1829:u32[])
    n1381 = Greater?(x=w1964, y=w1966) -> (0:w1965:bool)
    n1382 = feedback #5(w1746) -> (w1747:dbl[])
    n1383 = Build Array (concatenate)(w1746, w1747) -> (w1745:dbl[])
    n1384 = Select(t=w1963, s=w1965, f=w1964) -> (s? t:f=w1962:dbl)
    n1385 = feedback-in #2(w1962) -> ()
    n1386 = Array Size(array=w1950) -> (size(s)=w1947:i32)
    n1387 = Array Size(array=w1875) -> (size(s)=w1949:i32)
    n1388 = local read "MCL Scanning"() -> (w1960:bool)
    n1389 = local read "APD Integration Time (s)"() -> (w1838:dbl)
    n1390 = Build Array (concatenate)(w1831, w1988) -> (w1833:waveform(dbl)[])
    "All Signals" <- w1833
    n1391 = Split 1D Array(array=w1745, index=w1744) -> (first subarray=w1738:dbl[])  [unwired: 1 out]
    n1392 = feedback-in #5(w1738) -> ()
    n1393 = Multiply(x=w1949, y="APD Ave N") -> (x*y=w1948:dbl)
    n1394 = Greater?(x=w1947, y=w1948) -> (0:w1951:bool)
    n1395 = Not(x=w1965) -> (.not. x?=w1959:bool)
    n1396 = To Double Precision Float(number=w1811) -> (double precision float=w1810:dbl[])
    n1397 = call-poly <vilib>:"Mean.vi"("X"=w1738) -> ("mean"=w1737:dbl)  [unwired: 1 out]
    "Mean T1 Position (nm)" <- w1737
    n1398 = Subtract(x=w1738, y=w1737) -> (x-y=w1743:dbl[])
    n1399 = Square(x=w1743) -> (x^2=w1742:dbl[])
    n1400 = And(x=w1959, y=w1960) -> (x .and. y?=w1961:bool)
    n1401 = call-poly <vilib>:"Mean.vi"("X"=w1742) -> ("mean"=w1741:dbl)  [unwired: 1 out]
    n1402 = case shown="True" w1951 {
      tunnel: w1950 -> [w2168 w2175]
      tunnel: [w2168 w2173] -> w1891
      tunnel: w1948 -> [_ w2170]
      tunnel: w1947 -> [_ w2174]
      tunnel: w1829 -> [w2167 w2172]
      tunnel: [w2167 w2169] -> w1826
      frame False {
      }
      frame True {
        n1403 = Subtract(x=w2174, y=w2170) -> (x-y=w2171:dbl)
        n1404 = Array Subset(array=w2175, index=w2171, length=w2170) -> (w2173:u32[])
        n1405 = Array Subset(array=w2172, index=w2171, length=w2170) -> (w2169:u32[])
      }
    }
    n1406 = feedback-in #3(w1891) -> ()
    n1407 = feedback-in #4(w1826) -> ()
    n1408 = Or(x=w1961, y=w1957) -> (x .or. y?=w1958:bool)
    n1409 = Square Root(x=w1741) -> (sqrt(x)=w1740:dbl)
    n1410 = Equal?(x="Tab Control 6", y=T33."High Res Display") -> (x = y?=w1881:bool)
    n1411 = Multiply(x="APD Disp. Scale", y=w1831) -> (x*y=w1840:waveform(dbl)[])
    n1412 = Multiply(x="APD Disp. Downsample", y=w1838) -> (x*y=w1836:dbl)
    n1413 = Multiply(x=10.0, y=w1740) -> (x*y=→"Trap 1 Position RMS (A)":dbl)
    n1414 = Divide(x=w1840, y=w1836) -> (x/y=w1808:waveform(dbl)[])
    n1415 = Index Array(array=w1808, index=0) -> (element=w1818:waveform(dbl))
    n1416 = case "For computing FFTs for display" shown="True" "Compute FFT" {
      tunnel: w1835 -> [_ w2845]
      frame False {
      }
      frame True {
        n1417 = Build Array("FFT 1 Choice 1", "FFT 1 Choice 2", "FFT 2 Choice 1", "FFT 2 Choice 2") -> (w2838:u16[])
        n1418 = Array Size(array=w2845) -> (size(s)=w2844:i32)
        n1419 = feedback-in #6(w2838) -> ()
        n1420 = feedback #6(u16[] [100, 100, 100, 100]) -> (w2839:u16[])
        n1421 = feedback-in #7("# Spectra to Ave.") -> ()
        n1422 = feedback #7("# Spectra to Ave.") -> (w2836:dbl)
        n1423 = Not Equal?(x="# Spectra to Ave.", y=w2836) -> (x != y?=w2835:bool)
        n1424 = Not Equal?(x=w2838, y=w2839) -> (x != y?=w2837:bool)
        n1425 = feedback #8(1.0) -> (w2822:dbl)
        n1426 = Compound Arithmetic op=OR("Reset FFT", w2837, w2835) -> (w2820:bool)
        n1427 = Select(t=1.0, s=w2820, f=w2822) -> (s? t:f=w2824:dbl)
        n1428 = Greater?(x=w2824, y="# Spectra to Ave.") -> (0:w2843:bool)
        n1429 = Increment(x=w2824) -> (x+1=w2823:dbl)
        n1430 = feedback-in #8(w2823) -> ()
        n1431 = local read "DMA Update Period (s)"() -> (w2818:dbl)
        n1432 = Multiply(x="# Spectra to Ave.", y=w2818) -> (x*y=→"Ave. Time (s)":dbl)
        n1433 = Build Array(cluster{"f0":dbl, "df":dbl, "magnitude":dbl[]} {"f0"=0.0, "df"=0.0, "magnitude"=[]} ("PSD")) -> (w2827:cluster{"f0":dbl, "df":dbl, "magnitude":dbl[]}[])
        n1434 = Build Array(w2827, w2827, w2827, w2827) -> (w2829:T44)
        n1435 = feedback #9(w2829) -> (w2834:T44)
        n1436 = for {
          N: 4 -> [_]
          tunnel: w2838 -> [w2867] mode=indexing
          tunnel: w2845 -> [w2868]
          tunnel: w2844 -> [w2870]
          tunnel: w2820 -> [w2863]
          tunnel: w2843 -> [w2862]
          tunnel: "# Spectra to Ave." -> [w2861]
          tunnel: [w2860] -> w2833 mode=indexing
          tunnel: w2834 -> [w2865] mode=indexing
          tunnel: [w2864] -> w2821 mode=indexing
          tunnel: w2824 -> [w2859]
          n1437 = Less?(x=w2867, y=w2870) -> (x < y?=w2869:bool)
          n1438 = Index Array(array=w2868, index=w2867) -> (element=w2866:waveform(dbl))
          n1439 = case shown="True" w2869 {
            tunnel: w2866 -> [_ w2887]
            tunnel: w2865 -> [w2872 w2885]
            tunnel: [w2872 w2873] -> w2864
            tunnel: w2863 -> [_ w2884]
            tunnel: w2862 -> [_ w2877]
            tunnel: w2861 -> [_ w2876]
            tunnel: [cluster{"f0":dbl, "df":dbl, "magnitude":dbl[]} {"f0"=0.0, "df"=0.0, "magnitude"=[]} ("PSD") w2878] -> w2860
            tunnel: w2859 -> [_ w2875]
            frame False {
            }
            frame True {
              n1440 = call <vilib>:"Std Deviation and Variance.vi"("X"=w2887) -> ("mean"=w2888:dbl)  [unwired: 1 in, 2 out]
              n1441 = Subtract(x=w2887, y=w2888) -> (x-y=w2886:waveform(dbl))
              n1442 = xnode "Spectral Measurements"("Signals"=w2886) -> ("PSD"=w2880:cluster{"f0":dbl, "df":dbl, "magnitude":dbl[]})  [unwired: 1 in, 1 out]
              n1443 = case shown="False" w2884 {
                tunnel: w2885 -> [w2897 _]
                tunnel: [w2893 w2902] -> w2873
                tunnel: w2880 -> [w2896 w2903]
                tunnel: w2877 -> [w2895 _]
                frame False {
                  n1444 = Build Array (concatenate)(w2897, w2896) -> (w2894:cluster{"f0":dbl, "df":dbl, "magnitude":dbl[]}[])
                  n1445 = case shown="True" w2895 {
                    tunnel: w2894 -> [w2898 w2901]
                    tunnel: [w2898 w2899] -> w2893
                    frame False {
                    }
                    frame True {
                      n1446 = Delete From Array(array=w2901, index=0) -> (array with subset deleted=w2899:cluster{"f0":dbl, "df":dbl, "magnitude":dbl[]}[])  [unwired: 1 in, 1 out]
                    }
                  }
                }
                frame True {
                  n1447 = Build Array(w2903) -> (w2902:cluster{"f0":dbl, "df":dbl, "magnitude":dbl[]}[])
                }
              }
              n1448 = for {
                tunnel: w2873 -> [w2892] mode=indexing
                tunnel: [w2891] -> w2883 mode=indexing
                workers-P: _ -> [_]
                n1449 = Unbundle By Name(w2892) -> ("magnitude"=w2891:dbl[])
              }
              n1450 = Transpose 2D Array(2D array=w2883) -> (transposed array=w2882:dbl[][])
              n1451 = for {
                tunnel: w2882 -> [w2890] mode=indexing
                tunnel: [w2889] -> w2881 mode=indexing
                workers-P: _ -> [_]
                n1452 = Add Array Elements(numeric array=w2890) -> (sum=w2889:dbl)
              }
              n1453 = Select(t=w2876, s=w2877, f=w2875) -> (s? t:f=w2874:dbl)
              n1454 = Divide(x=w2881, y=w2874) -> (x/y=w2879:dbl[])
              n1455 = Bundle By Name(cluster=w2880, "magnitude"=w2879) -> (w2878:cluster{"f0":dbl, "df":dbl, "magnitude":dbl[]})
            }
          }
        }
        n1456 = case shown="True" w2820 {
          tunnel: w2821 -> [w2852 w2858]
          tunnel: [w2852 w2853] -> w2819
          frame False {
          }
          frame True {
            n1457 = Array Subset(array=w2858, index (row)=0 ("index"), length (row)=4 ("length"), index (col)=0 ("index"), length (col)=1 ("length")) -> (w2853:T44)
          }
        }
        n1458 = feedback-in #9(w2819) -> ()
        n1459 = Split 1D Array(array=w2833, index=2) -> (first subarray=→"FFT 1":cluster{"f0":dbl, "df":dbl, "magnitude":dbl[]}[], second subarray=→"FFT 2":cluster{"f0":dbl, "df":dbl, "magnitude":dbl[]}[])
      }
    }
    n1460 = Index Array(array=w1808, index=1) -> (element=w1816:waveform(dbl))
    n1461 = case "For displaying the high resolution display (no downsampling)" shown="True" w1881 {
      tunnel: w1835 -> [_ w2068]
      frame False {
      }
      frame True {
        n1462 = Index Array(array=w2068, index="High Res. Display") -> (element=w2069:waveform(dbl))
        n1463 = call <vilib>:"Std Deviation and Variance.vi"("X"=w2069) -> ("mean"=w2076:dbl, "standard deviation"=w2081:dbl)  [unwired: 1 in, 1 out]
        "Mean Intensity" <- w2076
        "Sigma" <- w2081
        n1464 = Subtract(x=w2069, y=w2076) -> (x-y=w2075:waveform(dbl))
        n1465 = Select(t=w2075, s="Subtract mean", f=w2069) -> (s? t:f=→"1 Channel":waveform(dbl))
        n1466 = Divide(x=w2081, y=w2076) -> (x/y=→"Sigma/Mean":dbl)
        n1467 = feedback #10(1) -> (w2070:i32)
        n1468 = Greater Or Equal?(x=w2070, y="Slow mean N ave.") -> (x >= y?=w2083:bool)
        n1469 = Increment(x=w2070) -> (x+1=w2085:i32)
        n1470 = Select(t=1, s=w2083, f=w2085) -> (s? t:f=w2072:i32)
        n1471 = feedback-in #10(w2072) -> ()
        n1472 = feedback #11() -> (w2073:waveform(dbl))  [unwired: 1 out]
        n1473 = case shown="Default" w2070 {
          tunnel: [w2088 w2091] -> w2074
          tunnel: w2073 -> [w2090 _]
          tunnel: w2069 -> [w2089 w2091]
          frame Default {
            n1474 = call-poly <vilib>:"Append Waveforms.vi"("waveform B"=w2089, "waveform A"=w2090) -> ("waveform out"=w2088:waveform(dbl))  [unwired: 1 in, 8 out]
          }
          frame 1 {
          }
        }
        n1475 = feedback-in #11(w2074) -> ()
        n1476 = case shown="True" w2083 {
          tunnel: w2074 -> [_ w2087]
          frame False {
          }
          frame True {
            n1477 = call-poly <vilib>:"Mean.vi"("X"=w2087) -> ("mean"=→"Slow mean":dbl)  [unwired: 1 out]
          }
        }
      }
    }
    n1478 = case "For plotting results of scanning MCL" shown="True" w1958 {
      tunnel: w1957 -> [_ w2208]
      tunnel: w1874 -> [_ w2304]
      tunnel: w1966 -> [_ _]
      tunnel: w1835 -> [_ w2278]
      tunnel: w1810 -> [_ w2209]
      tunnel: w1809 -> [_ w2182]
      frame False {
      }
      frame True {
        w2189 = u32 0 items=["Horizontal", "Vertical", "Central", "1st Diagonal", "2nd Diagonal"] ("Type of Symmetry")
        w2217 = u32 0 items=["Horizontal", "Vertical", "Central", "1st Diagonal", "2nd Diagonal"] ("Type of Symmetry")
        w2220 = u32 0 items=["Horizontal", "Vertical", "Central", "1st Diagonal", "2nd Diagonal"] ("Type of Symmetry")
        w2249 = u32 0 items=["Horizontal", "Vertical", "Central", "1st Diagonal", "2nd Diagonal"] ("Type of Symmetry")
        n1479 = Index Array(array=w2278, index=10) -> (element=w2284:waveform(dbl))
        n1480 = Index Array(array=w2278, index=11) -> (element=w2281:waveform(dbl))
        n1481 = local read "Cycles/step (MCL)"() -> (w2234:u64)
        n1482 = Index Array(array=w2278, index="Channel") -> (element=w2280:waveform(dbl))
        n1483 = Unbundle(w2182) -> ("New Image"=w2181:T2, "New Image"=w2180:T2, "New Image"=w2179:T2, "New Image"=w2178:T2)
        n1484 = Unbundle By Name(w2284) -> ("Y"=w2236:dbl[])
        n1485 = Unbundle By Name(w2281) -> ("Y"=w2238:dbl[])
        n1486 = Unbundle By Name(w2280) -> ("Y"=w2243:dbl[])
        n1487 = call "downsample 1D array - double.vi"("Ave N"=w2234, "Array In"=w2236) -> ("Array Out"=w2235:dbl[])  [unwired: 1 out]
        n1488 = call "downsample 1D array - double.vi"("Ave N"=w2234, "Array In"=w2238) -> ("Array Out"=w2237:dbl[])  [unwired: 1 out]
        n1489 = call "downsample 1D array - double.vi"("Ave N"=w2234, "Array In"=w2243) -> ("Array Out"=w2242:dbl[])  [unwired: 1 out]
        n1490 = feedback #12(w2304) -> (w2305:dbl[])
        n1491 = Build Array (concatenate)(w2305, w2304) -> (w2286:dbl[])
        n1492 = feedback #13(w2209) -> (w2211:dbl[])
        n1493 = Build Array (concatenate)(w2211, w2209) -> (w2210:dbl[])
        n1494 = local read "Scan steps (MCL)"() -> (w2191:u64)
        n1495 = Select(t=w2304, s=w2208, f=w2286) -> (s? t:f=w2290:dbl[])
        n1496 = feedback-in #12(w2290) -> ()
        n1497 = Select(t=w2209, s=w2208, f=w2210) -> (s? t:f=w2192:dbl[])
        n1498 = feedback-in #13(w2192) -> ()
        n1499 = local read "Scan lines (y)"() -> (w2177:u64)
        n1500 = local read "N APD Samp/step"() -> (w2193:dbl)
        n1501 = feedback #14(w2235) -> (w2292:dbl[])
        n1502 = Build Array (concatenate)(w2292, w2235) -> (w2283:dbl[])
        n1503 = feedback #15(w2242) -> (w2302:dbl[])
        n1504 = Build Array (concatenate)(w2302, w2242) -> (w2301:dbl[])
        n1505 = feedback #16(w2237) -> (w2294:dbl[])
        n1506 = Build Array (concatenate)(w2294, w2237) -> (w2295:dbl[])
        n1507 = Select(t=w2235, s=w2208, f=w2283) -> (s? t:f=w2239:dbl[])
        n1508 = feedback-in #14(w2239) -> ()
        n1509 = Select(t=w2242, s=w2208, f=w2301) -> (s? t:f=w2241:dbl[])
        n1510 = feedback-in #15(w2241) -> ()
        n1511 = Select(t=w2237, s=w2208, f=w2295) -> (s? t:f=w2240:dbl[])
        n1512 = feedback-in #16(w2240) -> ()
        n1513 = Multiply(x=w2191, y=u64 2) -> (x*y=w2176:u64)
        n1514 = call "integrate 1D array interval - double.vi"("Ave N"=w2193, "Array In"=w2192) -> ("Array Out"=w2204:dbl[])  [unwired: 1 out]
        n1515 = call "integrate 1D array interval - double.vi"("Ave N"=w2193, "Array In"=w2290) -> ("Array Out"=w2289:dbl[])  [unwired: 1 out]
        n1516 = Array Size(array=w2204) -> (size(s)=w2205:i32)
        n1517 = Array Size(array=w2289) -> (size(s)=w2291:i32)
        n1518 = Multiply(x=w2177, y=w2176) -> (x*y=w2207:u64)
        n1519 = Multiply(x=w2177, y=w2176) -> (x*y=w2299:u64)
        n1520 = call-poly <vilib>:"Mean.vi"("X"=w2239) -> ("mean"=w2223:dbl)  [unwired: 1 out]
        n1521 = Subtract(x=w2207, y=w2205) -> (x-y=w2198:u64)
        n1522 = call-poly <vilib>:"Mean.vi"("X"=w2241) -> ("mean"=w2228:dbl)  [unwired: 1 out]
        n1523 = call-poly <vilib>:"Mean.vi"("X"=w2240) -> ("mean"=w2226:dbl)  [unwired: 1 out]
        n1524 = call-poly <vilib>:"Mean.vi"("X"=w2204) -> ("mean"=w2195:dbl)  [unwired: 1 out]
        n1525 = Subtract(x=w2299, y=w2291) -> (x-y=w2233:u64)
        n1526 = call-poly <vilib>:"Mean.vi"("X"=w2289) -> ("mean"=w2230:dbl)  [unwired: 1 out]
        n1527 = Initialize Array(1.0 ("element"), w2198) -> (w2194:dbl[])
        n1528 = Initialize Array(1.0 ("element"), w2233) -> (w2224:dbl[])
        n1529 = Multiply(x=w2194, y=w2195) -> (x*y=w2196:dbl[])
        n1530 = Multiply(x=w2224, y=w2226) -> (x*y=w2227:dbl[])
        n1531 = Multiply(x=w2224, y=w2228) -> (x*y=w2229:dbl[])
        n1532 = Multiply(x=w2224, y=w2223) -> (x*y=w2225:dbl[])
        n1533 = Multiply(x=w2224, y=w2230) -> (x*y=w2231:dbl[])
        n1534 = Build Array (concatenate)(w2239, w2225) -> (w2293:dbl[])
        n1535 = Build Array (concatenate)(w2241, w2229) -> (w2297:dbl[])
        n1536 = Build Array (concatenate)(w2240, w2227) -> (w2296:dbl[])
        n1537 = Build Array (concatenate)(w2204, w2196) -> (w2206:dbl[])
        n1538 = Build Array (concatenate)(w2289, w2231) -> (w2298:dbl[])
        n1539 = Reshape Array(w2293, w2177, w2176) -> (w2259:dbl[][])
        n1540 = Reshape Array(w2206, w2177, w2176) -> (w2202:dbl[][])
        n1541 = Reshape Array(w2297, w2177, w2176) -> (w2251:dbl[][])
        n1542 = Reshape Array(w2296, w2177, w2176) -> (w2266:dbl[][])
        n1543 = Reshape Array(w2298, w2177, w2176) -> (w2276:dbl[][])
        n1544 = Array Subset(array=w2266, index (col)=0 ("index"), length (col)=w2191) -> (w2271:dbl[][])  [unwired: 2 in]
        n1545 = Array Subset(array=w2266, index (col)=w2191) -> (w2269:dbl[][])  [unwired: 3 in]
        n1546 = Array Subset(array=w2251, index (col)=0 ("index"), length (col)=w2191) -> (w2257:dbl[][])  [unwired: 2 in]
        n1547 = Array Subset(array=w2251, index (col)=w2191) -> (w2255:dbl[][])  [unwired: 3 in]
        n1548 = Array Subset(array=w2202, index (col)=0 ("index"), length (col)=w2191) -> (w2201:dbl[][])  [unwired: 2 in]
        n1549 = Array Subset(array=w2202, index (col)=w2191) -> (w2199:dbl[][])  [unwired: 3 in]
        n1550 = Array Subset(array=w2276, index (col)=0 ("index"), length (col)=w2191) -> (w2275:dbl[][])  [unwired: 2 in]
        n1551 = Array Subset(array=w2276, index (col)=w2191) -> (w2273:dbl[][])  [unwired: 3 in]
        n1552 = Array Subset(array=w2259, index (col)=0 ("index"), length (col)=w2191) -> (w2264:dbl[][])  [unwired: 2 in]
        n1553 = Array Subset(array=w2259, index (col)=w2191) -> (w2262:dbl[][])  [unwired: 3 in]
        n1554 = for {
          tunnel: w2271 -> [w2313] mode=indexing
          tunnel: [w2312] -> w2270 mode=indexing
          workers-P: _ -> [_]
          n1555 = Reverse 1D Array(array=w2313) -> (reversed array=w2312:dbl[])
        }
        n1556 = for {
          tunnel: w2257 -> [w2309] mode=indexing
          tunnel: [w2308] -> w2256 mode=indexing
          workers-P: _ -> [_]
          n1557 = Reverse 1D Array(array=w2309) -> (reversed array=w2308:dbl[])
        }
        n1558 = for {
          tunnel: w2201 -> [w2307] mode=indexing
          tunnel: [w2306] -> w2200 mode=indexing
          workers-P: _ -> [_]
          n1559 = Reverse 1D Array(array=w2307) -> (reversed array=w2306:dbl[])
        }
        n1560 = for {
          tunnel: w2275 -> [w2315] mode=indexing
          tunnel: [w2314] -> w2274 mode=indexing
          workers-P: _ -> [_]
          n1561 = Reverse 1D Array(array=w2315) -> (reversed array=w2314:dbl[])
        }
        n1562 = for {
          tunnel: w2264 -> [w2311] mode=indexing
          tunnel: [w2310] -> w2263 mode=indexing
          workers-P: _ -> [_]
          n1563 = Reverse 1D Array(array=w2311) -> (reversed array=w2310:dbl[])
        }
        n1564 = Index Array(array=w2276, index (row)=0) -> (element=→"Waveform Graph":dbl[])  [unwired: 1 in]
        n1565 = Add(x=w2270, y=w2269) -> (x+y=w2268:dbl[][])
        n1566 = Add(x=w2256, y=w2255) -> (x+y=w2254:dbl[][])
        n1567 = Add(x=w2200, y=w2199) -> (x+y=w2184:dbl[][])
        n1568 = Add(x=w2274, y=w2273) -> (x+y=w2248:dbl[][])
        n1569 = Add(x=w2263, y=w2262) -> (x+y=w2261:dbl[][])
        n1570 = Divide(x=w2254, y=2) -> (x/y=w2252:dbl[][])
        n1571 = Divide(x=w2268, y=2) -> (x/y=w2213:dbl[][])
        n1572 = Divide(x=w2261, y=2) -> (x/y=w2215:dbl[][])
        n1573 = To Single Precision Float(number=w2248) -> (single precision float=w2247:sgl[][])
        n1574 = Transpose 2D Array(2D array=w2252) -> (transposed array=→"Data map":dbl[][])
        n1575 = To Single Precision Float(number=w2184) -> (single precision float=w2188:sgl[][])
        n1576 = To Single Precision Float(number=w2213) -> (single precision float=w2219:sgl[][])
        n1577 = To Single Precision Float(number=w2215) -> (single precision float=w2216:sgl[][])
        n1578 = call "IMAQ ArrayToImage"("Image Pixels (Float)"=w2247, "Image"=w2181) -> ("Image Out"=w2250:T2)  [unwired: 8 in, 1 out]
        n1579 = call "IMAQ ArrayToImage"("Image Pixels (Float)"=w2188, "Image"=w2180) -> ("Image Out"=w2190:T2)  [unwired: 8 in, 1 out]
        n1580 = call "IMAQ ArrayToImage"("Image Pixels (Float)"=w2219, "Image"=w2179) -> ("Image Out"=w2221:T2)  [unwired: 8 in, 1 out]
        n1581 = call "IMAQ ArrayToImage"("Image Pixels (Float)"=w2216, "Image"=w2178) -> ("Image Out"=w2218:T2)  [unwired: 8 in, 1 out]
        n1582 = call "IMAQ Symmetry"("Type of Symmetry"=w2249, "Image Src"=w2250) -> ("Image Dst Out"=w2245:T2)  [unwired: 3 in, 1 out]
        n1583 = call "IMAQ Symmetry"("Type of Symmetry"=w2189, "Image Src"=w2190) -> ("Image Dst Out"=w2186:T2)  [unwired: 3 in, 1 out]
        n1584 = call "IMAQ Symmetry"("Type of Symmetry"=w2220, "Image Src"=w2221) -> ("Image Dst Out"=→"Detection Laser X":T2)  [unwired: 3 in, 1 out]
        n1585 = call "IMAQ Symmetry"("Type of Symmetry"=w2217, "Image Src"=w2218) -> ("Image Dst Out"=→"Detection Laser Y":T2)  [unwired: 3 in, 1 out]
        n1586 = call "IMAQ Set Simple Calibration"("Calibration Axis Info"=T34 {"Origin Pixel"={"X"=0.0, "Y"=0.0}, "Angle Relative to Horizontal (deg)"=0.0, "Axis Reference"=0}, "Grid Descriptor"=T35 {"X Step"=0.3, "Y Step"=0.3, "Unit"=enum."Undefined"}, "Image"=w2245) -> ("Calibrated Image"=→"APD 1":T2)  [unwired: 7 in, 1 out]
        n1587 = call "IMAQ Set Simple Calibration"("Calibration Axis Info"=T34 {"Origin Pixel"={"X"=0.0, "Y"=0.0}, "Angle Relative to Horizontal (deg)"=0.0, "Axis Reference"=0}, "Grid Descriptor"=T35 {"X Step"=0.3, "Y Step"=0.3, "Unit"=enum."Undefined"}, "Image"=w2186) -> ("Calibrated Image"=→"APD 2":T2)  [unwired: 7 in, 1 out]
      }
    }
    n1588 = Subtract(x=w1816, y="APD 2 Offset") -> (x-y=w1813:waveform(dbl))
    n1589 = Subtract(x=w1818, y="APD 1 Offset") -> (x-y=w1814:waveform(dbl))
    n1590 = Index Array(array=w1833, index=3) -> (element=w1902:waveform(dbl))
    n1591 = Index Array(array=w1833, index=6) -> (element=w1899:waveform(dbl))
    n1592 = Build Array(w1814, w1813) -> (→"APD Chart":waveform(dbl)[])
    n1593 = Array Size(array=w1891) -> (size(s)=w1946:i32)
    n1594 = call <vilib>:"Std Deviation and Variance.vi"("X"=w1826) -> ("standard deviation"=w1825:dbl)  [unwired: 1 in, 2 out]
    n1595 = Add Array Elements(numeric array=w1826) -> (sum=w1828:u32)
    n1596 = Add Array Elements(numeric array=w1891) -> (sum=w1956:u32)
    n1597 = call <vilib>:"Std Deviation and Variance.vi"("X"=w1891) -> ("standard deviation"=w1890:dbl)  [unwired: 1 in, 2 out]
    n1598 = Divide(x="T1 offset_x (mV)", y=1000.0) -> (x/y=w1903:dbl)
    n1599 = Divide(x=w1825, y=w1824) -> (x/y=w1821:dbl)
    "Rate sigma (Hz) 2" <- w1821
    n1600 = Multiply(x=w1824, y=w1946) -> (x*y=w1827:dbl)
    "Int. Time (s)" <- w1827
    n1601 = Divide(x=w1828, y=w1827) -> (x/y=w1822:dbl)
    "APD 2 Rate (Hz)" <- w1822
    n1602 = Divide(x=w1956, y=w1827) -> (x/y=w1888:dbl)
    "APD 1 Rate (Hz)" <- w1888
    n1603 = Divide(x=w1890, y=w1824) -> (x/y=w1889:dbl)
    "Rate sigma (Hz)" <- w1889
    n1604 = Divide(x=w1821, y=w1822) -> (x/y=→"Sigma/Mean 2":dbl)
    n1605 = Divide(x=w1889, y=w1888) -> (x/y=→"Sigma/Mean":dbl)
    n1606 = Divide(x="T2 offset_x (mV)", y=1000.0) -> (x/y=w1901:dbl)
    n1607 = case shown="1" "Calibration" {
      tunnel: "T1 alpha_x (nm/V)" -> [_ w2144 w2165]
      tunnel: "T1 kappa_x (pN/nm)" -> [_ _ w2155]
      tunnel: "T2 alpha_x (nm/V)" -> [_ w2143 w2163]
      tunnel: "T2 kappa_x (pN/nm)" -> [_ _ w2156]
      tunnel: w1902 -> [w2126 w2141 w2161]
      tunnel: w1899 -> [w2125 w2139 w2159]
      tunnel: [w2126 w2138 w2158] -> w1932
      tunnel: [w2125 w2137 w2157] -> w1931
      tunnel: ["T1 X (V)" ("Label.Text") "T1 X (nm)" ("Label.Text") "T1 X (pN)" ("Label.Text")] -> w1920
      tunnel: ["T2 X (V)" ("Label.Text") "T2 X (nm)" ("Label.Text") "T2 X (pN)" ("Label.Text")] -> w1919
      tunnel: ["Position (V)" ("Label.Text") "Position (nm)" ("Label.Text") "Force (pN)" ("Label.Text")] -> w1921
      tunnel: w1901 -> [_ w2129 w2148]
      tunnel: w1903 -> [_ w2132 w2150]
      tunnel: ["Mean (V)" ("Label.Text") "Mean (nm)" ("Label.Text") "Mean (pN)" ("Label.Text")] -> w1916
      tunnel: ["Difference (V)" ("Label.Text") "Difference (nm)" ("Label.Text") "Difference (pN)" ("Label.Text")] -> w1841
      frame 0, Default {
      }
      frame 1 {
        # "position"
        n1608 = Unbundle By Name(w2141) -> ("Y"=w2145:dbl[])
        n1609 = Unbundle By Name(w2139) -> ("Y"=w2130:dbl[])
        n1610 = Subtract(x=w2145, y=w2132) -> (x-y=w2133:dbl[])
        n1611 = Subtract(x=w2130, y=w2129) -> (x-y=w2131:dbl[])
        n1612 = Multiply(x=w2131, y=w2143) -> (x*y=w2140:dbl[])
        n1613 = Multiply(x=w2144, y=w2133) -> (x*y=w2142:dbl[])
        n1614 = Bundle By Name(cluster=w2139, "Y"=w2140) -> (w2137:waveform(dbl))
        n1615 = Bundle By Name(cluster=w2141, "Y"=w2142) -> (w2138:waveform(dbl))
      }
      frame 2 {
        # "force"
        n1616 = Unbundle By Name(w2161) -> ("Y"=w2166:dbl[])
        n1617 = Unbundle By Name(w2159) -> ("Y"=w2164:dbl[])
        n1618 = Subtract(x=w2164, y=w2148) -> (x-y=w2149:dbl[])
        n1619 = Subtract(x=w2166, y=w2150) -> (x-y=w2151:dbl[])
        n1620 = Compound Arithmetic op=MULTIPLY(w2149, w2163, w2156) -> (w2160:dbl[])
        n1621 = Compound Arithmetic op=MULTIPLY(w2155, w2165, w2151) -> (w2162:dbl[])
        n1622 = Bundle By Name(cluster=w2159, "Y"=w2160) -> (w2157:waveform(dbl))
        n1623 = Bundle By Name(cluster=w2161, "Y"=w2162) -> (w2158:waveform(dbl))
      }
    }
    n1624 = feedback-in #17("Calibration") -> ()
    n1625 = feedback #17(u16 1 ("Calibration")) -> (w1923:u16)
    n1626 = Not Equal?(x=w1923, y="Calibration") -> (x != y?=w1879:bool)
    n1627 = Unbundle By Name(w1902) -> ("Y"=w1905:dbl[])
    n1628 = Unbundle By Name(w1899) -> ("Y"=w1908:dbl[])
    n1629 = Subtract(x=w1905, y=w1903) -> (x-y=w1906:dbl[])
    n1630 = Subtract(x=w1908, y=w1901) -> (x-y=w1907:dbl[])
    n1631 = disable-structure shown="Enabled" {
      disable-tunnel: [-1.0 ("y") 1.0] -> w1909
      frame Disabled {
      }
      frame Enabled {
      }
    }
    n1632 = Multiply(x=w1907, y="T2 alpha_x (nm/V)") -> (x*y=w1898:dbl[])
    n1633 = Multiply(x="T1 alpha_x (nm/V)", y=w1906) -> (x*y=w1897:dbl[])
    n1634 = Multiply(x=w1931, y=w1909) -> (x*y=w1910:waveform(dbl))
    n1635 = case shown="True" "Read Lateness and Rel Phase" {
      tunnel: w1733 -> [w2092 w2114]
      tunnel: w1732 -> [w2093 w2113]
      tunnel: [w2092 w2112] -> w1894
      tunnel: [w2093 w2111] -> w1893
      frame False {
      }
      frame True {
        n1636 = xnode "Read/Write Control"("FPGA VI Reference In"=w2114, "error in"=w2113) -> ("FPGA VI Reference Out"=w2112:T19, "error out"=w2111:errorcluster, "GI Relative phase"=→"GI relative phase":i16, "Relative phase"=→"Relative phase (AI1)":i16, "AI Late Counter"=→"Late Counter (AI1)":u16, "GI Late Counter"=→"GI Late Counter":u16, "MCL Late Counter"=→"MCL Late Counter":u16, "MCL Relative Phase"=→"Relative Phase (MCL)":i16, "APD Acq Relative Phase"=→"APD Acq Relative Phase":i16, "APD 1 Gate Relative Phase"=→"APD 1 Gate Relative Phase":i16, "APD 2 Gate Relative Phase"=→"APD 2 Gate Relative Phase":i16, "APD Acq Late Counter"=→"APD Acq Late Counter":u16, "APD 1 Gate Late Counter"=→"APD 1 Gate Late Counter":u16, "APD 2 Gate Late Counter"=→"APD 2 Gate Late Counter":u16, "Green FB Relative Phase"=→"Relative phase (Green FB)":i16, "GI Relative phase 2"=→"GI relative phase 2":i16, "GI Late Counter 2"=→"GI Late Counter 2":u16, "Trap Pos FIFO Timeout"=→"Trap Pos FIFO Timeout":u16, "Trap AI FIFO Timeout"=→"Trap AI FIFO Timeout":u16)
      }
    }
    n1637 = Subtract(x=w1898, y=w1897) -> (x-y=w1896:dbl[])
    n1638 = Unbundle By Name(w1931) -> ("Y"=w1866:dbl[])
    n1639 = Unbundle By Name(w1932) -> ("Y"=w1867:dbl[])
    n1640 = Build Array(w1932, w1910) -> (→"Force":waveform(dbl)[])
    n1641 = Subtract(x=w1896, y="Offset (nm)") -> (x-y=w1864:dbl[])
    n1642 = call-poly <vilib>:"Mean.vi"("X"=w1866) -> ("mean"=w1845:dbl)  [unwired: 1 out]
    "T2 X" <- w1845
    n1643 = Absolute Value(x=w1867) -> (abs(x)=w1868:dbl[])
    n1644 = Absolute Value(x=w1866) -> (abs(x)=w1869:dbl[])
    n1645 = call-poly <vilib>:"Mean.vi"("X"=w1867) -> ("mean"=w1846:dbl)  [unwired: 1 out]
    "T1 X" <- w1846
    n1646 = Add(x=w1868, y=w1869) -> (x+y=w1870:dbl[])
    n1647 = Bundle By Name(cluster=w1902, "Y"=w1864) -> (w1832:waveform(dbl))
    "Bead Separation" <- w1832
    n1648 = Divide(x=w1870, y=2.0) -> (x/y=→"Vec Mean of T1 T2":dbl[])
    n1649 = case shown="True" w1879 {
      tunnel: w1921 -> [_ w2119]
      tunnel: w1920 -> [_ w2118]
      tunnel: w1919 -> [_ w2117]
      tunnel: w1916 -> [_ w2116]
      tunnel: w1841 -> [_ w2115]
      frame False {
      }
      frame True {
        n1650 = property on="Force" class="WFChart (strict)"("YScale.NameLbl.Text"=w2119) -> ()  [unwired: 2 in, 2 out]
        n1651 = property on="T2 X" class="DigNum (strict)"("Caption.Text"=w2117) -> ()  [unwired: 2 in, 2 out]
        n1652 = property on="T1 X" class="DigNum (strict)"("Caption.Text"=w2118) -> ()  [unwired: 2 in, 2 out]
        n1653 = property on="Mean" class="DigNum (strict)"("Caption.Text"=w2116) -> ()  [unwired: 2 in, 2 out]
        n1654 = property on="Difference" class="DigNum (strict)"("Caption.Text"=w2115) -> ()  [unwired: 2 in, 2 out]
      }
    }
    n1655 = local read "Tether"() -> (w1873:bool)
    n1656 = Absolute Value(x=w1846) -> (abs(x)=w1843:dbl)
    n1657 = Absolute Value(x=w1845) -> (abs(x)=w1842:dbl)
    n1658 = Add(x=w1843, y=w1842) -> (x+y=w1918:dbl)
    n1659 = Subtract(x=w1843, y=w1842) -> (x-y=→"Difference":dbl)
    n1660 = feedback #18(w1864) -> (w1863:dbl[])
    n1661 = Divide(x=w1918, y=2.0) -> (x/y=w1872:dbl)
    "Mean" <- w1872
    n1662 = case shown="True" w1873 {
      tunnel: w1872 -> [_ w2051]
      frame False {
      }
      frame True {
        n1663 = Greater?(x="Lost Tether Alarm Threshold (pN)", y=w2051) -> (0:w2049:bool)
        n1664 = case shown="True" w2049 {
          frame False {
          }
          frame True {
            n1665 = flat-sequence {
              frame #0 {
                # "stop only if saving"
                n1666 = local read "Saving..."() -> (w2064:bool)
                n1667 = And(x=w2064, y="TA Cancel Save?") -> (x .and. y?=w2063:bool)
                n1668 = local write "Stop Saving"(w2063) -> ()
              }
              frame #1 {
                n1669 = case shown="True" "TA Green Off?" {
                  frame False {
                  }
                  frame True {
                    w2067 = FALSE ("Fl. Triggered...")
                    n1670 = local write "Fl. Triggered..."(w2067) -> ()
                    n1671 = property on="Green Laser ON/Interlacing" class="Bool (strict)"("Val(Sgnl)"=w2067) -> ()  [unwired: 2 in, 2 out]
                  }
                }
              }
            }
            n1672 = local read "Time tether formed"() -> (w2058:timestamp)
            n1673 = Get Date/Time In Seconds() -> (seconds since 1Jan1904=w2059:timestamp)
            n1674 = Subtract(x=w2059, y=w2058) -> (x-y=w2057:dbl)
            n1675 = Number To Decimal String(number=w2057) -> (decimal integer string=w2054:string)  [unwired: 1 out]
            n1676 = local read "Messages"() -> (w2061:string)
            n1677 = call <vilib>:"Beep.vi"() -> ()  [unwired: 3 in, 9 out]
            n1678 = Concatenate Strings("Lost tether (" ("Message to add"), w2054, " s)." ("string")) -> (w2056:string)
            n1679 = local write "Tether"(FALSE ("Tether")) -> ()
            n1680 = call "Update messages.vi"("Message to add"=w2056, "Old message string"=w2061) -> ("New message string"=w2060:string)
            n1681 = local write "Messages"(w2060) -> ()
            n1682 = property on="Trap Pos. FB ON" class="Bool (strict)"("Val(Sgnl)"=FALSE ("Value (Signaling)")) -> ()  [unwired: 2 in, 2 out]
          }
        }
      }
    }
    n1683 = Build Array (concatenate)(w1864, w1863) -> (w1862:dbl[])
    n1684 = Split 1D Array(array=w1862, index=w1744) -> (first subarray=w1858:dbl[])  [unwired: 1 out]
    n1685 = feedback-in #18(w1858) -> ()
    n1686 = call-poly <vilib>:"Mean.vi"("X"=w1858) -> ("mean"=w1857:dbl)  [unwired: 1 out]
    "Bead Mean (nm)" <- w1857
    n1687 = Subtract(x=w1858, y=w1857) -> (x-y=w1856:dbl[])
    n1688 = Square(x=w1856) -> (x^2=w1855:dbl[])
    n1689 = call-poly <vilib>:"Mean.vi"("X"=w1855) -> ("mean"=w1854:dbl)  [unwired: 1 out]
    n1690 = Square Root(x=w1854) -> (sqrt(x)=w1853:dbl)
    n1691 = Multiply(x=10.0, y=w1853) -> (x*y=→"RMS (Ang)":dbl)
    n1692 = xnode "Read/Write Control"("FPGA VI Reference In"=w1894, "error in"=w1893) -> ("FPGA VI Reference Out"=w2012:T19, "error out"=w2006:errorcluster, "AI2 Y Sum Set 1"=w2002:i16, "AI2 Y Sum Set 2"=w2001:i16, "AI1 X Set 1"=w1778:fxp<+/-,16,1>, "AI1 X Set 2"=w1777:fxp<+/-,16,1>, "Trap Pos FB Int Signal"=→"Trap Pos FB Int Signal":fxp<+/-,24,9>, "Trap Pos FB Int-Norm Signal"=→"Trap Pos FB Int-Norm Signal":fxp<+/-,16,1>, "Trap Pos FB Action"=w1771:i64, "Scanning"=→"AOD Scanning":bool, "Scan I"=→"AOD Scan I":u64, "Scanning MCL"=w2004:bool, "Scan I (MCL)"=→"MCL Scan I":u64, "Green FB Signals"=w1941:T45)  [unwired: 1 out]
    "MCL Scanning" <- w2004
    "Trap Pos FB Action" <- w1771
    n1693 = local read "AI2 (V)"() -> (w2003:cluster{"Set 1":dbl, "Set 2":dbl})
    n1694 = Bundle By Name(cluster=w2003, "Set 1"=w2002, "Set 2"=w2001) -> (w1999:cluster{"Set 1":dbl, "Set 2":dbl})
    n1695 = Divide(x=w1771, y=327.67) -> (x/y=→"Action (%)":dbl)
    n1696 = local read "Trap X (AI1)"() -> (w1791:T10)
    n1697 = Divide(x=w1999, y=3276.7) -> (x/y=w1998:cluster{"Set 1":dbl, "Set 2":dbl})
    n1698 = local write "AI2 (V)"(w1998) -> ()
    n1699 = Bundle(cluster=w1791, "Trap 1"=w1778, "Trap 2"=w1777) -> (→"Trap X (AI1)":T10)
    n1700 = Divide(x=w1941, y=3276.7) -> (x/y=w1937:T46)
    n1701 = Unbundle By Name(w1937) -> ("Green FB Ch 0"=w1940:dbl, "Green FB Ch 1"=w1939:dbl, "Green FB Ch 2"=w1938:dbl)
    n1702 = Divide(x=w1940, y=w1938) -> (x/y=w1936:dbl)
    n1703 = Divide(x=w1939, y=w1938) -> (x/y=w1935:dbl)
    n1704 = flat-sequence "To save data" {
      tunnel: [w2941] -> w2023
      tunnel: [w2942] -> w2022
      tunnel: w1972 -> [w2935]
      tunnel: w1860 -> [w2939]
      tunnel: ["Save Calibration"] -> w1995
      tunnel: w1992 -> [w2938]
      tunnel: [w2931] -> w1991
      tunnel: [w2928] -> w1990
      tunnel: [w2925] -> w1989
      tunnel: w1971 -> [w2927]
      tunnel: w1877 -> [w2921]
      tunnel: [w2921] -> w1876
      tunnel: ["Start Saving"] -> w1834
      tunnel: [w2915] -> w1760
      tunnel: [w2914] -> w1759
      tunnel: w2023 -> [w3176]
      tunnel: w2022 -> [w3175]
      tunnel: w1761 -> [w3174]
      tunnel: w1995 -> [w3173]
      tunnel: w1991 -> [w3171]
      tunnel: w1990 -> [w3170]
      tunnel: w1989 -> [w3169]
      tunnel: w1847 -> [w3168]
      tunnel: w1886 -> [w3167]
      tunnel: w1876 -> [w3166]
      tunnel: w1834 -> [w3165]
      tunnel: w1832 -> [w3164]
      tunnel: w1808 -> [w3163]
      tunnel: w1760 -> [w3162]
      tunnel: w1759 -> [w3161]
      tunnel: w1758 -> [w3160]
      frame #0 {
        n1705 = Or(x="Save N Sets", y="Start Saving") -> (x .or. y?=w2922:bool)
        n1706 = To Double Precision Float(number=w2938) -> (double precision float=w2932:dbl)
        n1707 = Build Array(w2922, "Save Calibration", w2935, w2927) -> (w2937:bool[])
        n1708 = Compound Arithmetic op=OR("Save Calibration", w2935, w2922, w2927) -> (w2940:bool)
        n1709 = Boolean Array To Number(Boolean array=w2937) -> (number=w2934:u32)
        n1710 = feedback #19(FALSE ("Save APD Data\nwith Trap Data")) -> (w2916:bool)
        n1711 = feedback #20(refnum<k0> refnum) -> (w2943:refnum<file>)
        n1712 = feedback #21(refnum<k0> refnum) -> (w2918:refnum<file>)
        n1713 = feedback #22(FALSE ("Save APD Data\nwith Trap Data")) -> (w2926:bool)
        n1714 = feedback #23(refnum<k0> refnum) -> (w2929:refnum<file>)
        n1715 = feedback #24(0) -> (w2945:i32)
        n1716 = feedback #25() -> (w2933:u32)  [unwired: 1 out]
        n1717 = case shown="True" w2940 {
          tunnel: [w2952 1] -> w2941
          tunnel: w2945 -> [w2954 _]
          tunnel: [w2953 w2972] -> w2942
          tunnel: w2943 -> [w2953 _]
          tunnel: w2939 -> [_ w2992]
          tunnel: w2932 -> [_ w2990]
          tunnel: w2934 -> [_ w2993]
          tunnel: [w2951 w2971] -> w2931
          tunnel: w2933 -> [w2951 _]
          tunnel: [w2950 w2969] -> w2928
          tunnel: w2929 -> [w2950 _]
          tunnel: [w2949 w2968] -> w2925
          tunnel: w2926 -> [w2949 _]
          tunnel: "Start Saving" -> [_ w2966]
          tunnel: w2921 -> [_ w2965]
          tunnel: [w2948 w2956] -> w2914
          tunnel: w2918 -> [w2948 _]
          tunnel: [w2947 w2955] -> w2915
          tunnel: w2916 -> [w2947 _]
          frame False {
            n1718 = Increment(x=w2954) -> (x+1=w2952:i32)
          }
          frame True {
            w2962 = FALSE ("Start Saving")
            w2967 = 9.0  # File Version
            w2975 = FALSE ("prepend array or string size? (T)")
            w2973 = T29."big-endian, network order" ("byte order (0:big-endian, network order)")
            # "write file headers"
            n1719 = local read "BD 1 Frequency 1 (MHz)"() -> (w2989:dbl)
            n1720 = local read "BD 2 Frequency 1 (MHz)"() -> (w2988:dbl)
            n1721 = local read "BD 1 Frequency 2 (MHz)"() -> (w2987:dbl)
            n1722 = local read "BD 2 Frequency 2 (MHz)"() -> (w2986:dbl)
            n1723 = local read "BD 1 Frequency 3 (MHz)"() -> (w2985:dbl)
            n1724 = local read "BD 2 Frequency 3 (MHz)"() -> (w2984:dbl)
            n1725 = Array Size(array=w2965) -> (size(s)=w2964:i32)
            n1726 = To Double Precision Float(number=w2964) -> (double precision float=w2963:dbl)
            n1727 = local write "Save Calibration"(w2962) -> ()
            n1728 = local write "Start Saving"(w2962) -> ()
            n1729 = Build Array("Save APD Data\nwith Trap Data", "Save Trap Pos. Data") -> (w2959:bool[])
            n1730 = Boolean Array To Number(Boolean array=w2959) -> (number=w2958:u32)
            n1731 = Build Array(w2989, w2988, w2987, w2986, w2985, w2984) -> (w2983:dbl[])
            n1732 = case shown="4" w2993 {
              tunnel: w2992 -> [w3064 w3084 w3100 w3138]
              tunnel: w2963 -> [w3069 w3091 w3120 w3157]
              tunnel: w2990 -> [w3068 w3090 w3119 w3156]
              tunnel: [w3065 w3086 w3111 w3148] -> w2981
              tunnel: [w3056 "Cal sets to save" w3101 w3139] -> w2971
              tunnel: w2983 -> [w3066 w3087 w3113 w3150]
              tunnel: "Save APD Data\nwith Trap Data" -> [w3063 _ w3097 w3136]
              tunnel: [w3063 w3078 w3097 w3136] -> w2968
              tunnel: w2967 -> [w3059 w3079 w3095 w3134]
              tunnel: w2966 -> [w3058 _ _ _]
              tunnel: [w3049 w3078 w3094 w3124] -> w2955
              tunnel: "Save Trap Pos. Data" -> [w3049 _ w3094 w3124]
              tunnel: w2958 -> [w3048 _ w3093 w3123]
              frame 1, Default {
                # "timeseries"
                n1733 = case shown="True" "Profile" {
                  tunnel: [w3072 w3075] -> w3053
                  tunnel: [w3072 w3074] -> w3052
                  tunnel: [w3072 w3073] -> w3051
                  tunnel: [w3072 w3077] -> w3050
                  frame False {
                    w3072 = 0.0 ("f")
                  }
                  frame True {
                    n1734 = local read "Current Position"() -> (w3076:dbl[])
                    n1735 = local read "Y change (mm)"() -> (w3077:dbl)
                    n1736 = call "subVI_explode3array.vi"("Array"=w3076) -> ("x"=w3075:dbl, "y"=w3074:dbl, "z"=w3073:dbl)  [unwired: 12 in]
                  }
                }
                n1737 = local read "Save ave N"() -> (w3071:dbl)
                n1738 = Multiply(x=w3071, y=w3064) -> (x*y=w3070:dbl)
                n1739 = To Double Precision Float(number=w3048) -> (double precision float=w3062:dbl)
                n1740 = Build Array(w3059, w3064, w3070, w3069, w3068, 0.0 ("f")) -> (w3067:dbl[])
                n1741 = Build Array(w3062, w3053, w3052, w3051, w3050) -> (w3060:dbl[])
                n1742 = Select(t=u32 4000000000, s=w3058, f="N sets to save") -> (s? t:f=w3056:u32)
                n1743 = Build Array (concatenate)(w3067, w3066, w3060) -> (w3065:dbl[])
              }
              frame 2 {
                w3081 = 0.0 ("f")
                w3078 = FALSE ("Save APD Data\nwith Trap Data")
                # "calibration"
                n1744 = Boolean To (0,1)(Boolean=w3078) -> (0, 1=w3083:i16)
                n1745 = To Double Precision Float(number=w3083) -> (double precision float=w3082:dbl)
                n1746 = Build Array(w3082, w3081, w3081, w3081, w3081) -> (w3080:dbl[])
                n1747 = Build Array(w3079, w3084, w3084, w3091, w3090, 1.0 ("t")) -> (w3088:dbl[])
                n1748 = Build Array (concatenate)(w3088, w3087, w3080) -> (w3086:dbl[])
                "Calibrating Trap..." <- TRUE ("Calibrating...")
              }
              frame 4 {
                w3098 = 0.0 ("f")
                # "write file header for a trap \nraster scan"
                # "scan dir (x/y = 0/1)"
                # "cycles/step"
                # "n scans (f/b)"
                # "steps"
                # "freq. range"
                # "AOD raster scan"
                n1749 = local read "Number of F/B Scans (AOD)"() -> (w3105:u16)
                n1750 = local read "Cycles/step (AOD)"() -> (w3107:u64)
                n1751 = local read "Scan Range (MHz)"() -> (w3110:dbl)
                n1752 = local read "Scan steps (AOD)"() -> (w3109:u64)
                n1753 = local read "Scan BD"() -> (w3117:bool)
                n1754 = local read "Save ave N"() -> (w3122:dbl)
                n1755 = Boolean To (0,1)(Boolean=w3117) -> (0, 1=w3116:i16)
                n1756 = To Double Precision Float(number=w3105) -> (double precision float=w3104:dbl)
                n1757 = To Double Precision Float(number=w3109) -> (double precision float=w3108:dbl)
                n1758 = To Double Precision Float(number=w3107) -> (double precision float=w3106:dbl)
                n1759 = To Double Precision Float(number=w3116) -> (double precision float=w3115:dbl)
                n1760 = Multiply(x=w3122, y=w3100) -> (x*y=w3121:dbl)
                n1761 = To Double Precision Float(number=w3093) -> (double precision float=w3099:dbl)
                n1762 = Build Array(w3099, w3098, w3098, w3098, w3098) -> (w3096:dbl[])
                n1763 = local read "N sets should be saved"() -> (w3102:dbl)
                n1764 = Build Array(w3115, w3110, w3108, w3106, w3104) -> (w3112:dbl[])
                n1765 = Build Array(w3095, w3100, w3121, w3120, w3119, 2.0 ("t")) -> (w3114:dbl[])
                n1766 = Round Toward +Infinity(x=w3102) -> (ceil(x): smallest int >= x=w3103:dbl)
                n1767 = Build Array (concatenate)(w3114, w3113, w3096, w3112) -> (w3111:dbl[])
                n1768 = To Unsigned Long Integer(number=w3103) -> (unsigned 32bit integer=w3101:u32)
              }
              frame 8 {
                w3131 = 0.0 ("f")
                # "MCL raster scan"
                n1769 = local read "Number of scans (MCL)"() -> (w3126:u64)
                n1770 = local read "Scan lines (y)"() -> (w3125:u64)
                n1771 = local read "2D or 1D Scan"() -> (w3128:bool)
                n1772 = local read "Scan Range (V)\n(of steps)"() -> (w3147:dbl)
                n1773 = local read "Fast Scan Dir"() -> (w3154:bool)
                n1774 = local read "Cycles/step (MCL)"() -> (w3144:u64)
                n1775 = local read "Scan steps (MCL)"() -> (w3146:u64)
                n1776 = Select(t=w3125, s=w3128, f=w3126) -> (s? t:f=w3127:u64)
                n1777 = Boolean To (0,1)(Boolean=w3128) -> (0, 1=w3130:i16)
                n1778 = local read "Save ave N"() -> (w3159:dbl)
                n1779 = local read "Initial X"() -> (w3133:dbl)
                n1780 = local read "Initial Y"() -> (w3132:dbl)
                n1781 = To Double Precision Float(number=w3130) -> (double precision float=w3129:dbl)
                n1782 = Boolean To (0,1)(Boolean=w3154) -> (0, 1=w3153:i16)
                n1783 = To Double Precision Float(number=w3127) -> (double precision float=w3142:dbl)
                n1784 = To Double Precision Float(number=w3146) -> (double precision float=w3145:dbl)
                n1785 = To Double Precision Float(number=w3144) -> (double precision float=w3143:dbl)
                n1786 = To Double Precision Float(number=w3153) -> (double precision float=w3152:dbl)
                n1787 = Multiply(x=w3159, y=w3138) -> (x*y=w3158:dbl)
                n1788 = To Double Precision Float(number=w3123) -> (double precision float=w3137:dbl)
                n1789 = local read "N sets should be saved (MCL)"() -> (w3140:dbl)
                n1790 = Build Array(w3137, w3129, w3131, w3131, w3131) -> (w3135:dbl[])
                n1791 = Build Array(w3152, w3147, w3145, w3143, w3142, w3133, w3132) -> (w3149:dbl[])
                n1792 = Build Array(w3134, w3138, w3158, w3157, w3156, 3.0 ("t")) -> (w3151:dbl[])
                n1793 = Round Toward +Infinity(x=w3140) -> (ceil(x): smallest int >= x=w3141:dbl)
                n1794 = Build Array (concatenate)(w3151, w3150, w3135, w3149) -> (w3148:dbl[])
                n1795 = To Unsigned Long Integer(number=w3141) -> (unsigned 32bit integer=w3139:u32)
              }
            }
            n1796 = local read "Index"() -> (w2998:dbl)
            n1797 = call "Create new save file.vi"("Insert"="", "Ext"=".dat", "Index In"=w2998) -> ("Path Out"=w2957:path, "Index Out"=w2970:dbl)
            n1798 = local write "Save file name"(w2957) -> ()
            n1799 = local write "Index"(w2970) -> ()
            n1800 = local write "Save index"(w2970) -> ()
            n1801 = Array Size(array=w2981) -> (size(s)=w2982:i32)
            n1802 = Open/Create/Replace File(file path (use dialog)=w2957, operation (0:open)=T22."create", access (0:read/write)=enum16{"read/write", "read-only", "write-only"}."write-only") -> (refnum out=w2995:refnum<file>)  [unwired: 1 in, 4 out]
            n1803 = local write "Saving..."(TRUE ("Saving...")) -> ()
            n1804 = To Double Precision Float(number=w2982) -> (double precision float=w2980:dbl)
            n1805 = String Length(string="Comment (data description)") -> (length=w2978:i32)
            n1806 = To Double Precision Float(number=w2978) -> (double precision float=w2977:dbl)
            n1807 = Deny Access(7:w2995) -> (3:w2994:refnum<file>)  [unwired: 1 in, 2 out]
            n1808 = Build Array (concatenate)(w2980, w2981, w2977) -> (w2979:dbl[])
            n1809 = case "If fluorescence data to be saved" shown="True" w2968 {
              tunnel: w2957 -> [_ w3047]
              tunnel: [refnum<k0> refnum w3027] -> w2969
              frame False {
              }
              frame True {
                w3026 = 0.0
                n1810 = local read "APD Integration Time (s)"() -> (w3032:dbl)
                n1811 = local read "N APD Samp/step"() -> (w3025:dbl)
                n1812 = Path To String(path=w3047) -> (string=w3046:string)
                n1813 = String Length(string=w3046) -> (length=w3045:i32)
                n1814 = Subtract(x=w3045, y=4) -> (x-y=w3043:i32)
                n1815 = String Subset(string=w3046, length (rest)=w3043) -> (substring=w3042:string)  [unwired: 1 out]
                n1816 = Build Array(w3032, w3025, w3026, w3026, w3026, w3026, w3026, w3026) -> (w3029:dbl[])
                n1817 = Concatenate Strings(w3042, "_fl.dat" ("string")) -> (w3040:string)
                n1818 = Array Size(array=w3029) -> (size(s)=w3031:i32)
                n1819 = String To Path(string=w3040) -> (path=w3036:path)
                n1820 = Open/Create/Replace File(file path (use dialog)=w3036, operation (0:open)=T22."create", access (0:read/write)=enum16{"read/write", "read-only", "write-only"}."write-only") -> (refnum out=w3037:refnum<file>)  [unwired: 1 in, 4 out]
                n1821 = Deny Access(7:w3037) -> (3:w3033:refnum<file>)  [unwired: 1 in, 2 out]
                n1822 = To Double Precision Float(number=w3031) -> (double precision float=w3030:dbl)
                n1823 = Build Array (concatenate)(w3030, w3029) -> (w3028:dbl[])
                n1824 = Write to Binary File(file (use dialog)=w3033, data=w3028, 5:FALSE ("prepend array or string size? (T)"), 9:T29."big-endian, network order" ("byte order (0:big-endian, network order)")) -> (refnum out=w3027:refnum<file>)  [unwired: 1 in, 3 out]
              }
            }
            n1825 = case shown="True" w2955 {
              tunnel: w2957 -> [_ w3009]
              tunnel: [refnum<k0> refnum w3008] -> w2956
              frame False {
              }
              frame True {
                w3004 = 0.0 ("element")
                n1826 = Path To String(path=w3009) -> (string=w3023:string)
                n1827 = Build Array(w3004, w3004, w3004, w3004, w3004, w3004, w3004, w3004) -> (w3005:dbl[])
                n1828 = String Length(string=w3023) -> (length=w3022:i32)
                n1829 = Subtract(x=w3022, y=4) -> (x-y=w3020:i32)
                n1830 = Array Size(array=w3005) -> (size(s)=w3007:i32)
                n1831 = String Subset(string=w3023, length (rest)=w3020) -> (substring=w3019:string)  [unwired: 1 out]
                n1832 = To Double Precision Float(number=w3007) -> (double precision float=w3006:dbl)
                n1833 = Concatenate Strings(w3019, "_pos.dat" ("string")) -> (w3017:string)
                n1834 = Build Array (concatenate)(w3006, w3005) -> (w3003:dbl[])
                n1835 = String To Path(string=w3017) -> (path=w3013:path)
                n1836 = Open/Create/Replace File(file path (use dialog)=w3013, operation (0:open)=T22."create", access (0:read/write)=enum16{"read/write", "read-only", "write-only"}."write-only") -> (refnum out=w3014:refnum<file>)  [unwired: 1 in, 4 out]
                n1837 = Deny Access(7:w3014) -> (3:w3010:refnum<file>)  [unwired: 1 in, 2 out]
                n1838 = Write to Binary File(file (use dialog)=w3010, data=w3003, 5:FALSE ("prepend array or string size? (T)"), 9:T29."big-endian, network order" ("byte order (0:big-endian, network order)")) -> (refnum out=w3008:refnum<file>)  [unwired: 1 in, 3 out]
              }
            }
            n1839 = Write to Binary File(file (use dialog)=w2994, data=w2979, 5:w2975, 9:w2973) -> (refnum out=w2976:refnum<file>)  [unwired: 1 in, 3 out]
            n1840 = Write to Binary File(file (use dialog)=w2976, data="Comment (data description)", 5:w2975, 9:w2973) -> (refnum out=w2972:refnum<file>)  [unwired: 1 in, 3 out]
          }
        }
        n1841 = feedback-in #19(w2915) -> ()
        n1842 = feedback-in #20(w2942) -> ()
        n1843 = feedback-in #21(w2914) -> ()
        n1844 = feedback-in #22(w2925) -> ()
        n1845 = feedback-in #23(w2928) -> ()
        n1846 = feedback-in #24(w2941) -> ()
        n1847 = feedback-in #25(w2931) -> ()
      }
      frame #1 {
        n1848 = local read "Saving..."() -> (w3172:bool)
        n1849 = case shown="True" w3172 {
          tunnel: w3176 -> [_ w3186]
          tunnel: w3175 -> [_ w3200]
          tunnel: w3174 -> [_ w3196]
          tunnel: w3173 -> [_ w3195]
          tunnel: w3171 -> [_ w3194]
          tunnel: w3170 -> [_ w3189]
          tunnel: w3169 -> [_ w3188]
          tunnel: w3168 -> [_ w3187]
          tunnel: w3167 -> [_ w3185]
          tunnel: w3166 -> [_ w3183]
          tunnel: w3165 -> [_ w3182]
          tunnel: w3164 -> [_ w3181]
          tunnel: w3163 -> [_ w3180]
          tunnel: w3162 -> [_ w3179]
          tunnel: w3161 -> [_ w3178]
          tunnel: w3160 -> [_ w3177]
          frame False {
          }
          frame True {
            n1850 = Multiply(x=w3186, y=w3185) -> (x*y=→"Time (s)":dbl)
            n1851 = Less Or Equal?(x=w3186, y=w3194) -> (x <= y?=w3198:bool)
            n1852 = Or(x="Stop Saving", y="Abort save 2") -> (x .or. y?=w3190:bool)
            n1853 = Not(x=w3190) -> (.not. x?=w3199:bool)
            n1854 = And(x=w3198, y=w3199) -> (x .and. y?=w3197:bool)
            n1855 = case shown="False" w3197 {
              tunnel: w3200 -> [w3207 w3275]
              tunnel: [0.0 w3278] -> w3193
              tunnel: w3186 -> [_ w3276]
              tunnel: w3194 -> [_ w3277]
              tunnel: w3196 -> [_ w3272]
              tunnel: w3195 -> [_ _]
              tunnel: w3189 -> [w3205 w3265]
              tunnel: w3188 -> [w3204 w3266]
              tunnel: w3187 -> [_ w3264]
              tunnel: w3183 -> [_ w3263]
              tunnel: w3182 -> [_ w3217]
              tunnel: w3181 -> [_ w3256]
              tunnel: w3180 -> [_ w3234]
              tunnel: w3179 -> [w3202 w3215]
              tunnel: w3178 -> [w3203 w3214]
              tunnel: w3177 -> [_ w3211]
              frame False {
                w3201 = FALSE
                n1856 = Close File(refnum=w3207) -> ()  [unwired: 1 in, 2 out]
                n1857 = case shown="True" w3204 {
                  tunnel: w3205 -> [_ w3209]
                  frame False {
                  }
                  frame True {
                    n1858 = Close File(refnum=w3209) -> ()  [unwired: 1 in, 2 out]
                  }
                }
                n1859 = case shown="True" w3202 {
                  tunnel: w3203 -> [_ w3208]
                  frame False {
                  }
                  frame True {
                    n1860 = Close File(refnum=w3208) -> ()  [unwired: 1 in, 2 out]
                  }
                }
                n1861 = local write "Calibrating Trap..."(w3201) -> ()
                n1862 = call <vilib>:"Beep.vi"() -> ()  [unwired: 3 in, 9 out]
                n1863 = local write "Stop Saving"(w3201) -> ()
                n1864 = property on="Raster Scanning..." class="Bool (strict)"("Val(Sgnl)"=w3201) -> ()  [unwired: 2 in, 2 out]
                "Saving..." <- w3201
              }
              frame True {
                n1865 = local read "Calibrating Trap..."() -> (w3267:bool)
                n1866 = case "Write fl. data" shown="True" w3266 {
                  tunnel: w3265 -> [_ w3301]
                  tunnel: w3264 -> [_ w3300]
                  frame False {
                  }
                  frame True {
                    n1867 = Write to Binary File(file (use dialog)=w3301, data=w3300, 5:FALSE ("prepend array or string size? (T)"), 9:T29."big-endian, network order" ("byte order (0:big-endian, network order)")) -> ()  [unwired: 1 in, 4 out]
                  }
                }
                n1868 = Greater?(x="Save ave N", y=1.0) -> (0:w3270:bool)
                n1869 = Not(x=w3267) -> (.not. x?=w3269:bool)
                n1870 = And(x=w3269, y=w3270) -> (x .and. y?=w3212:bool)
                n1871 = case shown="True" w3212 {
                  tunnel: w3211 -> [w3281 w3292]
                  tunnel: [w3281 w3284] -> w3210
                  tunnel: "Save ave N" -> [_ w3285]
                  frame False {
                  }
                  frame True {
                    w3282 = 2 ("dimension size")
                    n1872 = Array Size(array=w3292) -> (size(s)=w3286:i32)
                    n1873 = Divide(x=w3286, y=w3282) -> (x/y=w3290:dbl)
                    n1874 = Reshape Array(w3292, w3290, w3282) -> (w3291:u64[][])
                    n1875 = Transpose 2D Array(2D array=w3291) -> (transposed array=w3289:u64[][])
                    n1876 = for {
                      tunnel: w3289 -> [w3294] mode=indexing
                      tunnel: [w3293] -> w3283 mode=indexing
                      tunnel: w3285 -> [w3295]
                      workers-P: _ -> [_]
                      n1877 = call "downsample 1D array - U64.vi"("Ave N"=w3295, "Array In"=w3294) -> ("Array Out"=w3293:u64[])  [unwired: 1 in]
                    }
                    n1878 = Transpose 2D Array(2D array=w3283) -> (transposed array=w3288:u64[][])
                    n1879 = Divide(x=w3286, y=w3285) -> (x/y=w3287:dbl)
                    n1880 = Reshape Array(w3288, w3287) -> (w3284:u64[])
                  }
                }
                n1881 = case shown="True" w3212 {
                  tunnel: w3272 -> [w3304 w3316]
                  tunnel: [w3304 w3308] -> w3268
                  tunnel: "Save ave N" -> [_ w3309]
                  tunnel: w3263 -> [_ w3307]
                  frame False {
                    # "don't downsample data for trap calibration"
                  }
                  frame True {
                    n1882 = Array Size(array=w3316) -> (size(s)=w3310:i32)
                    n1883 = Array Size(array=w3307) -> (size(s)=w3306:i32)
                    n1884 = Divide(x=w3310, y=w3306) -> (x/y=w3314:dbl)
                    n1885 = Reshape Array(w3316, w3314, w3306) -> (w3315:i16[][])
                    n1886 = Transpose 2D Array(2D array=w3315) -> (transposed array=w3313:i16[][])
                    n1887 = for {
                      tunnel: w3313 -> [w3319] mode=indexing
                      tunnel: [w3318] -> w3305 mode=indexing
                      tunnel: w3309 -> [w3317]
                      workers-P: _ -> [_]
                      n1888 = call "downsample 1D array - I16.vi"("Ave N"=w3317, "Array In"=w3319) -> ("Array Out"=w3318:i16[])  [unwired: 1 out]
                    }
                    n1889 = Transpose 2D Array(2D array=w3305) -> (transposed array=w3312:i16[][])
                    n1890 = Divide(x=w3310, y=w3309) -> (x/y=w3311:dbl)
                    n1891 = Reshape Array(w3312, w3311) -> (w3308:i16[])
                  }
                }
                n1892 = Index Array(array=w3234, index=1) -> (element=w3237:waveform(dbl))
                n1893 = Index Array(array=w3234, index=0) -> (element=w3239:waveform(dbl))
                n1894 = Unbundle By Name(w3237) -> ("Y"=w3241:dbl[])
                n1895 = Unbundle By Name(w3239) -> ("Y"=w3249:dbl[])
                n1896 = case "Write trap pos. data" shown="True" w3215 {
                  tunnel: w3214 -> [_ w3297]
                  tunnel: w3210 -> [_ w3296]
                  frame False {
                  }
                  frame True {
                    n1897 = Write to Binary File(file (use dialog)=w3297, data=w3296, 5:FALSE ("prepend array or string size? (T)"), 9:T29."big-endian, network order" ("byte order (0:big-endian, network order)")) -> ()  [unwired: 1 in, 4 out]
                  }
                }
                n1898 = Write to Binary File(file (use dialog)=w3275, data=w3268, 5:FALSE ("prepend array or string size? (T)"), 9:T29."big-endian, network order" ("byte order (0:big-endian, network order)")) -> ()  [unwired: 1 in, 4 out]
                n1899 = feedback #26(w3241) -> (w3243:dbl[])
                n1900 = Build Array (concatenate)(w3243, w3241) -> (w3242:dbl[])
                n1901 = Select(t=w3241, s=w3217, f=w3242) -> (s? t:f=w3227:dbl[])
                n1902 = feedback-in #26(w3227) -> ()
                n1903 = feedback #27(w3249) -> (w3262:dbl[])
                n1904 = Build Array (concatenate)(w3262, w3249) -> (w3261:dbl[])
                n1905 = Select(t=w3249, s=w3217, f=w3261) -> (s? t:f=w3236:dbl[])
                n1906 = feedback-in #27(w3236) -> ()
                n1907 = Divide(x=w3276, y=w3277) -> (x/y=w3279:dbl)
                n1908 = Multiply(x=w3279, y=100.0) -> (x*y=w3278:dbl)
                n1909 = Build Array(w3236, w3227) -> (→"Saved APD":dbl[][])
                n1910 = Array Size(array=w3236) -> (size(s)=w3254:i32)
                n1911 = Unbundle By Name(w3256) -> ("Y"=w3260:dbl[])
                n1912 = Subtract(x=w3254, y="N pts to average") -> (x-y=w3230:i32)
                n1913 = Multiply(x="N pts to average", y=u16 2) -> (x*y=w3231:u16)
                n1914 = Subtract(x=w3254, y=w3231) -> (x-y=w3229:i32)
                n1915 = feedback #28(w3260) -> (w3259:dbl[])
                n1916 = Build Array (concatenate)(w3259, w3260) -> (w3258:dbl[])
                n1917 = Select(t=w3260, s=w3217, f=w3258) -> (s? t:f=w3257:dbl[])
                "Trap Delta Graph" <- w3257
                n1918 = feedback-in #28(w3257) -> ()
                n1919 = Array Subset(array=w3236, index=w3230, length="N pts to average") -> (w3253:dbl[])
                n1920 = Array Subset(array=w3236, index=w3229, length="N pts to average") -> (w3252:dbl[])
                n1921 = Array Subset(array=w3227, index=w3230, length="N pts to average") -> (w3233:dbl[])
                n1922 = Array Subset(array=w3227, index=w3229, length="N pts to average") -> (w3232:dbl[])
                n1923 = call-poly <vilib>:"Mean.vi"("X"=w3253) -> ("mean"=w3251:dbl)  [unwired: 1 out]
                n1924 = call-poly <vilib>:"Mean.vi"("X"=w3233) -> ("mean"=w3226:dbl)  [unwired: 1 out]
                n1925 = call-poly <vilib>:"Mean.vi"("X"=w3252) -> ("mean"=w3250:dbl)  [unwired: 1 out]
                n1926 = call-poly <vilib>:"Mean.vi"("X"=w3232) -> ("mean"=w3225:dbl)  [unwired: 1 out]
                n1927 = Subtract(x=w3226, y=w3225) -> (x-y=w3216:dbl)
                "Delta Fl. 2" <- w3216
                n1928 = Subtract(x=w3251, y=w3250) -> (x-y=w3248:dbl)
                "Delta Fl. 1" <- w3248
                n1929 = Initialize Array(w3248, 1 ("dimension size")) -> (w3245:dbl[])
                n1930 = Initialize Array(w3216, 1 ("dimension size")) -> (w3222:dbl[])
                n1931 = feedback #29(w3245) -> (w3246:dbl[])
                n1932 = Build Array (concatenate)(w3246, w3245) -> (w3244:dbl[])
                n1933 = feedback #30(w3222) -> (w3223:dbl[])
                n1934 = Build Array (concatenate)(w3223, w3222) -> (w3221:dbl[])
                n1935 = Select(t=w3245, s=w3217, f=w3244) -> (s? t:f=w3220:dbl[])
                n1936 = feedback-in #29(w3220) -> ()
                n1937 = Select(t=w3222, s=w3217, f=w3221) -> (s? t:f=w3219:dbl[])
                n1938 = feedback-in #30(w3219) -> ()
                n1939 = Build Array(w3220, w3219) -> (→"Save APD Deriv":dbl[][])
              }
            }
            "Progress" <- w3193
            "Progress 2" <- w3193
          }
        }
      }
    }
    n1940 = Bundle By Name(cluster=w1937, "Green FB Ch 0"=w1936, "Green FB Ch 1"=w1935) -> (w1915:T46)
    "Green FB Signals (V)" <- w1915
    n1941 = Unbundle By Name(w1915) -> ("Green FB Ch 2"=→"Green FB Plot":dbl)
    n1942 = local read "wait to reset values"() -> (w2007:bool)
    n1943 = Not(x=w2004) -> (.not. x?=w2008:bool)
    n1944 = And(x=w2008, y=w2007) -> (x .and. y?=w2009:bool)
    n1945 = case "Part of MCL raster scanning: returns to initial positions after scan done" shown="True" w2009 {
      tunnel: w2012 -> [w2745 w2752]
      tunnel: [w2745 w2751] -> w2011
      tunnel: w2006 -> [w2744 w2750]
      tunnel: [w2744 w2749] -> w2005
      frame False {
      }
      frame True {
        w2760 = 10.0 ("y")
        w2759 = 32767.0 ("y")
        # "to return scan values\nafter a synchronous \nAOM scan"
        n1946 = local read "AO2"() -> (w2753:dbl)
        n1947 = local read "AO1"() -> (w2754:dbl)
        n1948 = local write "wait to reset values"(FALSE ("wait to reset values")) -> ()
        n1949 = Multiply(x=w2754, y=w2759) -> (x*y=w2756:dbl)
        n1950 = Multiply(x=w2753, y=w2759) -> (x*y=w2758:dbl)
        n1951 = Divide(x=w2756, y=w2760) -> (x/y=w2755:dbl)
        n1952 = Divide(x=w2758, y=w2760) -> (x/y=w2757:dbl)
        n1953 = To Word Integer(number=w2755) -> (16bit integer=w2761:i16)
        n1954 = To Word Integer(number=w2757) -> (16bit integer=w2762:i16)
        n1955 = local read "Total Counts (ticks)"() -> (w2746:u32)
        n1956 = xnode "Read/Write Control"("FPGA VI Reference In"=w2752, "error in"=w2750, "AO1"=w2761, "AO2"=w2762, "MCL count"=w2746) -> ("FPGA VI Reference Out"=w2751:T19, "error out"=w2749:errorcluster)
        n1957 = local read "Scan Range (V)\n(of steps)"() -> (w2747:dbl)
        n1958 = property on="Scan Range (V)\n(of steps)" class="DigNum (strict)"("Val(Sgnl)"=w2747) -> ()  [unwired: 2 in, 2 out]
      }
    }
    n1959 = node-c288() -> ()  [unwired: 2 out]
  }
  n1960 = node-c288(3 ("Processor")) -> (w74:T23)  [unwired: 3 out]
  n1961 = timed-loop "Mouse control: trap position (AOM deflection), set confocal spot from image" {
    tunnel: [w3321] -> w34
    tunnel: w24 -> [w3320]
    timing: w76 -> [_]
    timing-out: [_] -> w75
    stop <- w3321 stop-if-true
    n1962 = node-c288() -> ()  [unwired: 2 out]
    n1963 = event shown="[0] \"Pane\": Mouse Down" {
      selector: _ -> [_ _]
      dyn-events: _ -> [_ _]
      timeout: _ -> [_ _]
      tunnel: w3320 -> [w3324 _]
      event Mouse Down {
        n1964 = event-data() -> ("Time"=w3326:u32, "Coords"=w3325:T7, "Button"=w3327:u16)  [unwired: 6 out]
        n1965 = case shown="1" w3327 {
          tunnel: w3326 -> [_ _ w3430]
          tunnel: w3325 -> [_ w3364 w3428]
          tunnel: w3324 -> [_ _ w3426]
          frame 0, Default {
          }
          frame 1 {
            n1966 = property on="APD 2" class="ImageControl"() -> ("Displayed Image Position"=w3334:cluster{"Left":i32, "Top":i32})  [unwired: 2 in, 2 out]
            n1967 = property on="APD 1" class="ImageControl"() -> ("Displayed Image Position"=w3363:cluster{"Left":i32, "Top":i32})  [unwired: 2 in, 2 out]
            n1968 = property on="Detection Laser X" class="ImageControl"() -> ("Displayed Image Position"=w3360:cluster{"Left":i32, "Top":i32})  [unwired: 2 in, 2 out]
            n1969 = property on="Detection Laser Y" class="ImageControl"() -> ("Displayed Image Position"=w3359:cluster{"Left":i32, "Top":i32})  [unwired: 2 in, 2 out]
            n1970 = property on="APD 2" class="ImageControl"() -> ("Displayed Image Size"=w3333:cluster{"Width":u32, "Height":u32})  [unwired: 2 in, 2 out]
            n1971 = property on="APD 1" class="ImageControl"() -> ("Displayed Image Size"=w3361:cluster{"Width":u32, "Height":u32})  [unwired: 2 in, 2 out]
            n1972 = property on="Detection Laser X" class="ImageControl"() -> ("Displayed Image Size"=w3362:cluster{"Width":u32, "Height":u32})  [unwired: 2 in, 2 out]
            n1973 = property on="Detection Laser Y" class="ImageControl"() -> ("Displayed Image Size"=w3358:cluster{"Width":u32, "Height":u32})  [unwired: 2 in, 2 out]
            n1974 = Unbundle By Name(w3333) -> ("Width"=w3330:u32, "Height"=w3329:u32)
            n1975 = Unbundle By Name(w3334) -> ("Left"=w3332:i32, "Top"=w3331:i32)
            n1976 = Unbundle By Name(w3361) -> ("Width"=w3355:u32, "Height"=w3354:u32)
            n1977 = Unbundle By Name(w3362) -> ("Width"=w3351:u32, "Height"=w3350:u32)
            n1978 = Unbundle By Name(w3358) -> ("Width"=w3347:u32, "Height"=w3346:u32)
            n1979 = Unbundle By Name(w3363) -> ("Left"=w3357:i32, "Top"=w3356:i32)
            n1980 = Unbundle By Name(w3360) -> ("Left"=w3353:i32, "Top"=w3352:i32)
            n1981 = Unbundle By Name(w3359) -> ("Left"=w3349:i32, "Top"=w3348:i32)
            n1982 = Bundle("Left"=w3332, "Top"=w3331, "Width"=w3330, "Height"=w3329) -> (w3328:T47)  [unwired: 1 in]
            n1983 = Bundle("Left"=w3357, "Top"=w3356, "Width"=w3355, "Height"=w3354) -> (w3345:T47)  [unwired: 1 in]
            n1984 = Bundle("Left"=w3353, "Top"=w3352, "Width"=w3351, "Height"=w3350) -> (w3344:T47)  [unwired: 1 in]
            n1985 = Bundle("Left"=w3349, "Top"=w3348, "Width"=w3347, "Height"=w3346) -> (w3343:T47)  [unwired: 1 in]
            n1986 = Build Cluster Array(w3328, w3345, w3344, w3343) -> (w3342:T48)
            n1987 = for {
              tunnel: w3364 -> [w3375]
              tunnel: w3342 -> [w3376] mode=indexing
              shift-right: [w3373] -> w3340
              shift-left: TRUE -> [w3374]
              shift-right: [w3372] -> w3338
              shift-left: _ -> [w3368]
              shift-right: [w3371] -> w3337
              shift-left: _ -> [w3367]
              shift-right: [w3370] -> w3336
              shift-left: _ -> [w3366]
              shift-right: [w3369] -> w3335
              shift-left: _ -> [w3365]
              n1988 = case shown="True" w3374 {
                selector: w3374 -> [w3381 _]
                tunnel: w3376 -> [_ w3390]
                tunnel: w3375 -> [_ w3388]
                tunnel: [w3381 w3386] -> w3373
                tunnel: [w3380 w3385] -> w3372
                tunnel: [w3379 w3384] -> w3371
                tunnel: [w3378 w3383] -> w3370
                tunnel: [w3377 w3382] -> w3369
                tunnel: w3368 -> [w3380 _]
                tunnel: w3367 -> [w3379 _]
                tunnel: w3366 -> [w3378 _]
                tunnel: w3365 -> [w3377 _]
                frame False {
                }
                frame True {
                  n1989 = Unbundle(w3390) -> (w3389:T47)
                  n1990 = call "isclickinwindow.vi"("Image Param"=w3389, "Point32"=w3388) -> ("4 Y"=w3382:i32, "3 Height"=w3383:i32, "2 X"=w3384:i32, "1 Width"=w3385:i32, "In image?"=w3387:bool)  [unwired: 1 in]
                  n1991 = Not(x=w3387) -> (.not. x?=w3386:bool)
                }
              }
            }
            n1992 = Not(x=w3340) -> (.not. x?=w3339:bool)
            n1993 = case shown="True" w3339 {
              tunnel: w3337 -> [_ w3403]
              tunnel: w3335 -> [_ w3402]
              tunnel: w3338 -> [_ w3401]
              tunnel: w3336 -> [_ w3400]
              frame False {
              }
              frame True {
                w3396 = FALSE ("Get Point")
                n1994 = local read "Scan lines (y)"() -> (w3405:u64)
                n1995 = local read "Actual MCL Inc (V)"() -> (w3397:dbl)
                n1996 = local read "Scan steps (MCL)"() -> (w3404:u64)
                n1997 = Divide "Y Pix/step"(x=w3400, y=w3405) -> (x/y=w3412:dbl)
                n1998 = Divide "Y V/pix"(x=w3397, y=w3412) -> (x/y=w3411:dbl)
                n1999 = Divide "Y half step offset"(x=w3397, y=2.0) -> (x/y=w3413:dbl)
                n2000 = Divide "X pix/step"(x=w3401, y=w3404) -> (x/y=w3410:dbl)
                n2001 = Negate(x=w3413) -> (-x=w3414:dbl)
                n2002 = local read "Initial Y"() -> (w3420:dbl)
                n2003 = Multiply(x=w3402, y=w3411) -> (x*y=w3421:dbl)
                n2004 = Divide "X half step offset"(x=w3397, y=2.0) -> (x/y=w3407:dbl)
                n2005 = Divide "X V/pix"(x=w3397, y=w3410) -> (x/y=w3409:dbl)
                n2006 = Multiply(x=w3397, y=w3404) -> (x*y=w3416:dbl)
                n2007 = Compound Arithmetic op=ADD(w3414, w3421, w3420) -> (w3398:dbl)
                "Pointer Y (V)" <- w3398
                n2008 = Multiply(x=w3409, y=w3403) -> (x*y=w3418:dbl)
                n2009 = Negate(x=w3407) -> (-x=w3406:dbl)
                n2010 = local read "Initial X"() -> (w3419:dbl)
                n2011 = Negate(x=w3418) -> (-x=w3417:dbl)
                n2012 = Compound Arithmetic op=ADD(w3406, w3416, w3419, w3417) -> (w3399:dbl)
                "Pointer X (V)" <- w3399
                n2013 = Or(x="Set X Only", y="Set Confocal Spot (X-Y)") -> (x .or. y?=w3392:bool)
                n2014 = Or(x="Set Confocal Spot (X-Y)", y="Set Y Only") -> (x .or. y?=w3391:bool)
                n2015 = case shown="True" w3392 {
                  tunnel: w3399 -> [_ w3422]
                  frame False {
                  }
                  frame True {
                    n2016 = property on="AO2" class="Slide (strict)"("Val(Sgnl)"=w3422) -> ()  [unwired: 2 in, 2 out]
                  }
                }
                n2017 = case shown="True" w3391 {
                  tunnel: w3398 -> [_ w3423]
                  frame False {
                  }
                  frame True {
                    n2018 = property on="AO1" class="Slide (strict)"("Val(Sgnl)"=w3423) -> ()  [unwired: 2 in, 2 out]
                  }
                }
                n2019 = local write "Set Confocal Spot (X-Y)"(w3396) -> ()
                n2020 = local write "Set X Only"(w3396) -> ()
                n2021 = local write "Set Y Only"(w3396) -> ()
              }
            }
          }
          frame 3 {
            n2022 = local read "BD 2 Frequency 1 (MHz)"() -> (w3424:dbl)
            n2023 = local read "BD 1 Frequency 1 (MHz)"() -> (w3425:dbl)
            n2024 = local write "Manipulating Trap"(TRUE ("Manipulating Trap")) -> ()
            n2025 = local write "Coords"(T7 {"Horizontal"=0, "Vertical"=0} ("Coords")) -> ()
            n2026 = while {
              tunnel: w3430 -> [w3435]
              tunnel: w3428 -> [w3434]
              tunnel: w3426 -> [w3433]
              tunnel: w3425 -> [w3432]
              tunnel: w3424 -> [w3431]
              stop <- w3436 stop-if-true
              n2027 = event shown="[0] \"Pane\": Mouse Move" {
                selector: _ -> [_ _]
                dyn-events: _ -> [_ _]
                timeout: _ -> [_ _]
                tunnel: ["Force Manip Abort" w3500] -> w3436
                tunnel: w3435 -> [w3443 _]
                tunnel: w3434 -> [w3441 _]
                tunnel: w3433 -> [w3440 _]
                tunnel: w3432 -> [w3439 _]
                tunnel: w3431 -> [w3438 _]
                event Mouse Move {
                  n2028 = event-data() -> ("Time"=w3444:u32, "Coords"=w3445:T7)  [unwired: 3 out]
                  n2029 = Less?(x=w3444, y=w3443) -> (x < y?=w3442:bool)
                  n2030 = case "Makes sure old motion events prior to mouse click aren't used" shown="False" w3442 {
                    tunnel: w3445 -> [w3487 _]
                    tunnel: w3441 -> [w3488 _]
                    tunnel: w3440 -> [w3465 _]
                    tunnel: w3439 -> [w3461 _]
                    tunnel: w3438 -> [w3460 _]
                    frame False {
                      n2031 = Subtract(x=w3487, y=w3488) -> (x-y=w3486:T7)
                      "Coords" <- w3486
                      n2032 = local read "Y RF Frequency Limits (MHz)"() -> (w3446:T16)
                      n2033 = To Double Precision Float(number=w3486) -> (double precision float=w3485:cluster{"Horizontal":dbl, "Vertical":dbl})
                      n2034 = Multiply(x=cluster{"Horizontal":dbl, "Vertical":dbl} {"Horizontal"=-1.0, "Vertical"=1.0}, y="Manipulation Scaling") -> (x*y=w3481:cluster{"Horizontal":dbl, "Vertical":dbl})
                      n2035 = local read "X RF Frequency Limits (MHz)"() -> (w3447:T16)
                      n2036 = Multiply(x=w3485, y=w3481) -> (x*y=w3483:cluster{"Horizontal":dbl, "Vertical":dbl})
                      n2037 = Unbundle By Name(w3483) -> ("Horizontal"=w3478:dbl, "Vertical"=w3482:dbl)
                      n2038 = Unbundle By Name(w3446) -> ("Maximum"=w3449:dbl, "Minimum"=w3448:dbl)
                      n2039 = Boolean To (0,1)(Boolean="Manip. X?") -> (0, 1=w3476:i16)
                      n2040 = Boolean To (0,1)(Boolean="Manip. Y?") -> (0, 1=w3473:i16)
                      n2041 = local read "BD 1 Frequency 2 (MHz)"() -> (w3463:dbl)
                      n2042 = Multiply(x=w3482, y=w3473) -> (x*y=w3475:dbl)
                      n2043 = Multiply(x=w3476, y=w3478) -> (x*y=w3479:dbl)
                      n2044 = local read "BD 2 Frequency 2 (MHz)"() -> (w3462:dbl)
                      n2045 = Unbundle By Name(w3447) -> ("Maximum"=w3451:dbl, "Minimum"=w3450:dbl)
                      n2046 = Add(x=w3460, y=w3475) -> (x+y=w3453:dbl)
                      n2047 = Add(x=w3461, y=w3479) -> (x+y=w3455:dbl)
                      n2048 = In Range and Coerce(upper limit=w3451, x=w3455, lower limit=w3450) -> (coerced(x)=w3454:dbl)  [unwired: 1 out]
                      n2049 = In Range and Coerce(upper limit=w3449, x=w3453, lower limit=w3448) -> (coerced(x)=w3452:dbl)  [unwired: 1 out]
                      n2050 = Subtract(x=w3454, y=w3463) -> (x-y=w3472:dbl)
                      n2051 = Subtract(x=w3452, y=w3462) -> (x-y=w3471:dbl)
                      n2052 = Square(x=w3472) -> (x^2=w3470:dbl)
                      n2053 = Square(x=w3471) -> (x^2=w3469:dbl)
                      n2054 = Add(x=w3470, y=w3469) -> (x+y=w3468:dbl)
                      n2055 = Square Root(x=w3468) -> (sqrt(x)=w3464:dbl)
                      n2056 = In Range and Coerce(upper limit="Limit Max (MHz)", x=w3464, lower limit="Limit Min (MHz)") -> (In Range?=w3457:bool)  [unwired: 1 out]
                      n2057 = Not(x="Limits Enable") -> (.not. x?=w3456:bool)
                      n2058 = Or(x=w3457, y=w3456) -> (x .or. y?=w3458:bool)
                      n2059 = case shown="True" w3458 {
                        tunnel: w3465 -> [_ w3498]
                        tunnel: w3464 -> [_ w3489]
                        tunnel: w3454 -> [_ w3496]
                        tunnel: w3463 -> [_ w3495]
                        tunnel: w3452 -> [_ w3494]
                        tunnel: w3462 -> [_ w3493]
                        tunnel: w3447 -> [_ w3491]
                        tunnel: w3446 -> [_ w3490]
                        frame False {
                        }
                        frame True {
                          n2060 = local read "BD 1 Frequency 3 (MHz)"() -> (w3497:dbl)
                          n2061 = local read "BD 2 Frequency 3 (MHz)"() -> (w3492:dbl)
                          n2062 = local write "Trap Delta (MHz)"(w3489) -> ()
                          n2063 = property on="Initial delta (MHz)" class="DigNum (strict)"("Val(Sgnl)"=w3489) -> ()  [unwired: 2 in, 2 out]
                          n2064 = call "set RF board frequency - interlace.vi"("Board 2 Frequency Limits"=w3490, "Board 1 Frequency Limits"=w3491, "FPGA VI Reference In"=w3498, "Board 2 Frequency 3 (MHz)"=w3492, "Board 1 Frequency 3 (MHz)"=w3497, "Board 2 Frequency 2 (MHz)"=w3493, "Board 2 Frequency 1 (MHz)"=w3494, "Board 1 Frequency 2 (MHz)"=w3495, "Board 1 Frequency 1  (MHz)"=w3496) -> ()  [unwired: 1 in, 2 out]
                          n2065 = local write "BD 2 Frequency 1 (MHz)"(w3494) -> ()
                          n2066 = local write "BD 1 Frequency 1 (MHz)"(w3496) -> ()
                        }
                      }
                    }
                    frame True {
                    }
                  }
                }
                event Mouse Up {
                  n2067 = event-data() -> ("Button"=w3499:u16)  [unwired: 8 out]
                  n2068 = case shown="3" w3499 {
                    tunnel: [FALSE TRUE] -> w3500
                    frame 0, Default {
                    }
                    frame 3 {
                      n2069 = local write "Manipulating Trap"(FALSE ("Manipulating Trap")) -> ()
                    }
                  }
                }
              }
            }
          }
        }
      }
      event Mouse Move {
        n2070 = event-data() -> ()  [unwired: 6 out]
      }
    }
    n2071 = local read "Stop All"() -> (w3321:bool)
    n2072 = node-c288() -> ()  [unwired: 2 out]
  }
  n2073 = timed-loop "Oscillate AOD (debugging)" {
    tunnel: w24 -> [w3505]
    tunnel: [w3504] -> w36
    timing: w74 -> [_]
    timing-out: [_] -> w73
    stop <- w3504 stop-if-true
    n2074 = node-c288() -> ()  [unwired: 2 out]
    n2075 = event shown="[0] \"Oscillate Set 2\", \"Fish for Tether\": Value Change" {
      selector: _ -> [_ _ _]
      dyn-events: _ -> [_ _ _]
      timeout: _ -> [_ _ _]
      tunnel: w3505 -> [w3512 _ _]
      tunnel: [FALSE ("Stop All") _ w3780] -> w3504
      event "Oscillate Set 2", "Fish for Tether": Value Change {
        n2076 = event-data() -> ()  [unwired: 6 out]
        n2077 = local read "Oscillate Set 2"() -> (w3511:bool)
        n2078 = Or(x=w3511, y="Fish for Tether") -> (x .or. y?=w3509:bool)
        n2079 = case shown="True" w3509 {
          tunnel: w3512 -> [_ w3515]
          tunnel: "Fish for Tether" -> [_ w3514]
          frame False {
          }
          frame True {
            n2080 = case shown="True" w3514 {
              frame False {
              }
              frame True {
                n2081 = local write "Scan axis 2"(TRUE) -> ()
                n2082 = local write "Tether"(FALSE ("Tether")) -> ()
              }
            }
            n2083 = node-c288("Period") -> (w3517:T23)  [unwired: 3 out]
            n2084 = timed-loop "Oscillate AOD" {
              timing: w3517 -> [_]
              timing-out: [_] -> w3516
              tunnel: w3515 -> [w3527]
              tunnel: w3514 -> [w3526]
              i -> [w3529]
              stop <- w3525 stop-if-true
              n2085 = node-c288() -> (w3528:i64)  [unwired: 1 out]
              n2086 = flat-sequence {
                tunnel: w3529 -> [w3555]
                tunnel: w3528 -> [w3554]
                tunnel: w3527 -> [w3538]
                tunnel: w3526 -> [w3540]
                tunnel: [w3540] -> w3524
                tunnel: [w3539] -> w3523
                tunnel: [w3537] -> w3522
                tunnel: [w3534] -> w3520
                tunnel: w3524 -> [w3591]
                tunnel: w3523 -> [w3589]
                tunnel: w3522 -> [w3588]
                tunnel: [w3587] -> w3521
                tunnel: w3520 -> [w3586]
                tunnel: [w3655] -> w3525
                tunnel: w3521 -> [w3653]
                frame #0 {
                  n2087 = Divide(x=w3554, y=i64 1000) -> (x/y=w3549:dbl)
                  n2088 = Multiply(x=w3549, y=w3555) -> (x*y=w3551:dbl)
                  n2089 = Multiply(x="Osc. freq. (Hz)", y=6.283185307179586) -> (x*y=w3552:dbl)
                  n2090 = Multiply(x=w3552, y=w3551) -> (x*y=w3536:dbl)
                  n2091 = local read "BD 1 Frequency 2 (MHz)"() -> (w3533:dbl)
                  n2092 = local read "BD 1 Frequency 1 (MHz)"() -> (w3530:dbl)
                  n2093 = case shown="True" w3540 {
                    tunnel: w3536 -> [w3561 w3568]
                    tunnel: w3533 -> [_ w3578]
                    tunnel: [w3558 w3562] -> w3541
                    tunnel: [FALSE w3571] -> w3537
                    tunnel: [0.0 w3564] -> w3534
                    tunnel: w3530 -> [_ w3563]
                    frame False {
                      n2094 = Sine(x=w3561) -> (sin(x)=w3559:dbl)
                      n2095 = Multiply(x=w3559, y="Osc. amp. (MHz)") -> (x*y=w3558:dbl)
                    }
                    frame True {
                      n2096 = Cosine(x=w3568) -> (cos(x)=w3581:dbl)
                      n2097 = Subtract(x=w3578, y=w3563) -> (x-y=w3577:dbl)
                      n2098 = Decrement(x=w3581) -> (x-1=w3580:dbl)
                      n2099 = Subtract(x=w3577, y="Closest Delta (MHz)") -> (x-y=w3574:dbl)
                      n2100 = Divide(x=w3580, y=2.0) -> (x/y=w3575:dbl)
                      n2101 = Multiply(x=w3575, y=w3574) -> (x*y=w3562:dbl)
                      n2102 = local read "Vec Mean of T1 T2"() -> (w3570:dbl[])
                      n2103 = Greater?(x=w3570, y="Stop F (pN)") -> (0:w3572:bool[])
                      n2104 = Or Array Elements(Boolean array=w3572) -> (logical OR=w3571:bool)
                      n2105 = Divide(x=w3568, y=6.283185307179586) -> (x/y=w3567:dbl)
                      n2106 = Round Toward +Infinity(x=w3567) -> (ceil(x): smallest int >= x=w3564:dbl)
                      "Attempts" <- w3564
                      n2107 = Greater?(x=w3564, y="Attempt Limit") -> (0:w3566:bool)
                      n2108 = case shown="True" w3566 {
                        frame False {
                        }
                        frame True {
                          n2109 = local write "Fish for Tether"(FALSE ("Fish for Tether")) -> ()
                          n2110 = call <vilib>:"Beep.vi"() -> ()  [unwired: 3 in, 9 out]
                          n2111 = local read "Messages"() -> (w3583:string)
                          n2112 = call "Update messages.vi"("Message to add"="Tether fishing timeout." ("Messages"), "Old message string"=w3583) -> ("New message string"=→"Messages":string)
                        }
                      }
                    }
                  }
                  n2113 = local read "Y RF Frequency Limits (MHz)"() -> (w3542:T16)
                  n2114 = local read "X RF Frequency Limits (MHz)"() -> (w3543:T16)
                  n2115 = local read "BD 1 Frequency 3 (MHz)"() -> (w3548:dbl)
                  n2116 = local read "BD 2 Frequency 2 (MHz)"() -> (w3532:dbl)
                  n2117 = Select(t=w3533, s="Scan axis 2", f=w3532) -> (s? t:f=w3544:dbl)
                  n2118 = Add(x=w3541, y=w3544) -> (x+y=w3539:dbl)
                  n2119 = Select(t=w3539, s="Scan axis 2", f=w3533) -> (s? t:f=w3531:dbl)
                  n2120 = Select(t=w3532, s="Scan axis 2", f=w3539) -> (s? t:f=w3546:dbl)
                  n2121 = local read "BD 2 Frequency 3 (MHz)"() -> (w3547:dbl)
                  n2122 = call "set RF board frequency - interlace.vi"("Board 2 Frequency Limits"=w3542, "Board 1 Frequency Limits"=w3543, "FPGA VI Reference In"=w3538, "Board 2 Frequency 3 (MHz)"=w3547, "Board 1 Frequency 3 (MHz)"=w3548, "Board 2 Frequency 2 (MHz)"=w3532, "Board 2 Frequency 1 (MHz)"=w3546, "Board 1 Frequency 2 (MHz)"=w3531, "Board 1 Frequency 1  (MHz)"=w3530) -> ()  [unwired: 1 in, 2 out]
                }
                frame #1 {
                  n2123 = And(x=w3591, y=w3588) -> (x .and. y?=w3590:bool)
                  n2124 = case "Only if were fishing and now formed tether" shown="True" w3590 {
                    tunnel: w3589 -> [w3593 w3605]
                    tunnel: [w3592 w3604] -> w3587
                    tunnel: w3586 -> [_ w3600]
                    frame False {
                      n2125 = local read "Fish for Tether"() -> (w3592:bool)
                      n2126 = case shown="True" w3592 {
                        tunnel: w3593 -> [_ _]
                        frame False {
                        }
                        frame True {
                        }
                      }
                    }
                    frame True {
                      w3604 = FALSE ("Fish for Tether")
                      n2127 = call <vilib>:"Beep.vi"() -> ()  [unwired: 3 in, 9 out]
                      n2128 = Number To Decimal String(number=w3600, width (-)=i16 1) -> (decimal integer string=w3598:string)
                      n2129 = case shown="\"2\", \"3\", \"4\", \"5\", \"6\"" "Then..." {
                        selector: "Then..." -> [_ w3608]
                        tunnel: w3605 -> [w3607 _]
                        frame "1", Default {
                          # "do nothing"
                          n2130 = property on="BD 1 Frequency 1 (MHz)" class="DigNum (strict)"("Val(Sgnl)"=w3607) -> ()  [unwired: 2 in, 2 out]
                        }
                        frame "2", "3", "4", "5", "6" {
                          n2131 = flat-sequence {
                            tunnel: w3608 -> [w3610]
                            frame #0 {
                              n2132 = property on="Trap Delta (MHz)" class="DigNum (strict)"("Val(Sgnl)"="Move to Delta 1 (MHz)") -> ()  [unwired: 2 in, 2 out]
                            }
                            frame #1 {
                              n2133 = case shown="\"5\", \"6\"" w3610 {
                                selector: w3610 -> [w3613 w3623 _]
                                frame "3", "4" {
                                n2134 = flat-sequence {
                                tunnel: w3613 -> [w3614]
                                tunnel: [w3614] -> w3611
                                tunnel: [w3616] -> w3612
                                tunnel: w3611 -> [w3616]
                                tunnel: w3612 -> [w3620]
                                frame #0 {
                                n2135 = property on="Green Laser ON/Interlacing" class="Bool (strict)"("Val(Sgnl)"=TRUE ("Value (Signaling)")) -> ()  [unwired: 2 in, 2 out]
                                }
                                frame #1 {
                                n2136 = Multiply(x="Wait Before Save (s)", y=u32 1000 ("x")) -> (x*y=w3618:u32)
                                n2137 = Wait (ms)(milliseconds to wait=w3618) -> ()  [unwired: 1 out]
                                }
                                frame #2 {
                                n2138 = property on="Start Saving" class="Bool (strict)"("Value"=TRUE ("Start Saving")) -> ()  [unwired: 2 in, 2 out]
                                n2139 = case shown="\"4\"" w3620 {
                                frame Default {
                                }
                                frame "4" {
                                n2140 = property on="Fl. Triggered..." class="Bool (strict)"("Val(Sgnl)"=TRUE ("Value (Signaling)")) -> ()  [unwired: 2 in, 2 out]
                                }
                                }
                                }
                                }
                                }
                                frame "5", "6" {
                                n2141 = stacked-sequence {
                                tunnel: w3623 -> [_ _ _ _ _ _ _ _ w3640 _ _]
                                frame #0 {
                                n2142 = Replace Array Subset(array=u32[] [0] ("Index Values"), new element="Raster Set Upon Tether", index=0) -> (w3624:u32[])
                                n2143 = property on="Saved AOD Raster Scan Parameter Sets" class="Arr (strict)"("Index Values"=w3624) -> ()  [unwired: 2 in, 2 out]
                                }
                                frame #1 {
                                n2144 = Wait (ms)(milliseconds to wait=u32 500) -> ()  [unwired: 1 out]
                                }
                                frame #2 {
                                n2145 = property on="Load parameters" class="Bool (strict)"("Val(Sgnl)"=TRUE ("Value (Signaling)")) -> ()  [unwired: 2 in, 2 out]
                                }
                                frame #3 {
                                n2146 = Wait (ms)(milliseconds to wait=u32 500) -> ()  [unwired: 1 out]
                                }
                                frame #4 {
                                n2147 = property on="Trap Raster Scan" class="Bool (strict)"("Val(Sgnl)"=TRUE ("Value (Signaling)")) -> ()  [unwired: 2 in, 2 out]
                                }
                                frame #5 {
                                n2148 = Wait (ms)(milliseconds to wait=u32 2000) -> ()  [unwired: 1 out]
                                }
                                frame #6 {
                                n2149 = while {
                                stop <- w3635 stop-if-true
                                n2150 = local read "Raster Scanning..."() -> (w3634:bool)
                                n2151 = local read "Saving..."() -> (w3637:bool)
                                n2152 = Wait (ms)(milliseconds to wait=u32 100) -> ()  [unwired: 1 out]
                                n2153 = Not(x=w3637) -> (.not. x?=w3636:bool)
                                n2154 = Not(x=w3634) -> (.not. x?=w3633:bool)
                                n2155 = And(x=w3636, y=w3633) -> (x .and. y?=w3635:bool)
                                }
                                }
                                frame #7 {
                                n2156 = property on="Trap Delta (MHz)" class="DigNum (strict)"("Val(Sgnl)"="Move to Delta 2 (MHz)") -> ()  [unwired: 2 in, 2 out]
                                }
                                frame #8 {
                                n2157 = local read "Tether"() -> (w3641:bool)
                                n2158 = case shown="True" w3641 {
                                tunnel: w3640 -> [_ w3642]
                                frame False {
                                }
                                frame True {
                                n2159 = flat-sequence {
                                tunnel: w3642 -> [w3644]
                                frame #0 {
                                n2160 = Wait (ms)(milliseconds to wait=u32 500) -> ()  [unwired: 1 out]
                                }
                                frame #1 {
                                n2161 = case shown="\"6\"" w3644 {
                                frame Default {
                                }
                                frame "6" {
                                n2162 = property on="Green Laser ON/Interlacing" class="Bool (strict)"("Val(Sgnl)"=TRUE ("Green Laser ON/Interlacing")) -> ()  [unwired: 2 in, 2 out]
                                }
                                }
                                }
                                frame #2 {
                                n2163 = Wait (ms)(milliseconds to wait=u32 500) -> ()  [unwired: 1 out]
                                }
                                frame #3 {
                                n2164 = local write "Start Saving"("Save at end (5, 6)") -> ()
                                }
                                }
                                }
                                }
                                }
                                frame #9 {
                                n2165 = local read "Bead Sep. Int. Time (s)"() -> (w3650:dbl)
                                n2166 = Multiply(x=w3650, y=1000.0) -> (x*y=w3649:dbl)
                                n2167 = Wait (ms)(milliseconds to wait=w3649) -> ()  [unwired: 1 out]
                                }
                                frame #10 {
                                n2168 = property on="Rescale on Mean" class="Bool (strict)"("Val(Sgnl)"=TRUE ("Value (Signaling)")) -> ()  [unwired: 2 in, 2 out]
                                }
                                }
                                }
                                frame "2", Default {
                                }
                              }
                            }
                          }
                        }
                      }
                      n2169 = Concatenate Strings("Formed tether in ", w3598, " attempt(s)." ("string")) -> (w3595:string)
                      n2170 = local read "Messages"() -> (w3602:string)
                      n2171 = local write "Fish for Tether"(w3604) -> ()
                      n2172 = call "Update messages.vi"("Message to add"=w3595, "Old message string"=w3602) -> ("New message string"=w3601:string)
                      n2173 = local write "Messages"(w3601) -> ()
                      n2174 = Get Date/Time In Seconds() -> (seconds since 1Jan1904=→"Time tether formed":timestamp)
                      "Tether" <- "Tether Alarm?"
                    }
                  }
                }
                frame #2 {
                  n2175 = local read "Oscillate Set 2"() -> (w3654:bool)
                  n2176 = local read "Stop All"() -> (w3656:bool)
                  n2177 = Not Or(1:w3653, 2:w3654) -> (0:w3652:bool)
                  n2178 = Compound Arithmetic op=OR(w3656, w3652) -> (w3655:bool)
                }
              }
              n2179 = node-c288() -> ()  [unwired: 2 out]
            }
            n2180 = node-c288(w3516) -> ()  [unwired: 1 out]
          }
        }
      }
      event "Fl. Triggered...": Value Change {
        n2181 = event-data() -> ()  [unwired: 7 out]
        n2182 = case shown="True" "Fl. Triggered..." {
          frame False {
          }
          frame True {
            n2183 = node-c288() -> (w3668:T23)  [unwired: 4 out]
            n2184 = timed-loop {
              timing: w3668 -> [_]
              timing-out: [_] -> w3667
              tunnel: "Action" -> [w3672]
              shift-right: [w3669] -> _
              shift-left: u8 255 -> [w3671]
              stop <- w3673 stop-if-true
              n2185 = node-c288() -> ()  [unwired: 2 out]
              n2186 = flat-sequence {
                tunnel: w3672 -> [w3685]
                tunnel: w3671 -> [w3682]
                tunnel: [w3681] -> w3670
                tunnel: [w3771] -> w3673
                tunnel: w3670 -> [w3770]
                tunnel: [w3770] -> w3669
                frame #0 {
                  n2187 = local read "Delta Fl. 2"() -> (w3676:dbl)
                  n2188 = local read "Delta Fl. 1"() -> (w3677:dbl)
                  n2189 = Select(t=w3677, s="APD to Watch", f=w3676) -> (s? t:f=w3675:dbl)
                  n2190 = Multiply(x="Fl. Delta Thresh. (kHz)", y=1000.0) -> (x*y=w3684:dbl)
                  n2191 = Greater?(x=w3675, y=w3684) -> (0:w3679:bool)
                  n2192 = Or(x="Force Yank", y=w3679) -> (x .or. y?=w3680:bool)
                  n2193 = case shown="True" w3680 {
                    tunnel: w3685 -> [_ w3695]
                    tunnel: w3682 -> [w3687 w3691]
                    tunnel: [w3687 w3688] -> w3681
                    frame False {
                    }
                    frame True {
                      n2194 = flat-sequence {
                        tunnel: w3692 -> [w3701]
                        tunnel: [w3701] -> w3696
                        tunnel: w3695 -> [w3700]
                        tunnel: [w3700] -> w3694
                        tunnel: [w3699] -> w3693
                        tunnel: w3691 -> [w3698]
                        tunnel: [w3697] -> w3690
                        tunnel: w3696 -> [w3726]
                        tunnel: w3694 -> [w3725]
                        tunnel: w3693 -> [w3724]
                        tunnel: w3690 -> [w3723]
                        tunnel: [w3723] -> w3689
                        tunnel: w3689 -> [w3768]
                        tunnel: [w3768] -> w3688
                        frame #0 {
                          n2195 = call <vilib>:"Beep.vi"() -> ()  [unwired: 3 in, 9 out]
                          n2196 = local write "Waiting"(FALSE ("Waiting")) -> ()
                          n2197 = Increment(x=w3698) -> (x+1=w3697:u8)
                          n2198 = case shown="\"Yank\"" w3700 {
                            tunnel: w3697 -> [_ _ w3707]
                            frame "Image" {
                              n2199 = property on="Confocal Image" class="Bool (strict)"("Val(Sgnl)"=TRUE ("Value (Signaling)")) -> ()  [unwired: 2 in, 2 out]
                            }
                            frame "Alarm", Default {
                            }
                            frame "Yank" {
                              n2200 = flat-sequence {
                                tunnel: w3707 -> [w3710]
                                tunnel: [w3709] -> w3706
                                tunnel: ["N Array El"] -> w3705
                                tunnel: w3706 -> [w3720]
                                tunnel: w3705 -> [w3716]
                                frame #0 {
                                n2201 = Multiply(x="Yank Delay (s)", y=1000.0) -> (x*y=w3713:dbl)
                                n2202 = Quotient & Remainder(x=w3710, y="N Array El") -> (x-y*floor(x/y)=w3709:u8)  [unwired: 1 out]
                                n2203 = Wait (ms)(milliseconds to wait=w3713) -> ()  [unwired: 1 out]
                                }
                                frame #1 {
                                n2204 = Random Number (0-1)() -> (number: 0 to 1=w3717:dbl)
                                n2205 = Multiply(x=w3716, y=w3717) -> (x*y=w3715:dbl)
                                n2206 = Round Toward -Infinity(1:w3715) -> (0:w3714:dbl)
                                n2207 = Select(t=w3714, s="Random Choice", f=w3720) -> (s? t:f=w3718:dbl)
                                n2208 = Index Array(array="Yank to Delta Array (MHz)", index=w3718) -> (element=w3721:dbl)
                                n2209 = property on="Trap Delta (MHz)" class="DigNum (strict)"("Val(Sgnl)"=w3721) -> ()  [unwired: 2 in, 2 out]
                                }
                              }
                            }
                          }
                          n2210 = local read "Time (s)"() -> (w3699:dbl)
                          "Fl. High" <- TRUE ("Yanking")
                        }
                        frame #1 {
                          n2211 = node-c288() -> (w3728:T23)  [unwired: 4 out]
                          n2212 = timed-loop {
                            timing: w3728 -> [_]
                            timing-out: [_] -> w3727
                            tunnel: w3726 -> [w3744]
                            tunnel: w3725 -> [w3742]
                            tunnel: w3724 -> [w3741]
                            stop <- w3743 stop-if-true
                            n2213 = node-c288() -> ()  [unwired: 2 out]
                            n2214 = local read "Fl. Delta Thresh. (kHz)"() -> (w3736:dbl)
                            n2215 = local read "Fl. Triggered..."() -> (w3745:bool)
                            n2216 = local read "Delta Fl. 1"() -> (w3732:dbl)
                            n2217 = local read "Delta Fl. 2"() -> (w3730:dbl)
                            n2218 = local read "Stop All"() -> (w3739:bool)
                            n2219 = local read "APD to Watch"() -> (w3731:bool)
                            n2220 = Select(t=w3732, s=w3731, f=w3730) -> (s? t:f=w3729:dbl)
                            n2221 = Not(x=w3745) -> (.not. x?=w3740:bool)
                            n2222 = Multiply(x=w3736, y=1000.0) -> (x*y=w3735:dbl)
                            n2223 = Negate(x=w3735) -> (-x=w3734:dbl)
                            n2224 = Less?(x=w3729, y=w3734) -> (x < y?=w3738:bool)
                            n2225 = Compound Arithmetic op=OR(w3738, w3739, w3740, "Force Reset") -> (w3743:bool)
                            n2226 = case shown="True" w3743 {
                              tunnel: w3744 -> [_ w3756]
                              tunnel: w3742 -> [_ w3755]
                              tunnel: w3741 -> [_ w3753]
                              frame False {
                              }
                              frame True {
                                n2227 = case shown="\"Yank\"" w3755 {
                                tunnel: w3756 -> [_ w3757]
                                frame "Image", Default {
                                }
                                frame "Yank" {
                                n2228 = flat-sequence {
                                tunnel: [w3762] -> w3758
                                tunnel: w3757 -> [w3762]
                                tunnel: w3758 -> [w3763]
                                frame #0 {
                                n2229 = local read "Yank Delay (s)"() -> (w3761:dbl)
                                n2230 = Multiply(x=w3761, y=1000.0) -> (x*y=w3759:dbl)
                                n2231 = Wait (ms)(milliseconds to wait=w3759) -> ()  [unwired: 1 out]
                                }
                                frame #1 {
                                n2232 = property on="Trap Delta (MHz)" class="DigNum (strict)"("Val(Sgnl)"=w3763) -> ()  [unwired: 2 in, 2 out]
                                }
                                }
                                }
                                }
                                n2233 = local read "Time (s)"() -> (w3754:dbl)
                                n2234 = Subtract(x=w3754, y=w3753) -> (x-y=w3750:dbl)
                                "Duration (s)" <- w3750
                                n2235 = Number To Decimal String(number=w3750, width (-)=i16 0) -> (decimal integer string=w3748:string)
                                n2236 = Concatenate Strings(w3748, " s fluorescence event." ("string")) -> (w3746:string)
                                n2237 = local read "Messages"() -> (w3752:string)
                                n2238 = call "Update messages.vi"("Message to add"=w3746, "Old message string"=w3752) -> ("New message string"=w3751:string)
                                n2239 = call <vilib>:"Beep.vi"() -> ()  [unwired: 3 in, 9 out]
                                n2240 = local write "Messages"(w3751) -> ()
                              }
                            }
                            n2241 = node-c288() -> ()  [unwired: 2 out]
                          }
                          n2242 = node-c288(w3727) -> ()  [unwired: 1 out]
                        }
                        frame #2 {
                          n2243 = local write "Fl. High"(FALSE ("Yanking")) -> ()
                        }
                      }
                      n2244 = local read "Trap Delta (MHz)"() -> (w3692:dbl)
                    }
                  }
                }
                frame #1 {
                  n2245 = local read "Stop All"() -> (w3774:bool)
                  n2246 = local read "Fl. Triggered..."() -> (w3772:bool)
                  n2247 = Not(x=w3772) -> (.not. x?=w3773:bool)
                  n2248 = Or(x=w3773, y=w3774) -> (x .or. y?=w3771:bool)
                  n2249 = Not(x=w3771) -> (.not. x?=→"Waiting":bool)
                }
              }
              n2250 = node-c288() -> ()  [unwired: 2 out]
            }
            n2251 = node-c288(w3667) -> ()  [unwired: 1 out]
          }
        }
      }
      event "Stop All": Value Change {
        n2252 = event-data() -> ()  [unwired: 7 out]
        n2253 = local read "Stop All"() -> (w3780:bool)
      }
    }
    n2254 = node-c288() -> ()  [unwired: 2 out]
  }
  n2255 = node-c288(w14) -> ()  [unwired: 1 out]
  n2256 = node-c288(w68) -> ()  [unwired: 1 out]
  n2257 = node-c288(w75) -> ()  [unwired: 1 out]
  n2258 = node-c288(w73) -> ()  [unwired: 1 out]
  n2259 = node-c288(w163) -> ()  [unwired: 1 out]
  n2260 = flat-sequence {
    tunnel: w33 -> [w3785]
    tunnel: [w3784] -> w39
    tunnel: [w3781] -> w38
    tunnel: w37 -> [_]
    tunnel: w36 -> [_]
    tunnel: w35 -> [_]
    tunnel: w34 -> [_]
    tunnel: w32 -> [w3782]
    tunnel: w39 -> [w3788]
    tunnel: w38 -> [w3787]
    frame #0 {
      w3783 = FALSE ("APD to FIFO")
      n2261 = xnode "Read/Write Control"("FPGA VI Reference In"=w3785, "error in"=w3782, "APD to FIFO"=w3783, "AI to FIFO"=w3783) -> ("FPGA VI Reference Out"=w3784:T19, "error out"=w3781:errorcluster)
    }
    frame #1 {
      n2262 = xnode "Invoke Method"("FPGA VI Reference In"=w3788, "error in"=w3787) -> ("FPGA VI Reference Out"=w3786:T19)  [unwired: 1 out]
      n2263 = xnode "Close FPGA VI Reference"("FPGA VI Reference In"=w3786) -> ()  [unwired: 1 in, 1 out]
    }
  }
